vi "UHR-Fleezers Control (host) -TL FB Corrected.vi"(0 "Tab Control":T5(tab)) -> ()   [LabVIEW 2013]
uses:
  <vilib>/Utility/miscctls.llb/LVPoint32TypeDef.ctl
  <vilib>/Utility/miscctls.llb/LVMinMaxIncTypeDef.ctl
  <vilib>/userdefined/High Color/nirio_resource_hc.ctl
  <vilib>/Platform/TimedLoop/XDataNode/timing_clust.ctl
  <vilib>/Platform/TimedLoop/XDataNode/nitl_modes.ctl
  <vilib>/Platform/TimedLoop/XDataNode/wakeup.ctl
  <vilib>/Analysis/baseanly.llb/Mean (DBL).vi
  <vilib>/FPGAPlugInAG/PCIe-7852R/niLvFpga_Open_PCIe-7852R.vi
  <vilib>/FPGAPlugInAG/PCIe-7852R/niLvFpga_Reset_PCIe-7852R.vi
  <vilib>/Utility/error.llb/Error Cluster From Error Code.vi
  <vilib>/rvi/errors/niLvFpgaAdjustHostInterfaceError.vi
  <vilib>/rvi/interface/common/niFpgaWaitOnOcc.vi
  <vilib>/FPGAPlugInAG/PCIe-7852R/niLvFpga_Run_PCIe-7852R.vi
  <vilib>/express/express analysis/Spectral/Block/exnSpectralBlock spectral measurements PSD poly.vi
  <vilib>/express/express analysis/Spectral/Block/exnSpectralBlock spectral measurements PSD WFM.vi
  <vilib>/Waveform/WDTOps.llb/WDT Append Waveforms DBL.vi
  <vilib>/FPGAPlugInAG/PCIe-7852R/niLvFpga_Abort_PCIe-7852R.vi
  <vilib>/FPGAPlugInAG/PCIe-7852R/niLvFpga_Close_PCIe-7852R.vi
  openfpgaref.8.6.ctl
  <vilib>/Platform/TimedLoop/XDataNode/XDataNode.xnode
  <vilib>/rvi/interface/nirviOpenFPGA/nirviOpenFPGA.xnode
  FPGA Bitfiles/UHR-FleezersInst_FPGATarget_UHR-FleezersCont_9yP24kGuHI0.lvbitx
  UHR-Fleezers Control (fpga) FB changed - 10.3.vi
  <vilib>/rvi/interface/nirviMethod/nirviMethod.xnode
  <vilib>/rvi/interface/nirviReadWriteControl/nirviReadWriteControl.xnode
  <vilib>/express/express analysis/Spectral/XNode/ExpressSpectralMeasurementsBlockNode.xnode
  <vilib>/rvi/interface/nirviCloseFPGA/nirviCloseFPGA.xnode
  <vilib>/Analysis/NI_AALBase.lvlib
  <vilib>/Platform/TimedLoop/XDataNode/XDNodeRunTimeDep.lvlib
  <vilib>/vision/NI_Vision_Development_Module.lvlib
  <vilib>/rvi/errors/niLvFpgaMergeErrorWithErrorCode.vi
  NiFpgaLv.dll
  <vilib>/FPGAPlugInAG/PCIe-7852R/niLvFpga_ConfigureFifo_PCIe-7852R.vi
  <vilib>/FPGAPlugInAG/PCIe-7852R/niLvFpga_ReadFifo_PCIe-7852R.vi
panel:
  out "Tether Extension (nm, calculated)":dbl=nan format="%0.2f"
  in  "Set SP to Reading":bool
  out "Trap X (AI1)":T1={"Trap 1"=-1.0, "Trap 2"=0.899993896484375}
  in  "Trap Pos FB SP":fxp<+/-,16,1>=-0.092803955078125 caption="Setpoint"
  in  "Trap Pos. FB ON":bool
  out "Trap Positions":waveform(dbl)[](graph)=[{"t0"=timestamp(12.90000000000001 s since 1904-01-01), "dt"=0.15, "Y"=[-1.7479351299698465e-12, -1.7479351299698465e-12], "attributes"=variant("NI_ChannelName"=variant(string "Trap 1 Pos."))}, {"t0"=timestamp(12.90000000000001 s since 1904-01-01), "dt"=0.15, "Y"=[6.991740519879386e-12, 6.991740519879386e-12], "attributes"=variant("NI_ChannelName"=variant(string "Trap 2 Pos."))}]
  out "Action (%)":dbl(knob) scale=-100.0..100.0
  in  "Trap Pos. FB Out Scale 2^n":u8=23 caption="Action Scale"
  out "Location path":path=path "C:/Users/Fleezers/Desktop/UHR-Fleezers Instrument - Charlie/Locations.txt"
  out "Location Matrix":string[][](array[string])=[["N.D.\r\n", "N.D.\r\n", "N.D.\r\n"], ["0.19233\r\n", "0.00156\r\n", "0.20615\r\n"], ["N.D.\r\n", "N.D.\r\n", "N.D.\r\n"], ["N.D.\r\n", "N.D.\r\n", "N.D.\r\n"]]
  in  "radius":i32=10 min=1 max=20
  in  "clear markers":bool
  in  "trap\nmarkers?":bool
  in  "Pump 3 contents":string="Bottom: ADig beads" caption="contents"
  in  "Pump 1 contents":string="Top: DNA beads" caption="contents"
  in  "Scripts":T2(tab)
  in  "Take Stepping Data":bool
  in  "Got DNA bead":bool
  in  "Got ADig bead":bool
  in  "Cap 1 Flow ON":bool=TRUE
  in  "Move Cap. 1 (DNA Top)":bool
  in  "Cal/Data Acq. Spot":bool
  in  "Dump Beads":bool
  in  "Cap 1 T ON":bool=TRUE
  in  "Cap 1 Samp Flow ON":bool=TRUE
  in  "Offset 2 Set":dbl=2.0
  in  "Offset 1 Set":dbl=1.0
  in  "Cal @ (MHz)":dbl=20.0
  in  "W/ Offset 1":bool=TRUE
  in  "Offset 1 Start (MHz)":dbl=13.0
  in  "W/ Offset 2":bool
  in  "Offset 2 Start (MHz)":dbl=16.0
  in  "Pause at Closest Delta (s)":dbl
  in  "Move to Delta 2 (MHz)":dbl=41.0
  in  "Attempt Limit":dbl=30.0 caption="Limit"
  out "Attempts":dbl=1.0
  in  "Wait Before Save (s)":u32=1
  in  "Fish for Tether":bool
  in  "Closest Delta (MHz)":dbl=13.0 step=0.25
  in  "Stop F (pN)":dbl=10.0
  in  "Then...":string(combo)="2"
  in  "Move to Delta 1 (MHz)":dbl=15.0
  in  "Tether Alarm?":bool=TRUE
  out "Tether":bool
  in  "TA Cancel Save?":bool=TRUE
  in  "TA Green Off?":bool=TRUE
  in  "Raster Set Upon Tether":u32=1
  in  "Save at end (5, 6)":bool
  in  "N Steps":dbl=20.0
  in  "Step Size (nm)":dbl=0.34
  in  "Save ave factor":dbl=1.0
  in  "Dip Trap Delta 1 (MHz)":dbl=15.0
  in  "Move Trap Before?":bool
  in  "Save Data After?":bool
  in  "Green ON After?":bool
  in  "Dip Trap Delta 2 (MHz)":dbl=15.0
  in  "Move Trap After?":bool
  in  "Duration (s)":dbl=1.0
  in  "Dip for Protein":bool
  in  "APD to Watch":bool
  out "Duration (s)":dbl
  in  "Action":string(combo)="Yank"
  in  "Fl. Triggered...":bool
  in  "Fl. Delta Thresh. (kHz)":dbl=0.6
  out "Waiting":bool
  out "Fl. High":bool
  in  "N pts to average":u16=6
  in  "Yank Delay (s)":dbl=3.5
  in  "Yank to Delta Array (MHz)":dbl[](array[numeric])=[16.3, 15.85, 14.85]
  in  "N Array El":u8=3 min=1 step=1
  in  "Random Choice":bool=TRUE
  in  "Force Yank":bool
  in  "Force Reset":bool
  in  "Y change (mm)":dbl
  in  "Profile":bool
  out "Sigma/Mean 2":dbl=nan caption="Sigma/Mean" format="%#_2g"
  out "Rate sigma (Hz) 2":dbl caption="Sigma (Hz)" format="%0.2f"
  out "APD 2 Rate (Hz)":dbl format="%#_3p"
  out "Primary Video Display":T3(plugin-control)
  out "Waveform Graph":dbl[](graph) caption="APD Line Scan"
  out "Messages":string="7:59 AM\tUHR-Fleezers ready.\r"
  in  "APD Ave N":dbl=10.0
  out "Int. Time (s)":dbl=3.0
  in  "Stop All":bool=TRUE
  out "Sigma/Mean":dbl=nan format="%#_2g"
  out "Rate sigma (Hz)":dbl caption="Sigma (Hz)" format="%0.2f"
  in  "Tab Control 6":T4(tab)=enum."Imaging"
  in  "APD 2 Offset":dbl
  in  "APD 1 Offset":dbl
  out "RMS (Ang)":dbl=nan format="%_2g"
  in  "Bead Sep. Int. Time (s)":dbl=5.0 caption="Int. Time (s)"
  in  "Below (kHz)":dbl=0.5
  in  "Above (kHz)":dbl=2.0
  in  "Adjust Scale\nto Mean":bool
  in  "Rescale on Mean":bool
  in  "Offset (nm)":dbl
  out "Mean":dbl=nan caption="Mean (pN)" format="%#_3g"
  out "Force":waveform(dbl)[](graph)=[{"t0"=timestamp(12.90000000000001 s since 1904-01-01), "dt"=0.15, "Y"=[nan, nan], "attributes"=variant("NI_ChannelName"=variant(string "T1 X"))}, {"t0"=timestamp(12.90000000000001 s since 1904-01-01), "dt"=0.15, "Y"=[nan, nan], "attributes"=variant("NI_ChannelName"=variant(string "T2 X"))}]
  out "APD Chart":waveform(dbl)[](graph)=[{"t0"=timestamp(12.90000000000001 s since 1904-01-01), "dt"=0.02, "Y"=[0.0, 0.0, 0.0, 0.0, 0.0, 0.0, 0.0, 0.0, 0.0, 0.0, 0.0, 0.0, 0.0, 0.0, 0.0], "attributes"=variant("NI_ChannelName"=variant(string "APD 1"))}, {"t0"=timestamp(12.90000000000001 s since 1904-01-01), "dt"=0.02, "Y"=[0.0, 0.0, 0.0, 0.0, 0.0, 0.0, 0.0, 0.0, 0.0, 0.0, 0.0, 0.0, 0.0, 0.0, 0.0], "attributes"=variant("NI_ChannelName"=variant(string "APD 2"))}]
  in  "Calibration":u16(ring) items=["None", "Position", "Force"]
  out "T1 X":dbl=nan caption="T1 X (pN)" format="%0.2f"
  out "T2 X":dbl=nan caption="T2 X (pN)" format="%0.2f"
  out "Bead Separation":waveform(dbl)(graph)={"t0"=timestamp(12.90000000000001 s since 1904-01-01), "dt"=0.15, "Y"=[nan, nan], "attributes"=variant("NI_ChannelName"=variant(string "T1 X"))}
  in  "Amplitude (nm)":dbl=3.0
  out "Bead Mean (nm)":dbl=nan caption="Mean (nm)" format="%0.2f"
  out "Difference":dbl=nan caption="Difference (pN)" format="%.2g"
  in  "Take Detection Laser\nImage":bool
  out "APD 2":T3(plugin-control) caption="APD 2 (Cy5)"
  in  "Flip Green Filter":bool
  in  "Set X Only":bool
  in  "Set Y Only":bool
  out "APD 1":T3(plugin-control) caption="APD 1 (Cy3)"
  out "Detection Laser Y":T3(plugin-control)
  out "Pointer Y (V)":dbl format="%_3g"
  out "Pointer X (V)":dbl format="%_3g"
  in  "Set Confocal Spot (X-Y)":bool
  out "Detection Laser X":T3(plugin-control)
  out "Saved APD":dbl[][](graph) caption="Most Recent Time Trace"
  out "Trap Delta Graph":dbl[](graph) caption="Most Recent Time Trace"
  out "Save APD Deriv":dbl[][](graph) caption="Most Recent Time Trace"
  out "Delta Fl. 1":dbl
  out "Delta Fl. 2":dbl
  out "All Signals":waveform(dbl)[](graph)=[{"t0"=timestamp(12.90000000000001 s since 1904-01-01), "dt"=0.02, "Y"=[0.0, 0.0, 0.0, 0.0, 0.0, 0.0, 0.0, 0.0, 0.0, 0.0, 0.0, 0.0, 0.0, 0.0, 0.0], "attributes"=variant("NI_ChannelName"=variant(string "APD 1"))}, {"t0"=timestamp(12.90000000000001 s since 1904-01-01), "dt"=0.02, "Y"=[0.0, 0.0, 0.0, 0.0, 0.0, 0.0, 0.0, 0.0, 0.0, 0.0, 0.0, 0.0, 0.0, 0.0, 0.0], "attributes"=variant("NI_ChannelName"=variant(string "APD 2"))}, {"t0"=timestamp(12.90000000000001 s since 1904-01-01), "dt"=0.15, "Y"=[nan, nan], "attributes"=variant("NI_ChannelName"=variant(string "T1 Y"))}, {"t0"=timestamp(12.90000000000001 s since 1904-01-01), "dt"=0.15, "Y"=[nan, nan], "attributes"=variant("NI_ChannelName"=variant(string "T1 X"))}, {"t0"=timestamp(12.90000000000001 s since 1904-01-01), "dt"=0.15, "Y"=[-0.0004235663930173644, -0.0004722739341410556], "attributes"=variant("NI_ChannelName"=variant(string "T1 Sum"))}, {"t0"=timestamp(12.90000000000001 s since 1904-01-01), "dt"=0.15, "Y"=[nan, nan], "attributes"=variant("NI_ChannelName"=variant(string "T2 Y"))}, {"t0"=timestamp(12.90000000000001 s since 1904-01-01), "dt"=0.15, "Y"=[nan, nan], "attributes"=variant("NI_ChannelName"=variant(string "T2 X"))}, {"t0"=timestamp(12.90000000000001 s since 1904-01-01), "dt"=0.15, "Y"=[-0.0005883053071687949, -0.0006281319620349712], "attributes"=variant("NI_ChannelName"=variant(string "T2 Sum"))}, {"t0"=timestamp(12.90000000000001 s since 1904-01-01), "dt"=0.15, "Y"=[nan, nan], "attributes"=variant("NI_ChannelName"=variant(string "T1 FB X"))}, {"t0"=timestamp(12.90000000000001 s since 1904-01-01), "dt"=0.15, "Y"=[-0.0004680013428144157, -0.0005167699209570592], "attributes"=variant("NI_ChannelName"=variant(string "T2 FB Sum"))}, {"t0"=timestamp(12.90000000000001 s since 1904-01-01), "dt"=0.15, "Y"=[nan, nan], "attributes"=variant("NI_ChannelName"=variant(string "T2 FB X"))}, {"t0"=timestamp(12.90000000000001 s since 1904-01-01), "dt"=0.15, "Y"=[-0.0006226691488387671, -0.0006504715109714008], "attributes"=variant("NI_ChannelName"=variant(string "T2 FB Sum"))}, {"t0"=timestamp(12.90000000000001 s since 1904-01-01), "dt"=0.15, "Y"=[-0.0007901852473525123, -0.0008601641895809732], "attributes"=variant("NI_ChannelName"=variant(string "PSD Y"))}, {"t0"=timestamp(12.90000000000001 s since 1904-01-01), "dt"=0.15, "Y"=[0.00031556138798181086, 0.0002525101474044007], "attributes"=variant("NI_ChannelName"=variant(string "PSD X"))}, {"t0"=timestamp(12.90000000000001 s since 1904-01-01), "dt"=0.15, "Y"=[-0.00019678334910122974, -0.0002453993346964931], "attributes"=variant("NI_ChannelName"=variant(string "PSD Sum"))}]
  in  "Signals to Plot":i32(listbox)
  out "Trap Disp. Freq. (Hz)":dbl=6.666666666666667 caption="Freq. (Hz)" format="%#_6p"
  out "Display Period (s)":dbl=0.15 caption="Period (s)" format="%#_6p"
  in  "Trap Disp. Downsample":dbl=10000.0 caption="Downsample" max=20000.0
  in  "APD Disp. Scale":dbl=0.1 caption="Scale (Divide,\nfor above plot only)"
  in  "APD Disp. Downsample":dbl=2.0 caption="Integrate" min=1.0 max=30.0 step=1.0
  out "APD Display Freq. (Hz)":dbl=50.0 caption="Freq. (Hz)"
  out "APD Display Period (s)":dbl=0.02 caption="Period (s)"
  out "FFT 1":cluster{"f0":dbl, "df":dbl, "magnitude":dbl[]}[](graph)=[{"f0"=0.0, "df"=16.666666666666668, "magnitude"=[-331.1367572010275, -79.05506245821404, -86.61411242440559, -88.4728176091699, -90.3181253945935, -94.12566333707997, -92.52740723119955, -94.92192587982518, -99.60936585245742, -96.87568627870715, -94.02570383337763, -83.8058550151726, -97.57441397235512, -101.59968530846606, -101.523049255742, -103.35038532190343, -101.58594091014982, -102.96098031851216, -91.39759462745924, -103.75019963279499, -104.45030075054324, -103.04245334279298, -104.0720279134107, -106.06482372394834, -103.69131867828104, -104.40395035115309, -105.96420043276396, -107.6735556337804, -106.673030006608, -107.34889066208132, -108.05626565233933, -106.25659018850432, -105.29934513380842, -105.43096056709592, -108.3728498841465, -106.0555440144992, -105.78001282181421, -107.48741857324953, -108.67624970548897, -105.39976667156175, -105.91413119232612, -109.4222808198164, -107.0898971593174, -107.91164191890915, -108.26032038855709, -107.58332347164534, -108.23559688234297, -108.01271040303237, -107.66511723652701, -106.51901583170391, -109.27249501469946, -108.55647681594805, -107.93499259231463, -107.05068166453935, -109.13641475410455, -109.29679733781423, -108.19360835527803, -109.57747591546632, -109.58364591011674, -110.47061433372711, -109.8144340420426, -108.79067462293897, -107.54887553357234, -107.99559866705923, -108.85023923652685, -109.68733225238618, -108.51101278437793, -108.51620475114115, -108.22212402200637, -104.63726950302143, -110.2989919678048, -107.61796444414897, -108.68882962798736, -104.79193983043893, -103.59504263746938, -93.64633660288543, -101.9191640501395, -105.73717393151816, -108.92572458793902, -107.43962662800902, -107.79595323081325, -107.0923101993207, -108.17603277205289, -107.87074270713183, -109.20899066381877, -108.61832060412445, -109.10072003106593, -105.76480632823524, -108.60877649218978, -109.67541158970121, -110.2286232768028, -109.84952155309578, -109.33772024076384, -109.95251642394683, -110.14777282585466, -109.13825677905699, -110.05989365698167, -109.39359990189426, -110.56255614635295, -109.66477183197163, -108.9397158528824, -110.26529907650465, -109.20049464984628, -108.20183857013548, -109.09752250184418, -108.00440442238454, -108.35465963524055, -111.16774134451799, -110.34812550238405, -108.94506763426756, -108.72845542102493, -109.41512344014713, -112.44661664432377, -110.35437330889101, -111.32939440655925, -109.42989530434981, -110.98084669076195, -111.92160561143541, -108.57755551751093, -111.40042616180912, -110.15284955891853, -112.21455132279115, -111.40787773511747, -108.82949641635288, -110.13442122547907, -111.42229298204664, -112.06314940885191, -110.6015308813694, -109.51144097251623, -111.15989713761475, -110.25535755335385, -109.65868178057926, -110.51649885452997, -109.77194745285269, -108.4234206864394, -109.50892632093968, -109.46471287444389, -107.92241289271415, -109.72283805386196, -108.63426821579918, -110.37316681536255, -111.09713996884652, -110.32903619589223, -105.32012665515045, -107.36858557554393, -108.00382215905725, -110.06430686942338, -108.81666625979916, -110.01277074453823, -110.94194741225512, -109.65934609082873, -107.80979136006962, -112.81333866824724, -111.61474300955487, -109.83998277184975, -109.45953946904639, -109.79640584952526, -108.19172301667324, -109.28894656674316, -107.61471301278785, -108.83814006090513, -109.08866847726084, -108.20250571862371, -107.96222236861584, -107.03811197900873, -108.93533000393974, -107.74482548035408, -110.79811544577694, -111.1387476496877, -107.42970105883512, -109.18442281176472, -108.73546184641192, -108.71800246690864, -108.51945944378063, -108.06825856571285, -107.27210712368412, -108.12304695877637, -107.84933283677306, -109.73682373154998, -109.32284761503395, -109.31328817453769, -106.68762108642842, -109.79203616876461, -109.9020278896408, -110.27080024357275, -108.54152101558762, -111.00464391726017, -112.42244020766577, -110.82707315747889, -111.00344011890857, -109.90461839395674, -109.42877207451863, -109.73549298167016, -111.67494793393293, -108.85799077901427, -108.5348443278263, -109.803781083881, -108.30644755543659, -108.5079527456017, -111.2055351312823, -108.53089994340155, -108.01739789012176, -108.70360662855235, -107.95873456794631, -109.58297170693093, -108.9372401694271, -110.15921663527153, -109.22399119911955, -110.89883651739237, -108.92840112258382, -110.0545300523626, -109.05961065387005, -109.45831398589371, -108.61239387653227, -110.13001256174265, -108.80060224137931, -109.46327400696283, -108.0177965824709, -109.29727944627197, -110.3237255895986, -109.03258262543821, -110.97880178489321, -109.70034895077919, -111.16405638194153, -109.17324451464711, -109.65698250854277, -108.96750235822178, -112.00534231585624, -108.69274607723942, -108.98110446396657, -108.40723795464795, -111.44459094807324, -111.74799245277113, -111.1601960491512, -108.92048232753773, -110.30506377784799, -111.33145973979093, -110.91850998672503, -110.33684985776448, -108.90206518366908, -109.28458878227542, -108.98773986023751, -110.85813863075646, -109.00041591105906, -110.84543686681204, -109.84382395806176, -109.69722434763266, -108.50915601095721, -107.80829925826895, -110.59736107582401, -109.75377770317087, -109.3992084496136, -110.51151565846742, -112.49753959826434, -109.7299632589479, -109.54070743868353, -109.90314341132164, -111.05974202976806, -109.03766862152392, -109.46667095459878, -109.52800799036197, -111.3163121356807, -110.07817134522178, -108.69251657453547, -109.40472158898045, -109.71400709815576, -110.60534468715097, -109.46937396724682, -107.70342491418788, -109.86331122597839, -108.64971387994616, -110.90117371097081, -108.34928840565928, -110.04172889660904, -111.52979926554961, -110.34759300823305, -109.62712781837159, -109.24131154553284, -110.23196152450447, -108.68509612326807, -108.0246905483419, -106.61876139289784, -101.5519630114271, -80.57695480953835, -102.03744443354402, -107.1449217193017, -110.0695213407169, -106.61597783999268, -110.79221011808191, -109.58974545931426, -109.1149802216988, -109.20993813088597, -109.63768480465863, -110.10428394219181, -109.08445084271477, -108.83472375362581, -109.69508502050168, -108.05588796178941, -110.62586360101581, -109.95315261676905, -107.52208264977473, -108.80708007514875, -110.43484881098874, -110.45942171588936, -107.83804717866751, -109.98973910294193, -109.3496496054193, -108.425252911127, -110.94579264380809, -108.54181722177951, -108.67696070083541, -108.4150202151644, -109.24973583101504, -112.0454922608961, -111.29046597340738, -110.75018248960077, -109.38326363603683, -109.2033340336957, -109.45076170874889, -109.52878049853727, -109.32340869724774, -110.98123395128233, -110.75736340635505, -109.7218385823809, -107.97422606064993, -109.77313701758703, -110.95948744392717, -110.08996774172691, -108.51011830110778, -109.78063140243836, -110.65996628628228, -109.83684298615616, -110.33329049188029, -110.13755118968292, -110.3717925645783, -108.55302219178951, -106.86811628734195, -108.6302156589162, -108.75341391045045, -108.32589578384841, -108.70061474734084, -112.30742263527534, -109.16842570592085, -109.29767035534508, -108.87829025017463, -108.2255616391397, -108.4316108616088, -108.82995906929271, -110.40135575415563, -109.51623498946435, -109.79409808792403, -107.03832759632121, -108.36534528684132, -109.72010868372905, -107.90933028179892, -106.95643597294047, -111.29929166165778, -110.23001135794706, -108.98838015381585, -109.79115357104436, -108.18627479511115, -108.14988122174307, -109.12074063466532, -109.41904850488358, -111.40409873721113, -108.83156790193294, -108.77032248953847, -108.88363158686694, -108.47515048290681, -105.94172147874599, -109.38146940214403, -109.21277078848794, -108.11309390545507, -110.70840012427504, -109.5504457849329, -109.52330684534209, -110.06776026911132, -108.21949434182314, -111.21266686269992, -108.78581501170974, -108.43115799297222, -109.63260325780062, -109.84070220619535, -109.72041980780126, -110.29615941882527, -110.60316734262464, -108.79165446414692, -110.95840439895592, -109.64926233107009, -109.16526769544322, -108.65292362430982, -109.56113898129935, -109.85693046339026, -108.92316027325207, -109.79492493553914, -109.38157962945887, -110.24545136266825, -109.30031463492487, -109.0795429936869, -111.4091719525013, -108.63499083917162, -108.43863465339358, -109.23207864880891, -111.21947487191643, -109.24525201480154, -109.56842406077318, -109.46711940800672, -111.91389548262572, -108.15655736690546, -108.71882059966947, -111.26328503478568, -110.95027143873176, -108.4853106242357, -110.36902802777546, -109.9314203579182, -108.77686164101732, -108.71871020068312, -111.04829661168574, -109.95072655339462, -109.88221342875462, -109.53241732756136, -108.2625005404823, -108.00677030040697, -110.19659317581693, -108.93858924796267, -109.46817875483995, -110.78063992017232, -111.11066570318451, -110.78774336696706, -109.19199744617812, -108.54914256407436, -109.28414960420909, -110.64143585101183, -110.5855350821307, -109.47578632252726, -108.89705360836223, -109.89214013612292, -107.93271261027171, -109.32631601340563, -108.60274611341092, -109.40110159872573, -110.889237682208, -110.01391165813328, -109.99747108785071, -108.65542819213674, -110.37211847668736, -110.44656500845738, -110.8128133834973, -108.8909299260433, -110.19551227077532, -111.37647266643523, -110.83802189730321, -109.98519377913681, -110.52378970770522, -108.16970420057817, -110.70974729773344, -110.76836765494402, -110.26884275594577, -109.22041044268806, -109.87809744746195, -107.76823252107832, -109.12119474042969, -110.28066108731146, -108.55000033509207, -110.18152097767907, -110.73030521152278, -111.49470908029893, -110.2320929919509, -110.03370979233021, -109.79181668155233, -108.6673501209991, -109.86695766650877, -107.88926518046961, -110.95525003776572, -109.18130359755742, -110.42618009658618, -107.90341931158893, -111.44736855661769, -110.72634267386593, -109.29945988519303, -107.67889101961411, -108.81148059987765, -109.13375212757057, -109.8122873383549, -109.80176697684155, -109.96342275204768, -109.90406635707086, -108.75674342748256, -110.12362902701081, -109.82151095527837, -108.62543344241836, -110.09171852771195, -110.21434637862887, -109.97254504855631, -109.27043209093468, -111.35149588204125, -110.12399876776051, -111.65983675538546, -109.28788875768564, -110.86554069990251, -111.26990906470603, -108.60956517491746, -111.49613890850938, -111.79685722966795, -109.26269485364045, -110.38555615546439, -109.40641023162068, -110.966136593156, -108.78892524584494, -110.29340727375603, -111.44032043281035, -109.95212021173755, -109.79233511584334, -112.41184021118175, -109.73687851881148, -108.65493879781806, -110.76132988919045, -108.43230346094671, -110.32968175895853, -110.29890782023821, -108.77609076424456, -110.3298662333555, -109.47734504217333, -108.2677295732245, -109.21234363352882, -107.83278941978479, -108.85136784424789, -108.43241251530755, -109.76609391460555, -108.53204373005357, -110.9660641972934, -110.3152512161094, -110.72570499399905, -109.23877906286317, -111.72407743101837, -109.20311421918561, -108.06021800233717, -109.29288625761943, -108.78395253409145, -111.85250172876302, -108.78827588901797, -109.79775055719482, -109.12089297455859, -109.49896359356035, -110.34432647103819, -107.94700097960238, -109.30489238477631, -108.89170290869342, -108.82574563272509, -110.11024077194833, -107.37946433552314, -109.60167933458756, -107.80625057819019, -110.11489057210264, -107.35436859378505, -105.69819484613895, -109.11280625683739, -109.27770293057978, -107.7053735252589, -109.75022444894368, -109.3310543596577, -107.87683693707739, -108.19931495338068, -109.26462246191564, -106.71885779297867, -100.00018022217961, -92.54434511397295, -107.20472143807373, -107.39203415155283, -110.04461177268398, -108.48860496315312, -109.0057168110333, -108.37627790492552, -108.4108380728248, -109.65509454313073, -109.64243000632982, -97.04219069306761, -109.0928856629964, -107.9760697315632, -107.52611064047497, -108.87702814778996, -109.08437599027614, -110.70097118837974, -109.00969860961283, -110.38275386163214, -110.0699155421545, -106.91498895181175, -106.22178738309017, -109.36827866896039, -107.59953130968307, -109.19516217272808, -108.31502495393616, -109.384158926223, -107.11670654202719, -108.09436312738853, -110.14559230873704, -109.84997663447679, -107.83465335309926, -108.60947100624459, -108.9932479423645, -109.17174810371898, -108.79457339828916, -109.40909327982367, -109.6328723628302, -109.51081854476179, -107.63054408568418, -109.63728404010122, -108.51163794839918, -107.55002282725216, -108.97796212764939, -107.24648164623483, -112.21470452291085, -108.74294024554423, -109.62070777514892, -108.05768666239368, -109.8224946685739, -109.34575507446003, -108.53536952609525, -109.60789300457671, -107.56681538208278, -109.22777325016398, -108.79047910308894, -110.10332477250668, -108.00206387955672, -108.45604004720035, -109.00645795765472, -109.81039564269616, -108.92785144634745, -108.3978471520567, -107.94411095685999, -110.53486519304262, -108.8773780319227, -109.03345093296107, -107.30746693745031, -108.54277704832029, -108.77629108166091, -108.91111762599647, -107.74965195880401, -109.97375370738439, -109.76326492689246, -107.91717581777407, -109.0730556927617, -107.66804873204664, -110.40438871064791, -108.05794247751498, -108.80206615156494, -107.51329354700796, -108.83687012994949, -107.57713176895379, -107.94774159581414, -109.41894615439651, -107.10869425078764, -110.51480854078629, -108.92221367099775, -109.91358786461535, -110.1744263092835, -109.30795472883494, -107.91359710691006, -109.77888185049835, -109.52060975706438, -108.66686651982212, -108.71041801553639, -110.13619546359467, -108.87957097273856, -109.72150387215271, -109.00776068810654, -109.70251113927438, -110.75769213896399, -108.53234896741436, -109.69439526582246, -110.15412541604617, -108.25183374628219, -107.97402569656481, -110.34920156998648, -108.45106995186384, -108.82031145748209, -111.38690005057539, -107.01968459818563, -110.3044500039584, -110.8755481852125, -111.08915057663255, -107.94824988655199, -110.21669144934839, -109.90539774633154, -109.58985438756767, -110.12258796623348, -109.41689951612143, -109.31128210476795, -109.00258476567323, -109.11093063041056, -108.83347064311234, -108.32685287566952, -109.44770946560935, -108.40145063144861, -109.68448193892085, -108.76525439243828, -107.62837139034596, -107.39300298848994, -109.36993934990318, -109.2465218489418, -106.66307369796812, -110.15891092764934, -109.57151745419041, -108.92425698310808, -109.8036704717834, -108.79751146756549, -109.25926431818017, -108.46260574057584, -109.1967554647261, -110.63319560262356, -109.02343067385144, -111.22073171487528, -109.4731095097105, -109.69335000085164, -109.48782989577005, -107.95204227683271, -108.19468255763758, -111.36195112053247, -109.55696116543685, -110.3130767640534, -108.9621824253354, -109.99735074896789, -109.20198058456344, -108.12100614259485, -111.27227490807289, -110.09248554008288, -109.14395535060149, -110.80882692379708, -109.22632926901655, -108.64497210802793, -111.00030482190711, -111.1317849358033, -107.43140429257826, -107.9783302193555, -109.2639893652291, -108.97008485446163, -108.66556668859064, -108.12995785876932, -109.73001061107855, -108.09691302413727, -110.68391499215569, -112.78583642012705, -108.7093037763389, -110.67868795924797, -109.0190959349128, -108.36247198231372, -109.82829353258869, -108.24916379311045, -109.84154533905823, -108.55470160833775, -109.75438989348815, -108.82865632118325, -107.63622268162582, -111.00943492886312, -110.81824358463759, -109.46028423652966, -107.52479398900992, -108.99087806823736, -109.94494831750349, -110.26788355564504, -109.8954055022304, -106.9478122391182, -108.91705388158901, -107.76095584490312, -109.28456723055147, -109.7982307261767, -108.98552661346622, -109.98937979783426, -110.57907422426224, -108.68113463944836, -108.06257240208589, -110.0707224529617, -109.19515280354733, -109.35868842818849, -110.37311467065695, -109.0404734478992, -108.16686395270187, -108.61859220485148, -109.19986437876149, -108.19707189725302, -110.06564239663074, -108.87850403465154, -110.63824157544798, -107.36918104067212, -108.7008736325543, -110.9359398265406, -111.08529123080929, -108.44209934821818, -109.79529621208783, -108.38917887958179, -108.169117639508, -109.24332926356216, -110.50584058811704, -109.63592524002665, -109.32261039377495, -109.16720880524552, -109.3084314664462, -109.5812223978583, -107.70213196487856, -108.0557884982431, -110.67058020007828, -111.68459781023608, -109.66270627185824, -110.52536245663693, -109.70208409132103, -108.78645420809342, -109.23122088059863, -109.24601474121832, -111.25604763816514, -109.50225851581177, -107.32434217163818, -109.28548556764925, -107.59972621660836, -110.46928774723048, -109.25950101547609, -110.32016453935465, -107.78482761561703, -107.89462895091089, -107.51366154391481, -108.08036891159172, -109.53371809947035, -101.2452927166745, -109.32763325689056, -107.52166868423687, -109.89648659445174, -109.11350200980485, -109.81336712738089, -110.02799517445062, -108.02767143538516, -107.97850220501483, -109.50772934896838, -109.31069875721964, -108.49991657749598, -105.60880911233095, -109.79128597340213, -106.91084537903113, -107.84880087118997, -109.63628170511824, -109.03203967193224, -110.64186113413658, -110.98027990365594, -112.33841002907062, -111.01793075565425, -108.58025797022215, -110.4259296883756, -110.38643255981424, -108.93051671115133, -110.97544177116494, -108.63883100482677, -108.37581711765226, -108.90240163126536, -107.94688047875466, -109.9482937437732, -110.09097112364414, -110.09805032265376, -111.44307114024532, -109.15483789122554, -110.9713708217832, -107.8548737634672, -111.41418477109195, -109.45699779859628, -97.03595099331734, -109.16746744169623, -109.66209204485918, -112.57048704774604, -109.73989735035725, -108.16252575067017, -110.7546980664636, -108.91536673403449, -109.20509151422344, -111.0260632167785, -109.62924582406518, -110.45466277291722, -110.2973970018937, -109.67550222925419, -108.84481022020094, -107.23686414357573, -111.79004633370906, -109.85453094194085, -109.45617270081004, -110.73920606732504, -108.90879956851099, -109.67774425528265, -109.4745715721361, -110.18080454693559, -109.26079184315502, -109.41692499885505, -109.02240975088358, -107.80833423058168, -109.32657361431549, -107.87138278655101, -110.910364670719, -109.70067156846706, -108.55301754282077, -109.4243252157005, -109.77567725161107, -107.83737232063925, -110.36509412773016, -109.6371048811367, -109.49430894422814, -108.55509251499753, -108.03996302911446, -110.4385715838736, -110.08864436068788, -109.48922484379962, -109.90865554258562, -109.7491963238264, -110.04796094537969, -107.413043439116, -108.54229076126079, -108.2522516728666, -109.75464941327974, -110.26795832300996, -109.28073673851144, -108.62990200974927, -109.89408067552287, -109.09160284731726, -109.90740624925795, -109.92534708896517, -109.79578862362752, -109.97278346890566, -107.80679350393824, -112.81728446281548, -108.09689504419987, -109.89549991422173, -108.43930976031248, -109.95153099843282, -108.18277483720716, -111.89607792605433, -109.52567003805, -109.17125106979698, -109.64300739407085, -108.21045178846524, -109.64036472149706, -109.02324448538845, -109.039163008889, -110.41006510134076, -109.50289952116489, -110.4732620447796, -110.08777181504614, -110.15589511434341, -109.55705089158471, -109.2547682932589, -110.86823885471617, -109.96330502176939, -109.85995369810554, -110.63211290903473, -112.08007783432191, -110.24725218052279, -107.62861148917592, -110.08691795849435, -108.89793794632287, -111.07702220466341, -109.46946126482341, -109.19747345337464, -110.70018609416007, -109.66366205691908, -110.78032312133551, -108.05724200456513, -108.195661625627, -110.90724508408255, -110.08307674771669, -110.76863516643007, -110.46620425061583, -109.16986788877276, -109.61921294239114, -108.51159432329543, -109.96308336765689, -107.38178944242856, -111.95930944846394, -109.3329826827624, -109.59119636368249, -108.83148571828912, -110.46194288788257, -105.87694286145472, -107.985886302892, -109.2975019660806, -111.05138725716857, -109.60005889204612, -110.92871351729086, -110.73480546964537, -108.41587420326718, -109.84275465824477, -108.8249071047676, -107.65358887817105, -108.3254150042995, -111.47362100321767, -112.7287536850025, -108.8217125660507, -109.50232320231771, -110.29587061625348, -109.30644535112089, -107.69178032077258, -110.84522325672016, -109.3735891463141, -109.12506388923123, -109.65582307934665, -111.11427272192576, -112.19827973435466, -109.11306367925813, -108.19203577968261, -107.89831568266465, -108.85805249169313, -109.51100049661844, -111.71546684086955, -109.53880495724334, -107.07739286222231, -110.66836728754211, -111.5415170557177, -110.16051267940297, -110.6107546662698, -111.36389129556191, -107.77888179117923, -110.34160392509817, -109.61287125994414, -110.23791773883013, -111.00669159903549, -110.97165069538953, -109.43965413392434, -110.6813161690388, -110.31441293654314, -111.96129906273796, -108.15998218707462, -110.08095912053633, -109.41084567452768, -109.28774416263552, -110.80159950384204, -110.41956747809755, -108.85005186267244, -107.9069227847757, -108.84249369063123, -109.92569208845894, -109.34109797584448, -109.41334788055491, -108.76462023086997, -108.22069272136177, -107.0786679601274, -108.30206755098202, -108.57613406368954, -110.83330887636482, -111.93966942736989, -109.76373713473264, -108.25782074884941, -108.16490627215555, -109.93351470267982, -110.75525684428368, -108.22814762283093, -109.73442331991602, -107.53145627482685, -108.27195221226805, -110.33032779278457, -109.48951857415828, -108.12599093700939, -107.97627415508097, -108.81426859968796, -111.21764717894752, -109.80856212352333, -110.92658779118501, -109.71551885834796, -110.38682741010847, -108.87671328341361, -109.68368600774755, -108.35359806351899, -111.7519400010676, -109.89407081573103, -108.24301180922755, -110.00646944788126, -108.6685299083706, -107.52856885980722, -111.7622363038509, -111.0025144494897, -108.64719599357296, -110.62968467177518, -108.821509935539, -107.94915453463719, -111.53070432277694, -109.87282048586256, -110.71167589371663, -109.79225006081626, -109.96203471712074, -110.29921092232489, -110.10644439440416, -111.28815007382043, -111.19165661703703, -108.46024117100558, -110.22528296512183, -110.32184972386672, -110.05120383416072, -109.78792549362107, -109.00355659956696, -108.85989369286315, -113.00899556732638, -110.91756826567867, -111.25016866167897, -111.84225040552181, -110.54451635944174, -110.72722829912917, -109.60759702177283, -110.49362602516815, -108.74419542915284, -110.3379671069179, -109.66259088220754, -110.45956400953156, -109.13956157147233, -109.27130155486806, -110.83015602667983, -109.17970724944131, -109.09662765889193, -108.0447366108107, -108.9536269357457, -110.35663108940085, -108.73418835472056, -113.42965806805827, -111.81270536656905, -110.06155590173537, -108.76582224646269, -106.7488061675813, -108.5700320158723, -111.11038264410035, -110.41435767488723, -109.12763443489911, -109.30517580756394, -111.61251165371237, -109.8116632664339, -109.36845864976851, -109.00390009629231, -110.54359197165573, -109.52629258465976, -110.75932197632896, -109.50903215359567, -107.42652056246085, -107.81146496533543, -103.22224383145215, -108.53803076819163, -109.78623360072066, -109.66306634612869, -110.80245829141279, -111.87835085452016, -102.27372781471168, -111.27763038431458, -108.45838423437681, -108.79077917058028, -109.31951755762685, -110.05415097017186, -109.5535934823387, -111.62732254641111, -110.73478247119641, -109.9468722686683, -110.39698367573979, -109.30612942398305, -109.7578384694043, -109.34817295524313, -105.56944757301993, -110.1940418750125, -109.27076023513962, -111.03491935225027, -112.2980497521063, -110.65725497955563, -109.0567530102422, -110.31700596563523, -109.64508026365678, -109.6190471404421, -110.52566833759428, -109.68595899227789, -109.7431160985074, -110.4798230300751, -109.45506977604765, -110.69504157940786, -110.63067849573177, -108.06456949500138, -107.99354148885966, -108.11349194720599, -109.15944121207349, -110.61766925164031, -110.14145801314527, -110.67420842201165, -111.91532881806512, -112.15901550030345, -109.94774413630104, -109.2819568305201, -110.94623189179737, -110.17685430287735, -110.39082916961016, -109.53953238698966, -110.76940623620611, -109.89327922318515, -109.10275695043765, -110.21445972656734, -110.58968777252528, -110.57016757660259, -109.59208496373341, -109.07946946465374, -109.10762003745964, -110.36892993974607, -109.81864495218393, -112.12972189864566, -109.26185849434863, -111.56305819991357, -111.36019621828058, -110.3397604159226, -109.58675612753163, -110.58041217474447, -106.34739062044932, -108.6722699609389, -110.03906060709869, -109.16794717548382, -109.65012481802809, -109.35377624077988, -110.51889143862303, -110.03397458059777, -110.7981307056636, -110.56653507062292, -107.61367005067231, -109.99279736988825, -111.79875182878175, -108.60382315996031, -109.71381533228038, -108.60388131505613, -107.0933685540362, -107.86037690830757, -108.40980028847238, -108.83869602763895, -110.76921375395764, -109.96766364716046, -110.8256171465781, -110.13805084291067, -108.5349140035878, -110.57158437465219, -110.8920694413417, -108.71646695477324, -108.33274238445665, -108.96152108305608, -111.03750932994224, -109.48915027983756, -110.29725207211165, -110.79527247268442, -109.47969936716117, -109.79306701834035, -110.16840035577498, -110.29840230783668, -109.15306387075587, -110.72651274964761, -109.08881658764956, -110.8349724030761, -110.64653625576447, -111.40392562616867, -109.94581588927414, -108.85136340231294, -109.77228546607624, -111.48297395390018, -109.7334001251941, -109.30537415590783, -109.63937411233408, -109.69785848648013, -109.3523781030017, -112.04667421182404, -111.56311816195343, -108.18548447362308, -110.63388993686104, -111.39768634137992, -109.87157345395542, -108.6734208287271, -109.46213300216168, -111.75774769437145, -110.10245994173216, -109.52385139033495, -110.96513097775451, -111.8709319163154, -111.54948269614047, -110.29760900080463, -108.52168175904663, -111.09033925738258, -111.14752744054172, -108.83074523709202, -109.05704141259113, -111.74377805749482, -109.57200906899736, -108.84121318623825, -110.86657990204343, -109.54363603755047, -110.89448416316372, -109.58965570570145, -110.21012263847972, -110.4063470702923, -109.5021950342969, -110.33648801598177, -110.90551031296536, -109.69205870504638, -109.8648503154861, -110.28183391384131, -109.65970942950766, -108.43615680946908, -111.11790511866548, -110.89043476451553, -113.64898442872548, -113.08004494963895, -110.81525412051718, -113.91009875719509, -110.95802128672312, -110.40944585634135, -110.33464695414992, -109.98984645778987, -110.18795067005652, -110.62364351231234, -110.44029833291248, -109.01598585569788, -110.95430216511514, -109.77987141110621, -108.54452361812068, -111.41780266439777, -110.47172771858405, -109.06084635984516, -109.30794593246578, -108.8764083815745, -108.18222749506985, -110.31330487887435, -109.04176821738014, -108.8558386035048, -109.47888284507395, -110.01459604573937, -110.48596659065309, -112.6781342298378, -109.85522803775775, -109.0569534499285, -109.08991286548698, -110.89485727880403, -109.18715778948663, -111.50381433568144, -111.3545424730884, -110.07710926239977, -111.99977850157067, -109.47444853853723, -109.81605328527645, -110.74995213151195, -112.56834665925544, -108.52052472391404, -110.89121213995557, -112.02004142355113, -108.66413739656008, -111.10053848695652, -110.41241079991636, -111.80152991764473, -110.21746151515111, -110.63265128607344, -109.483042128511, -112.78639954059729, -109.47114195846122, -109.23309637902875, -108.97133643967169, -110.08909147812822, -111.01105271457081, -111.18602432128249, -110.04633990216801, -109.53453538673071, -108.81939452082017, -111.13486114285661, -111.65877073200598, -111.63763706753498, -112.14107810664572, -113.6231865196724, -109.31743865878806, -109.18551713085722, -108.74951309653638, -109.28206426212142, -112.36687029711229, -110.10933061193728, -111.29501093502684, -108.19021080564794, -109.34497312126749, -110.37228033937312, -108.63277512903049, -110.61033993911002, -111.2975761598062, -111.49780004751436, -109.91019436685814, -109.32789992989028, -111.4482538110117, -110.1538439123475, -110.66347034043578, -110.05055133068794, -108.53002033538341, -111.7522199783972, -113.49108651193104, -108.03793940563418, -110.07108694011555, -110.83958739865201, -109.62805629409038, -112.69637731014087, -109.57996950503268, -110.104850643722, -108.83376203949506, -108.69400304840181, -110.59434352922563, -110.69121011800921, -110.18694553784364, -111.90598571547098, -110.30230802494223, -109.66810649416752, -112.6017099000434, -111.00296745333219, -110.64462650261785, -111.4775358707403, -111.98753241268494, -112.26574909791167, -112.04796822399412, -110.65853064447325, -109.6623218025264, -109.40559579075378, -110.42174451813142, -109.18991987957241, -111.02050178263048, -112.77950487440032, -110.42443751566815, -111.35440372400903, -108.5263524245987, -105.07498063939795, -107.15444425741984, -110.4508720018025, -110.25163264819463, -111.1383261104107, -109.91171620173931, -110.52200560606038, -110.5299174299573, -109.34628087255733, -110.26101817411786, -109.65071853372183, -109.66953335961068, -110.83590602054682, -110.980546313788, -109.4110066989163, -111.47223607390256, -110.00281523859483, -109.4088722967626, -109.00401922839337, -109.59655302543185, -109.7359970854586, -111.46016206343049, -110.23478747568004, -109.29441275295858, -109.82941912510167, -110.43088525283673, -108.21649744751299, -108.70220592702613, -105.2334473604296, -110.60620657984927, -107.97533820921146, -110.7664079806058, -110.56406610911355, -111.76465470250328, -108.84172809688911, -111.03661078143631, -109.85351980370237, -110.70091167176791, -109.52380717508088, -108.4356492672842, -112.25498760397127, -110.69648730540193, -110.36748838594507, -109.99090797924349, -111.2678642544111, -110.42541694325627, -111.4575545259775, -109.3211175669008, -112.7465573314208, -109.56208667784249, -111.59733497772172, -109.42295730962105, -108.55804089331346, -108.71397903286748, -110.09188290952392, -108.90810063278326, -110.31333217069538, -109.69794714542728, -109.06210020835357, -112.42465112160288, -111.74630553904855, -109.99304310093493, -108.93867687355595, -113.1669287525049, -109.09193568851137, -109.27500368450697, -108.99643325722404, -110.53962759110647, -111.2052088429852, -110.05855563908841, -110.30763723153481, -110.03411001268613, -109.6161415052669, -110.6304714466923, -110.17116005754627, -109.0753171640551, -110.92564270851628, -109.60831770517053, -110.25913363817017, -107.76644895378317, -109.2619309023068, -107.64198246311884, -107.37056168314048, -107.31978563121643, -107.68171928702894, -104.57515288104209, -104.75187637758803, -105.27246893266054, -106.96524396060869, -105.93920355631757, -103.66449995825586, -104.08476660009461, -104.53081578265315, -103.0148493379086, -106.74751670818362, -104.92309629919443, -103.98320340724693, -104.81633219413234, -105.77996356028235, -107.12559309216644, -107.28196039053535, -108.84583578337953, -109.4494696919565, -109.15525441177898, -109.7634811359225, -110.79433338587495, -108.44440079452527, -108.79597700117748, -109.98590735173822, -110.72144284267539, -109.30550753718086, -109.70072152916897, -109.65801130162137, -109.65949265997646, -109.82238573025273, -110.30669821947491, -109.83394128869384, -108.90433312205332, -110.664046708231, -110.39926453734134, -110.37725911098757, -112.12508639032839, -110.26795666332589, -108.98741993218054, -107.76168841100478, -109.82334992872889, -110.83516363498563, -112.60649745671253, -111.1960726449926, -111.03919163866381, -112.05129034965563, -108.83187987662883, -109.57240688505179, -109.32857861150738, -109.54934849013647, -108.29359879300195, -111.5179112931669, -109.52702486426027, -109.95429980789645, -110.7011078611564, -109.43204524997455, -105.56031249677113, -107.70609254346495, -108.78303653454363, -108.11457060956113, -110.44215460317537, -110.78267897406572, -110.33119812901934, -109.34449539666907, -108.82636558484161, -107.1834151347969, -108.83808254322192, -108.2542825327446, -108.80298057862501, -107.59922121598055, -108.9131916496929, -109.51519107961856, -107.7704986323755, -108.79678029009878, -111.13791068210752, -110.402746275919, -111.31702623823912, -108.49812727557243, -110.63723264798182, -109.32890666586829, -110.29721723278237, -111.66560929315017, -111.04227698307153, -111.36927505376269, -112.5203298417673, -109.93967930487354, -110.14533835678606, -110.3868348991775, -110.85413569165249, -108.44519725537315, -107.93391978795047, -109.82778679299085, -109.79311153223738, -109.25261055399044, -111.47738679135526, -111.11775495397512, -108.65898844492045, -110.26505495390529, -111.02017977446526, -110.34817965403467, -107.55161094495372, -110.21667403085983, -112.43970497917284, -110.70535338255132, -110.79438078890512, -109.81809822502822, -108.99167960596515, -106.5556893069368, -97.51736665041192, -105.29926513345109, -108.72453297392224, -108.23203912463346, -109.50324111400698, -110.9939986929772, -108.05367524487318, -108.37339392211176, -109.8553291283933, -110.46179639493138, -112.48795697163695, -111.88145079973545, -110.8678969738583, -110.62677605624849, -111.83824818603244, -109.76798658735359, -109.6654742351465, -112.58543522753767, -110.3406716250781, -109.55013159400883, -108.00481229232405, -109.90793236599207, -111.28597960985334, -110.54144527494444, -110.14704702870655, -111.2652554338908, -110.97520848958668, -108.63647576273343, -110.52472680617548, -113.16137826273847, -109.62457037485827, -109.53869420402964, -110.71399284283449, -108.55435337782664, -108.09492728294455, -112.2373886856363, -110.3693019226993, -111.65116752865308, -111.3223986412311, -109.67734725401074, -111.36420709226297, -109.14293108556625, -110.5982939020188, -110.29596476096043, -112.69847120697035, -108.39052787054206, -109.06205229490357, -110.00045399262885, -110.71775009467346, -110.69530760167493, -112.54144940754935, -109.55755373438097, -107.88943697845929, -109.98578587243783, -110.14202980613851, -110.80051915904802, -109.11327182471621, -109.50637030500913, -109.77023677605327, -109.98552825925917, -110.40235854896, -109.37603004890141, -111.36989177909379, -110.8399811877331, -109.30394670937987, -112.2769814990538, -109.10893172594731, -109.17733972841754, -108.35968166480572, -112.64492569586005, -110.13779257328873, -110.64439690778532, -108.45446935516622, -108.97325006911116, -110.54637968933774, -110.66412364132371, -111.38627695224784, -109.8942998516069, -110.36392017322382, -109.92355133054227, -109.61886697310419, -109.71969465343778, -109.85627196259388, -112.1407808286419, -111.1013489416651, -110.70428953307596, -109.3454280179969, -110.22984684615578, -109.53826801613613, -107.83673208330934, -108.72742563398342, -109.5745872123195, -108.83031823548816, -110.89059911076627, -109.87842545384129, -109.21980161063786, -109.07140273870678, -109.04628915564135, -108.79255665097845, -105.20875397856382, -110.0838008881032, -109.68293832806683, -111.24644641302518, -110.01257579497496, -110.99281477454484, -108.99296184719546, -110.96495665514604, -110.70404386182749, -108.25078498739035, -100.77667501455139, -107.61479263900088, -110.06600976399395, -110.02035637581871, -111.45524052052504, -109.975541184397, -111.07333860975358, -108.4808974233161, -109.59513524582242, -110.74711589861774, -109.50005300854993, -105.23071652566294, -111.81094849223531, -109.0168079712372, -111.89029991620679, -109.90672274216391, -109.30959446424889, -108.23718655264584, -110.10868108588909, -109.21139771899594, -110.33333323577992, -110.25792318324204, -110.67825932924109, -112.33148517950511, -108.9724848367048, -110.78371843797613, -111.40913868573313, -110.2930522718577, -111.9538408094371, -108.63639312641844, -112.4462941079034, -110.40266356498321, -108.66617580940074, -109.44306834729083, -111.08962916641603, -110.52132608161017, -110.53757698855654, -111.5587344449704, -109.77722315102946, -110.40060629757771, -109.45395807961631, -108.77558572395142, -109.0151938598724, -109.80739619986889, -108.9332873172888, -112.49933978358132, -111.28667321897437, -110.40629082858706, -109.9829216820938, -108.85102919990373, -110.84179127037925, -110.27309817549309, -109.88857884367955, -112.24517967927224, -110.23377125710859, -111.26951227953063, -110.09782138347559, -109.77508406986834, -110.55359722398646, -110.09534729906368, -109.96333904888587, -110.29372855476366, -111.36651812163072, -109.97141184588116, -110.16701683369045, -112.8562627359291, -110.66651146857079, -108.78873821095968, -108.59208174618087, -110.31784275318834, -109.43177042415276, -112.80272887161644, -111.79874205007107, -111.08216899537892, -110.73699224045636, -111.04738767291953, -110.43395896705012, -111.62106163510778, -111.32599933330843, -110.29360981749807, -109.66562228449096, -109.21316193790335, -110.06363162177448, -110.54480468587292, -109.31791670875509, -112.65386492377107, -109.91857609999171, -110.57233605624137, -110.7597333064856, -111.49767138733276, -109.36548654843229, -112.34145274183716, -110.52831153822652, -111.55802243871352, -111.81399803046556, -110.17680125962372, -111.23811621944807, -110.48042049674514, -112.43786993562033, -109.56507357271987, -110.67030752598993, -110.86377249100713, -109.06001892813467, -111.37023727930494, -109.52881096984436, -112.95107295160436, -110.49467818026214, -109.29804210589607, -109.89270706931751, -109.46354468058833, -112.10350702955014, -111.06083529077077, -110.49996587015904, -111.1617248913634, -108.84725633199014, -111.42852695852422, -110.01433866707184, -109.11616968390972, -110.76961079765468, -111.80403513904453, -109.84442686379181, -109.65447921666167, -111.3378640555306, -110.8882647652338, -112.58014202075226, -109.67128881545659, -111.73429980763389, -110.82258070774773, -110.71895931098041, -112.5117489008152, -109.16182299471309, -109.71651258790612, -109.7770618808562, -111.94294809571427, -111.1629115541574, -109.57489224865171, -109.8402445779754, -111.17931450307283, -110.09045865447595, -109.23658206733491, -112.54929616847242, -110.5150381158864, -111.32296447909377, -111.64472156295191, -111.65832771066007, -111.03359562742956, -110.85303206770837, -110.80655337650862, -109.3712696310075, -110.57313454785879, -111.18525355670417, -111.67423695430561, -112.00829831274282, -111.08915434609605, -110.3298290221436, -108.68552957386795, -112.11377370993225, -110.80288297661977, -110.33640536217185, -109.5907971201988, -107.9195263775506, -108.50223113159429, -111.91191347156142, -110.29585599512956, -109.50902788911351, -110.76819145749467, -108.86899533416589, -112.09963049260891, -110.13374376572433, -110.15881393584463, -110.87392107947531, -109.18658540731009, -109.72734703956934, -110.18732487568724, -108.76554115185057, -109.94122289815374, -110.39583285609643, -111.09540935727229, -110.6618176357367, -111.6281345666718, -109.69686483639367, -110.31633402076315, -110.61246951748903, -111.73300235294965, -111.34221378834899, -109.46708370903485, -110.70412671997354, -110.7007891485379, -110.31685483435038, -111.03016917417074, -110.94517365625376, -109.46580797053619, -111.20935248224806, -109.20661126636224, -109.50147037097533, -110.14241781654353, -109.8510950344643, -111.3794198224028, -111.28966889207122, -110.43347441663424, -109.86759980279523, -111.92101892013198, -109.31594011390644, -112.92253433794441, -110.74000829597605, -110.3690783911604, -111.9386136764295, -111.04196305034188, -110.41800427558245, -110.94287511448232, -111.66035388807579, -107.53723747644062, -110.68014818358719, -111.86628806511304, -110.12097497430523, -109.69880468221378, -111.4312783987915, -109.18240866486639, -111.45649839248873, -110.1242345454651, -113.75911576151633, -112.71747598882953, -110.9614554157337, -110.92294419716129, -110.87229098694876, -111.09943759113875, -109.48107247947176, -108.62783006742795, -110.8108025857779, -111.63342408317932, -112.0221522906341, -109.96411229549527, -111.29821085030613, -110.04566676239914, -108.41674583097112, -107.50256474992416, -108.68086611003493, -110.3738906060137, -108.86763212826641, -109.81681043446049, -111.04539822346567, -111.73290882980949, -109.75238769150758, -110.55268275367449, -110.48423701377924, -112.1116140908134, -109.53952175199518, -108.538611608547, -111.3788321484912, -110.36378736224961, -110.37712171023523, -109.82150687920334, -109.17046632238393, -105.1169578108227, -110.84067642540583, -112.91626789016587, -111.32030958133453, -108.93375913686056, -112.44450956563915, -111.1596840012794, -110.17380444915341, -109.634859036508, -110.68819277718731, -110.0648098825346, -108.87385575091399, -111.99676414571755, -111.32585405719519, -110.59892045991457, -110.32589048340424, -111.1172696292077, -109.79946399891651, -110.10030723919304, -110.71841081343656, -112.23013150012054, -108.94400401141407, -109.71044551701596, -111.77560214164039, -109.68779520039777, -110.96119601299907, -113.66477058855787, -110.17794649102234, -110.30159876509862, -110.11953836266514]}, ...(2 in all)]
  out "FFT 2":cluster{"f0":dbl, "df":dbl, "magnitude":dbl[]}[](graph)=[{"f0"=0.0, "df"=16.666666666666668, "magnitude"=[-324.19011195451765, -78.1272953812706, -85.85545438627958, -89.30587144190069, -92.90590394398903, -93.63083388385274, -91.8644929119412, -95.26924857401164, -97.0710469181336, -98.01148078956652, -99.33043660296804, -95.58776817681839, -99.9570097527269, -101.45494093095093, -101.51838334751548, -101.00386616525799, -103.01963069818913, -103.20223925731209, -103.53783076500916, -103.48065647812659, -103.97797518531912, -104.58942778240602, -104.46991277190502, -104.59813972158683, -104.56685024229951, -104.69893799348945, -105.05669000016238, -106.17061117835001, -106.43303821862656, -107.39468286383597, -106.2899368267905, -105.7863846168199, -105.17170638885071, -104.53818172761852, -106.70340956723133, -106.55444321137247, -106.67654843051936, -107.79888413750199, -107.86424326005849, -106.09722609215336, -107.71648639013972, -107.79500725395155, -106.17330953637067, -105.43663624517525, -108.04970689199158, -109.92106271611999, -106.2505251183406, -110.60221373795562, -107.11377887451098, -108.4126937286195, -108.37794745021417, -113.22457316369011, -106.38281814065472, -107.55385617652075, -108.93026538982782, -106.19334142366085, -108.90462602264525, -107.63084712174981, -109.12192537022624, -107.90627042480016, -109.44472079190832, -108.91731458372392, -105.74102972706788, -105.74407510394178, -107.5989477192235, -106.2838630137392, -107.46190542725505, -107.38881299750702, -109.08024783239452, -104.97871836903269, -106.65424712290651, -107.04966019632134, -106.16202578092883, -102.98374199247179, -99.1568704142098, -87.07383781389657, -96.41471411313154, -102.65176579899618, -107.65674867775193, -102.85397890306213, -107.58658613411464, -104.79044898833125, -106.65282019869865, -108.65027966345534, -109.46169054950127, -108.69969979291741, -110.4048706652988, -108.81020193837274, -109.42808902484134, -108.85398463561398, -108.3849716744813, -109.1844457168716, -109.32787859535676, -111.01992124870878, -106.64843449415699, -108.9926343573667, -111.59837822080355, -110.57121677672183, -111.17280164669164, -110.68901970586144, -111.69013245592781, -109.90200577018311, -109.3554172126163, -110.7515368822992, -109.2863324212524, -109.66209701262974, -108.50795548698007, -110.58126481096504, -112.36093896766921, -109.78612141282203, -108.85120530917233, -109.91424431080952, -109.84698632196245, -110.93960894966105, -109.77214706089354, -110.30762971422381, -108.77791302937449, -110.79522659679036, -108.47242514643455, -111.20629758187835, -109.05996769621125, -111.13574821570619, -107.79388178889101, -111.5768481279296, -110.52058839597171, -111.58729762739313, -108.99000864386126, -111.6585121505227, -110.50715371958135, -108.87151956974363, -110.30486244367107, -108.32392040018144, -108.1769507919999, -110.43198471512189, -109.81454097966842, -110.26717009815644, -110.82924135076777, -110.34103661156989, -110.0692667126265, -109.34555682020833, -109.1694484721415, -109.9940980324044, -110.81940616215803, -108.21162003366862, -107.97087538330561, -107.55312461506225, -110.60339321606872, -110.09004629292225, -109.05860430198882, -113.1412749514818, -109.81628200948371, -108.62343219429849, -109.48172424209761, -110.85978755785311, -109.47778611557064, -108.81728552967951, -107.47864241666747, -107.61735128422292, -109.62511618983821, -110.32417726356636, -108.24287897478176, -108.60460879530194, -110.2181558494026, -107.95550802888957, -110.80234484950323, -111.09955733353904, -109.43923052503506, -108.98949130235951, -110.05778199870154, -110.36224432927585, -108.13523430027999, -110.681114579241, -110.49106131529867, -108.73493328004297, -110.07663907252234, -109.9968931372618, -112.10715231091008, -108.80994125105168, -111.63774865669372, -111.54355694032755, -111.64024217585788, -109.34986300492378, -108.88053713185408, -111.14370830146245, -111.17327416167232, -110.36311492990576, -109.99414559884396, -112.96912007380595, -111.43191437097785, -111.71327312809349, -108.77202323682606, -110.25970374932486, -112.59574277180732, -109.77247894866957, -110.09219852365874, -111.7197662726775, -109.85454092697009, -110.06789440397942, -110.38055758638309, -111.04251386932805, -111.54279434240568, -109.74385329575985, -110.98924544863415, -111.17898077762852, -110.98364252730245, -110.75024385843372, -109.24766708578407, -109.67753987004863, -110.6537235844391, -111.84436313010086, -109.12654337292446, -109.65519521121124, -111.1845162935778, -110.5009101465602, -110.22980642268818, -110.88540043278346, -110.29249073109453, -108.80459864528464, -107.49372141121728, -108.50353962704821, -110.00730069533373, -112.012876492648, -109.01283702976382, -109.07442203290057, -108.2961442983685, -111.60962842680907, -108.84312815413224, -108.6276642979969, -108.75132871638827, -109.30004903844721, -107.20359872252604, -109.12175943862074, -110.43914247337625, -109.55954680842791, -110.37116786618797, -108.55907813251434, -110.19249995041955, -106.95269845697632, -111.07027929458712, -110.1073996792702, -110.61729280468039, -109.6419175310234, -109.47995019876329, -109.66602827275211, -110.01953864498805, -108.45989120418268, -109.79778555296474, -109.94663827736616, -109.52410616839379, -110.58014441463794, -110.09182359045897, -111.0487262011397, -110.49609187214915, -110.6114701312941, -111.17752423063314, -109.74965389041003, -108.58973724447526, -108.84292130035902, -108.90689510645983, -110.69840140049361, -111.30494362640982, -111.00224390075273, -110.50848328538423, -111.59232911931113, -109.30826761863756, -108.44510893127558, -109.63744704504391, -108.95037574307332, -111.36486409910674, -112.74508631930381, -111.03952454593811, -110.57133212903979, -110.59969855145111, -108.25570461975128, -110.44617635200193, -110.32190307214704, -110.95204704643322, -112.0595421753479, -110.45342552693265, -112.50183987758867, -110.08217804938009, -108.90353583389084, -107.02032313792242, -88.3334978919524, -107.92027625495886, -109.83148570028482, -110.30427997450572, -110.92855407802753, -109.67404674397338, -111.03606345823586, -110.58277018943096, -109.77692362669393, -109.39170901729935, -110.20711662408928, -109.41601946806779, -110.34213214925832, -111.2283900972803, -111.51682597931386, -110.47069117801351, -110.93808974285523, -111.11277478000933, -112.50698886748012, -112.12918507523611, -110.46316790252011, -109.9387334819968, -109.78723249688426, -107.13037722044297, -108.16132376075751, -109.07255491017162, -108.85068428558272, -110.28038153100799, -107.77611023481016, -110.69754506886444, -110.09495581837979, -109.21214884561816, -112.62718526248648, -109.22048725312992, -109.17793923163308, -110.87372121410577, -109.71902632604333, -112.61041177225496, -109.6374750969677, -110.74738952366951, -108.93404661877067, -109.84938675700889, -112.25316361679832, -110.30788094875312, -109.26929069321925, -111.20853536783942, -110.05212566057608, -111.72448131932816, -111.55474439772887, -111.81988954424324, -108.44452452934028, -109.21897824914645, -109.55634869894358, -111.36318572800242, -110.05777399011298, -109.64458567712875, -108.73315084760529, -108.93332091319675, -108.4816455312154, -108.80120578498936, -108.1804470361839, -109.7177707524778, -109.31977709844544, -109.33603116022124, -111.46120546572519, -111.7480378245176, -109.17907150677627, -110.47970652472505, -109.73718750984082, -109.7935026884937, -110.40458408612054, -110.91781389491092, -108.39352075861481, -108.27512197925346, -109.59155075404814, -110.40183121737397, -109.25423373270381, -108.37769008625712, -107.91335995938509, -109.5576520703013, -107.27392145737491, -110.98592762117059, -108.41809950647861, -111.48163889400448, -109.70961684769624, -109.22952568656495, -109.76504719131209, -108.86928627177666, -107.97855299877004, -109.8412204399902, -109.6690048999326, -112.28329030175193, -111.54977099314607, -109.55689540119126, -107.93716711232997, -109.84247640855929, -111.5098351445789, -109.14317615215809, -110.28319116384824, -110.57901069942578, -107.2890252845352, -109.66754569546274, -110.15708115946433, -108.83782190109405, -111.60783857760667, -111.46884385151185, -109.21985333366634, -109.63605494317056, -110.87999187262697, -112.26992029775087, -111.05491095860552, -109.22795442529183, -108.99135781712076, -110.46475190704264, -109.35746113713218, -109.29125989270668, -107.40922407684049, -109.24391685563656, -110.41554602144217, -110.68952735085914, -110.62457364102458, -110.39856310555466, -108.84256124354566, -110.01614601335088, -109.8071306678428, -110.2804500736802, -108.76205061238203, -110.3962440297242, -108.98253716257014, -109.32990745926702, -111.17276766165281, -110.41113652364085, -110.36616199963426, -112.09767002991742, -108.43599666470733, -110.91876588140981, -109.05329272502944, -107.07198690769708, -108.72934463903034, -108.6666471996132, -108.97529973794413, -109.68895260146817, -109.2658844652487, -109.75690097249196, -109.38585024123027, -110.17593039468063, -107.87223111061134, -108.15261097418302, -110.09277437980633, -110.8665497655964, -108.43061614348413, -110.3052458526819, -109.22446919161898, -110.51909692711594, -110.06620699121913, -109.53439413051383, -110.31952463872884, -111.4732125902982, -110.41443606663168, -109.9579358088152, -109.930778061577, -108.5473214465574, -109.34719220288939, -109.16964653934396, -110.04824158176345, -109.42616539603762, -108.3556027482992, -110.62331917617789, -111.3652147859356, -110.12362012120938, -110.13175448595814, -111.20110099151856, -111.50643914621541, -108.11659117128028, -111.06037600347967, -109.03822892917451, -108.25678204604324, -110.82608024151122, -109.15887945314851, -109.88255674562845, -111.18322672526185, -110.95836040044516, -107.91535345885436, -110.66285812468733, -109.61906549925033, -109.58059721670746, -109.65198009505977, -109.65950565672951, -108.95264505276342, -109.23343669003113, -110.74308548011575, -106.39170014998685, -109.61471203101753, -108.24258770956924, -109.84609566640096, -107.83834185503922, -108.93052854090027, -107.55568820082641, -109.758551082242, -110.65892780872205, -111.99907420485852, -110.71043004141137, -110.62257237494617, -109.15610413532767, -106.87403836327807, -108.19175324576331, -110.27819583792918, -110.23918003777561, -108.29703377268754, -110.07182881114713, -109.60256111108491, -111.00394752430006, -110.30750337485472, -108.78309624082331, -109.24103013025798, -108.76979253891403, -109.91618737478264, -108.83915940855513, -110.92536150834754, -109.72250903746432, -108.96533939688658, -111.08949280651164, -109.20335070860871, -109.37826578362439, -109.77953166722301, -110.1867310744785, -110.07114559821346, -110.7003631567182, -107.86455899696074, -108.94113264174617, -109.35999427135138, -109.33627364788704, -108.96588828808375, -109.08716536982254, -108.73575375369026, -109.47770132070654, -109.83726171472907, -110.73516506891792, -110.56827134787686, -107.65667508354096, -109.30200115708924, -109.28406803847896, -110.55374624323233, -111.2017766725333, -108.50851279608973, -109.79494403619485, -109.08320018013063, -110.21850624918747, -108.4652936555984, -108.74837610538873, -108.81326140648238, -108.83830180036702, -108.785270477003, -110.01845876259073, -108.76030368637825, -108.57879884880157, -110.6610608456059, -108.74669367794318, -111.55956030460833, -110.22906685783455, -110.48411613865359, -109.48060880085136, -112.77556331479562, -108.2676071206087, -108.8571136162698, -108.56944905160177, -109.16406757131058, -111.42259299295839, -108.25216316582294, -110.48487127684025, -109.69532331373831, -108.13992755196784, -109.2987762526628, -109.82536192480795, -111.28650061088359, -109.12820736404241, -109.37960655471406, -108.96014976926716, -107.97535047619023, -112.31953123574708, -109.06198330523004, -107.52722515967098, -107.31555373665437, -99.89671790804692, -107.44442600896275, -110.6549218761941, -108.02265794322076, -109.63582761762919, -110.00574746987859, -109.51565124961209, -109.3550083591902, -110.4541529175301, -107.85799722437162, -105.1197113090786, -110.25038075579738, -110.39710812865657, -109.3618876098789, -107.6131301952152, -109.21529527621463, -108.7995754403799, -108.48347353145697, -106.45678488065816, -109.60427918561142, -110.81194387812535, -109.52215044127382, -109.88751598659705, -109.30205143590227, -110.74984456751768, -109.03952092986351, -110.69170786328897, -110.39236248162467, -108.65456161733339, -107.60439764386904, -109.97367926606955, -110.2754359970249, -108.81546418006434, -106.99691398176165, -108.42047325825182, -107.24499915944605, -109.28116135603187, -108.70650358781573, -108.05516916105047, -107.20893100196241, -112.07029265690055, -109.38099990478445, -111.53461820465232, -108.11312509555277, -108.76714028655223, -109.89565008459624, -107.71879172001115, -108.08434857420214, -108.79142773619792, -107.25153085963885, -110.05595039449301, -109.31604222314259, -109.94405791565286, -109.04715370361387, -108.89278831045846, -108.84682466376424, -110.0067927716526, -107.63768959294084, -108.98109382020348, -111.4720219575084, -110.76023788797733, -108.78599647633777, -106.59726674064618, -108.66715709719243, -107.99134359630926, -110.11396713841884, -107.21091759882775, -108.08576824949941, -108.80217666857972, -111.72949572713338, -107.33126296136014, -107.33731660097102, -108.04470462977443, -109.42963925921418, -111.03517778720736, -109.55293581015796, -107.99948151285162, -106.59480934999681, -107.63777243313498, -108.96490626068824, -108.8948210299064, -108.30870516747477, -109.13612869658097, -109.59971429402015, -110.2571461001396, -108.7655464686992, -109.81144209568883, -109.80796806645141, -109.20948481699544, -108.68653880881129, -109.26329796696166, -109.22428132233863, -110.12571678351438, -109.14615461144786, -107.08261621308327, -109.11338327144382, -107.75421565039201, -107.45291780756361, -109.00477000647248, -107.41031480478154, -109.98948062864928, -107.45953654921264, -106.37522884807879, -107.7786128523167, -108.03610987358499, -108.05926797128022, -108.59400205554164, -109.89620453365603, -109.03811240487515, -109.96909236705363, -109.28212981785472, -109.6772152101994, -108.26493868190678, -110.55558039199732, -106.6252818398841, -110.19075011176416, -109.56520012524705, -109.8023423576176, -111.2697570480663, -108.26752571816566, -112.00337375484828, -109.85709226796116, -109.36922081321148, -108.8424844298318, -111.2512302139209, -110.61775974680471, -110.22501328999012, -107.76874906708105, -110.71023653476604, -109.4025656165291, -107.66667684986125, -107.59759854092948, -107.94763263251238, -107.3888591871119, -108.62692803125044, -109.18012867988286, -107.78662871481455, -108.5072814073944, -109.50348958982907, -109.95177634938378, -107.78756251182895, -108.03865042797304, -110.1814993556385, -109.34937567548833, -109.52162025123161, -109.50819015441117, -108.20953105254624, -110.52154040214435, -109.3324404469266, -109.2696617050831, -109.54675609195674, -108.5940367000989, -109.40184828664549, -108.2518305610941, -108.55972691669434, -109.03647225394408, -108.48166656251695, -107.42023429066523, -109.42453054302521, -110.09532345960083, -108.78315822119662, -109.97508586102265, -108.22687406536997, -109.17110028890058, -110.15390449992647, -107.88577458651508, -108.28851074361447, -108.52030295163331, -110.03496861709483, -109.40014319167584, -107.73048113044877, -108.17571683963915, -110.34839852994926, -108.55894048192191, -108.74107339998285, -111.17734138993401, -110.22946440841412, -109.45511941802884, -108.0657300641843, -109.33797363184166, -106.95974095511333, -107.93068343723691, -109.78867669512647, -107.2087297624043, -109.542665021243, -110.05035859052961, -110.30235238883523, -109.20586170783808, -109.2796396673401, -109.14260673746566, -108.22019460542734, -109.99011886871159, -109.89103038547285, -110.36964772493243, -108.62340319923602, -109.06779821699769, -109.21830861066148, -107.7402395759509, -107.7178850938205, -113.45665085929117, -109.24039191621704, -109.30387033426037, -107.61849760982835, -109.41430582703529, -109.11482836392241, -111.89328423764577, -111.84653367963301, -109.00674896486915, -109.84488648739638, -109.41914760797953, -108.53442910169935, -109.66883322968232, -107.68762956301386, -109.82583101109167, -107.83405397804887, -108.78052031141966, -107.37842078941692, -105.40843158543845, -108.81430898189338, -109.57374640194516, -109.41111270322058, -108.82621700188898, -110.2552502368822, -110.23903890097205, -110.52171662278697, -108.21249857906324, -109.97268479379733, -108.20088823960992, -108.85682002802234, -110.11642849164285, -109.94087886999255, -111.63180946270296, -108.20899499456195, -106.73341567332112, -109.90003508676807, -110.14688274481229, -109.62259307329889, -107.57811196819495, -106.88584597822792, -109.16132624528932, -109.78677836397806, -108.59319344451784, -108.55877448618652, -109.46883711353044, -108.47309455543844, -108.09487065732198, -109.82219079158135, -109.63780237877428, -109.28348848877269, -107.62893405379826, -109.46986737961593, -108.03089712610223, -110.3931917410696, -106.06970126043262, -109.41866550703786, -105.31710372440419, -109.20218082282653, -108.28467118008108, -108.80026326744611, -107.40729224715713, -111.07322915141532, -107.1057186510818, -107.98286374205958, -108.51298722989311, -108.69632670891366, -107.96509231988331, -108.15882223414738, -106.85862416470376, -109.70705792539056, -108.64519930633055, -106.78708421443504, -109.43552377900174, -109.4474526498122, -109.10135248755788, -111.43316642580763, -109.33457343739448, -110.23547887071898, -108.95690647379442, -109.21159903769149, -108.12969562680841, -110.82751409340537, -108.55724349027832, -109.8796329603075, -108.50369978374582, -107.43145467247209, -108.60003323209516, -108.77155705999647, -109.33806063660796, -108.37500858898439, -109.65641721611547, -109.81905873737344, -108.03483220769625, -110.48028107566635, -108.60527372219985, -109.28768201151478, -99.8804125587218, -108.8913334544964, -108.23534920737794, -111.07646463287153, -108.59029790589766, -110.3405916586831, -107.66387718565608, -108.73793152614131, -110.61440166477816, -108.76211382544581, -110.23236978486065, -109.10669297094852, -109.15247609779597, -109.00539004923506, -110.14424353412238, -110.55445060661157, -109.48721312920799, -108.17040942305823, -108.77592227268228, -108.77130256578067, -107.82494496098512, -109.57266989523707, -108.75767497229612, -108.13688624150026, -107.8280716764963, -105.676279602552, -107.6370316684844, -109.73508547021689, -109.25365178573009, -108.86767843317584, -109.70969944273735, -108.91917504090888, -109.97734866522867, -112.17308993943783, -110.28356299479682, -110.7927103729386, -110.30837645846702, -107.56364161860179, -109.50188349731121, -109.36065627483853, -109.75389877587511, -109.81713476007774, -108.14524057525358, -109.43832376796216, -110.89342891210596, -108.15657882822792, -106.84106061627887, -107.83091759905821, -108.61794662682962, -109.57142366843581, -109.85402645528154, -110.12877022469837, -109.19414429724044, -110.56168468006764, -108.74720588273881, -107.90448559921305, -108.54421401507743, -105.06700039841249, -109.17937358052484, -108.94317576365822, -107.79410219455083, -109.24955437598658, -108.23334395173994, -108.98759227946937, -107.05986359444529, -107.20956512998849, -109.00295831471958, -109.43119556916457, -108.93348410522628, -108.99932477701081, -106.6448790859128, -109.06877251308666, -107.67053918439544, -109.15052780608639, -110.16878033319385, -106.55101141640301, -108.02811045752685, -111.52173447126572, -110.16854119242062, -110.93164036911654, -111.25979320890855, -108.82629030379024, -108.52004501839738, -107.09697056562636, -108.94233383169858, -107.37962568194772, -109.1239201710643, -108.93949898577122, -110.62573772949195, -110.09592372075662, -107.56136391005947, -110.45600430869621, -108.79481000016084, -109.41462449554598, -109.30248158488335, -108.70735295493108, -109.9174743694956, -109.94232543385962, -110.71725446170196, -110.0346196158573, -110.34814317845934, -110.6651078322521, -107.55409880424479, -108.71734776861287, -109.50902203986271, -110.40207542979611, -108.7847687630861, -111.10599488129682, -109.30824728923263, -108.20134064331717, -110.55959112431609, -107.77099734327174, -110.23862843385446, -108.48520797666865, -108.54205896654946, -107.79288769037599, -109.84022250170581, -108.02758364115576, -109.35132492327935, -108.87009749667932, -109.86905123364855, -109.19826752168308, -106.835240323691, -109.37910022114056, -110.80633973102931, -109.12703823829597, -111.07432699570984, -111.8064506085314, -110.09349947650527, -108.66467295777367, -108.75119108236053, -112.63983351316729, -110.90940743670113, -110.27973159222081, -109.57141664526549, -108.61645363771719, -109.31742355616147, -109.5839599160637, -110.01188998365383, -110.01923429741011, -108.94779759137936, -108.26169431000017, -109.24553201026085, -109.95709526422822, -110.68677343596859, -108.7678734483002, -110.47090469179284, -110.31604700116512, -110.10256600741997, -109.76634647265719, -110.8830805828562, -109.94609564072982, -109.20662382740542, -108.12492970530919, -110.5274435478767, -108.02351960398035, -110.6264936805739, -107.14559226383577, -109.13821777857531, -111.05324489472586, -110.15190797512811, -107.96366234783144, -110.03950681967147, -109.17476300510336, -110.41251816187909, -111.39219865477246, -111.32530426869943, -109.97369363558423, -108.98666403063845, -109.62049358645565, -109.58130494498671, -111.72738873188874, -110.39825891106616, -108.57430325757545, -111.28625510212446, -108.77421250595326, -109.75025415031793, -109.51948456745635, -108.82129398637998, -109.81362137198361, -107.86292494316123, -107.49318292857053, -109.66948564589373, -109.54288390056654, -107.99912445612077, -110.3497559614379, -108.00549349666127, -110.01361420523357, -108.4977916421456, -109.67078387286976, -109.85678367732866, -112.01237658746248, -108.4855625950998, -110.84880875737286, -110.9178674382154, -110.44187536727453, -108.75076921971127, -110.04946286646651, -109.99780941000827, -110.14242932305507, -109.56343773672316, -109.6278993388131, -108.77419573790174, -109.10543670530926, -109.7801848627463, -110.30733124104881, -113.13440550301436, -109.32709134514755, -109.74136656933283, -110.01525283266193, -109.43924662938396, -110.25325289253, -107.75460576671303, -110.60057027395933, -110.71458404922404, -110.15788509050662, -110.69167485018224, -110.96006652476157, -111.01156633983031, -111.6058448010008, -109.51364005052672, -109.76058205940885, -108.43421621088261, -109.47973949170208, -109.25533250208288, -109.47422603921065, -111.36411644613841, -107.27566171102698, -110.45098686173688, -109.93589296291184, -109.03803734663714, -110.53118128434016, -110.2408872254969, -110.0532234862915, -109.94185495614619, -110.2662004220774, -109.51094016962288, -108.5210104215432, -108.13691752270934, -110.18460088390265, -108.32609309150783, -109.89652230508281, -109.80923900768477, -109.01917388968883, -110.01248300968739, -109.43415605440147, -108.09823485138017, -107.40637725320931, -109.40632232658412, -111.97981999127656, -111.16609811629485, -111.64500793960192, -110.99793748693381, -109.55531276386903, -110.2535662621666, -108.17429802469516, -109.09425673355422, -110.23187110421917, -110.55358397926925, -109.93461124753053, -109.55604345832225, -109.44569510408274, -109.72185151080762, -109.52963702944834, -109.2303630328152, -109.74819502244243, -109.3932530349457, -109.17096788339686, -110.46153727064616, -113.1073731246639, -109.43753070459397, -108.13332547768168, -109.42294574929969, -108.45798401969856, -110.29453435046327, -112.66249403705643, -108.78314667434937, -105.9634478773668, -109.14327524669528, -108.50645190860273, -100.81571594994128, -104.4482859840643, -110.68926237051092, -109.12362553230196, -109.45234390564677, -107.91461416156068, -110.67788819353727, -110.05744935668449, -111.78333392154664, -106.83628914455993, -110.11115457346548, -109.13434608275826, -110.80006861194663, -110.35323502651462, -112.29149906501372, -109.01656376530778, -109.30871662948859, -109.79736315392456, -109.17848983603582, -108.09752397056482, -111.6039030763455, -109.27008844877828, -110.84475733314184, -109.72393917557073, -111.31060762894991, -110.78858793807466, -107.12841545099752, -109.54510865218204, -105.2805426080281, -106.28514149354733, -109.50656759582803, -110.14700878401054, -110.49737016725709, -109.19811547071924, -109.92527399676051, -110.7961615015146, -109.7447227818197, -109.49432012009893, -108.714081576733, -110.09766801550917, -109.08448507943001, -110.36154838733857, -109.86328656267403, -109.21144237434696, -112.4145136888034, -108.57567151011159, -109.66748589540896, -109.72985837578446, -109.29989238126763, -109.85868902806475, -111.01778182304162, -111.23625326328558, -110.01270868104203, -109.27067928081415, -109.71171312410247, -109.28697459293629, -110.67868067201007, -110.91353786857455, -111.21479955051575, -109.11315965407708, -109.40418681804496, -107.80511819596003, -107.37201025889816, -111.81969609169838, -109.89875624306032, -110.29328043898657, -109.74853280072202, -111.39527865400605, -109.47746221101964, -111.75141177452517, -109.31325306583483, -109.30117448911659, -109.3997781364162, -109.45356931295724, -109.60585285774386, -111.33951689512735, -107.74187210470228, -109.62706021606415, -108.72139655505221, -109.79552836110567, -110.64354037499807, -110.96138240913136, -110.02215059889615, -110.92978442698893, -110.0620778287114, -110.85019647293322, -111.77397403227091, -109.81257196800128, -109.15643451383403, -110.72777566469594, -108.7463769025616, -109.80959395914073, -111.24500986151126, -110.48863498350322, -110.30863780110901, -109.79331354195703, -110.34087081762074, -109.45183222569266, -109.6440990067103, -111.15034876658994, -112.14912485578341, -111.8886180186196, -110.57054820211916, -111.07556239924551, -110.5872832735073, -110.28912501038172, -108.91501133754849, -111.44575118962761, -109.90799859177967, -109.74421995550023, -108.70941446115883, -110.28822893097275, -109.70039554000401, -110.33701797570251, -110.79445894683306, -109.57694314608153, -108.816904416038, -109.66517126767175, -109.39501469321644, -110.85775022889956, -109.3689402795614, -112.09107318723095, -110.67985626248422, -110.32971146814747, -112.08166943494875, -109.93955548712543, -109.31722953035252, -110.2062913031861, -108.22565380081006, -110.680898028151, -111.95386604441454, -110.83354130587097, -108.5873626748948, -111.97536144124408, -109.23944159551515, -111.57859477689586, -110.80135186615524, -110.4800953731021, -110.14040729648133, -109.25873050390551, -108.87000960474569, -110.97091597211167, -110.15787270199012, -111.62434537618091, -108.5421625277294, -110.42258666403919, -110.96896115868603, -108.98253068925274, -109.54245055160168, -110.28051096122468, -109.48060498658319, -109.77618362117276, -111.64513838754992, -111.13945484239875, -110.18094280356001, -110.43757222770748, -110.81588360154201, -110.11656805555333, -108.47936291282355, -109.16476249859961, -109.3549985917136, -110.77753190334253, -111.46065694661178, -110.40387985996301, -109.95673803226478, -111.58660981285446, -108.59894875229345, -109.37333363882607, -110.26849699991793, -109.30500469266264, -109.23789020998296, -110.82000706486865, -109.25927538839868, -111.03285659417519, -111.08899832832414, -110.69361682858042, -109.45187168573815, -109.9614018482838, -109.70209527974106, -112.11903952100165, -109.59713611623246, -110.70292028698111, -110.12743849746808, -110.63315585514292, -108.60450276298175, -109.32832664986026, -109.99753023477764, -109.46644696130294, -109.1781290160558, -111.58830180575129, -111.67229040267557, -111.3750024136205, -108.33616679452298, -109.99797067800029, -110.50892429124391, -108.66074740829372, -111.17094662568759, -109.87538933985836, -109.152526628291, -110.44623159817101, -110.21603106403009, -110.64376935639365, -109.36897426842583, -108.67303022227141, -109.89327693080823, -111.50442955563923, -111.37532237834381, -109.38132821290205, -109.73509680539144, -110.53918379735906, -111.22869870340647, -109.39977573957616, -110.3674665334106, -110.5366125953241, -109.99025356764304, -109.97300035646616, -109.87631077033762, -109.64608829594286, -113.02486102973394, -108.26250283140733, -109.62234918138763, -111.18766216512655, -110.33666026406992, -110.5808115327039, -108.2971671321189, -110.10964334161903, -110.61254021379767, -109.89852549557533, -110.16562049054073, -109.41433790018287, -111.2453823439446, -110.45554802599901, -113.11454453784393, -110.7333866145056, -110.00858191882439, -108.54745315874294, -110.08430415376903, -111.9006972727596, -110.3031506154679, -110.26331790366497, -109.36797925566673, -109.04860552478912, -111.83514212681175, -111.38960737633833, -109.01429665187288, -110.96404839103826, -108.95488871107163, -109.09652004914592, -111.884304581971, -110.57566691021339, -111.95113404442795, -110.13677174050159, -108.10078686353354, -107.69442565416006, -112.42676605669463, -109.12681161784135, -109.23120766087519, -110.57649395555585, -110.22143082743162, -108.40065951773644, -109.46923168308618, -111.39095086729745, -110.46375658526013, -111.45145283328486, -112.22610823637353, -110.61090190564383, -112.22250292674809, -111.7379343196361, -110.18530386733481, -108.93867365671692, -111.89304844956082, -109.06146134986984, -110.98405731832798, -109.76366821333497, -108.08326795663608, -109.95041147835065, -112.94140614324155, -111.79814935135965, -108.07337559063119, -109.13733403265212, -111.74906646037496, -111.12228668433455, -110.02899450462209, -110.22237716929811, -109.0224776891049, -110.18135850497721, -113.32516073881047, -111.3576490243877, -110.60510094465171, -109.6935518470342, -110.36313473154901, -111.95933240129618, -109.49625308071019, -109.18827910216122, -110.54311407822692, -108.4811035913567, -112.81280225723607, -108.86530665787413, -110.85796435061886, -110.40059714639627, -108.19250716343407, -108.96956521802292, -108.61281798886506, -109.78061525370413, -111.58885511891798, -109.06279169160345, -111.43043988466789, -111.63169336321079, -109.54702536206447, -109.62860636296405, -109.47865811135546, -108.02265793654806, -109.97461304995515, -110.72549884050886, -111.57309413919933, -110.03317891949746, -110.39570411598524, -110.27606115470397, -110.63294457306095, -110.71821689302902, -110.38076268941819, -111.51223508887897, -110.40703572670697, -112.24933273737743, -109.74954300082398, -108.46020292937696, -111.05315219575881, -110.38635148390118, -109.58268303790976, -112.34211536832117, -108.45894118755307, -108.96463982695337, -110.56040438523046, -110.67803313671729, -111.07349872375121, -110.42184162876096, -111.82081126435692, -108.85923651136297, -112.57723799596502, -113.65690874668172, -112.62314325834605, -110.70357529341362, -110.959925221544, -111.26336183001875, -108.1350700630152, -107.94545932312926, -111.17610778209841, -110.20386728310686, -108.55646511121591, -109.8400922569145, -111.73466587035968, -110.47272877573613, -108.33011124048193, -107.93042857580332, -108.60928277989103, -109.25240966798974, -108.96403833602028, -106.94222615757475, -109.37086694261907, -106.72743097285155, -109.03160193412796, -107.3549903889451, -106.8543848510082, -107.83503929060929, -106.30745467433752, -108.36915807168845, -107.13065938379303, -107.84769200880969, -106.08004345082777, -108.15244601930225, -108.37254117816573, -106.57863034819223, -108.1283698227614, -108.19776505569902, -107.58283412238643, -108.17365133196301, -108.6794309781181, -107.91552140588759, -111.60122989270022, -107.04360635941174, -111.55535949001795, -109.39870426166594, -109.55937904851662, -111.81389508925734, -109.88957041098786, -110.84764586896561, -110.59130246272693, -111.15944135223884, -110.19496154041607, -111.51861903129362, -110.74798816525838, -111.37312965175558, -110.10842817220238, -110.73198099204856, -111.36708667993291, -110.30840247819665, -110.11744489669044, -110.55237850846444, -108.2073528237766, -112.70750856801911, -110.99917956040802, -109.84949484779976, -111.3403161887679, -110.08924435263565, -110.17749213365616, -112.10849123224503, -110.94270741299202, -109.29350963424746, -110.33477486966507, -112.19620157705627, -111.45484078395934, -111.86858843505124, -110.22491147345858, -108.96177661263177, -108.67862820579893, -107.55155410582937, -108.27984439169573, -108.72682528077233, -110.64231212183269, -109.32873093119183, -112.98564364754564, -110.78933114228725, -108.50921025910479, -107.91087245586935, -112.57350030929283, -111.75871577457525, -108.42095298945462, -112.31266064114303, -110.1295657579673, -109.67444664474456, -110.33749884929306, -109.16098218724147, -109.63554874360221, -109.15892392675141, -111.90580809179818, -108.81196712336858, -111.42223552606656, -109.90571484965518, -109.99739812086352, -111.64103850263211, -111.31463957090885, -110.61247447444549, -110.20960333715526, -110.1707327818923, -109.70412636554525, -110.97278093107532, -110.24386747740314, -109.81378546061525, -110.83784085086458, -109.77357954318757, -111.22663832948885, -111.14563050139252, -110.87152231402447, -110.34246044319893, -109.97174570657546, -110.23599592972218, -111.08206161770731, -110.0073315341242, -111.11748366902188, -112.04005964728601, -109.81290191679287, -109.68543639040858, -112.01143296194752, -110.13641850530031, -108.19348942447623, -109.7534468948808, -109.36697824644176, -97.56454580435337, -104.97829040517887, -108.1539132982256, -110.048991273122, -107.46172505860011, -110.49269280640675, -109.94209901400029, -109.38576869679022, -111.43699124347364, -110.89973083498887, -111.2994445418276, -109.25144782032437, -113.25676258473536, -110.82078737428088, -109.97779571182073, -113.36294799183014, -111.38584551238931, -112.17267897274873, -108.56430946159155, -112.06841286528645, -110.36822473102735, -109.54758527532016, -110.48190506674653, -110.03535695860182, -109.3951469796576, -112.41910682256774, -111.38124138857238, -109.37850389100952, -111.65544568836181, -111.55876881606889, -109.3029209617236, -109.20030046194076, -108.82610577621037, -110.53329453526098, -109.96090595542142, -109.67834229432077, -110.62303603007352, -109.8388817181171, -109.22430039793213, -108.92749786663613, -110.05794249283548, -109.58534943218437, -110.50493887507297, -109.96373022997366, -111.0645036323456, -111.28501675364454, -109.77386932343008, -108.8952247140968, -110.09242801628717, -112.90943444063141, -110.72299296247249, -109.39094335967056, -110.95165384057718, -109.59809519359453, -110.4978602309597, -109.67109981692639, -111.2489619905986, -110.0937750887109, -109.76771021128954, -108.32976315018955, -111.3058145792439, -111.09464974601362, -110.99797900696136, -109.174315000222, -109.630351559617, -110.26289147175856, -110.22688407202517, -109.96748050100612, -112.13247633583758, -110.59994952890855, -110.93023020153811, -109.22457750926695, -110.26162558926984, -110.09713110375579, -111.73858994918328, -109.78183160058515, -109.7603471824367, -110.96016892586911, -111.23309626937036, -109.83093663960678, -114.05354944347246, -111.58202863059464, -110.42281828744524, -110.9521484732059, -112.5120328206343, -111.614891937737, -109.84428787405484, -111.61119567831453, -110.43095563229411, -111.71833448430398, -110.01132196809407, -109.37558169247951, -109.14091380022785, -110.42663661754088, -110.3598013572826, -109.78207135281417, -109.94058843992468, -109.88210328447205, -108.6217811850147, -107.17834387173707, -110.6447226986756, -111.10704778101115, -111.24396771977769, -110.47849395539598, -110.75150631628034, -109.67662689396347, -109.23145032835053, -108.83780193265358, -109.43468321661163, -102.22521103859944, -106.90009867479111, -108.91580608784525, -109.58671397003187, -110.56692028436989, -108.75103142680105, -111.00795573084157, -110.75039085328763, -109.48222099288613, -111.8621134816908, -110.26507966786443, -108.885924716389, -109.30841399453053, -112.3188631425597, -111.05677697153163, -108.8268571902449, -109.63028152237679, -114.82339015806369, -107.03435216376964, -111.34847692589166, -109.61354114874855, -112.32687758049907, -109.59816404231358, -111.64248480241805, -111.84075757907273, -110.44017657636552, -110.15181635726277, -111.93813663582833, -109.11826378836209, -109.99779889778326, -109.927119030584, -109.4389650887841, -111.52448814187727, -111.38736268499642, -110.51920914917922, -108.64230614681055, -108.90307263595304, -110.57246891832371, -109.65575340646116, -109.80359672370373, -108.83368585528197, -111.09385004343437, -108.83430005497769, -112.37784208819113, -109.50005381621696, -109.67421750136593, -111.39664088797532, -109.70867599669316, -109.52498993629875, -111.12341349673187, -110.0484037026941, -109.55138667646308, -111.06614422098669, -109.4785941493091, -110.25724082617013, -110.93950616855716, -110.53487953881397, -111.45722057988401, -110.32393446412904, -110.34361936710438, -108.6610336097813, -109.53631603696368, -108.06930707969195, -107.68056561368934, -108.73860971027449, -108.87111384617579, -108.40433837098611, -110.55999576884835, -106.83832061167207, -108.28786975902513, -109.18482905697472, -107.81071696594883, -107.91047268802457, -108.79613111673706, -111.05361322310213, -109.97897453479862, -109.12920563729425, -111.20538391490288, -109.26286135293664, -111.31400407177502, -109.92167984752287, -110.70854322826071, -108.59406515713611, -109.69371333227458, -109.36664873267313, -110.35521729513704, -110.40667924006368, -112.0181844636846, -111.01529188207431, -110.59246505728431, -109.95068312717868, -110.75807466894047, -109.58596443762707, -111.12127793384956, -109.59041634463125, -111.56255571372793, -110.43405578864342, -108.39660324329928, -111.1420710307505, -113.64788483868595, -111.67645688353934, -111.36878760365944, -109.68523694561108, -110.11608766310304, -109.25670490330123, -110.73546181099229, -111.77855039399805, -107.9662794718261, -109.67483334602832, -109.891258579519, -110.24757768183042, -109.50202895993814, -110.07763831916637, -109.96891925839451, -110.97268925927641, -109.31698133827767, -112.27933593506792, -110.36206721075725, -109.47379463718867, -110.27836850941338, -110.63738280998388, -111.3611682777485, -110.72689155959884, -111.55480904927032, -111.16689658479412, -110.35555645743601, -111.56609319131051, -110.88279459952174, -114.73607246523177, -109.95813757295693, -107.64639932425493, -111.26486783320321, -112.03946356928121, -111.8915972448334, -110.35245920812773, -110.83155104803564, -110.67437747473863, -110.9959682920065, -110.7815352345103, -111.13722283763049, -112.54797265493127, -110.06894780898469, -111.65186554925783, -111.83545188116254, -110.65894756123697, -108.48458025065264, -112.43760714427981, -114.1368408201927, -110.40065777895025, -110.1066998945526, -108.60654239598591, -110.5716060205154, -110.74257357180736, -111.1136089342442, -111.53539811075092, -113.2559601458872, -109.2003227548348, -110.42285840441025, -111.4086884998834, -111.61503050693868, -110.8194303494779, -108.9701587059964, -112.58521089509063, -110.10873915265242, -112.43440038319561, -110.03468788439882, -111.57896603236308, -110.21939233582523, -109.03614470500777, -110.11738923539659, -109.55359574898291, -110.416473622654, -109.4626868574157, -111.17164025076731, -110.3579689035081, -109.04338716157822, -112.36157114517567, -109.32125615922843, -112.71105693789394, -110.11019129547768, -108.96439402555632, -111.107663418839, -111.48306369859839, -110.9317530461794, -107.98628540532181, -111.1636972328743, -110.47837837583148, -109.04649309175733, -110.27110334963734, -111.35803630614352, -110.77259078859605, -111.46352820533895, -111.16789261049541, -109.2376344776325, -111.6795794983659, -111.74292205167644, -109.40835022991612, -111.02163652600731, -108.79482078001607, -110.6718658416566, -111.08747067599332, -112.15383726791498, -109.47049126158717, -109.061574046483, -111.23993049318979, -111.02521156588335, -109.46012868444186, -110.13918914826291, -112.08180381836377, -110.61929875223015, -111.4424805369965, -111.43420275069585, -109.71347556238717, -110.24726273025648, -109.7860268673935, -109.94126895018422, -111.41948668868926, -108.90555991781676, -110.81242861886172, -109.65007052722677, -112.12672329335953, -110.01123170946096, -111.13980448279096, -113.92013682657084, -108.6000853867411, -110.66793592761913, -110.61237681642844, -110.00839105230496, -109.38083187034974, -109.46119372195675, -110.3708067287448, -108.55518656223285, -113.33935987443276, -111.92184778392033, -111.80820718236087, -107.36852757311246, -109.51077803361602, -110.066791721019, -108.756710558672, -107.91391289865918, -110.72851430959301, -111.39074956442978, -112.928843679455, -109.87348280521556, -112.21371750380071, -110.82495902297394, -109.94006136010094, -110.58757785050143, -110.2790091349881, -111.43884888223081, -108.09540986530712, -109.63783244641691, -110.19577975613292, -110.01690033746098, -112.75938920157155, -109.27158857362184, -111.19519821680541, -110.14381902425255, -110.45955291199236, -111.55660330002316, -110.75604254261134, -111.02122553784838, -111.6490091060193, -110.93362819419399, -110.49033159684308, -110.70789549836027, -110.41991882034145, -110.0264093421208, -109.18432746063652, -110.15292268755287, -112.40733942236504, -111.32869665965416, -110.95418667871114, -111.14291568823575, -111.75555369152653, -112.98146297069803, -109.73870744292117, -111.33806139459435, -110.18838799491355, -112.60408243005732, -110.26112648646833, -110.58257045107274, -109.75155437454112]}, ...(2 in all)]
  in  "FFT 1 Choice 1":u16(ring) items=["T1 Y", "T1 X", "T1 Sum", "T2 Y", "T2 X", "T2 Sum", "T1 FB X", "T1 FB Sum", "T2 FB X", "T2 FB Sum", "PSD Y", "PSD X", "PSD Y Sum", "none"]
  in  "FFT 2 Choice 1":u16(ring)=3 items=["T1 Y", "T1 X", "T1 Sum", "T2 Y", "T2 X", "T2 Sum", "T1 FB X", "T1 FB Sum", "T2 FB X", "T2 FB Sum", "PSD Y", "PSD X", "PSD Y Sum", "none"]
  in  "FFT 1 Choice 2":u16(ring)=1 items=["T1 Y", "T1 X", "T1 Sum", "T2 Y", "T2 X", "T2 Sum", "T1 FB X", "T1 FB Sum", "T2 FB X", "T2 FB Sum", "PSD Y", "PSD X", "PSD Y Sum", "none"]
  in  "FFT 2 Choice 2":u16(ring)=4 items=["T1 Y", "T1 X", "T1 Sum", "T2 Y", "T2 X", "T2 Sum", "T1 FB X", "T1 FB Sum", "T2 FB X", "T2 FB Sum", "PSD Y", "PSD X", "PSD Y Sum", "none"]
  in  "Compute FFT":bool
  in  "Reset FFT":bool
  in  "# Spectra to Ave.":dbl=25.0
  out "Ave. Time (s)":dbl=1.5
  out "1 Channel":waveform(dbl)(graph)={"t0"=timestamp(0 s since 1904-01-01), "dt"=1.4999999999999999e-05, "Y"=array[20000 elements], "attributes"=variant("NI_ChannelName"=variant(string "T1 Y"))}
  out "Slow mean":dbl=nan format="%0.2f"
  in  "Slow mean N ave.":dbl=1.0 min=1.0 step=1.0
  out "Mean Intensity":dbl=nan
  out "Sigma":dbl=nan
  out "Sigma/Mean":dbl=nan
  in  "Subtract mean":bool
  in  "High Res. Display":u16(ring) items=["T1 Y", "T1 X", "T1 Sum", "T2 Y", "T2 X", "T2 Sum", "T1 FB X", "T1 FB Sum", "T2 FB X", "T2 FB Sum", "PSD Y", "PSD X", "PSD Y Sum"]
  out "APD 1 Rate (Hz)":dbl format="%#_3p"
  out "Stage Moving":bool
  in  "Read Cal":bool
  in  "Confocal Linescan":bool
  in  "Speed (nm/s)":dbl=100.0
  in  "Furthest Withdraw (MHz)":dbl=15.0
  in  "Confocal Image":bool
  in  "Round T1 X":bool caption="Round"
  in  "T1 offset_x (mV)":dbl=nan format="%#_2g"
  in  "T1 kappa_x (pN/nm)":dbl=nan min=0.0 step=0.001 format="%#_2g"
  out "Time (s)":dbl=6.12
  out "Total Time (s)":dbl=60.0
  in  "Start Saving":bool
  in  "Cal sets to save":u32=50 min=1 step=1
  in  "Comment (data description)":string="testing confocal setup"
  out "Calibrating Trap...":bool
  in  "Trap 2 (ON/OFF)":bool=TRUE
  in  "Trap 1 (ON/OFF)":bool=TRUE
  in  "Save Calibration":bool
  in  "N sets to save":u32=200 caption="N Sets"
  in  "Save N Sets":bool
  out "Save file name":path=path "C:/Data/110526/110526_022.dat"
  in  "Save ave N":dbl=500.0 caption="Averaging Factor"
  out "Saving...":bool
  in  "Stop Saving":bool
  out "Progress":u16(slide) scale=0.0..100.0
  out "Manipulating Trap":bool
  out "Buffer Status":dbl(slide) scale=0.0..1.0
  out "Overflow (data lost)":bool
  in  "Reset":bool
  out "Data Rate (Hz)":dbl=66666.66666666667 caption="Trap Data Rate (Hz)" format="%#_3p"
  out "Data Period (s)":dbl=1.4999999999999999e-05 caption="Trap Data Period (s)" format="%#_6p"
  out "Save Data Rate (Hz)":dbl=133.33333333333334 caption="Rate (Hz)" format="%#_6p"
  out "Save Data Period (s)":dbl=0.0075 caption="Period (s)" format="%#_6p"
  in  "T1 alpha_x (nm/V)":dbl=nan step=10.0 format="%#_3g"
  in  "T2 alpha_x (nm/V)":dbl=nan step=10.0 format="%#_3g"
  in  "T2 kappa_x (pN/nm)":dbl=nan min=0.0 step=0.001 format="%#_2g"
  in  "T2 offset_x (mV)":dbl=nan format="%#_2g"
  in  "BD 1 Frequency 2 (MHz)":dbl=80.0 caption="T2 X (MHz)" min=50.0 max=100.0 step=1.0 format="%#_6p"
  in  "Green Laser ON/Interlacing":bool=TRUE
  in  "Round T2 X":bool caption="Round"
  in  "AO1":dbl(slide) caption="Confocal Y (V)" min=0.0 max=10.0 step=0.01 scale=0.0..10.0 scale format="%_1f"
  in  "AO2":dbl(slide) caption="Confocal X (V)" min=0.0 max=10.0 step=0.01 scale=0.0..10.0 scale format="%_1f"
  in  "Trap Raster Scan":bool
  out "Raster Scanning...":bool
  in  "Trap Delta (MHz)":dbl=20.0 step=1.0
  in  "Trap Intensity\nSetpoints (V)":cluster{"Set 1":dbl, "Set 2":dbl}={"Set 1"=5.2, "Set 2"=6.6}
  in  "Index":dbl=1.0 caption="Save File Index" min=1.0 step=1.0
  in  "BD 1 Frequency 1 (MHz)":dbl=65.0 caption="T1 X (MHz)" min=50.0 max=100.0 step=1.0 format="%#_6p"
  in  "Goto Top (F6)":bool
  in  "Save":bool
  in  "Capture":bool
  out "?":cluster{"x":string, "y":string, "z":string}={"x"="0.19233\r\n", "y"="0.00156\r\n", "z"="0.20615\r\n"}
  in  "Capture Locations":i32(listbox)=1
  out "X Pos":string="0.20503\r\n"
  out "Y Pos":string="0.00713\r\n"
  out "Z Pos Pos":string="0.21899\r\n"
  out "X Motion":string
  out "Y Motion":string
  out "Z motion":string
  in  "Goto Bottom (F7)":bool
  in  "Goto Exp (F8)":bool
  in  "Main:":bool caption="Inject Pump 3"
  in  "Inject Top:":bool caption="Inject Pump 1"
  in  "Shunt:":bool
  in  "Inject Bottom":bool
  out "Current Position":dbl[](array[numeric])=[4.2944, 4.91027471, 2.9278058] format="%7_7g"
  in  "Position Label 5":string="upper flow spot" caption="5"
  in  "Position 1 Label":string="Top capillary (SA beads)" caption="1"
  in  "Position 2 Label":string="Bottom capillary (AD) beads)" caption="2"
  in  "Position 3 Label":string="lower flow spot (ATP)" caption="3"
  in  "Position 4 Label":string="Dump beads" caption="4"
  out "Pump 3 cont disp":string="Left: ADig beads"
  out "Pump 1 cont disp":string="Right: DNA beads "
  in  "Ch 1 Inject Rate (ul/h)":dbl=50.0
  in  "Pump write delay (ms)":dbl=300.0
  in  "All Pump Parameters":T6={"Pump 1"={"Diameter (mm)"=4.61, "Units"=4.0, "Volume"=100.0, "Rate"=50.0}, "Pump 2"={"Diameter (mm)"=4.61, "Units"=3.0, "Volume"=0.0, "Rate"=0.0}, "Pump 3"={"Diameter (mm)"=4.61, "Units"=4.0, "Volume"=100.0, "Rate"=250.0}}
  in  "Ch 2 Inject Volume (uL)":dbl=100.0
  in  "Pump pause delay (ms)":u32
  in  "Ch 3 Inject Volume (uL)":dbl=100.0
  in  "Ch 3 Inject Rate (ul/h)":dbl=250.0
  in  "Flush Center Ch Volume (uL)":dbl=15.0
  in  "Flush Center Ch Rate (ul/m)":dbl=100.0
  in  "Inject Valve B":bool caption="Inject Pump 2\n(Flush Center)"
  in  "Total Volume\nFlushed (uL)":dbl
  in  "Tab Control 2":T7(tab)=enum."Feedback on Trap Intensity"
  in  "Restart RF":bool
  out "Total Counts (ticks)":u32=600
  in  "Trap ON/OFF X or Y Amp?":bool=TRUE
  in  "Oscillate Set 2":bool
  in  "Trap 1 ON":bool=TRUE
  in  "Number Interlace Sets":u8=3 min=1 max=3
  in  "DIO count 3 (ticks)":u32=200
  in  "DIO count 2 (ticks)":u32=200
  in  "DIO count 1 (ticks)":u32=200
  in  "BD 2 Amplitude 3 (%)":dbl min=0.0 max=75.0 step=1.0
  in  "BD 2 Amplitude 2 (%)":dbl min=0.0 max=75.0 step=1.0
  in  "BD 2 Amplitude 1 (%)":dbl min=0.0 max=75.0 step=1.0
  in  "BD 1 Amplitude 3 (%)":dbl min=0.0 max=75.0 step=1.0
  in  "BD 1 Amplitude 2 (%)":dbl=30.0 min=0.0 max=75.0 step=1.0
  in  "BD 1 Amplitude 1 (%)":dbl=30.0 min=0.0 max=75.0 step=1.0
  in  "BD 2 Frequency 3 (MHz)":dbl=26.0 min=50.0 max=100.0 step=1.0 format="%#_6p"
  in  "BD 1 Frequency 3 (MHz)":dbl=70.0 min=50.0 max=100.0 step=1.0 format="%#_6p"
  in  "BD 2 Frequency 2 (MHz)":dbl=26.0 min=50.0 max=100.0 step=1.0 format="%#_6p"
  in  "BD 2 Frequency 1 (MHz)":dbl=26.0 min=50.0 max=100.0 step=1.0 format="%#_6p"
  in  "Not-Interlacing Set":enum32{"Set 1", "Set 2", "Set 3"}(radio)
  in  "Interlace":bool=TRUE
  in  "Trap 2 ON":bool=TRUE
  in  "Trap 3 ON":bool
  in  "Scan axis 2":bool=TRUE
  in  "Osc. freq. (Hz)":dbl=0.25
  in  "Osc. amp. (MHz)":dbl=2.0 format="%1_3g"
  out "Coords":T8
  in  "Manipulation Scaling":cluster{"Horizontal":dbl, "Vertical":dbl}={"Horizontal"=0.075, "Vertical"=0.01}
  in  "Freq or Amp switch first":bool=TRUE
  in  "Swap F1 and F2":bool
  in  "Freq switch delay":u16
  in  "Amp switch delay":u16=5
  in  "Period":i64=2
  in  "MCL Step Increment (V_int)":dbl=3.0
  out "Time to Finish All (min)":dbl=0.122877 format="%#_2p"
  in  "Scan Speed (nm/s)":dbl=100.0
  in  "Scan Range (nm)":dbl=369.00000000000034
  in  "Step Size (nm)":dbl=1.0
  in  "MCL/AOM Scale Tweak":dbl=1.0
  in  "MCL Step Position Ratio":dbl=0.5
  in  "Move MCL Also?":bool=TRUE
  out "Final sep (nm)":dbl=4587.0
  out "Initial sep (nm)":dbl=4218.0
  out "Save index":dbl=22.0
  out "Final delta (MHz)":dbl=44.0
  out "Initial delta (MHz)":dbl=41.0
  out "Final freq. (MHz)":dbl=50.0
  out "Initial freq. (MHz)":dbl=53.0
  in  "Saved AOD Raster Scan Parameter Sets":T9(array[cluster])=[{"Scan Range AOD (nm) 2"=500.0, "Step Size AOD (nm) 2"=1.0, "Scan Speed AOD (nm/s) 2"=100.0, "Number of scans (AOD) 2"=1, "Label"="offset curve"}, {"Scan Range AOD (nm) 2"=420.0, "Step Size AOD (nm) 2"=1.0, "Scan Speed AOD (nm/s) 2"=100.0, "Number of scans (AOD) 2"=1, "Label"="hp raster check"}, {"Scan Range AOD (nm) 2"=6.8, "Step Size AOD (nm) 2"=0.34, "Scan Speed AOD (nm/s) 2"=0.34, "Number of scans (AOD) 2"=1, "Label"="3.4 kbp - 1 bp steps"}]
  in  "Load parameters":bool
  out "Scan Range (MHz)":dbl=-3.0000000000000027
  in  "Restart DMA? (AOD)":bool=TRUE caption="Restart DMA?"
  out "Incr. int (AOD)":i64=-7759651845
  out "Time/Scan (s) (AOD)":dbl=3.68631 format="%#_2p"
  out "Data points/scans":dbl=491508.0
  out "Data points/scan (f/b)":dbl=491508.0
  in  "Save scans":bool=TRUE
  out "AOD Scan I":u64 caption="Scan I"
  in  "Continuous AOD Scanning":bool caption="Continuous Scanning"
  in  "Abort AOD Scan":bool caption="Abort Scan"
  in  "Scan BD":bool=TRUE
  out "Cycles/step (AOD)":u64=666 format="%.3p"
  in  "Number of F/B Scans (AOD)":u16=1 min=1
  out "Scan steps (AOD)":u64=369
  out "Scan Increment (MHz)":dbl=-0.008152173913043485
  out "AOD Scanning":bool caption="Scanning"
  in  "Start AOD Scan":bool caption="Start Scan"
  out "N sets should be saved":dbl=24.5754
  out "Progress 2":u16(slide) caption="Progress" scale=0.0..100.0
  in  "Abort save 2":bool caption="Abort save"
  in  "Trap 1 Bead Size (nm)":dbl=2100.0
  in  "Trap 2 Bead Size (nm)":dbl=2100.0
  out "MCL Count":dbl=230502201.82069838
  in  "All FB On/Off":bool
  in  "AI2 to Setpoint":cluster{"Set 1":bool, "Set 2":bool}
  out "AI2 (V)":cluster{"Set 1":dbl, "Set 2":dbl}={"Set 1"=-0.0012207403790398877, "Set 2"=0.004577776421399579}
  in  "Reset Feedback":cluster{"Set 1":bool, "Set 2":bool}
  in  "PID Gains":T10={"Set 1"={"proportional gain (Kc)"=0, "integral gain (Kc*Ts/Ti)"=5, "derivative gain (Kc*Td/Ts)"=0}, "Set 2"={"proportional gain (Kc)"=0, "integral gain (Kc*Ts/Ti)"=5, "derivative gain (Kc*Td/Ts)"=0}}
  in  "Feedback On/Off":cluster{"Set 1":bool, "Set 2":bool}={"Set 1"=TRUE, "Set 2"=TRUE}
  in  "Reset Trap Pos. FB":bool
  in  "Tab Control 8":enum32{"Main Setting", "Details"}(tab)
  in  "Trap Pos FB Int Count":u16=100
  in  "Trap Pos. FB Gains":T11={"proportional gain (Kc)"=10.0, "integral gain (Kc*Ts/Ti)"=10.0, "derivative gain (Kc*Td/Ts)"=0.0} {"proportional gain (Kc)" format="%.11g"; "integral gain (Kc*Ts/Ti)" format="%.11g"; "derivative gain (Kc*Td/Ts)" format="%.11g"}
  in  "Trap Pos. FB Offset Factor":i64
  in  "Trap Pos FB Negate Action":bool
  in  "Trap Pos. FB Mult Factor":i64=33554432
  in  "Trap Pos. AI1 X Pre-scale":u16
  in  "Trap Pos. FB Range":T12={"output high"=0.999969482421875, "output low"=-1.0}
  out "Trap Pos FB Int Signal":fxp<+/-,24,9> format="%.18g"
  out "Trap Pos FB Int-Norm Signal":fxp<+/-,16,1> format="%.16g"
  in  "Set SP Using...":bool
  in  "Trap Pos FB Monitor\nT1 or T2":bool
  out "Trap X AI1 (DMA)":T13={"Set 1"=0.999969482421875, "Set 2"=0.999969482421875}
  in  "N El. to Ave.":dbl=10000.0
  out "Trap Pos FB Action":i64
  out "Mean T1 Position (nm)":dbl=-1.7479351299698465e-12 caption="Mean T1 (nm)" format="%0.2f"
  out "Trap 1 Position RMS (A)":dbl caption="RMS (Ang)"
  in  "Tab Control 3":enum32{"Timing", "MCL Scan", "Analog Out"}(tab)
  out "APD 2 Gate Late Counter":u32
  out "APD 2 Gate Relative Phase":i16
  in  "Phase Adj. (APD 2 Gate)":i16=20
  in  "Initial Phase Adjustment (APD 2 Gate)":i16=55
  out "APD 1 Gate Late Counter":u32
  in  "- phase (APD 1 Gate)":bool
  in  "+ phase (APD 1 Gate)":bool
  out "APD 1 Gate Relative Phase":i16
  in  "Phase Adj. (APD 1 Gate)":i16=20
  in  "Initial Phase Adjustment (APD 1 Gate)":i16=60
  in  "Save APD Data\nwith Trap Data":bool=TRUE
  out "APD FIFO Elements Remaining":u32
  in  "- phase (APD Acq)":bool
  in  "+ phase (APD Acq)":bool
  out "APD Acq Late Counter":u32
  out "APD Acq Relative Phase":i16
  in  "Phase Adj. (APD Acq)":i16=20
  in  "Initial Phase Adjustment (APD Acq)":i16
  in  "Invert APD Gate":bool caption="Invert Gate"
  in  "APD Gate OFF Count":u32=450 caption="Gate OFF Count"
  in  "APD Gate ON Count":u32=150 caption="Gate ON Count"
  in  "APD Gate":enum32{"ON", "OFF", "Interlace"}(radio)=enum."Interlace"
  in  "APD Integration Time (s)":dbl=0.01 caption="Integration Time (s)"
  out "APD Acq Rate (Hz)":dbl=100.0 caption="Rate (Hz)"
  out "APD Samples/FIFO Acq.":dbl=30.0
  out "APD Elements/DMA read":u32=60
  out "APD Int. Count":u32=400000 format="%.0p"
  in  "+ phase (APD 2 Gate)":bool
  in  "- phase (APD 2 Gate)":bool
  in  "Tab Control 5":enum32{"PSD X", "PSD Y", "Other Data Channel"}(tab)
  out "Data map":dbl[][](graph)
  in  "Channel":i32=4
  in  "Abort MCL Scan":bool
  out "MCL Scan I":u64
  out "MCL Scanning":bool
  in  "Start MCL Scan":bool
  out "wait to reset values":bool
  in  "Tab Control 4":enum32{"Scan Settings", "MCL FPGA Loop Timing"}(tab)
  out "Total Time (s)":dbl=48.0
  in  "Scan lines (y)":u64=20
  in  "Fast Scan Dir":bool=TRUE
  in  "2D or 1D Scan":bool=TRUE
  out "Initial X":dbl
  out "Initial Y":dbl
  out "Time/f+b scan (s) (MCL)":dbl=2.4 caption="Time/scan (s)"
  in  "Number of scans (MCL)":u64=1 caption="Scans"
  in  "Scan steps (MCL)":u64=40 caption="Scan steps (x)"
  in  "N APD Samp/step":dbl=3.0
  in  "Scan Range (V)\n(of steps)":dbl=3.5
  in  "Restart DMA? (MCL)":bool=TRUE caption="Restart DMA?"
  in  "Continuous MCL Scanning":bool caption="Cont. Scanning"
  in  "Center Scan":bool=TRUE
  in  "Save Data (MCL)":bool=TRUE caption="Save Data"
  out "Actual Incr. int (MCL)":i16=294 caption="Incr. int"
  out "Desired incr (int)":dbl=294.0628205128205
  out "Desired Scan Incr (V)":dbl=0.08974358974358974
  out "N sets should be saved (MCL)":dbl=160.0 caption="N sets should be saved"
  out "Data points/scans (MCL)":dbl=4800.0 caption="Data points/scans"
  out "Data points/scan (f+b)":dbl=240.0 caption="points/scan (f+b)"
  out "Cycles/step (MCL)":u64=2000 caption="Cycles/step" format="%.0p"
  out "Actual MCL Inc (V)":dbl=0.08972441785943175
  in  "Phase adjust (MCL)":i16 caption="Phase adjust"
  out "Relative Phase (MCL)":i16 caption="Relative Phase"
  in  "Initial Phase Adj. (MCL)":i16 caption="Initial Phase Adj."
  in  "Update Count (MCL)":u32=600
  in  "+ phase (MCL)":bool
  in  "- phase (MCL)":bool
  out "MCL Late Counter":u32
  in  "APD 1 AO Mult.":i16=1 min=1
  in  "APD 2 AO Mult.":i16=1 min=1
  in  "Tab Control 7":enum32{"Green FB Signals", "Slow MCL Scan"}(tab)
  out "Green FB Plot":dbl(graph)=10.0
  out "MCL Scan 2":cluster{"Begin (V)":dbl, dbl, dbl[]}(graph)
  out "MCL Scan":cluster{"Begin (V)":dbl, dbl, dbl[]}(graph)
  in  "Green laser mode":enum32{"Laser ON", "Laser OFF", "Interlace"}(radio)
  in  "GI Frequency, ON count":u32=150 min=1 step=1
  in  "Invert GI":bool
  out "GI Late Counter":u32
  in  "Phase adj. (GI)":i16=5
  out "GI relative phase":i16
  in  "+ phase (GI)":bool
  in  "Initial Phase Adjustment (GI)":i16=19
  in  "GI Frequency, OFF count":u32=450 min=1 step=1
  in  "- phase (GI)":bool
  out "Green FB Signals (V)":cluster{"Y":dbl, "X":dbl, "Sum":dbl}={"Y"=1.0, "X"=1.0, "Sum"=10.0}
  out "Relative phase (Green FB)":i16
  in  "+ phase (Green FB)":bool
  in  "- phase (Green FB)":bool
  in  "Green FB Count":u32=600
  in  "Phase adj. (Green FB)":i16=10
  in  "Initial Phase Adjustment (Green FB)":i16=50
  in  "Green FB On/Off":bool
  in  "Current When FB OFF (%)":dbl=10.0 min=0.0 max=100.0 step=1.0
  in  "Green int current ON count adj":u32=150
  in  "Green FB Gains":T14={"proportional gain (Kc)"=10, "integral gain (Kc*Ts/Ti)"=5, "derivative gain (Kc*Td/Ts)"=0}
  in  "Green FB Setpoint (mV)":dbl=100.0
  in  "- phase (GI) 2":bool
  in  "Initial Phase Adjustment (GI) 2":i16=-100
  in  "+ phase (GI) 2":bool
  out "GI relative phase 2":i16
  in  "Phase adj. (GI) 2":i16=20
  out "GI Late Counter 2":u32
  in  "Trap Position FIFO Depth":u32=300000 format="%.0p"
  in  "# Samples/trap":u32=20000 format="%.0p"
  out "Trap AI Elements/DMA read":u32=320000 format="%.0p"
  out "Ave. Rate (Hz)":dbl=200000.0 format="%#_6p"
  out "Trap AI FIFO El. Rem.":u32 format="%.0p"
  in  "Phase adj. (AI1)":i16
  out "Relative phase (AI1)":i16
  in  "+ phase (AI1)":bool
  in  "- phase (AI1)":bool
  out "Late Counter (AI1)":u32
  in  "Initial Phase Adjustment (AI1)":i16=180
  out "AI rate (Hz)":dbl=200000.0 format="%#_6p"
  in  "AI Count (ticks)":u32=200
  out "# Samples/channel":u32=40000 format="%.0p"
  in  "Trap AI FIFO Depth":u32=340000 format="%.0p"
  in  "Detector Type":string(combo)="UCB Fleezers 052511"
  in  "N Acq Sets (Traps + Fl.)":i16=3
  in  "Sets to FIFO (Traps)":T15={"Set 1"=TRUE, "Set 2"=TRUE, "Set 3"=FALSE}
  in  "FPGA Ave.":dbl=1.0 min=1.0 step=1.0
  out "Ave. Period (s)":dbl=5e-06 format="%#_6p"
  out "DMA Update Period (s)":dbl=0.3
  out "FPGA Averaging":bool
  out "Trap Sets":u32=2
  out "Counts/DMA":dbl=12000000.0 format="%#_6p"
  out "Trap Pos FIFO El Remaining":u32=141
  out "Trap Pos Elements/DMA read":u32=120000 format="%.0p"
  out "Trap AI FIFO Timeout":u16
  out "Trap Pos FIFO Timeout":u16
  out "Waveform Chart":i32(graph)=320000
  out "error out 2":errorcluster
  in  "Lost Tether Alarm Threshold (pN)":dbl=0.5
  in  "AOM X Cal (nm/MHz)":dbl=168.33
  in  "MCL X Cal (nm/V)":dbl=1070.0
  out "X RF Amplitude Limits (%)":T16={"Minimum"=0.0, "Maximum"=50.0, "Increment"=1.0}
  out "X RF Frequency Limits (MHz)":T16={"Minimum"=50.0, "Maximum"=100.0, "Increment"=1.0}
  out "Y RF Frequency Limits (MHz)":T16={"Minimum"=50.0, "Maximum"=100.0, "Increment"=1.0}
  out "Y RF Amplitude Limits (%)":T16={"Minimum"=0.0, "Maximum"=50.0, "Increment"=1.0}
  in  "Manip. X?":bool=TRUE
  in  "Manip. Y?":bool
  in  "Force Manip Abort":bool
  out "Read cal error":errorcluster
  in  "DAQ Delay (ms)":u32=1000
  in  "Start Scan":bool
  in  "Scan axis":bool
  in  "Osc. amp. (V)":dbl=5.0
  in  "Osc. center (V)":dbl=5.0
  in  "Osc. freq. (Hz) 2":dbl=1.0
  in  "MCL Mode":u16(ring) items=["Manual Positioning", "Sinusoidal Wave", "Linear Scan"]
  in  "Begin (V)":dbl
  in  "End (V)":dbl=10.0
  in  "N Points":dbl=20.0
  in  "Delay to Interlace (s)":dbl
  in  "Delayed Interlace Start":bool
  in  "Read Lateness and Rel Phase":bool
  out "Vec Mean of T1 T2":dbl[](array[numeric])=[nan, nan]
  in  "Cal read wait (s)":u32=5
  out "Time tether formed":timestamp=timestamp(3371146929.513132 s since 1904-01-01)
  in  "Chemyx Syringe Pump Serial Port":refnum<visa-resource-name>="ASRL3::INSTR"
  in  "Limit Min (MHz)":dbl=10.0 caption="Min (MHz)"
  in  "Limit Max (MHz)":dbl=16.0 caption="Max (MHz)"
  in  "Limits Enable":bool=TRUE caption="Enable"
  out "AI labels":string[](array[string])=["T1 Y", "T1 X", "T1 Sum", "T2 Y", "T2 X", "T2 Sum", "T1 FB X", "T2 FB Sum", "T2 FB X", "T2 FB Sum", "PSD Y", "PSD X", "PSD Sum"]
  in  "Save Trap Pos. Data":bool=TRUE
  in  "ESP Port":refnum<visa-resource-name>="COM4"
  in  "Axis 3":string="0.00500\r\n"
  in  "Axis 2":string="0.00500\r\n"
  in  "Axis 1":string="0.00500\r\n"
  in  "Axis 3":string="0.20000\r\n"
  in  "Axis 2":string="0.20000\r\n"
  in  "Axis 1":string="0.20000\r\n"
  in  "Activate Joystick":bool
  in  "ESP ZL-Limit":string="-0.09900"
  in  "ESP ZR-Limit":string="0.09900"
  in  "error in":errorcluster
  out "error out":errorcluster
  # "Save Positions of Cambers"
  # "After"
  # "During"
  # "Trap On?"
  # "BD Flow ON?"
  # "Samp Flow ON?"
  # "1"
  # "2"
  # "Trap Display:"
  # "APD Display:"
  # "originally 10k"
  # "Data Saving"
  # "Trap Manipulation"
  # "DAQ"
  # "Central frequency 80 MHz"
  # "F9"
  # "F10"
  # "Bead Calibration"
  # "Current Location"
  # "Select the chamber to go to"
  # "F4"
  # "Press F12 to move stage\nwith the mouse. F12 to cancel."
  # "F5"
  # "F6"
  # "F7"
  # "F8"
  # "Harvard Pump\n(sample channel for flow exp)"
  # "Chemyx Pump 2"
  # "Units: \n1 = ml/m\n2 = ml/h\n3 = ul/m\n4 = ul/h"
  # "Rate param is ul/h\nVolume param is ul"
  # "X"
  # "Y"
  # "Oscillate Set 2 freq. (debugging)"
  # "BD 1"
  # "BD 2"
  # "AOD Raster Scan"
  # "Approx. trap separations"
  # "X"
  # "Y"
  # "DON'T TURN ON\nUNTIL YOU CLOSE\nTHE LOOP"
  # "FPGA\nreading"
  # "DMA\ntransfer"
  # "APD Gates"
  # "APD 2"
  # "APD 1"
  # "X"
  # "2D"
  # "Y"
  # "1D"
  # "Green FB Measurement"
  # "Green Laser Interlacing"
  # "Digital Gate"
  # "Current Analog Control"
  # "was 87"
  # "originally 600k"
  # "Total AI Rates (NOT rates/trap)"
  # "originally 20k"
  # "(Samples/trap x Trap Sets)"
  # "(Samples/channel x\n8 if averaging (8 channels)\n4 if no averaging)"
  # "Trap 1"
  # "Trap 2"
  # "Flour./Trap 3"
  # "External Video Window"
  # "MCL Position Debugging"
  # "Temporary Control Storage\n(these used to be somewhere else, still want to keep them)"
  # "Y"
  # "X"
  # "Trap Position Difference Limits"
  # "Joystick Control"
  # "Setting Limit for the z-axis"
  # "Errors detected in determing Current Location"
  # "High Jog Velocity"
  # "Low Jog Velocity"
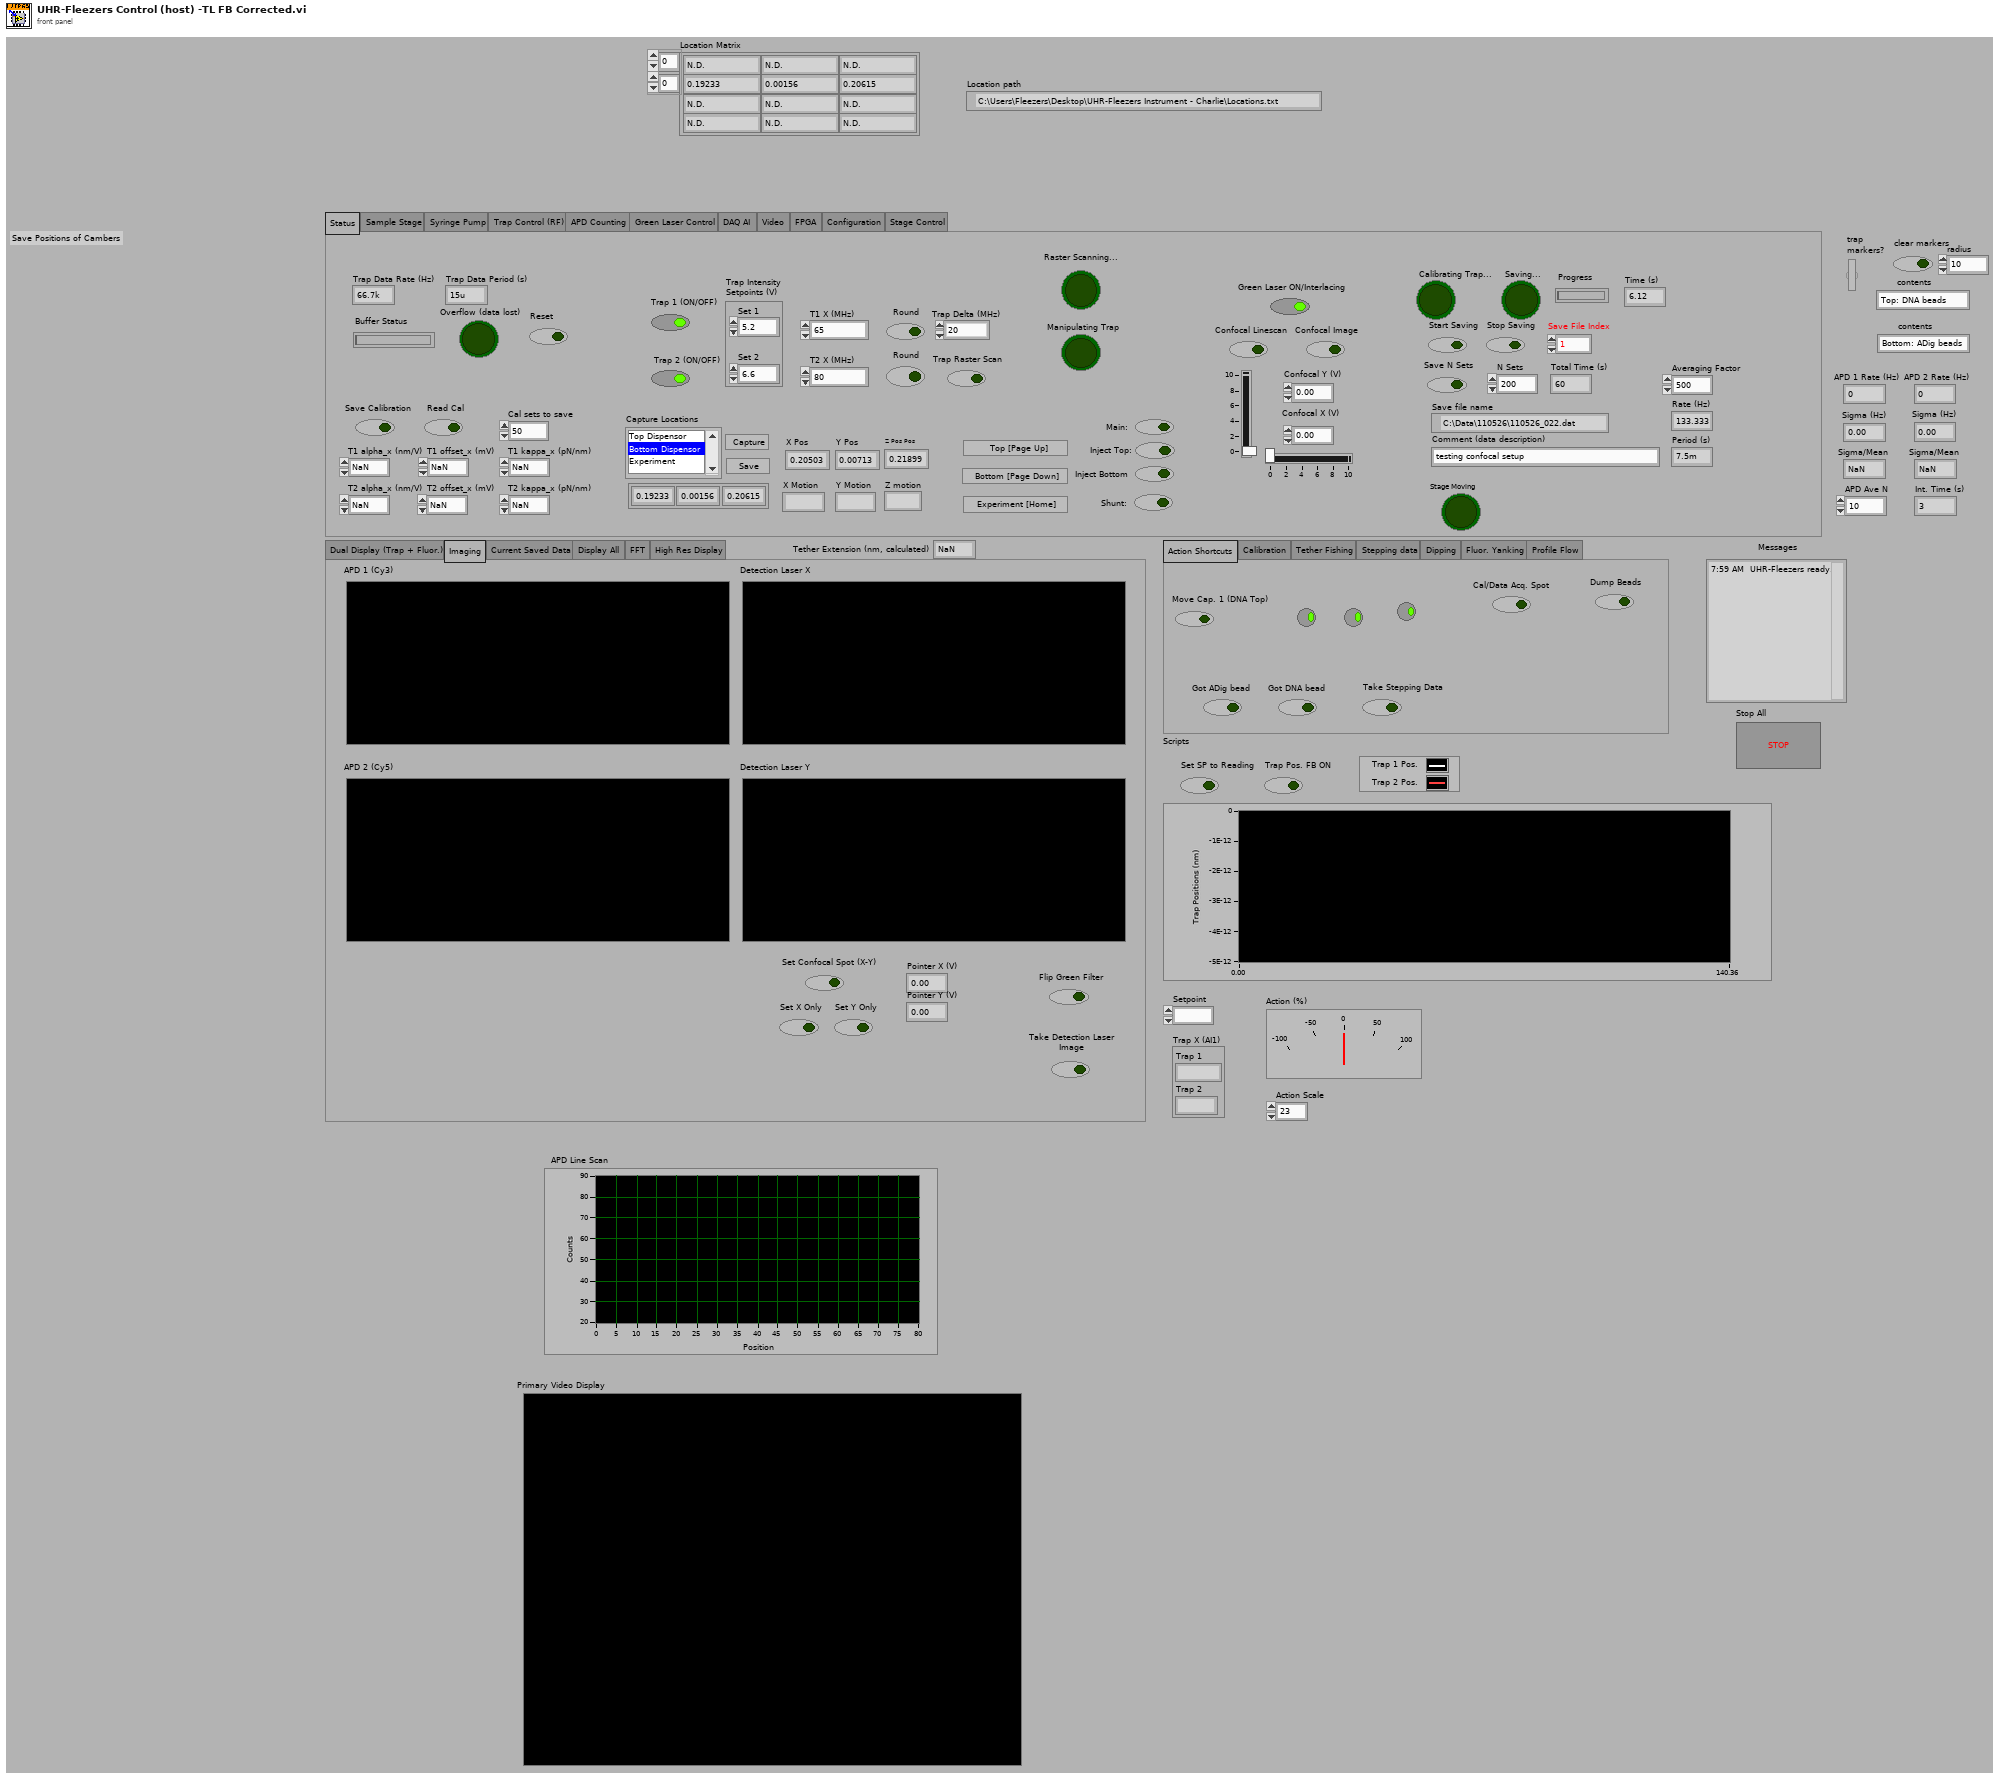
[diagram p1: front panel]
types:
  T1 = cluster{"Trap 1":fxp<+/-,16,1>, "Trap 2":fxp<+/-,16,1>}
  T2 = enum32{"Action Shortcuts", "Calibration", "Tether Fishing", "Stepping data", "Dipping", "Fluor. Yanking", "Profile Flow"}
  T3 = typedef "IMAQ Image.ctl" = refnum<image>
  T4 = enum32{"Dual Display (Trap + Fluor.)", "Imaging", "Current Saved Data", "Display All", "FFT", "High Res Display"}
  T5 = enum32{"Status", "Sample Stage", "Syringe Pump", "Trap Control (RF)", "APD Counting", "Green Laser Control", "DAQ AI", "Video", "FPGA", "Configuration", "Stage Control"}
  T6 = cluster{"Pump 1":cluster{"Diameter (mm)":dbl, "Units":dbl, "Volume":dbl, "Rate":dbl}, "Pump 2":cluster{"Diameter (mm)":dbl, "Units":dbl, "Volume":dbl, "Rate":dbl}, "Pump 3":cluster{"Diameter (mm)":dbl, "Units":dbl, "Volume":dbl, "Rate":dbl}}
  T7 = enum32{"IR Laser Interlacing (Direct RF Board Control Method)", "AOD Raster Scan", "Feedback on Trap Intensity", "Feedback on Trap Position"}
  T8 = typedef "LVPoint32TypeDef.ctl" = cluster{"Horizontal":i32, "Vertical":i32}
  T9 = cluster{"Scan Range AOD (nm) 2":dbl, "Step Size AOD (nm) 2":dbl, "Scan Speed AOD (nm/s) 2":dbl, "Number of scans (AOD) 2":u16, "Label":string}[]
  T10 = cluster{"Set 1":cluster{"proportional gain (Kc)":i16, "integral gain (Kc*Ts/Ti)":i16, "derivative gain (Kc*Td/Ts)":i16}, "Set 2":cluster{"proportional gain (Kc)":i16, "integral gain (Kc*Ts/Ti)":i16, "derivative gain (Kc*Td/Ts)":i16}}
  T11 = cluster{"proportional gain (Kc)":fxp<+/-,16,8>, "integral gain (Kc*Ts/Ti)":fxp<+/-,16,8>, "derivative gain (Kc*Td/Ts)":fxp<+/-,16,8>}
  T12 = cluster{"output high":fxp<+/-,16,1>, "output low":fxp<+/-,16,1>}
  T13 = cluster{"Set 1":fxp<+/-,16,1>, "Set 2":fxp<+/-,16,1>}
  T14 = cluster{"proportional gain (Kc)":i16, "integral gain (Kc*Ts/Ti)":i16, "derivative gain (Kc*Td/Ts)":i16}
  T15 = cluster{"Set 1":bool, "Set 2":bool, "Set 3":bool}
  T16 = typedef "LVMinMaxIncTypeDef.ctl" = cluster{"Minimum":dbl, "Maximum":dbl, "Increment":dbl}
  T17 = typedef "Image Type" = u32
  T18 = typedef "nirio_resource_hc.ctl" = tag
  T19 = typedef "openfpgaref.8.6.ctl" = refnum<k20>
  T20 = enum16{"CONNECT", "INITIALIZE VALVES", "DISCONNECT", "MOVE VALVE"}
  T21 = cluster{"New Image":T3, "New Image":T3, "New Image":T3, "New Image":T3}
  T22 = cluster{"Location Matrix[0]":string, "Location Matrix[1]":string, "Location Matrix[2]":string}
  T23 = enum16{"open", "replace", "create", "open or create", "replace or create", "replace or create with confirmation"}
  T24 = typedef "XDNodeRunTimeDep.lvlib/timing_clust.ctl" = cluster{"Expected End [f-1]":u64, "Actual End [f-1]":u64, "Finished Late? [f-1]":bool, "Expected End [i-1]":u64, "Actual End [i-1]":u64, "Finished Late? [i-1]":bool, "Expected Start [i]":u64, "Actual Start [i]":u64, "Expected Start [f]":u64, "Actual Start [f]":u64, "Source Name":string, "Structure Name":string, "Period":i64, "Deadline":i64, "Offset":i64, "Start":i64, "Priority":i32, "Timeout":i32, "Mode":T25, "Wakeup Reason":T26, "Error":errorcluster, "Source Type":string, "Secondary Source Type":string, "Global End Time":u64, "Global Start Time":u64, "Frame Duration":u64, "Iteration Duration":u64, "Assigned CPU":i32, "I/O Scan Engine Mode":u32}
  T25 = typedef "XDNodeRunTimeDep.lvlib/nitl_modes.ctl" = enum32{"No Change", "Process missed periods, maintain original phase", "Discard missed periods, maintain original phase", "Process missed periods, ignore original phase", "Discard missed periods, ignore original phase"}
  T26 = typedef "XDNodeRunTimeDep.lvlib/wakeup.ctl" = enum32{"Normal", "Aborted", "Asynchronous wakeup", "Timing source error", "Timed loop error", "Timeout"}
  T27 = cluster{"[0]":i32, "[1]":i32, "[2]":i32, "[3]":i32}
  T28 = cluster{"[0]":i32, "[1]":i32, "[2]":i32, "[3]":i32}[]
  T29 = enum16{"big-endian, network order", "native, host order", "little-endian"}
  T30 = cluster{"Scan Range AOD (nm) 2":dbl, "Step Size AOD (nm) 2":dbl, "Scan Speed AOD (nm/s) 2":dbl, "Number of scans (AOD) 2":u16, "Label":string}
  T31 = cluster{"[0]":dbl, "[1]":dbl, "[2]":dbl, "[3]":dbl, "[4]":dbl, "[5]":dbl}
  T32 = cluster{"Diameter (mm)":dbl, "Units":dbl, "Volume":dbl, "Rate":dbl}
  T33 = cluster{"Left":i32, "Top":i32, "Width":u32, "Height":u32}
  T34 = cluster{cluster{"Left":i32, "Top":i32, "Width":u32, "Height":u32}}[]
  T35 = enum32{"Normal Display", "Dual Display (APD)", "FFT", "High Res Display"}
  T36 = cluster{"Origin Pixel":cluster{"X":sgl, "Y":sgl}, "Angle Relative to Horizontal (deg)":sgl, "Axis Reference":u32}
  T37 = typedef "Simple Grid Descriptor" = cluster{"X Step":sgl, "Y Step":sgl, "Unit":T38}
  T38 = typedef "Image Unit" = enum32{"Undefined", "Angström", "Micrometer", "Millimeter", "Centimeter", "Meter", "Kilometer", "Microinch", "Inch", "Feet", "Nautical miles", "Standard miles", "Steps"}
  T39 = cluster{"averaging mode":u16, "weighting mode":u16, "number of averages":u32}
  T40 = cluster{"dB On (F)":bool, "unwrap phase (F)":bool, "convert to degree (F)":bool}
  T41 = cluster{string, string, string, string, string, string, string, string}
  T42 = cluster{string, string, string, string, string, string, string, string, string, string, string, string}
  T43 = cluster{string, string, string, string, string, string, string, string, string, string, string, string, string}
  T44 = cluster{string, string, string, string, string, string, string, string, string, string, string, string, string, string}
  T45 = cluster{"BD 1 Frequency 1 (MHz)":dbl, "BD 1 Frequency 2 (MHz)":dbl}
  T46 = cluster{"f0":dbl, "df":dbl, "magnitude":dbl[]}[][]
  T47 = cluster{"Green FB Ch 0":i16, "Green FB Ch 1":i16, "Green FB Ch 2":i16}
  T48 = cluster{"Green FB Ch 0":dbl, "Green FB Ch 1":dbl, "Green FB Ch 2":dbl}
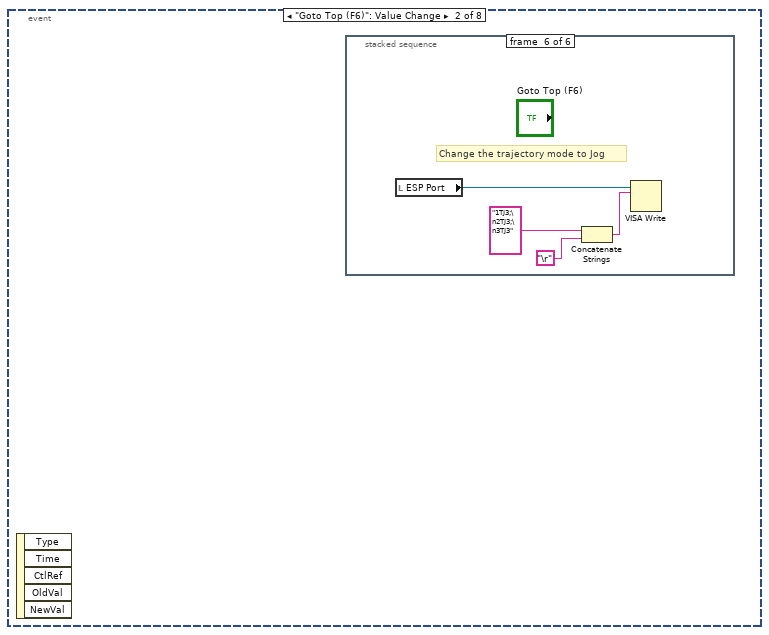
[diagram p4: hidden frame]
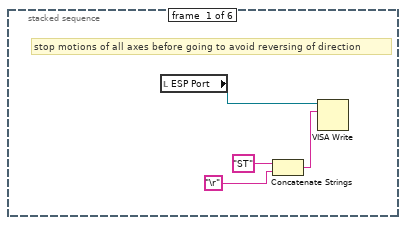
[diagram p5: hidden frame]
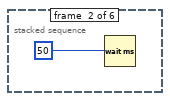
[diagram p6: hidden frame]
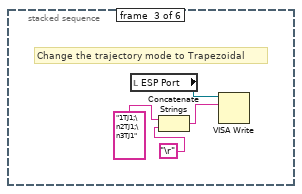
[diagram p7: hidden frame]
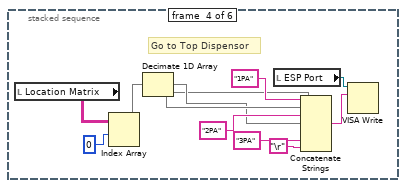
[diagram p8: hidden frame]
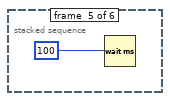
[diagram p9: hidden frame]
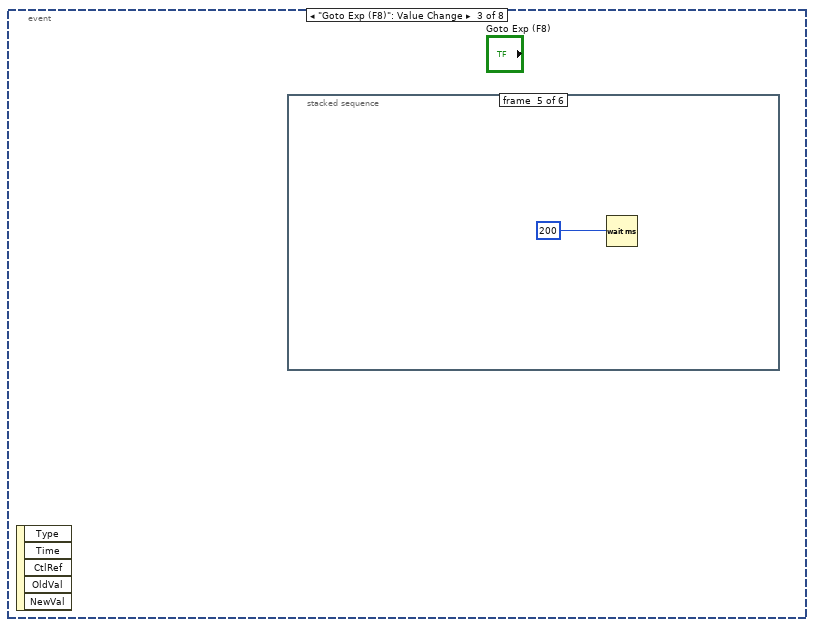
[diagram p10: hidden frame]
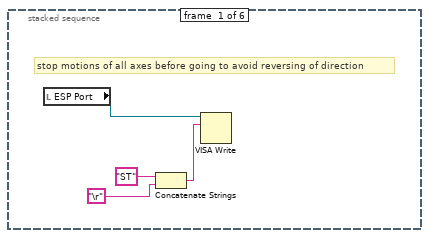
[diagram p11: hidden frame]
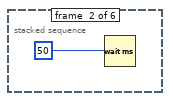
[diagram p12: hidden frame]
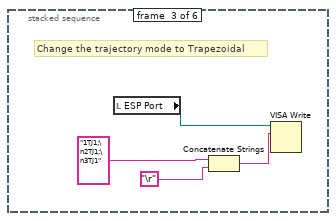
[diagram p13: hidden frame]
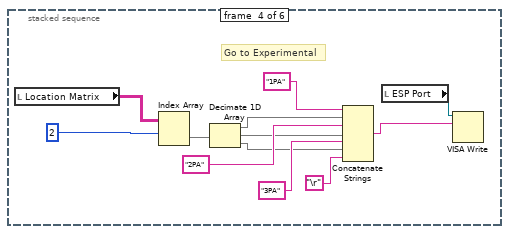
[diagram p14: hidden frame]
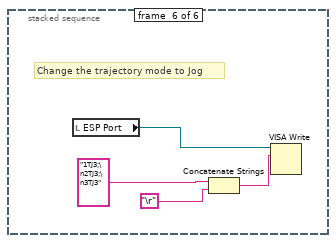
[diagram p15: hidden frame]
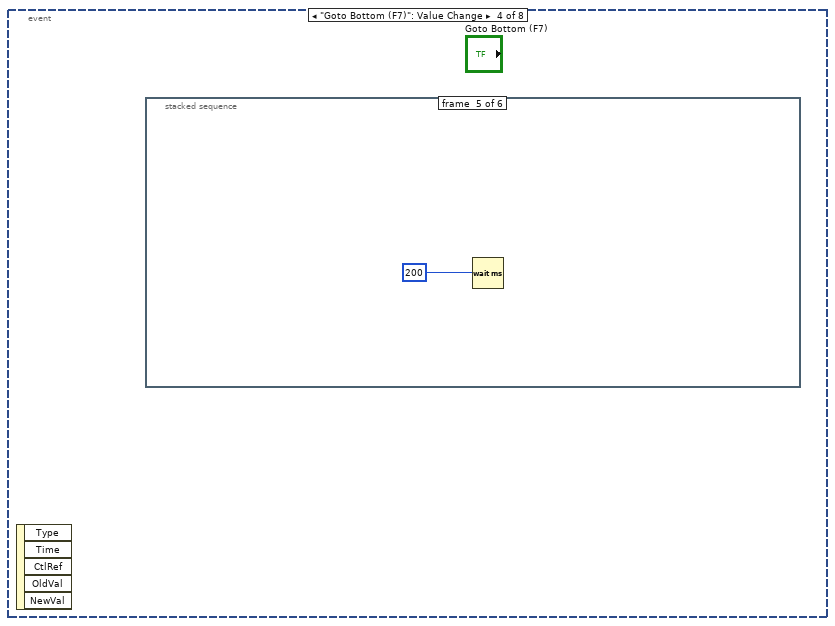
[diagram p16: hidden frame]
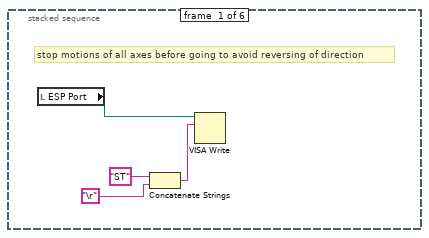
[diagram p17: hidden frame]
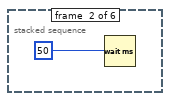
[diagram p18: hidden frame]
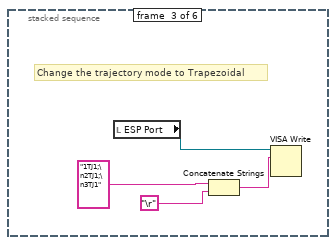
[diagram p19: hidden frame]
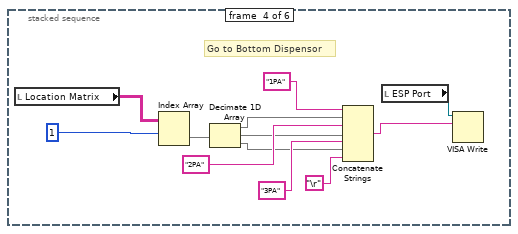
[diagram p20: hidden frame]
diagram:
  w64 = T17 2 items=["Grayscale (U8)", "Grayscale (I16)", "Grayscale (SGL)", "Complex (CSG)", "RGB (U32)", "HSL (U32)", "RGB (U64)", "Grayscale (U16)"] ("Image Type")
  w121 = cluster{"output high":i16, "output low":i16} {"output high"=3000, "output low"=0} ("FB output range 1")
  w196 = 10.0 ("y")
  w195 = 32767.0 ("y")
  w211 = 6.0  # clock mult.
  w212 = 49152000.0  # TCXO frequ.
  # "Initialize location matrix"
  n1 = Build Array("DIO count 1 (ticks)", "DIO count 2 (ticks)", "DIO count 3 (ticks)") -> (w110:u32[])
  n2 = Multiply(x="APD Integration Time (s)", y=40000000.0) -> (x*y=w128:dbl)
  n3 = Reciprocal(x="APD Integration Time (s)") -> (1/x=w125:dbl)
  n4 = local write "APD Acq Rate (Hz)"(w125) -> ()
  n5 = local read "AO1"() -> (w190:dbl)
  n6 = local read "AO2"() -> (w189:dbl)
  n7 = To Unsigned Long Integer(number=w128) -> (unsigned 32bit integer=w127:u32)
  "APD Int. Count" <- w127
  n8 = local read "Scan Increment (MHz)"() -> (w207:dbl)
  n9 = local read "Continuous MCL Scanning"() -> (w177:bool)
  n10 = local read "Fast Scan Dir"() -> (w176:bool)
  n11 = local read "Trap Intensity\nSetpoints (V)"() -> (w226:cluster{"Set 1":dbl, "Set 2":dbl})
  n12 = local read "Number of scans (MCL)"() -> (w178:u64)
  n13 = Multiply(x=w190, y=w195) -> (x*y=w192:dbl)
  n14 = Multiply(x=w189, y=w195) -> (x*y=w194:dbl)
  n15 = Divide(x=w192, y=w196) -> (x/y=w191:dbl)
  n16 = Divide(x=w194, y=w196) -> (x/y=w193:dbl)
  n17 = To Word Integer(number=w191) -> (16bit integer=w188:i16)
  n18 = To Word Integer(number=w193) -> (16bit integer=w187:i16)
  n19 = Not(x=w176) -> (.not. x?=w171:bool)
  n20 = local read "Cycles/step (MCL)"() -> (w179:u64)
  n21 = Multiply(x=w207, y=1000.0) -> (x*y=w214:dbl)
  n22 = local read "Scan steps (MCL)"() -> (w180:u64)
  n23 = local write "Trap Pos FIFO Timeout"(u16 0 ("Trap Pos FIFO Timeout")) -> ()
  n24 = local read "Desired Scan Incr (V)"() -> (w182:dbl)
  n25 = Scale By Power Of 2(n=48, x=w214) -> (x*2^n=w215:dbl)
  n26 = Multiply(x=w212, y=w211) -> (x*y=w210:dbl)
  n27 = Divide(x=w215, y=w210) -> (x/y=w209:dbl)
  n28 = local read "Number Interlace Sets"() -> (w103:u8)
  n29 = Split 1D Array(array=w110, index=w103) -> (first subarray=w112:u32[])  [unwired: 1 out]
  n30 = Add Array Elements(numeric array=w112) -> (sum=w111:u32)
  n31 = property on="AI Count (ticks)" class="DigNum (strict)"("Val(Sgnl)"="AI Count (ticks)") -> ()  [unwired: 2 in, 2 out]
  n32 = local read "# Samples/channel"() -> (w199:u32)
  n33 = local read "Number of F/B Scans (AOD)"() -> (w200:u16)
  n34 = To Quad Integer(1:w209) -> (0:w206:i64)
  n35 = local read "Not-Interlacing Set"() -> (w102:enum32{"Set 1", "Set 2", "Set 3"})
  n36 = To Unsigned Byte Integer(number=w102) -> (unsigned 8bit integer=w108:u8)
  n37 = Index Array(array=w110, index=w108) -> (element=w109:u32)
  n38 = local read "Feedback On/Off"() -> (w229:cluster{"Set 1":bool, "Set 2":bool})
  n39 = local read "PID Gains"() -> (w221:T10)
  n40 = Divide(x=40000000.0, y="AI Count (ticks)") -> (x/y=w168:dbl)
  n41 = Multiply(x=w182, y=32767.0) -> (x*y=w184:dbl)
  n42 = local read "Scan steps (AOD)"() -> (w205:u64)
  n43 = local read "All FB On/Off"() -> (w230:bool)
  n44 = local read "Cycles/step (AOD)"() -> (w204:u64)
  n45 = local write "AI rate (Hz)"(w168) -> ()
  n46 = Divide(x=w184, y=10.0) -> (x/y=w183:dbl)
  n47 = Multiply(x=w205, y=w204) -> (x*y=w203:u64)
  n48 = Multiply(x=3276.7, y=w226) -> (x*y=w225:cluster{"Set 1":dbl, "Set 2":dbl})
  n49 = To Word Integer(number=w183) -> (16bit integer=w181:i16)
  n50 = Multiply(x=w203, y=u64 2) -> (x*y=w201:u64)
  n51 = local read "Sets to FIFO (Traps)"() -> (w233:T15)
  n52 = Divide(x=w168, y="FPGA Ave.") -> (x/y=w169:dbl)
  n53 = To Word Integer(number=w225) -> (16bit integer=w224:cluster{"Set 1":i16, "Set 2":i16})
  n54 = xnode "Open FPGA VI Reference"("resource name"=T18 "RIO0") -> ("FPGA VI Reference Out"=w218:T19)  [unwired: 1 in, 1 out]
  n55 = Unbundle By Name(w221) -> ("Set 1"=w220:T14, "Set 2"=w219:T14)
  n56 = Multiply(x=w201, y=w200) -> (x*y=w198:u64)
  n57 = local write "Ave. Rate (Hz)"(w169) -> ()
  n58 = Divide(x=w198, y=w199) -> (x/y=w197:dbl)
  n59 = Unbundle By Name(w224) -> ("Set 1"=w223:i16, "Set 2"=w222:i16)
  n60 = local read "2D or 1D Scan"() -> (w122:bool)
  n61 = local write "Data points/scans"(w198) -> ()
  n62 = local read "Scan BD"() -> (w216:bool)
  n63 = And(x=w229, y=w230) -> (x .and. y?=w228:cluster{"Set 1":bool, "Set 2":bool})
  n64 = local write "Data points/scan (f/b)"(w201) -> ()
  n65 = Reciprocal(x=w169) -> (1/x=w170:dbl)
  n66 = local read "N Acq Sets (Traps + Fl.)"() -> (w161:i16)
  n67 = local write "N sets should be saved"(w197) -> ()
  n68 = Unbundle By Name(w228) -> ("Set 1"=w232:bool, "Set 2"=w231:bool)
  n69 = local read "Interlace"() -> (w104:bool)
  n70 = Select(t=w111, s=w104, f=w109) -> (s? t:f=w101:u32)
  n71 = local write "Update Count (MCL)"(w101) -> ()
  n72 = local write "Total Counts (ticks)"(w101) -> ()
  n73 = xnode "Invoke Method"("FPGA VI Reference In"=w218) -> ("FPGA VI Reference Out"=w120:T19, "error out"=w139:errorcluster)  [unwired: 1 in]
  n74 = local write "Ave. Period (s)"(w170) -> ()
  n75 = property on="2D or 1D Scan" class="Bool (strict)"("Val(Sgnl)"=w122) -> ()  [unwired: 2 in, 2 out]
  n76 = xnode "Read/Write Control"("FPGA VI Reference In"=w119, "error in"=w139, "ai count"="AI Count (ticks)", "Interlace ON/OFF"=w104, "Number Interlace Cycles"=w103, "AI1 Sets to FIFO"=w233, "FB On/Off Set 1"=w232, "FB On/Off Set 2"=w231, "Interlace Off Parameters"=w102, "FB Setpoint Set 1"=w223, "FB Setpoint Set 2"=w222, "FB Gains Set 1"=w220, "FB Gains Set 2"=w219, "FB output range 1"=w121, "FB output range 2"=w121, "Cycles per step"=w204, "Scan BD"=w216, "Number of scans"=w200, "Scan steps"=w205, "Scan freq.  increment"=w206, "AO1"=w188, "AO2"=w187, "Scan freq.  increment (MCL)"=w181, "Scan steps (MCL)"=w180, "Cycles per step (MCL)"=w179, "Number of scans (MCL)"=w178, "MCL count"=w101, "Cont. Scan (MCL)"=w177, "MCL Scan Axis"=w171, "1D or 2D Scan?"=w122, "N of AI1 Int Acq Sets"=w161, "Freq or Amp switch first"="Freq or Amp switch first", "Freq switch delay"="Freq switch delay", "Amp switch delay"="Amp switch delay", "Swap F1 and F2"="Swap F1 and F2", "APD Acq Rate Count"=w127, "APD to FIFO"=FALSE, "APD Gate Operating Mode"="APD Gate", "APD Gate ON Count"="APD Gate ON Count", "APD Gate OFF Count"="APD Gate OFF Count", "Invert APD Gate"="Invert APD Gate", "DIO count 1 (ticks)"="DIO count 1 (ticks)", "DIO count 2 (ticks)"="DIO count 2 (ticks)", "DIO count 3 (ticks)"="DIO count 3 (ticks)", "APD 1 AO scale factor"="APD 1 AO Mult.", "APD 2 AO scale factor"="APD 2 AO Mult.") -> ("FPGA VI Reference Out"=w96:T19, "error out"=w98:errorcluster)  [unwired: 1 in]
  n77 = local read "Green Laser ON/Interlacing"() -> (w99:bool)
  n78 = local read "Green laser mode"() -> (w100:enum32{"Laser ON", "Laser OFF", "Interlace"})
  n79 = local read "GI Frequency, OFF count"() -> (w92:u32)
  n80 = local read "GI Frequency, ON count"() -> (w91:u32)
  n81 = Multiply(x="Current When FB OFF (%)", y=655.35) -> (x*y=w82:dbl)
  n82 = local read "Green FB Count"() -> (w90:u32)
  n83 = Multiply(x="Green FB Setpoint (mV)", y=3.2767) -> (x*y=w79:dbl)
  n84 = To Unsigned Word Integer(number=w82) -> (unsigned 16bit integer=w80:u16)
  n85 = local read "Invert GI"() -> (w94:bool)
  n86 = To Word Integer(number=w79) -> (16bit integer=w77:i16)
  n87 = case shown="True" w99 {
    tunnel: w100 -> [_ w253]
    tunnel: [enum32{"Laser ON", "Laser OFF", "Interlace"}."Laser OFF" ("Green laser mode") w253] -> w93
    frame False {
    }
    frame True {
    }
  }
  n88 = local read "Trap Pos. AI1 X Pre-scale"() -> (w48:u16)
  n89 = local read "Trap Pos FB Monitor\nT1 or T2"() -> (w55:bool)
  n90 = local read "Trap Pos FB Int Count"() -> (w43:u16)
  n91 = local read "Trap Pos FB Negate Action"() -> (w54:bool)
  n92 = local read "Trap Pos. FB Offset Factor"() -> (w53:i64)
  n93 = local read "Trap Pos. FB Mult Factor"() -> (w52:i64)
  n94 = local read "Trap Pos. FB Gains"() -> (w50:T11)
  n95 = local read "Trap Pos. FB Range"() -> (w51:T12)
  n96 = xnode "Read/Write Control"("FPGA VI Reference In"=w96, "error in"=w98, "Green interlace ON count 2"=w91, "Green interlace OFF count 2"=w92, "Invert GI 2"=w94, "Operating Mode 2"=w93, "Green FB Gains"="Green FB Gains", "Green FB Setpoint"=w77, "Green FB On/Off"="Green FB On/Off", "Current Out"=w80, "Green int current ON count adj"="Green int current ON count adj", "Green FB Count"=w90, "Operating Mode"=w93, "Green interlace OFF count"=w92, "Green interlace ON count"=w91, "Invert GI"=w94, "Trap Pos FB Monitor T1 or T2"=w55, "Trap Pos FB Negate Action"=w54, "Trap Pos. FB Offset Factor"=w53, "Trap Pos. FB Mult Factor"=w52, "Trap Pos. FB Range"=w51, "Trap Pos. FB Gains"=w50, "Force feedback"=FALSE, "AI1 X Scale"=w48, "Trap Pos to FIFO"=TRUE, "Trap Pos FB Int Count"=w43) -> ("FPGA VI Reference Out"=w95:T19, "error out"=w97:errorcluster)
  n97 = xnode "Invoke Method"("FPGA VI Reference In"=w95, "error in"=w97, "Requested Depth"="Trap AI FIFO Depth") -> ("FPGA VI Reference Out"=w58:T19, "error out"=w57:errorcluster)  [unwired: 1 out]
  n98 = xnode "Invoke Method"("FPGA VI Reference In"=w58, "error in"=w57, "Requested Depth"="Trap Position FIFO Depth") -> ("FPGA VI Reference Out"=w45:T19, "error out"=w44:errorcluster)  [unwired: 1 out]
  n99 = flat-sequence {
    tunnel: w120 -> [w258]
    tunnel: [w258] -> w119
    tunnel: [w257] -> w118
    tunnel: [w256] -> w117
    tunnel: [w254] -> w115
    tunnel: [w255] -> w116
    frame #0 {
      w255 = T16 {"Minimum"=50.0, "Maximum"=100.0, "Increment"=1.0} ("Min Max Inc")
      w254 = T16 {"Minimum"=0.0, "Maximum"=75.0, "Increment"=1.0} ("Data Entry Limits")
      w257 = T16 {"Minimum"=50.0, "Maximum"=100.0, "Increment"=1.0} ("Min Max Inc")
      w256 = T16 {"Minimum"=0.0, "Maximum"=75.0, "Increment"=1.0} ("Data Entry Limits")
      n100 = property on="BD 2 Frequency 1 (MHz)" class="DigNum (strict)"("Data Range"=w255) -> ()  [unwired: 2 in, 2 out]
      n101 = property on="BD 2 Frequency 3 (MHz)" class="DigNum (strict)"("Data Range"=w255) -> ()  [unwired: 2 in, 2 out]
      n102 = property on="BD 2 Frequency 2 (MHz)" class="DigNum (strict)"("Data Range"=w255) -> ()  [unwired: 2 in, 2 out]
      n103 = property on="BD 1 Frequency 1 (MHz)" class="DigNum (strict)"("Data Range"=w257) -> ()  [unwired: 2 in, 2 out]
      n104 = property on="BD 1 Frequency 2 (MHz)" class="DigNum (strict)"("Data Range"=w257) -> ()  [unwired: 2 in, 2 out]
      n105 = property on="BD 1 Frequency 3 (MHz)" class="DigNum (strict)"("Data Range"=w257) -> ()  [unwired: 2 in, 2 out]
      n106 = property on="BD 2 Amplitude 1 (%)" class="DigNum (strict)"("Data Range"=w254) -> ()  [unwired: 2 in, 2 out]
      n107 = property on="BD 2 Amplitude 2 (%)" class="DigNum (strict)"("Data Range"=w254) -> ()  [unwired: 2 in, 2 out]
      n108 = property on="BD 2 Amplitude 3 (%)" class="DigNum (strict)"("Data Range"=w254) -> ()  [unwired: 2 in, 2 out]
      n109 = property on="BD 1 Amplitude 3 (%)" class="DigNum (strict)"("Data Range"=w256) -> ()  [unwired: 2 in, 2 out]
      n110 = property on="BD 1 Amplitude 2 (%)" class="DigNum (strict)"("Data Range"=w256) -> ()  [unwired: 2 in, 2 out]
      n111 = property on="BD 1 Amplitude 1 (%)" class="DigNum (strict)"("Data Range"=w256) -> ()  [unwired: 2 in, 2 out]
      "X RF Frequency Limits (MHz)" <- w257
      "X RF Amplitude Limits (%)" <- w256
      "Y RF Amplitude Limits (%)" <- w254
      "Y RF Frequency Limits (MHz)" <- w255
    }
  }
  n112 = xnode "Invoke Method"("FPGA VI Reference In"=w45, "error in"=w44) -> ("FPGA VI Reference Out"=w22:T19, "error out"=w21:errorcluster)  [unwired: 1 in]
  n113 = flat-sequence "Initial FPGA Loop Relative Phase Adjustment" {
    tunnel: "Initial Phase Adjustment (APD 2 Gate)" -> [w260]
    tunnel: "Initial Phase Adjustment (GI) 2" -> [w261]
    tunnel: "Initial Phase Adj. (MCL)" -> [w262]
    tunnel: w21 -> [w263]
    tunnel: w22 -> [w264]
    tunnel: "Initial Phase Adjustment (GI)" -> [w265]
    tunnel: "Initial Phase Adjustment (AI1)" -> [w266]
    tunnel: [w266] -> w31
    tunnel: [w265] -> w30
    tunnel: [w264] -> w29
    tunnel: [w263] -> w28
    tunnel: [w262] -> w27
    tunnel: [w261] -> w26
    tunnel: [w260] -> w25
    tunnel: [w278] -> w145
    tunnel: [w272] -> w143
    tunnel: "Initial Phase Adjustment (APD Acq)" -> [w271]
    tunnel: "Initial Phase Adjustment (APD 1 Gate)" -> [w270]
    tunnel: "Initial Phase Adjustment (Green FB)" -> [w269]
    tunnel: w31 -> [w277]
    tunnel: w30 -> [w276]
    tunnel: w29 -> [w275]
    tunnel: w28 -> [w274]
    tunnel: w27 -> [w273]
    tunnel: w26 -> [w268]
    tunnel: w25 -> [w267]
    tunnel: w145 -> [w280]
    tunnel: [w281] -> w144
    tunnel: w143 -> [w281]
    tunnel: [w280] -> w142
    tunnel: w144 -> [w284]
    tunnel: w142 -> [w283]
    tunnel: [w286] -> w141
    tunnel: [w285] -> w140
    tunnel: [w288] -> w20
    tunnel: [w289] -> w23
    tunnel: w141 -> [w289]
    tunnel: w140 -> [w288]
    frame #0 {
      n114 = Wait (ms)(milliseconds to wait=u32 1000) -> ()  [unwired: 1 out]
    }
    frame #1 {
      n115 = xnode "Read/Write Control"("FPGA VI Reference In"=w275, "error in"=w274, "Phase count adjustment"=w277, "Phase count adjustment (GI)"=w276, "Phase count adjustment (MCL)"=w273, "Phase Count Adjustment (APD Acq)"=w271, "Phase count adjustment (APD 1 Gate)"=w270, "Phase count adjustment (APD 2 Gate)"=w267, "Phase count adjustment (Green FB)"=w269, "Phase count adjustment (GI) 2"=w268) -> ("FPGA VI Reference Out"=w272:T19, "error out"=w278:errorcluster)
    }
    frame #2 {
      n116 = Wait (ms)(milliseconds to wait=u32 1000) -> ()  [unwired: 1 out]
    }
    frame #3 {
      w282 = TRUE
      n117 = xnode "Read/Write Control"("FPGA VI Reference In"=w284, "error in"=w283, "+ phase"=w282, "+ phase (GI)"=w282, "+ phase (MCL)"=w282, "+ phase (APD Acq)"=w282, "+ phase (APD 1 Gate)"=w282, "+ phase (APD 2 Gate)"=w282, "+ phase (Green FB)"=w282, "+ phase (GI) 2"=w282) -> ("FPGA VI Reference Out"=w285:T19, "error out"=w286:errorcluster)
    }
    frame #4 {
      n118 = Wait (ms)(milliseconds to wait=u32 1000) -> ()  [unwired: 1 out]
    }
  }
  n119 = local read "Phase adj. (Green FB)"() -> (w113:i16)
  n120 = local read "Phase adj. (GI) 2"() -> (w83:i16)
  n121 = local read "Phase adjust (MCL)"() -> (w172:i16)
  n122 = local read "Phase adj. (AI1)"() -> (w174:i16)
  n123 = local read "Phase adj. (GI)"() -> (w173:i16)
  n124 = xnode "Read/Write Control"("FPGA VI Reference In"=w20, "error in"=w23, "Phase count adjustment"=w174, "Phase count adjustment (GI)"=w173, "Phase count adjustment (MCL)"=w172, "Phase Count Adjustment (APD Acq)"="Phase Adj. (APD Acq)", "Phase count adjustment (APD 1 Gate)"="Phase Adj. (APD 1 Gate)", "Phase count adjustment (APD 2 Gate)"="Phase Adj. (APD 2 Gate)", "Phase count adjustment (Green FB)"=w113, "Phase count adjustment (GI) 2"=w83) -> ("FPGA VI Reference Out"=w19:T19, "error out"=w18:errorcluster)
  n125 = call "Initialize RF boards - interlace 3.vi"("error in"=w18, "FPGA VI Reference In"=w19) -> ("FPGA VI Reference Out"=w150:T19)  [unwired: 1 out]
  n126 = call "set RF board frequency - interlace.vi"("Board 2 Frequency Limits"=w116, "Board 1 Frequency Limits"=w118, "FPGA VI Reference In"=w150, "Board 2 Frequency 3 (MHz)"="BD 2 Frequency 3 (MHz)", "Board 1 Frequency 3 (MHz)"="BD 1 Frequency 3 (MHz)", "Board 2 Frequency 2 (MHz)"="BD 2 Frequency 2 (MHz)", "Board 2 Frequency 1 (MHz)"="BD 2 Frequency 1 (MHz)", "Board 1 Frequency 2 (MHz)"="BD 1 Frequency 2 (MHz)", "Board 1 Frequency 1  (MHz)"="BD 1 Frequency 1 (MHz)") -> ("error out"=w244:errorcluster, "FPGA VI Reference Out"=w245:T19)  [unwired: 1 in]
  n127 = call "set RF board amplitude - interlace.vi"("Board 2 Amplitude Limits"=w115, "Board 1 Amplitude Limits"=w117, "error in"=w244, "FPGA VI Reference In"=w245, "Board 2 Amplitude 3 (%)"="BD 2 Amplitude 3 (%)", "Board 1 Amplitude 3 (%)"="BD 1 Amplitude 3 (%)", "Board 2 Amplitude 2 (%)"="BD 2 Amplitude 2 (%)", "Board 2 Amplitude 1 (%)"="BD 2 Amplitude 1 (%)", "Board 1 Amplitude 2 (%)"="BD 1 Amplitude 2 (%)", "Board 1 Amplitude 1 (%)"="BD 1 Amplitude 1 (%)") -> ("error out"=w16:errorcluster, "FPGA VI Reference Out"=w17:T19)
  n128 = flat-sequence {
    tunnel: w17 -> [w298]
    tunnel: w16 -> [w297]
    tunnel: [w296] -> w237
    tunnel: [w295] -> w236
    tunnel: [w302] -> w235
    tunnel: w237 -> [w302]
    tunnel: [w301] -> w234
    tunnel: w236 -> [w301]
    tunnel: w235 -> [w311]
    tunnel: w234 -> [w310]
    tunnel: [w309] -> w12
    tunnel: [w304] -> w11
    tunnel: [w314] -> w40
    tunnel: [w318] -> w24
    tunnel: w12 -> [w318]
    tunnel: w11 -> [w313]
    frame #0 {
      n129 = local read "Trap 1 (ON/OFF)"() -> (w290:bool)
      n130 = xnode "Read/Write Control"("FPGA VI Reference In"=w298, "error in"=w297, "Direct RF Box  Communication"=FALSE) -> ("FPGA VI Reference Out"=w296:T19, "error out"=w295:errorcluster)
      n131 = local write "Saving..."(FALSE ("Saving Data")) -> ()
      n132 = local write "Stop All"(FALSE ("Stop All")) -> ()
      n133 = local write "Index"(1.0 ("Index")) -> ()
      n134 = property on="Trap 1 ON" class="Bool (strict)"("Value"=w290) -> ()  [unwired: 2 in, 2 out]
      "Manipulating Trap" <- FALSE ("Manipulating Trap")
    }
    frame #1 {
      n135 = local read "Trap 2 (ON/OFF)"() -> (w300:bool)
      n136 = Wait (ms)(milliseconds to wait=u32 50) -> ()  [unwired: 1 out]
      n137 = property on="Trap 2 ON" class="Bool (strict)"("Val(Sgnl)"=w300) -> ()  [unwired: 2 in, 2 out]
    }
    frame #2 {
      n138 = local read "Scan Range (nm)"() -> (w305:dbl)
      n139 = xnode "Read/Write Control"("FPGA VI Reference In"=w311, "error in"=w310, "FPGA Controls  RF Box"=TRUE ("Direct RF Box  Communication")) -> ("FPGA VI Reference Out"=w309:T19, "error out"=w304:errorcluster)
      n140 = call "Update messages.vi"("Message to add"="UHR-Fleezers ready.", "Old message string"="") -> ("New message string"=w308:string)
      n141 = local write "Messages"(w308) -> ()
      n142 = property on="Scan Range (nm)" class="DigNum (strict)"("Val(Sgnl)"=w305) -> ()  [unwired: 2 in, 2 out]
    }
    frame #3 {
      n143 = call "hamilton_controller.vi"("error in"=w313, "action"=T20."CONNECT") -> ("error out"=w315:errorcluster)  [unwired: 9 in]
      n144 = call "hamilton_controller.vi"("error in"=w315, "action"=T20."INITIALIZE VALVES") -> ("error out"=w314:errorcluster)  [unwired: 9 in]
    }
  }
  n145 = Subtract(x="BD 1 Frequency 1 (MHz)", y="BD 1 Frequency 2 (MHz)") -> (x-y=w160:dbl)
  n146 = Subtract(x="BD 2 Frequency 1 (MHz)", y="BD 2 Frequency 2 (MHz)") -> (x-y=w159:dbl)
  n147 = Square(x=w159) -> (x^2=w157:dbl)
  n148 = Square(x=w160) -> (x^2=w158:dbl)
  n149 = Add(x=w158, y=w157) -> (x+y=w156:dbl)
  n150 = Square Root(x=w156) -> (sqrt(x)=w155:dbl)
  n151 = local write "Trap Delta (MHz)"(w155) -> ()
  n152 = call "IMAQ Create"("Image Name"="APD 1 Image", "Image Type"=w64) -> ("New Image"=w63:T3)  [unwired: 3 in, 1 out]
  n153 = call "IMAQ Create"("Image Name"="APD 2 Image", "Image Type"=w64) -> ("New Image"=w62:T3)  [unwired: 3 in, 1 out]
  n154 = call "IMAQ Create"("Image Name"="Det. X Image", "Image Type"=w64) -> ("New Image"=w61:T3)  [unwired: 3 in, 1 out]
  n155 = call "IMAQ Create"("Image Name"="Det. Y Image", "Image Type"=w64) -> ("New Image"=w60:T3)  [unwired: 3 in, 1 out]
  n156 = Bundle("New Image"=w63, "New Image"=w62, "New Image"=w61, "New Image"=w60) -> (w59:T21)  [unwired: 1 in]
  n157 = Current VI's Path() -> (path=w1:path)
  n158 = Concatenate Strings("N.D.", "\r\n") -> (w5:string)
  n159 = Strip Path(path=w1) -> (stripped path=w2:path)  [unwired: 1 out]
  n160 = Initialize Array(w5, 4, 3) -> (w8:string[][])
  n161 = Build Path(base path=w2, name or relative path="Locations.txt") -> (appended path=→"Location path":path)
  n162 = local write "Location Matrix"(w8) -> ()
  n163 = while {
    stop <- w319 stop-if-true
    n164 = event shown="[0] Timeout" {
      selector: _ -> [_ _ _ _ _ _ _ _]
      dyn-events: _ -> [_ _ _ _ _ _ _ _]
      timeout: 10 -> [_ _ _ _ _ _ _ _]
      tunnel: [FALSE _ _ _ _ _ _ TRUE] -> w319
      event Timeout {
        # "Change the trajectory mode to Jog"
        # "Query and display stage positions"
        # "Setting ESP300 left and right limits for Z-axis, input in mm"
        # "Display Selected Location"
        n165 = event-data() -> ()  [unwired: 1 in, 2 out]
        n166 = local read "Capture Locations"() -> (w344:i32)
        n167 = local read "Location Matrix"() -> (w345:string[][])
        n168 = Concatenate Strings("1TP;\n2TP;\n3TP;\n1MD?;\n2MD?;\n3MD?" ("Substring"), "\r") -> (w328:string)
        n169 = local read "ESP Port"() -> (w331:refnum<visa-resource-name>)
        n170 = Index Array(array=w345, index (row)=w344) -> (element=w343:string[])  [unwired: 1 in]
        n171 = local read "ESP Port"() -> (w340:refnum<visa-resource-name>)
        n172 = VISA Write(VISA resource name=w331, write buffer=w328, error in (no error)="error in") -> (VISA resource name out=w329:refnum<visa-resource-name>, error out=w327:errorcluster)  [unwired: 1 out]
        n173 = Concatenate Strings("3SL" ("Substring"), "ESP ZL-Limit", ";3SR", "ESP ZR-Limit", "\r") -> (w339:string)
        n174 = Array To Cluster(array=w343) -> (cluster=w342:T22)
        n175 = case shown="True" TRUE ("Case Constant\n(See Context Help)") {
          tunnel: w329 -> [_ w383]
          tunnel: w327 -> [w364 w382]
          tunnel: [w364 w366] -> w333
          frame False {
          }
          frame True {
            w376 = u16 10 items=["1.0"=10, "1.5"=15, "2.0"=20] ("Serial Settings:Stop Bits")
            w377 = u16 0 items=["None", "Odd", "Even", "Mark", "Space"] ("Serial Settings:Parity")
            n176 = property class="Instr"(reference=w383, error in=w382, "Baud"=u32 921600 ("Serial Settings:Baud Rate"), "Data Bits"=u16 8 ("Serial Settings:Data Bits"), "Parity"=w377, "Stop Bits"=w376) -> (reference out=w381:refnum<visa-resource-name>, error out=w380:errorcluster, "Bytes at Port"=w365:u32)
            n177 = Wait (ms)(milliseconds to wait=u32 10) -> ()  [unwired: 1 out]
            n178 = VISA Read(VISA resource name=w381, byte count=w365, error in (no error)=w380) -> (VISA resource name out=w389:refnum<visa-resource-name>, read buffer=→"X Pos":string, error out=w390:errorcluster)  [unwired: 1 out]
            n179 = VISA Read(VISA resource name=w389, byte count=w365, error in (no error)=w390) -> (VISA resource name out=w387:refnum<visa-resource-name>, read buffer=→"Y Pos":string, error out=w388:errorcluster)  [unwired: 1 out]
            n180 = VISA Read(VISA resource name=w387, byte count=w365, error in (no error)=w388) -> (VISA resource name out=w375:refnum<visa-resource-name>, read buffer=→"Z Pos Pos":string, error out=w374:errorcluster)  [unwired: 1 out]
            n181 = VISA Read(VISA resource name=w375, byte count=w365, error in (no error)=w374) -> (VISA resource name out=w371:refnum<visa-resource-name>, read buffer=→"X Motion":string, error out=w372:errorcluster)  [unwired: 1 out]
            n182 = VISA Read(VISA resource name=w371, byte count=w365, error in (no error)=w372) -> (VISA resource name out=w370:refnum<visa-resource-name>, read buffer=→"Y Motion":string, error out=w368:errorcluster)  [unwired: 1 out]
            n183 = VISA Read(VISA resource name=w370, byte count=w365, error in (no error)=w368) -> (read buffer=→"Z motion":string, error out=w366:errorcluster)  [unwired: 2 out]
          }
        }
        "error out" <- w333
        n184 = VISA Write(VISA resource name=w340, write buffer=w339) -> ()  [unwired: 1 in, 3 out]
        n185 = local write item#485(w342) -> ()
        n186 = disable-structure shown="Disabled" {
          frame Disabled {
            # "Change Low Jog Velocity"
            # "Change High Jog Velocity"
            n187 = Concatenate Strings("1JH" ("Substring"), "Axis 1", "2JH" ("Substring"), "Axis 2", "3JH" ("Substring"), "Axis 3", "\r") -> (w363:string)
            n188 = local read "ESP Port"() -> (w362:refnum<visa-resource-name>)
            n189 = VISA Write(VISA resource name=w362, write buffer=w363) -> ()  [unwired: 1 in, 3 out]
            n190 = Concatenate Strings("1JW" ("Substring"), "Axis 1", "2JW" ("Substring"), "Axis 2", "3JW" ("Substring"), "Axis 3", "\r") -> (w354:string)
            n191 = local read "ESP Port"() -> (w353:refnum<visa-resource-name>)
            n192 = VISA Write(VISA resource name=w353, write buffer=w354) -> ()  [unwired: 1 in, 3 out]
          }
          frame Enabled {
          }
        }
        n193 = local read "ESP Port"() -> (w321:refnum<visa-resource-name>)
        n194 = Concatenate Strings("1TJ3;\n2TJ3;\n3TJ3" ("Substring"), "\r") -> (w322:string)
        n195 = VISA Write(VISA resource name=w321, write buffer=w322) -> ()  [unwired: 1 in, 3 out]
      }
      event "Goto Top (F6)": Value Change {
        n196 = event-data() -> ()  [unwired: 1 in, 5 out]
        n197 = stacked-sequence {
          frame #0 {
            # "stop motions of all axes before going to avoid reversing of direction"
            n198 = local read "ESP Port"() -> (w395:refnum<visa-resource-name>)
            n199 = Concatenate Strings("ST" ("Substring"), "\r") -> (w392:string)
            n200 = VISA Write(VISA resource name=w395, write buffer=w392) -> ()  [unwired: 1 in, 3 out]
          }
          frame #1 {
            n201 = Wait (ms)(milliseconds to wait=u32 50) -> ()  [unwired: 1 out]
          }
          frame #2 {
            # "Change the trajectory mode to Trapezoidal"
            n202 = local read "ESP Port"() -> (w400:refnum<visa-resource-name>)
            n203 = Concatenate Strings("1TJ1;\n2TJ1;\n3TJ1" ("Substring"), "\r") -> (w397:string)
            n204 = VISA Write(VISA resource name=w400, write buffer=w397) -> ()  [unwired: 1 in, 3 out]
          }
          frame #3 {
            # "Go to Top Dispensor"
            n205 = local read "Location Matrix"() -> (w412:string[][])
            n206 = Index Array(array=w412, index (row)=0) -> (element=w408:string[])  [unwired: 1 in]
            n207 = Decimate 1D Array(w408) -> (w406:string[], w404:string[], w402:string[])
            n208 = local read "ESP Port"() -> (w409:refnum<visa-resource-name>)
            n209 = Concatenate Strings("1PA" ("Substring"), w406, "2PA" ("Substring"), w404, "3PA" ("Substring"), w402, "\r") -> (w410:string)
            n210 = VISA Write(VISA resource name=w409, write buffer=w410) -> ()  [unwired: 1 in, 3 out]
          }
          frame #4 {
            n211 = Wait (ms)(milliseconds to wait=u32 100) -> ()  [unwired: 1 out]
          }
          frame #5 {
            # "Change the trajectory mode to Jog"
            n212 = local read "ESP Port"() -> (w417:refnum<visa-resource-name>)
            n213 = Concatenate Strings("1TJ3;\n2TJ3;\n3TJ3" ("Substring"), "\r") -> (w414:string)
            n214 = VISA Write(VISA resource name=w417, write buffer=w414) -> ()  [unwired: 1 in, 3 out]
          }
        }
      }
      event "Goto Exp (F8)": Value Change {
        n215 = event-data() -> ()  [unwired: 1 in, 5 out]
        n216 = stacked-sequence {
          frame #0 {
            # "stop motions of all axes before going to avoid reversing of direction"
            n217 = local read "ESP Port"() -> (w421:refnum<visa-resource-name>)
            n218 = Concatenate Strings("ST" ("Substring"), "\r") -> (w418:string)
            n219 = VISA Write(VISA resource name=w421, write buffer=w418) -> ()  [unwired: 1 in, 3 out]
          }
          frame #1 {
            n220 = Wait (ms)(milliseconds to wait=u32 50) -> ()  [unwired: 1 out]
          }
          frame #2 {
            # "Change the trajectory mode to Trapezoidal"
            n221 = local read "ESP Port"() -> (w426:refnum<visa-resource-name>)
            n222 = Concatenate Strings("1TJ1;\n2TJ1;\n3TJ1" ("Substring"), "\r") -> (w423:string)
            n223 = VISA Write(VISA resource name=w426, write buffer=w423) -> ()  [unwired: 1 in, 3 out]
          }
          frame #3 {
            # "Go to Experimental"
            n224 = local read "Location Matrix"() -> (w438:string[][])
            n225 = Index Array(array=w438, index (row)=2) -> (element=w434:string[])  [unwired: 1 in]
            n226 = Decimate 1D Array(w434) -> (w432:string[], w430:string[], w428:string[])
            n227 = Concatenate Strings("1PA" ("Substring"), w432, "2PA" ("Substring"), w430, "3PA" ("Substring"), w428, "\r") -> (w436:string)
            n228 = local read "ESP Port"() -> (w435:refnum<visa-resource-name>)
            n229 = VISA Write(VISA resource name=w435, write buffer=w436) -> ()  [unwired: 1 in, 3 out]
          }
          frame #4 {
            n230 = Wait (ms)(milliseconds to wait=u32 200) -> ()  [unwired: 1 out]
          }
          frame #5 {
            # "Change the trajectory mode to Jog"
            n231 = local read "ESP Port"() -> (w440:refnum<visa-resource-name>)
            n232 = Concatenate Strings("1TJ3;\n2TJ3;\n3TJ3" ("Substring"), "\r") -> (w443:string)
            n233 = VISA Write(VISA resource name=w440, write buffer=w443) -> ()  [unwired: 1 in, 3 out]
          }
        }
      }
      event "Goto Bottom (F7)": Value Change {
        n234 = event-data() -> ()  [unwired: 1 in, 5 out]
        n235 = stacked-sequence {
          frame #0 {
            # "stop motions of all axes before going to avoid reversing of direction"
            n236 = local read "ESP Port"() -> (w447:refnum<visa-resource-name>)
            n237 = Concatenate Strings("ST" ("Substring"), "\r") -> (w444:string)
            n238 = VISA Write(VISA resource name=w447, write buffer=w444) -> ()  [unwired: 1 in, 3 out]
          }
          frame #1 {
            n239 = Wait (ms)(milliseconds to wait=u32 50) -> ()  [unwired: 1 out]
          }
          frame #2 {
            # "Change the trajectory mode to Trapezoidal"
            n240 = local read "ESP Port"() -> (w452:refnum<visa-resource-name>)
            n241 = Concatenate Strings("1TJ1;\n2TJ1;\n3TJ1" ("Substring"), "\r") -> (w449:string)
            n242 = VISA Write(VISA resource name=w452, write buffer=w449) -> ()  [unwired: 1 in, 3 out]
          }
          frame #3 {
            # "Go to Bottom Dispensor"
            n243 = local read "Location Matrix"() -> (w464:string[][])
            n244 = Index Array(array=w464, index (row)=1) -> (element=w460:string[])  [unwired: 1 in]
            n245 = Decimate 1D Array(w460) -> (w458:string[], w456:string[], w454:string[])
            n246 = Concatenate Strings("1PA" ("Substring"), w458, "2PA" ("Substring"), w456, "3PA" ("Substring"), w454, "\r") -> (w462:string)
            n247 = local read "ESP Port"() -> (w461:refnum<visa-resource-name>)
            n248 = VISA Write(VISA resource name=w461, write buffer=w462) -> ()  [unwired: 1 in, 3 out]
          }
          frame #4 {
            n249 = Wait (ms)(milliseconds to wait=u32 200) -> ()  [unwired: 1 out]
          }
          frame #5 {
            # "Change the trajectory mode to Jog"
            n250 = local read "ESP Port"() -> (w466:refnum<visa-resource-name>)
            n251 = Concatenate Strings("1TJ3;\n2TJ3;\n3TJ3" ("Substring"), "\r") -> (w469:string)
            n252 = VISA Write(VISA resource name=w466, write buffer=w469) -> ()  [unwired: 1 in, 3 out]
          }
        }
      }
      event "Capture": Value Change {
        n253 = event-data() -> ()  [unwired: 1 in, 5 out]
        n254 = local read "Capture Locations"() -> (w470:i32)
        n255 = local read "Z Pos Pos"() -> (w471:string)
        n256 = local read "X Pos"() -> (w473:string)
        n257 = local read "Y Pos"() -> (w472:string)
        n258 = case shown="1" w470 {
          selector: w470 -> [w477 w484 w491 w498]
          tunnel: w473 -> [w480 w487 w494 w501]
          tunnel: w472 -> [w479 w486 w493 w500]
          tunnel: w471 -> [w478 w485 w492 w499]
          frame 0, Default {
            # "Capture Top Dispensor Location"
            n259 = local read "Location Matrix"() -> (w476:string[][])
            n260 = Build Array(w480, w479, w478) -> (w475:string[])
            n261 = Replace Array Subset(array=w476, new element=w475, index (row)=w477) -> (w474:string[][])  [unwired: 1 in]
            n262 = local write "Location Matrix"(w474) -> ()
          }
          frame 1 {
            # "Capture Bottom Dispensor Location"
            n263 = local read "Location Matrix"() -> (w483:string[][])
            n264 = Build Array(w487, w486, w485) -> (w482:string[])
            n265 = Replace Array Subset(array=w483, new element=w482, index (row)=w484) -> (w481:string[][])  [unwired: 1 in]
            n266 = local write "Location Matrix"(w481) -> ()
          }
          frame 2 {
            # "Capture Experimental Region Location"
            n267 = local read "Location Matrix"() -> (w490:string[][])
            n268 = Build Array(w494, w493, w492) -> (w489:string[])
            n269 = Replace Array Subset(array=w490, new element=w489, index (row)=w491) -> (w488:string[][])  [unwired: 1 in]
            n270 = local write "Location Matrix"(w488) -> ()
          }
          frame 3 {
            # "Capture Other Location"
            n271 = local read "Location Matrix"() -> (w497:string[][])
            n272 = Build Array(w501, w500, w499) -> (w496:string[])
            n273 = Replace Array Subset(array=w497, new element=w496, index (row)=w498) -> (w495:string[][])  [unwired: 1 in]
            n274 = local write "Location Matrix"(w495) -> ()
          }
        }
      }
      event "Save": Value Change {
        # "reshape Location Matrix to 1-D array to write"
        n275 = event-data() -> ()  [unwired: 1 in, 5 out]
        n276 = local read "Location Matrix"() -> (w505:string[][])
        n277 = local read "Location path"() -> (w502:path)
        n278 = Reshape Array(w505, 12) -> (w503:string[])
        n279 = Write to Text File(file (use dialog)=w502, text=w503) -> ()  [unwired: 2 in, 3 out]
      }
      event "Activate Joystick": Value Change {
        # "Change the trajectory mode to Jog"
        n280 = event-data() -> ()  [unwired: 1 in, 5 out]
        n281 = disable-structure shown="Disabled" {
          frame Disabled {
            n282 = case shown="True" "Activate Joystick" {
              frame False {
              }
              frame True {
                # "Change the trajectory mode to Jog"
                n283 = local read "ESP Port"() -> (w514:refnum<visa-resource-name>)
                n284 = Concatenate Strings("1TJ3;\n2TJ3;\n3TJ3" ("Substring"), "\r") -> (w511:string)
                n285 = VISA Write(VISA resource name=w514, write buffer=w511) -> ()  [unwired: 1 in, 3 out]
              }
            }
          }
          frame Enabled {
          }
        }
        n286 = local read "ESP Port"() -> (w506:refnum<visa-resource-name>)
        n287 = Concatenate Strings("1TJ3;\n2TJ3;\n3TJ3" ("Substring"), "\r") -> (w509:string)
        n288 = VISA Write(VISA resource name=w506, write buffer=w509) -> ()  [unwired: 1 in, 3 out]
      }
      event "Stop All": Mouse Down {
        n289 = event-data() -> ()  [unwired: 1 in, 5 out]
      }
    }
  }
  n290 = disable-structure shown="Disabled" {
    disable-tunnel: w24 -> [w544 _]
    frame Disabled {
      w539 = T17 0 items=["Grayscale (U8)", "Grayscale (I16)", "Grayscale (SGL)", "Complex (CSG)", "RGB (U32)", "HSL (U32)", "RGB (U64)", "Grayscale (U16)"] ("Image Type")
      n291 = call <vilib>:"IMAQ Init.vi"("Interface Name"="img0") -> ("error out"=w541:errorcluster, "IMAQ Session Out"=w543:refnum<k11>)  [unwired: 9 in]
      n292 = call <vilib>:"IMAQ Grab Setup.vi"("error in (no error)"=w541, "IMAQ Session In"=w543) -> ("error out"=w537:errorcluster, "IMAQ Session Out"=w538:refnum<k11>)  [unwired: 8 in]
      n293 = call "IMAQ Create"("Image Name"="untitled", "Image Type"=w539) -> ("New Image"=w536:T3)  [unwired: 3 in, 1 out]
      n294 = call <vilib>:"Application Directory.vi"() -> ("Application Directory"=w523:path)
      n295 = Build Path(base path=w523, name or relative path="_trap_screen_positions") -> (appended path=w531:path)
      n296 = Open/Create/Replace File(file path (use dialog)=w531, operation (0:open)=T23."open or create", access (0:read/write)=enum16{"read/write", "read-only", "write-only"}."read/write") -> (refnum out=w533:refnum<file>)  [unwired: 3 in, 2 out]
      n297 = local read "Trap Sets"() -> (w525:u32)
      n298 = for "Load trap positions on video screen from file." {
        N: w525 -> [_]
        tunnel: [w551] -> w526
        tunnel: w533 -> [w550]
        tunnel: [w547] -> w522 mode=indexing
        w549 = 4
        n299 = for {
          N: w549 -> [_]
          tunnel: [w555] -> w551
          tunnel: w550 -> [w554]
          tunnel: w549 -> [w553]
          tunnel: [w552] -> w548 mode=indexing
          n300 = Read from Binary File(5:w553, 11:w554) -> (2:w552:i32, 3:w555:refnum<file>)  [unwired: 4 in, 2 out]
        }
        n301 = Array To Cluster(array=w548) -> (cluster=w547:T27)
      }
      n302 = node-c288() -> (w546:T24)  [unwired: 4 in]
      n303 = timed-loop "acquire video and stage position" {
        timing: w546 -> [_]
        timing-out: [_] -> w545
        tunnel: w538 -> [w574]
        tunnel: w537 -> [w573]
        tunnel: w536 -> [w572]
        tunnel: [w571] -> w518
        tunnel: [w568] -> w519
        tunnel: [w569] -> w517
        tunnel: w544 -> [_]
        shift-right: [w565] -> w535
        shift-left: w522 -> [w566]
        tunnel: w525 -> [w563]
        stop <- w570 stop-if-true
        n304 = node-c288() -> ()  [unwired: 1 in, 1 out]
        n305 = event shown="[0] Timeout" {
          selector: _ -> [_ _ _ _]
          dyn-events: _ -> [_ _ _ _]
          timeout: 10 -> [_ _ _ _]
          tunnel: w574 -> [w585 w600 w609 w628]
          tunnel: w573 -> [w584 w602 w607 w630]
          tunnel: w572 -> [w583 w601 w608 w629]
          tunnel: [w582 w600 w609 w628] -> w571
          tunnel: [w575 w604 FALSE FALSE] -> w570
          tunnel: [w579 w602 w607 w630] -> w569
          tunnel: [w578 w601 w608 w629] -> w568
          tunnel: "radius" -> [_ _ w614 _]
          tunnel: w566 -> [w576 w603 w612 _]
          tunnel: [w576 w603 w613 cluster{i32, i32, i32, i32}[] []] -> w565
          tunnel: w563 -> [_ _ w605 _]
          event Timeout {
            n306 = event-data() -> ()  [unwired: 1 in, 2 out]
            n307 = call <vilib>:"IMAQ Grab Acquire.vi"("error in (no error)"=w584, "Image In"=w583, "IMAQ Session In"=w585) -> ("error out"=w580:errorcluster, "Image Out"=w581:T3, "IMAQ Session Out"=w582:refnum<k11>)  [unwired: 5 in, 1 out]
            n308 = case shown="True" "trap\nmarkers?" {
              tunnel: w576 -> [_ w593]
              tunnel: w581 -> [w587 w592]
              tunnel: w580 -> [w586 w591]
              tunnel: [w586 w590] -> w579
              tunnel: [w587 w588] -> w578
              frame False {
              }
              frame True {
                n309 = for {
                  tunnel: w593 -> [w599] mode=indexing
                  shift-right: [w597] -> w588
                  shift-left: w592 -> [w598]
                  tunnel: w591 -> [w596]
                  tunnel: [w595] -> w590
                  tunnel: u32 16711680 ("Color") -> [w594]
                  n310 = call "IMAQ Overlay Oval"("Color"=w594, "error in (no error)"=w596, "Bounding Rectangle"=w599, "Image"=w598) -> ("error out"=w595:errorcluster, "Image Out"=w597:T3)  [unwired: 6 in]
                }
              }
            }
            "Primary Video Display" <- w578
            n311 = Unbundle By Name(w580) -> ("status"=w575:bool)
          }
          event "Stop All": Value Change {
            n312 = event-data() -> ()  [unwired: 1 in, 5 out]
            n313 = local read "Stop All"() -> (w604:bool)
          }
          event "Primary Video Display": Mouse Down {
            n314 = event-data() -> ()  [unwired: 1 in, 7 out]
            n315 = Array Size(array=w612) -> (size(s)=w611:i32)
            n316 = Less?(x=w611, y=w605) -> (x < y?=w610:bool)
            n317 = case shown="True" w610 {
              tunnel: w614 -> [_ w624]
              tunnel: w612 -> [w615 w618]
              tunnel: [w615 w617] -> w613
              frame False {
              }
              frame True {
                n318 = property on="Primary Video Display" class="ImageControl"() -> ("Last Mouse Position"=w616:cluster{"X":i32, "Y":i32})  [unwired: 2 in, 2 out]
                n319 = Unbundle By Name(w616) -> ("X"=w626:i32, "Y"=w625:i32)
                n320 = Add(x=w625, y=w624) -> (x+y=w622:i32)
                n321 = Subtract(x=w625, y=w624) -> (x-y=w620:i32)
                n322 = Add(x=w626, y=w624) -> (x+y=w621:i32)
                n323 = Subtract(x=w626, y=w624) -> (x-y=w623:i32)
                n324 = Bundle(w623, w622, w621, w620) -> (w619:cluster{i32, i32, i32, i32})  [unwired: 1 in]
                n325 = Build Array (concatenate)(w618, w619) -> (w617:T28)
              }
            }
          }
          event "clear markers": Value Change {
            n326 = event-data() -> ()  [unwired: 1 in, 5 out]
          }
        }
        n327 = node-c288() -> ()  [unwired: 1 in, 1 out]
      }
      n328 = node-c288(w545) -> ()  [unwired: 1 out]
      n329 = Set File Position(offset (in bytes) (0)=i64 0, refnum=w526, from (0:start)=enum16{"start", "end", "current"}."start") -> (refnum out=w527:refnum<file>)  [unwired: 1 in, 1 out]
      n330 = for "Write trap positions to file so they can be remembered\nwhen program is removed from memory" {
        tunnel: w535 -> [w559] mode=indexing
        tunnel: [w557] -> w534
        tunnel: w527 -> [w556]
        n331 = Cluster To Array(cluster=w559) -> (array=w558:i32[])
        n332 = for {
          tunnel: w558 -> [w562] mode=indexing
          tunnel: [w561] -> w557
          tunnel: w556 -> [w560]
          n333 = Write to Binary File(file (use dialog)=w560, data=w562) -> (refnum out=w561:refnum<file>)  [unwired: 4 in, 2 out]
        }
      }
      n334 = Close File(refnum=w534) -> ()  [unwired: 1 in, 2 out]
      n335 = call "IMAQ Dispose"("Image"=w519, "error in (no error)"=w517) -> ("error out"=w516:errorcluster)  [unwired: 4 in]
      n336 = call <vilib>:"IMAQ Stop.vi"("error in (no error)"=w516, "IMAQ Session In"=w518) -> ("error out"=w520:errorcluster, "IMAQ Session Out"=w521:refnum<k11>)  [unwired: 8 in]
      n337 = call <vilib>:"IMAQ Close.vi"("error in (no error)"=w520, "IMAQ Session In"=w521) -> ()  [unwired: 9 in, 1 out]
    }
    frame Enabled {
    }
  }
  n338 = disable-structure shown="Enabled" {
    disable-tunnel: [w637 _] -> w35
    disable-tunnel: w24 -> [w636 _]
    frame Enabled {
      n339 = node-c288() -> (w639:T24)  [unwired: 4 out]
      n340 = timed-loop "Rough control of MCL mirror stage (debugging)" {
        tunnel: w636 -> [w642]
        tunnel: [w641] -> w637
        timing: w639 -> [_]
        timing-out: [_] -> w638
        stop <- w641 stop-if-true
        n341 = node-c288() -> ()  [unwired: 2 out]
        n342 = case shown="1" "MCL Mode" {
          tunnel: w642 -> [_ w645 w692]
          frame 0, Default {
            # "manual positioning"
          }
          frame 1 {
            # "sinusoidal wave"
            n343 = node-c288() -> (w647:T24)  [unwired: 4 out]
            n344 = timed-loop "Oscillate MCL mirror" {
              timing: w647 -> [_]
              timing-out: [_] -> w646
              tunnel: w645 -> [w686]
              i -> [w685]
              stop <- w648 stop-if-true
              n345 = node-c288() -> (w684:i64)  [unwired: 1 out]
              n346 = Multiply(x="AO1", y=32767.0) -> (x*y=w680:dbl)
              n347 = Multiply(x="AO2", y=32767.0) -> (x*y=w675:dbl)
              n348 = Divide(x=w680, y=10.0) -> (x/y=w681:dbl)
              n349 = Divide(x=w675, y=10.0) -> (x/y=w676:dbl)
              n350 = To Word Integer(number=w681) -> (16bit integer=w673:i16)
              n351 = To Word Integer(number=w676) -> (16bit integer=w672:i16)
              n352 = Divide(x=w684, y=i64 1000) -> (x/y=w655:dbl)
              n353 = Multiply(x=w655, y=w685) -> (x*y=w666:dbl)
              n354 = Multiply(x="Osc. freq. (Hz) 2", y=6.283185307179586) -> (x*y=w667:dbl)
              n355 = Multiply(x=w667, y=w666) -> (x*y=w665:dbl)
              n356 = Sine(x=w665) -> (sin(x)=w664:dbl)
              n357 = Multiply(x=w664, y="Osc. amp. (V)") -> (x*y=w662:dbl)
              n358 = Add(x=w662, y="Osc. center (V)") -> (x+y=w660:dbl)
              n359 = Divide(x=w660, y=10.0) -> (x/y=w658:dbl)
              n360 = Multiply(x=w658, y=32767.0) -> (x*y=w653:dbl)
              n361 = Select(t=w653, s="Scan axis", f=w673) -> (s? t:f=w671:dbl)
              n362 = Select(t=w672, s="Scan axis", f=w653) -> (s? t:f=w670:dbl)
              n363 = local read "MCL Mode"() -> (w652:u16)
              n364 = Not Equal?(x=w652, y=u16 1) -> (x != y?=w649:bool)
              n365 = local read "Stop All"() -> (w650:bool)
              n366 = xnode "Read/Write Control"("FPGA VI Reference In"=w686, "AO1"=w671, "AO2"=w670) -> ()  [unwired: 1 in, 2 out]
              n367 = Compound Arithmetic op=OR(w650, w649) -> (w648:bool)
              n368 = node-c288() -> ()  [unwired: 2 out]
            }
            n369 = node-c288(w646) -> ()  [unwired: 1 out]
          }
          frame 2 {
            # "linear scan"
            n370 = case shown="True" "Start Scan" {
              tunnel: w692 -> [_ w704]
              frame False {
              }
              frame True {
                n371 = Subtract(x="End (V)", y="Begin (V)") -> (x-y=w700:dbl)
                n372 = Decrement(x="N Points") -> (x-1=w699:dbl)
                n373 = Divide(x=w700, y=w699) -> (x/y=w697:dbl)
                n374 = for {
                  N: "N Points" -> [_]
                  tunnel: "Begin (V)" -> [w717]
                  tunnel: w704 -> [w709]
                  tunnel: [w708] -> w703 mode=indexing
                  tunnel: w697 -> [w707]
                  tunnel: [w705] -> w696 mode=indexing
                  i -> [w716]
                  n375 = Multiply(x=w707, y=w716) -> (x*y=w715:dbl)
                  n376 = Add(x=w717, y=w715) -> (x+y=w712:dbl)
                  n377 = local read "Scan axis"() -> (w706:bool)
                  n378 = local read "AO1"() -> (w714:dbl)
                  n379 = local read "AO2"() -> (w713:dbl)
                  n380 = Select(t=w712, s=w706, f=w714) -> (s? t:f=w711:dbl)
                  n381 = Select(t=w713, s=w706, f=w712) -> (s? t:f=w710:dbl)
                  n382 = flat-sequence {
                    tunnel: w711 -> [w721]
                    tunnel: w710 -> [w720]
                    tunnel: w709 -> [w718]
                    tunnel: [w731] -> w708
                    tunnel: [w730] -> w705
                    frame #0 {
                      w724 = 10.0 ("y")
                      w719 = 32767.0 ("y")
                      n383 = Multiply(x=w721, y=w719) -> (x*y=w727:dbl)
                      n384 = Multiply(x=w720, y=w719) -> (x*y=w725:dbl)
                      n385 = Divide(x=w727, y=w724) -> (x/y=w728:dbl)
                      n386 = Divide(x=w725, y=w724) -> (x/y=w726:dbl)
                      n387 = To Word Integer(number=w728) -> (16bit integer=w722:i16)
                      n388 = To Word Integer(number=w726) -> (16bit integer=w723:i16)
                      n389 = xnode "Read/Write Control"("FPGA VI Reference In"=w718, "AO1"=w722, "AO2"=w723) -> ()  [unwired: 1 in, 2 out]
                    }
                    frame #1 {
                      n390 = Wait (ms)(milliseconds to wait="DAQ Delay (ms)") -> ()  [unwired: 1 out]
                    }
                    frame #2 {
                      n391 = local read "Slow mean"() -> (w731:dbl)
                      n392 = local read "Sigma"() -> (w730:dbl)
                    }
                  }
                }
                n393 = Bundle("Begin (V)"="Begin (V)", w697, w703) -> (→"MCL Scan":cluster{"Begin (V)":dbl, dbl, dbl[]})  [unwired: 1 out]
                n394 = Bundle("Begin (V)"="Begin (V)", w697, w696) -> (→"MCL Scan 2":cluster{"Begin (V)":dbl, dbl, dbl[]})  [unwired: 1 out]
              }
            }
          }
        }
        n395 = local read "Stop All"() -> (w641:bool)
        n396 = node-c288() -> ()  [unwired: 2 out]
      }
      n397 = node-c288(w638) -> ()  [unwired: 1 out]
    }
    frame Disabled {
    }
  }
  n398 = node-c288(2 ("Processor")) -> (w15:T24)  [unwired: 3 in]
  n399 = node-c288() -> (w69:T24)  [unwired: 4 in]
  n400 = timed-loop "Control parameters (event loop)" {
    tunnel: w24 -> [w737]
    shift-right: [w736] -> _
    shift-left: errorcluster {"status"=FALSE, "code"=0, "source"=""} ("error out") -> [w735]
    tunnel: [w734] -> w37
    timing: w15 -> [_]
    timing-out: [_] -> w14
    stop <- w734 stop-if-true
    n401 = node-c288() -> ()  [unwired: 1 in, 1 out]
    n402 = event shown="[18] \"AI2 to Setpoint\", \"Trap Intensity Setpoints (V)\": Value Change" {
      selector: _ -> [_ _ _ _ _ _ _ _ _ _ _ _ _ _ _ _ _ _ _ _ _ _ _ _ _ _ _ _ _ _ _ _ _ _ _ _ _ _ _ _ _ _ _ _ _ _ _ _ _ _ _ _ _ _ _ _]
      dyn-events: _ -> [_ _ _ _ _ _ _ _ _ _ _ _ _ _ _ _ _ _ _ _ _ _ _ _ _ _ _ _ _ _ _ _ _ _ _ _ _ _ _ _ _ _ _ _ _ _ _ _ _ _ _ _ _ _ _ _]
      timeout: _ -> [_ _ _ _ _ _ _ _ _ _ _ _ _ _ _ _ _ _ _ _ _ _ _ _ _ _ _ _ _ _ _ _ _ _ _ _ _ _ _ _ _ _ _ _ _ _ _ _ _ _ _ _ _ _ _ _]
      tunnel: w737 -> [w775 _ _ _ w812 _ w834 _ w901 _ _ _ w944 _ _ w987 w993 w998 w1004 w1040 w1058 w1065 w1083 w1094 w1105 w1116 w1127 w1138 w1156 w1162 w1256 _ w1265 w1303 _ w1338 w1342 w1353 w1357 w1361 _ w1369 _ _ _ _ _ w1505 _ w1522 w1525 w1534 w1537 w1541 _ w1558]
      tunnel: [w774 _ _ _ w802 _ w833 _ w864 _ w909 _ w923 _ _ w986 w989 w995 w1001 w1039 w1056 w1064 w1077 w1088 w1099 w1110 w1121 w1132 w1154 w1161 w1254 _ w1263 w1301 _ w1336 w1340 w1343 w1355 w1359 _ w1367 _ _ _ _ _ w1503 _ _ _ _ _ _ _ _] -> w736
      tunnel: w735 -> [w773 _ _ _ w811 _ w832 _ w896 _ w909 _ w943 _ _ w985 w988 w994 w1000 w1038 w1057 w1063 w1082 w1093 w1104 w1115 w1126 w1137 w1155 w1160 w1255 _ w1264 w1302 _ w1337 w1341 w1352 w1356 w1360 _ w1368 _ _ _ _ _ w1504 _ w1521 w1524 w1533 w1536 w1540 _ w1557]
      tunnel: [_ _ _ _ _ _ _ _ _ _ w908 _ _ _ _ _ _ _ _ _ _ _ _ _ _ _ _ _ _ _ _ _ _ _ _ _ _ _ _ _ _ _ _ _ _ _ _ _ _ _ _ _ _ _ _ _] -> w734
      tunnel: [_ _ _ _ _ _ _ "Round T1 X" _ _ _ _ _ _ _ _ _ _ _ _ _ _ _ _ _ _ _ _ _ _ _ _ _ _ _ _ _ _ _ _ _ _ _ _ _ _ _ _ _ _ _ _ _ _ _ _] -> _
      tunnel: [_ _ _ "Adjust Scale\nto Mean" _ _ _ _ _ _ _ _ _ _ _ _ _ _ _ _ _ _ _ _ _ _ _ _ _ _ _ _ _ _ _ _ _ _ _ _ _ _ _ _ _ _ _ _ _ _ _ _ _ "Set SP to Reading" _ _] -> _
      tunnel: [_ _ _ _ _ _ _ _ _ "Round T2 X" _ "Delayed Interlace Start" _ _ _ _ _ _ _ _ _ _ _ _ _ _ _ _ _ _ _ _ _ _ _ _ _ _ _ _ _ _ _ _ _ _ _ _ _ _ _ _ _ _ _ _] -> _
      event "AI Count (ticks)", "Sets to FIFO (Traps)", "Save ave N", "FPGA Ave.", "# Samples/channel", "N sets to save": Value Change {
        # "So that if 'Save ave N' is updated, the AOD scanning code updates too."
        n403 = event-data() -> ()  [unwired: 6 out]
        n404 = local read "AI Count (ticks)"() -> (w755:u32)
        n405 = Boolean To (0,1)(Boolean="Sets to FIFO (Traps)") -> (0, 1=w765:cluster{"Set 1":i16, "Set 2":i16, "Set 3":i16})
        n406 = xnode "Read/Write Control"("FPGA VI Reference In"=w775, "error in"=w773, "ai count"=w755, "AI1 Sets to FIFO"="Sets to FIFO (Traps)", "N of AI1 Int Acq Sets"="N Acq Sets (Traps + Fl.)") -> ("error out"=w774:errorcluster)  [unwired: 1 out]
        n407 = Cluster To Array(cluster=w765) -> (array=w764:i16[])
        n408 = To Unsigned Long Integer(number=w764) -> (unsigned 32bit integer=w744:u32[])
        n409 = local read "Scan steps (AOD)"() -> (w766:u64)
        n410 = Multiply(x=w755, y="N Acq Sets (Traps + Fl.)") -> (x*y=w753:u32)
        n411 = Divide(x=40000000.0, y=w755) -> (x/y=w747:dbl)
        "AI rate (Hz)" <- w747
        "Ave. Rate (Hz)" <- w747
        n412 = Add Array Elements(numeric array=w744) -> (sum=w756:u32)
        "Trap Sets" <- w756
        n413 = Reciprocal(x=w747) -> (1/x=→"Ave. Period (s)":dbl)
        n414 = property on="Scan steps (AOD)" class="DigNum (strict)"("Val(Sgnl)"=w766) -> ()  [unwired: 2 in, 2 out]
        n415 = Divide(x=w747, y="N Acq Sets (Traps + Fl.)") -> (x/y=w770:dbl)
        "Data Rate (Hz)" <- w770
        n416 = Reciprocal(x=w770) -> (1/x=→"Data Period (s)":dbl)
        n417 = local read "Save ave N"() -> (w769:dbl)
        n418 = Divide(x=w770, y=w769) -> (x/y=w768:dbl)
        "Save Data Rate (Hz)" <- w768
        n419 = Reciprocal(x=w768) -> (1/x=→"Save Data Period (s)":dbl)
        n420 = Multiply(x=w753, y="# Samples/trap") -> (x*y=w751:u32)
        "Counts/DMA" <- w751
        n421 = property on="Trap Disp. Downsample" class="DigNum (strict)"("Maximum"="# Samples/trap") -> ()  [unwired: 2 in, 2 out]
        n422 = Multiply(x=w756, y="# Samples/trap") -> (x*y=w745:u32)
        "# Samples/channel" <- w745
        n423 = Multiply(x=w745, y=u32 8) -> (x*y=→"Trap AI Elements/DMA read":u32)
        n424 = local read "APD Int. Count"() -> (w752:u32)
        n425 = Multiply(x=w745, y=u32 3) -> (x*y=→"Trap Pos Elements/DMA read":u32)
        n426 = Divide(x=w751, y=w752) -> (x/y=w742:dbl)
        "APD Samples/FIFO Acq." <- w742
        n427 = Divide(x=w751, y=40000000.0) -> (x/y=w749:dbl)
        "DMA Update Period (s)" <- w749
        n428 = Multiply(x=2.0, y=w742) -> (x*y=→"APD Elements/DMA read":dbl)
        n429 = property on="APD Disp. Downsample" class="DigNum (strict)"("Maximum"=w742) -> ()  [unwired: 2 in, 2 out]
        n430 = local read "N sets to save"() -> (w762:u32)
        n431 = Multiply(x=w749, y=w762) -> (x*y=→"Total Time (s)":dbl)
        "FPGA Averaging" <- FALSE ("FPGA Averaging")
      }
      event "Rescale on Mean": Value Change {
        n432 = event-data() -> ()  [unwired: 7 out]
        n433 = And(x=FALSE, y="Rescale on Mean") -> (x .and. y?=w777:bool)
        n434 = local write "Rescale on Mean"(w777) -> ()
        n435 = local read "Bead Mean (nm)"() -> (w782:dbl)
        n436 = Add(x="Amplitude (nm)", y=w782) -> (x+y=w780:dbl)
        n437 = Subtract(x=w782, y="Amplitude (nm)") -> (x-y=w779:dbl)
        n438 = property on="Bead Separation" class="WFChart (strict)"("YScale.Minimum"=w779) -> ()  [unwired: 2 in, 2 out]
        n439 = property on="Bead Separation" class="WFChart (strict)"("YScale.Maximum"=w780) -> ()  [unwired: 2 in, 2 out]
      }
      event "Detector Type": Value Change {
        n440 = event-data() -> ()  [unwired: 7 out]
        n441 = local read "AI labels"() -> (w783:string[])
        n442 = property on="High Res. Display" class="Ring (strict)"("Strings []"=w783) -> ()  [unwired: 2 in, 2 out]
        n443 = Build Array (concatenate)(w783, "none") -> (w784:string[])
        n444 = property on="FFT 1 Choice 1" class="Ring (strict)"("Strings []"=w784) -> ()  [unwired: 2 in, 2 out]
        n445 = property on="FFT 1 Choice 2" class="Ring (strict)"("Strings []"=w784) -> ()  [unwired: 2 in, 2 out]
        n446 = property on="FFT 2 Choice 1" class="Ring (strict)"("Strings []"=w784) -> ()  [unwired: 2 in, 2 out]
        n447 = property on="FFT 2 Choice 2" class="Ring (strict)"("Strings []"=w784) -> ()  [unwired: 2 in, 2 out]
        n448 = Bundle("APD 1", "APD 2") -> (w787:cluster{string, string})  [unwired: 1 out]
        n449 = Cluster To Array(cluster=w787) -> (array=w785:string[])
        n450 = Build Array (concatenate)(w785, w784) -> (w789:string[])
        n451 = Array Size(array=w789) -> (size(s)=w790:i32)
        n452 = property on="Signals to Plot" class="LstBox (strict)"("Item Names"=w789) -> ()  [unwired: 2 in, 2 out]
        n453 = property on="Signals to Plot" class="LstBox (strict)"("Number of Rows"=w790) -> ()  [unwired: 2 in, 2 out]
        n454 = property on="All Signals" class="WFChart (strict)"("LegNumRows"=w790) -> ()  [unwired: 2 in, 2 out]
      }
      event "Adjust Scale\nto Mean": Value Change {
        n455 = event-data() -> ()  [unwired: 7 out]
        n456 = local read "APD 1 Rate (Hz)"() -> (w799:dbl)
        n457 = Multiply(x=1000.0, y="Above (kHz)") -> (x*y=w797:dbl)
        n458 = Multiply(x=1000.0, y="Below (kHz)") -> (x*y=w795:dbl)
        n459 = Add(x=w797, y=w799) -> (x+y=w792:dbl)
        n460 = Subtract(x=w799, y=w795) -> (x-y=w793:dbl)
        n461 = property on="APD Chart" class="WFChart (strict)"("YScale.Minimum"=w793) -> ()  [unwired: 2 in, 2 out]
        n462 = property on="APD Chart" class="WFChart (strict)"("YScale.Maximum"=w792) -> ()  [unwired: 2 in, 2 out]
      }
      event "Phase adj. (AI1)", "+ phase (AI1)", "- phase (AI1)": Value Change {
        n463 = event-data() -> ()  [unwired: 7 out]
        n464 = Negate(x="Phase adj. (AI1)") -> (-x=w809:i16)
        n465 = Select(t=w809, s="- phase (AI1)", f="Phase adj. (AI1)") -> (s? t:f=w808:i16)
        n466 = xnode "Read/Write Control"("FPGA VI Reference In"=w812, "error in"=w811, "Phase count adjustment"=w808) -> ("FPGA VI Reference Out"=w807:T19, "error out"=w806:errorcluster)
        n467 = Or(x="- phase (AI1)", y="+ phase (AI1)") -> (x .or. y?=w803:bool)
        n468 = xnode "Read/Write Control"("FPGA VI Reference In"=w807, "error in"=w806, "+ phase"=w803) -> ("error out"=w802:errorcluster)  [unwired: 1 out]
      }
      event "Signals to Plot": Double Click {
        w815 = u32 9868950 ("Color Box")
        n469 = event-data() -> ("Row"=w817:i32)  [unwired: 9 out]
        n470 = property on="All Signals" class="WFChart (strict)"("Active Plot"=w817) -> (error out=w828:errorcluster)  [unwired: 2 in, 1 out]
        n471 = property on="All Signals" class="WFChart (strict)" props=["Plot", "Visible?", "Plot", "Plot Color"](error in=w828) -> (error out=w827:errorcluster, "Plot.Visible?"=w826:bool)  [unwired: 1 in, 2 out]
        n472 = Select(t=FALSE ("Plot.Visible"), s=w826, f=TRUE ("Plot.Visible")) -> (s? t:f=w821:bool)
        n473 = property on="All Signals" class="WFChart (strict)"(error in=w827, "Plot.Visible?"=w821) -> (error out=w823:errorcluster)  [unwired: 1 in, 1 out]
        n474 = property on="All Signals" class="WFChart (strict)"(error in=w823) -> (error out=w818:errorcluster, "Plot.Plot Color"=w822:u32)  [unwired: 1 in, 1 out]
        n475 = property on="Signals to Plot" class="LstBox (strict)"(error in=w818, "Active Row"=w817) -> (error out=w816:errorcluster)  [unwired: 1 in, 1 out]
        n476 = Select(t=w822, s=w821, f=u32 0) -> (s? t:f=w819:u32)
        n477 = property on="Signals to Plot" class="LstBox (strict)"(error in=w816, "CellFontColor"=w819, "SelColor"=w815, "CellBG"=w815, "CellFontSize"=u32 20 ("Active Row:Cell Font:Size"), "CellFontBold"=TRUE ("Active Row:Cell Font:Bold")) -> ()  [unwired: 1 in, 2 out]
      }
      event "BD 1 Frequency 1 (MHz)", "BD 1 Frequency 2 (MHz)", "BD 1 Frequency 3 (MHz)", "BD 2 Frequency 1 (MHz)", "BD 2 Frequency 2 (MHz)", "BD 2 Frequency 3 (MHz)", "Trap Delta (MHz)": Value Change {
        # "anytime one of the frequencies is changed, write it to the RF board UNLESS Set 2 is being oscillated. The oscillation\nscript writes the frequencies to the RF board."
        n478 = event-data() -> ("CtlRef"=w831:refnum<vi>)  [unwired: 6 out]
        n479 = control-ref of="Trap Delta (MHz)"() -> (w830:refnum<vi>)
        n480 = Equal?(x=w830, y=w831) -> (x = y?=w829:bool)
        n481 = case shown="False" "Oscillate Set 2" {
          tunnel: w834 -> [w857 _]
          tunnel: [w856 w860] -> w833
          tunnel: w832 -> [w855 w860]
          tunnel: w829 -> [w842 _]
          frame False {
            w836 = 80
            n482 = local read "BD 1 Frequency 2 (MHz)"() -> (w844:dbl)
            n483 = Divide(x="Trap Delta (MHz)", y=2) -> (x/y=w838:dbl)
            n484 = Subtract(x=w836, y=w838) -> (x-y=w837:dbl)
            n485 = local write "BD 1 Frequency 1 (MHz)"(w837) -> ()
            n486 = Add(x=w836, y=w838) -> (x+y=w843:dbl)
            n487 = Select(t=w843, s=w842, f=w844) -> (s? t:f=w841:dbl)
            n488 = local read "Y RF Frequency Limits (MHz)"() -> (w845:T16)
            n489 = local read "X RF Frequency Limits (MHz)"() -> (w846:T16)
            n490 = local read "BD 1 Frequency 3 (MHz)"() -> (w858:dbl)
            n491 = local write "BD 1 Frequency 2 (MHz)"(w841) -> ()
            n492 = local read "BD 2 Frequency 1 (MHz)"() -> (w849:dbl)
            n493 = local read "BD 2 Frequency 2 (MHz)"() -> (w848:dbl)
            n494 = local read "BD 2 Frequency 3 (MHz)"() -> (w859:dbl)
            n495 = call "set RF board frequency - interlace.vi"("Board 2 Frequency Limits"=w845, "Board 1 Frequency Limits"=w846, "error in"=w855, "FPGA VI Reference In"=w857, "Board 2 Frequency 3 (MHz)"=w859, "Board 1 Frequency 3 (MHz)"=w858, "Board 2 Frequency 2 (MHz)"=w848, "Board 2 Frequency 1 (MHz)"=w849, "Board 1 Frequency 2 (MHz)"=w841, "Board 1 Frequency 1  (MHz)"=w837) -> ("error out"=w856:errorcluster)  [unwired: 1 out]
            n496 = Subtract(x=w849, y=w848) -> (x-y=w853:dbl)
            n497 = Subtract(x=w841, y=w837) -> (x-y=w854:dbl)
            n498 = Square(x=w853) -> (x^2=w851:dbl)
            n499 = Square(x=w854) -> (x^2=w852:dbl)
            n500 = Add(x=w852, y=w851) -> (x+y=w850:dbl)
            n501 = Square Root(x=w850) -> (sqrt(x)=w847:dbl)
            n502 = local write "Trap Delta (MHz)"(w847) -> ()
            n503 = property on="Initial delta (MHz)" class="DigNum (strict)"("Val(Sgnl)"=w847) -> ()  [unwired: 2 in, 2 out]
          }
          frame True {
          }
        }
      }
      event "Round T1 X": Value Change {
        n504 = event-data() -> ()  [unwired: 7 out]
        n505 = local read "BD 1 Frequency 1 (MHz)"() -> (w863:dbl)
        n506 = Round To Nearest(number=w863) -> (nearest integer value=w862:dbl)
        n507 = property on="BD 1 Frequency 1 (MHz)" class="DigNum (strict)"("Val(Sgnl)"=w862) -> ()  [unwired: 2 in, 2 out]
      }
      event "Restart RF": Value Change {
        n508 = event-data() -> ()  [unwired: 7 out]
        n509 = xnode "Read/Write Control"("FPGA VI Reference In"=w901, "error in"=w896, "FPGA Controls  RF Box"=FALSE) -> ("FPGA VI Reference Out"=w900:T19, "error out"=w895:errorcluster)
        n510 = local read "Y RF Amplitude Limits (%)"() -> (w876:T16)
        n511 = local read "X RF Amplitude Limits (%)"() -> (w877:T16)
        n512 = local read "X RF Frequency Limits (MHz)"() -> (w879:T16)
        n513 = local read "Y RF Frequency Limits (MHz)"() -> (w878:T16)
        n514 = xnode "Read/Write Control"("FPGA VI Reference In"=w900, "error in"=w895, "Direct RF Box  Communication"=TRUE) -> ("FPGA VI Reference Out"=w899:T19, "error out"=w894:errorcluster)
        n515 = local read "BD 2 Frequency 3 (MHz)"() -> (w886:dbl)
        n516 = local read "BD 2 Frequency 2 (MHz)"() -> (w887:dbl)
        n517 = local read "BD 1 Frequency 3 (MHz)"() -> (w890:dbl)
        n518 = local read "BD 1 Frequency 1 (MHz)"() -> (w891:dbl)
        n519 = local read "BD 2 Frequency 1 (MHz)"() -> (w888:dbl)
        n520 = local read "BD 1 Frequency 2 (MHz)"() -> (w889:dbl)
        n521 = call "Initialize RF boards - interlace 3.vi"("error in"=w894, "FPGA VI Reference In"=w899) -> ("error out"=w893:errorcluster, "FPGA VI Reference Out"=w898:T19)
        n522 = local read "BD 2 Amplitude 2 (%)"() -> (w881:dbl)
        n523 = local read "BD 2 Amplitude 1 (%)"() -> (w882:dbl)
        n524 = local read "BD 2 Amplitude 3 (%)"() -> (w880:dbl)
        n525 = local read "BD 1 Amplitude 3 (%)"() -> (w885:dbl)
        n526 = local read "BD 1 Amplitude 1 (%)"() -> (w884:dbl)
        n527 = local read "BD 1 Amplitude 2 (%)"() -> (w883:dbl)
        n528 = call "set RF board frequency - interlace.vi"("Board 2 Frequency Limits"=w878, "Board 1 Frequency Limits"=w879, "error in"=w893, "FPGA VI Reference In"=w898, "Board 2 Frequency 3 (MHz)"=w886, "Board 1 Frequency 3 (MHz)"=w890, "Board 2 Frequency 2 (MHz)"=w887, "Board 2 Frequency 1 (MHz)"=w888, "Board 1 Frequency 2 (MHz)"=w889, "Board 1 Frequency 1  (MHz)"=w891) -> ("error out"=w892:errorcluster, "FPGA VI Reference Out"=w897:T19)
        n529 = call "set RF board amplitude - interlace.vi"("Board 2 Amplitude Limits"=w876, "Board 1 Amplitude Limits"=w877, "error in"=w892, "FPGA VI Reference In"=w897, "Board 2 Amplitude 3 (%)"=w880, "Board 1 Amplitude 3 (%)"=w885, "Board 2 Amplitude 2 (%)"=w881, "Board 2 Amplitude 1 (%)"=w882, "Board 1 Amplitude 2 (%)"=w883, "Board 1 Amplitude 1 (%)"=w884) -> ("error out"=w869:errorcluster, "FPGA VI Reference Out"=w873:T19)
        n530 = xnode "Read/Write Control"("FPGA VI Reference In"=w873, "error in"=w869, "Direct RF Box  Communication"=FALSE) -> ("FPGA VI Reference Out"=w872:T19, "error out"=w871:errorcluster)
        n531 = flat-sequence {
          tunnel: w871 -> [w902]
          tunnel: [w902] -> w870
          frame #0 {
            n532 = Wait (ms)(milliseconds to wait=u32 50) -> ()  [unwired: 1 out]
          }
        }
        n533 = xnode "Read/Write Control"("FPGA VI Reference In"=w872, "error in"=w870, "FPGA Controls  RF Box"=TRUE) -> ("error out"=w865:errorcluster)  [unwired: 1 out]
        n534 = property on="Restart RF" class="Bool (strict)"(error in=w865, "Value"=FALSE ("Restart RF")) -> (error out=w864:errorcluster)  [unwired: 1 in, 1 out]
      }
      event "Round T2 X": Value Change {
        n535 = event-data() -> ()  [unwired: 7 out]
        n536 = local read "BD 1 Frequency 2 (MHz)"() -> (w905:dbl)
        n537 = Round To Nearest(number=w905) -> (nearest integer value=w904:dbl)
        n538 = property on="BD 1 Frequency 2 (MHz)" class="DigNum (strict)"("Val(Sgnl)"=w904) -> ()  [unwired: 2 in, 2 out]
      }
      event "Stop All": Value Change {
        n539 = event-data() -> ()  [unwired: 7 out]
        n540 = call "hamilton_controller.vi"("action"=T20."DISCONNECT") -> ()  [unwired: 10 in, 1 out]
        n541 = local read "Stop All"() -> (w908:bool)
      }
      event "Delayed Interlace Start": Value Change {
        n542 = event-data() -> ()  [unwired: 7 out]
        n543 = flat-sequence {
          frame #0 {
            n544 = Multiply(x="Delay to Interlace (s)", y=1000.0) -> (x*y=w911:dbl)
            n545 = Wait (ms)(milliseconds to wait=w911) -> ()  [unwired: 1 out]
          }
          frame #1 {
            n546 = property on="Green laser mode" class="RadioBtnsControl (strict)"("Val(Sgnl)"=enum32{"Laser ON", "Laser OFF", "Interlace"}."Interlace" ("Value (Signaling)")) -> ()  [unwired: 2 in, 2 out]
          }
        }
      }
      event "BD 1 Amplitude 1 (%)", "BD 1 Amplitude 2 (%)", "BD 1 Amplitude 3 (%)", "BD 2 Amplitude 1 (%)", "BD 2 Amplitude 2 (%)", "BD 2 Amplitude 3 (%)", "Trap 1 ON", "Trap 2 ON", "Trap 3 ON", "Feedback On/Off", "All FB On/Off": Value Change {
        w935 = i16 1 ("f")
        n547 = event-data() -> ()  [unwired: 7 out]
        n548 = local write "Trap 1 (ON/OFF)"("Trap 1 ON") -> ()
        n549 = local write "Trap 2 (ON/OFF)"("Trap 2 ON") -> ()
        n550 = Boolean To (0,1)(Boolean="Trap 3 ON") -> (0, 1=w936:i16)
        n551 = Boolean To (0,1)(Boolean="Trap 1 ON") -> (0, 1=w937:i16)
        n552 = Boolean To (0,1)(Boolean="Trap 2 ON") -> (0, 1=w938:i16)
        n553 = Select(t=w938, s="Trap ON/OFF X or Y Amp?", f=w935) -> (s? t:f=w933:i16)
        n554 = Select(t=w937, s="Trap ON/OFF X or Y Amp?", f=w935) -> (s? t:f=w934:i16)
        n555 = Select(t=w936, s="Trap ON/OFF X or Y Amp?", f=w935) -> (s? t:f=w932:i16)
        n556 = Select(t=w935, s="Trap ON/OFF X or Y Amp?", f=w938) -> (s? t:f=w930:i16)
        n557 = Select(t=w935, s="Trap ON/OFF X or Y Amp?", f=w937) -> (s? t:f=w931:i16)
        n558 = Select(t=w935, s="Trap ON/OFF X or Y Amp?", f=w936) -> (s? t:f=w929:i16)
        n559 = And(x="All FB On/Off", y="Feedback On/Off") -> (x .and. y?=w927:cluster{"Set 1":bool, "Set 2":bool})
        n560 = local read "BD 1 Amplitude 1 (%)"() -> (w947:dbl)
        n561 = local read "BD 1 Amplitude 2 (%)"() -> (w946:dbl)
        n562 = local read "BD 1 Amplitude 3 (%)"() -> (w945:dbl)
        n563 = Unbundle By Name(w927) -> ("Set 1"=w922:bool, "Set 2"=w919:bool)
        n564 = local read "Y RF Amplitude Limits (%)"() -> (w915:T16)
        n565 = local read "X RF Amplitude Limits (%)"() -> (w916:T16)
        n566 = local read "BD 2 Amplitude 1 (%)"() -> (w948:dbl)
        n567 = local read "BD 2 Amplitude 2 (%)"() -> (w949:dbl)
        n568 = local read "BD 2 Amplitude 3 (%)"() -> (w950:dbl)
        n569 = And(x="Trap 2 ON", y=w919) -> (x .and. y?=w917:bool)
        n570 = And(x="Trap 1 ON", y=w922) -> (x .and. y?=w920:bool)
        n571 = Multiply(x=w934, y=w947) -> (x*y=w942:dbl)
        n572 = Multiply(x=w946, y=w933) -> (x*y=w940:dbl)
        n573 = Multiply(x=w945, y=w932) -> (x*y=w941:dbl)
        n574 = Multiply(x=w948, y=w931) -> (x*y=w951:dbl)
        n575 = Multiply(x=w949, y=w930) -> (x*y=w952:dbl)
        n576 = Multiply(x=w950, y=w929) -> (x*y=w953:dbl)
        n577 = call "set RF board amplitude - interlace.vi"("Board 2 Amplitude Limits"=w915, "Board 1 Amplitude Limits"=w916, "error in"=w943, "FPGA VI Reference In"=w944, "Board 2 Amplitude 3 (%)"=w953, "Board 1 Amplitude 3 (%)"=w941, "Board 2 Amplitude 2 (%)"=w952, "Board 2 Amplitude 1 (%)"=w951, "Board 1 Amplitude 2 (%)"=w940, "Board 1 Amplitude 1 (%)"=w942) -> ("error out"=w924:errorcluster, "FPGA VI Reference Out"=w925:T19)
        n578 = xnode "Read/Write Control"("FPGA VI Reference In"=w925, "error in"=w924, "FB On/Off Set 1"=w920, "FB On/Off Set 2"=w917) -> ("error out"=w923:errorcluster)  [unwired: 1 out]
      }
      event "Load parameters": Value Change {
        n579 = event-data() -> ()  [unwired: 7 out]
        n580 = property on="Saved AOD Raster Scan Parameter Sets" class="Arr (strict)"() -> ("Index Values"=w964:u32[])  [unwired: 2 in, 2 out]
        n581 = Index Array(array=w964, index=0) -> (element=w961:u32)
        n582 = local write "Load parameters"(FALSE ("Load parameters")) -> ()
        n583 = Index Array(array="Saved AOD Raster Scan Parameter Sets", index=w961) -> (element=w960:T30)
        n584 = Unbundle By Name(w960) -> ("Scan Range AOD (nm) 2"=w959:dbl, "Step Size AOD (nm) 2"=w958:dbl, "Scan Speed AOD (nm/s) 2"=w957:dbl, "Number of scans (AOD) 2"=w956:u16)
        n585 = flat-sequence {
          tunnel: w959 -> [w967]
          tunnel: w958 -> [w966]
          tunnel: w957 -> [w965]
          tunnel: w956 -> [w968]
          frame #0 {
            n586 = local write "Scan Speed (nm/s)"(w965) -> ()
            n587 = local write "Scan Range (nm)"(w967) -> ()
            n588 = local write "Step Size (nm)"(w966) -> ()
          }
          frame #1 {
            n589 = property on="Number of F/B Scans (AOD)" class="DigNum (strict)"("Val(Sgnl)"=w968) -> ()  [unwired: 2 in, 2 out]
          }
        }
      }
      event "Trap 1 (ON/OFF)", "Trap 2 (ON/OFF)": Value Change {
        n590 = event-data() -> ()  [unwired: 7 out]
        n591 = property on="Trap 2 ON" class="Bool (strict)"("Val(Sgnl)"="Trap 2 (ON/OFF)") -> ()  [unwired: 2 in, 2 out]
        n592 = property on="Trap 1 ON" class="Bool (strict)"("Val(Sgnl)"="Trap 1 (ON/OFF)") -> ()  [unwired: 2 in, 2 out]
      }
      event "DIO count 1 (ticks)", "DIO count 2 (ticks)", "DIO count 3 (ticks)", "Interlace", "Number Interlace Sets", "Not-Interlacing Set": Value Change {
        n593 = event-data() -> ()  [unwired: 7 out]
        n594 = local read "DIO count 3 (ticks)"() -> (w981:u32)
        n595 = local read "DIO count 1 (ticks)"() -> (w983:u32)
        n596 = local read "DIO count 2 (ticks)"() -> (w982:u32)
        n597 = To Unsigned Byte Integer(number="Not-Interlacing Set") -> (unsigned 8bit integer=w972:u8)
        n598 = Add(x=w972, y=u8 1) -> (x+y=w976:u8)
        n599 = xnode "Read/Write Control"("FPGA VI Reference In"=w987, "error in"=w985, "DIO count 1 (ticks)"=w983, "DIO count 2 (ticks)"=w982, "DIO count 3 (ticks)"=w981, "Interlace ON/OFF"="Interlace", "Number Interlace Cycles"="Number Interlace Sets", "Interlace Off Parameters"=w976) -> ("error out"=w986:errorcluster)  [unwired: 1 out]
        n600 = Build Array(w983, w982, w981) -> (w974:u32[])
        n601 = Split 1D Array(array=w974, index="Number Interlace Sets") -> (first subarray=w984:u32[])  [unwired: 1 out]
        n602 = Index Array(array=w974, index=w972) -> (element=w973:u32)
        n603 = Add Array Elements(numeric array=w984) -> (sum=w978:u32)
        n604 = Select(t=w978, s="Interlace", f=w973) -> (s? t:f=→"Total Counts (ticks)":u32)
      }
      event "Reset Feedback": Value Change {
        n605 = event-data() -> ()  [unwired: 7 out]
        n606 = Unbundle By Name("Reset Feedback") -> ("Set 1"=w991:bool, "Set 2"=w990:bool)
        n607 = xnode "Read/Write Control"("FPGA VI Reference In"=w993, "error in"=w988, "FB Reset Set 1"=w991, "FB Reset Set 2"=w990) -> ("error out"=w989:errorcluster)  [unwired: 1 out]
      }
      event "PID Gains": Value Change {
        n608 = event-data() -> ()  [unwired: 7 out]
        n609 = Unbundle By Name("PID Gains") -> ("Set 1"=w997:T14, "Set 2"=w996:T14)
        n610 = xnode "Read/Write Control"("FPGA VI Reference In"=w998, "error in"=w994, "FB Gains Set 1"=w997, "FB Gains Set 2"=w996) -> ("error out"=w995:errorcluster)  [unwired: 1 out]
      }
      event "AI2 to Setpoint", "Trap Intensity\nSetpoints (V)": Value Change {
        n611 = event-data() -> ()  [unwired: 7 out]
        n612 = xnode "Read/Write Control"("FPGA VI Reference In"=w1004, "error in"=w1000) -> ("FPGA VI Reference Out"=w1003:T19, "error out"=w1002:errorcluster, "AI4 Y Sum Set 1"=w1011:i16, "AI4 Y Sum Set 2"=w1010:i16)
        n613 = Cluster To Array(cluster="AI2 to Setpoint") -> (array=w1014:bool[])
        n614 = local read "AI2 (V)"() -> (w1012:cluster{"Set 1":dbl, "Set 2":dbl})
        n615 = Or Array Elements(Boolean array=w1014) -> (logical OR=w1015:bool)
        n616 = Bundle By Name(cluster=w1012, "Set 1"=w1011, "Set 2"=w1010) -> (w1009:cluster{"Set 1":dbl, "Set 2":dbl})
        n617 = Divide(x=w1009, y=3276.7) -> (x/y=w1008:cluster{"Set 1":dbl, "Set 2":dbl})
        "AI2 (V)" <- w1008
        n618 = case shown="True" w1015 {
          tunnel: [w1018 w1035] -> w1007
          tunnel: "AI2 to Setpoint" -> [_ w1031]
          tunnel: "Trap Intensity\nSetpoints (V)" -> [w1019 w1034]
          tunnel: w1008 -> [_ w1028]
          frame False {
            n619 = Multiply(x=3276.7, y=w1019) -> (x*y=w1020:cluster{"Set 1":dbl, "Set 2":dbl})
            n620 = To Word Integer(number=w1020) -> (16bit integer=w1018:cluster{"Set 1":i16, "Set 2":i16})
          }
          frame True {
            n621 = Unbundle By Name(w1028) -> ("Set 1"=w1027:dbl, "Set 2"=w1026:dbl)
            n622 = Unbundle By Name(w1034) -> ("Set 1"=w1033:dbl, "Set 2"=w1032:dbl)
            n623 = Unbundle By Name(w1031) -> ("Set 1"=w1030:bool, "Set 2"=w1029:bool)
            n624 = Select(t=w1027, s=w1030, f=w1033) -> (s? t:f=w1025:dbl)
            n625 = Select(t=w1026, s=w1029, f=w1032) -> (s? t:f=w1024:dbl)
            n626 = Bundle By Name(cluster=w1034, "Set 1"=w1025, "Set 2"=w1024) -> (w1022:cluster{"Set 1":dbl, "Set 2":dbl})
            n627 = local write "Trap Intensity\nSetpoints (V)"(w1022) -> ()
            n628 = Multiply(x=3276.7, y=w1022) -> (x*y=w1023:cluster{"Set 1":dbl, "Set 2":dbl})
            n629 = To Word Integer(number=w1023) -> (16bit integer=w1035:cluster{"Set 1":i16, "Set 2":i16})
          }
        }
        n630 = Unbundle By Name(w1007) -> ("Set 1"=w1006:i16, "Set 2"=w1005:i16)
        n631 = xnode "Read/Write Control"("FPGA VI Reference In"=w1003, "error in"=w1002, "FB Setpoint Set 1"=w1006, "FB Setpoint Set 2"=w1005) -> ("error out"=w1001:errorcluster)  [unwired: 1 out]
      }
      event "Invert GI": Value Change {
        n632 = event-data() -> ()  [unwired: 7 out]
        n633 = xnode "Read/Write Control"("FPGA VI Reference In"=w1040, "error in"=w1038, "Invert GI"="Invert GI", "Invert GI 2"="Invert GI") -> ("error out"=w1039:errorcluster)  [unwired: 1 out]
      }
      event "Green FB Setpoint (mV)", "Green FB Gains", "Green FB On/Off", "Current When FB OFF (%)", "Green int current ON count adj": Value Change {
        n634 = event-data() -> ()  [unwired: 7 out]
        n635 = local read "Green FB Setpoint (mV)"() -> (w1047:dbl)
        n636 = local read "Current When FB OFF (%)"() -> (w1050:dbl)
        n637 = Multiply(x=w1047, y=3.2767) -> (x*y=w1046:dbl)
        n638 = Multiply(x=w1050, y=655.35) -> (x*y=w1051:dbl)
        n639 = To Unsigned Word Integer(number=w1051) -> (unsigned 16bit integer=w1049:u16)
        n640 = local read "Green int current ON count adj"() -> (w1054:u32)
        n641 = local read "Green FB Gains"() -> (w1053:T14)
        n642 = local read "Green Laser ON/Interlacing"() -> (w1044:bool)
        n643 = local read "Green laser mode"() -> (w1043:enum32{"Laser ON", "Laser OFF", "Interlace"})
        n644 = local read "Green FB On/Off"() -> (w1055:bool)
        n645 = Equal?(x=w1043, y=enum32{"Laser ON", "Laser OFF", "Interlace"}."Interlace") -> (x = y?=w1041:bool)
        n646 = Compound Arithmetic op=AND(w1041, w1055, w1044) -> (w1045:bool)
        n647 = xnode "Read/Write Control"("FPGA VI Reference In"=w1058, "error in"=w1057, "Green FB Setpoint"=w1046, "Green FB On/Off"=w1045, "Current Out"=w1049, "Green int current ON count adj"=w1054, "Green FB Gains"=w1053) -> ("error out"=w1056:errorcluster)  [unwired: 1 out]
      }
      event "Green laser mode", "Green Laser ON/Interlacing": Value Change {
        n648 = event-data() -> ()  [unwired: 7 out]
        n649 = case shown="True" "Green Laser ON/Interlacing" {
          tunnel: "Green laser mode" -> [_ w1072]
          tunnel: [enum32{"Laser ON", "Laser OFF", "Interlace"}."Laser OFF" ("Green laser mode") w1072] -> w1060
          tunnel: [FALSE w1068] -> w1059
          frame False {
          }
          frame True {
            n650 = local read "Green FB On/Off"() -> (w1069:bool)
            n651 = Equal?(x=w1072, y=enum32{"Laser ON", "Laser OFF", "Interlace"}."Interlace") -> (x = y?=w1070:bool)
            n652 = And(x=w1070, y=w1069) -> (x .and. y?=w1068:bool)
          }
        }
        n653 = xnode "Read/Write Control"("FPGA VI Reference In"=w1065, "error in"=w1063, "Operating Mode"=w1060, "Operating Mode 2"=w1060, "Green FB On/Off"=w1059) -> ("error out"=w1064:errorcluster)  [unwired: 1 out]
      }
      event "- phase (APD 1 Gate)", "+ phase (APD 1 Gate)": Value Change {
        n654 = event-data() -> ()  [unwired: 7 out]
        n655 = local read "Phase Adj. (APD 1 Gate)"() -> (w1073:i16)
        n656 = Negate(x=w1073) -> (-x=w1081:i16)
        n657 = Select(t=w1081, s="- phase (APD 1 Gate)", f=w1073) -> (s? t:f=w1080:i16)
        n658 = Or(x="- phase (APD 1 Gate)", y="+ phase (APD 1 Gate)") -> (x .or. y?=w1076:bool)
        n659 = xnode "Read/Write Control"("FPGA VI Reference In"=w1083, "error in"=w1082, "Phase count adjustment (APD 1 Gate)"=w1080) -> ("FPGA VI Reference Out"=w1078:T19, "error out"=w1079:errorcluster)
        n660 = xnode "Read/Write Control"("FPGA VI Reference In"=w1078, "error in"=w1079, "+ phase (APD 1 Gate)"=w1076) -> ("error out"=w1077:errorcluster)  [unwired: 1 out]
      }
      event "+ phase (APD 2 Gate)", "- phase (APD 2 Gate)": Value Change {
        n661 = event-data() -> ()  [unwired: 7 out]
        n662 = local read "Phase Adj. (APD 2 Gate)"() -> (w1084:i16)
        n663 = Negate(x=w1084) -> (-x=w1092:i16)
        n664 = Select(t=w1092, s="- phase (APD 2 Gate)", f=w1084) -> (s? t:f=w1091:i16)
        n665 = Or(x="- phase (APD 2 Gate)", y="+ phase (APD 2 Gate)") -> (x .or. y?=w1087:bool)
        n666 = xnode "Read/Write Control"("FPGA VI Reference In"=w1094, "error in"=w1093, "Phase count adjustment (APD 2 Gate)"=w1091) -> ("FPGA VI Reference Out"=w1089:T19, "error out"=w1090:errorcluster)
        n667 = xnode "Read/Write Control"("FPGA VI Reference In"=w1089, "error in"=w1090, "+ phase (APD 2 Gate)"=w1087) -> ("error out"=w1088:errorcluster)  [unwired: 1 out]
      }
      event "Phase Adj. (APD Acq)", "+ phase (APD Acq)", "- phase (APD Acq)": Value Change {
        n668 = event-data() -> ()  [unwired: 7 out]
        n669 = local read "Phase Adj. (APD Acq)"() -> (w1097:i16)
        n670 = Negate(x=w1097) -> (-x=w1103:i16)
        n671 = Select(t=w1103, s="+ phase (APD Acq)", f=w1097) -> (s? t:f=w1102:i16)
        n672 = Or(x="+ phase (APD Acq)", y="- phase (APD Acq)") -> (x .or. y?=w1098:bool)
        n673 = xnode "Read/Write Control"("FPGA VI Reference In"=w1105, "error in"=w1104, "Phase Count Adjustment (APD Acq)"=w1102) -> ("FPGA VI Reference Out"=w1100:T19, "error out"=w1101:errorcluster)
        n674 = xnode "Read/Write Control"("FPGA VI Reference In"=w1100, "error in"=w1101, "+ phase (APD Acq)"=w1098) -> ("error out"=w1099:errorcluster)  [unwired: 1 out]
      }
      event "Phase adj. (GI)", "+ phase (GI)", "- phase (GI)": Value Change {
        n675 = event-data() -> ()  [unwired: 7 out]
        n676 = Negate(x="Phase adj. (GI)") -> (-x=w1114:i16)
        n677 = Select(t=w1114, s="+ phase (GI)", f="Phase adj. (GI)") -> (s? t:f=w1113:i16)
        n678 = Or(x="+ phase (GI)", y="- phase (GI)") -> (x .or. y?=w1109:bool)
        n679 = xnode "Read/Write Control"("FPGA VI Reference In"=w1116, "error in"=w1115, "Phase count adjustment (GI)"=w1113) -> ("FPGA VI Reference Out"=w1111:T19, "error out"=w1112:errorcluster)
        n680 = xnode "Read/Write Control"("FPGA VI Reference In"=w1111, "error in"=w1112, "+ phase (GI)"=w1109) -> ("error out"=w1110:errorcluster)  [unwired: 1 out]
      }
      event "Phase adj. (GI) 2", "+ phase (GI) 2", "- phase (GI) 2": Value Change {
        n681 = event-data() -> ()  [unwired: 7 out]
        n682 = Negate(x="Phase adj. (GI) 2") -> (-x=w1125:i16)
        n683 = Select(t=w1125, s="+ phase (GI) 2", f="Phase adj. (GI) 2") -> (s? t:f=w1124:i16)
        n684 = Or(x="+ phase (GI) 2", y="- phase (GI) 2") -> (x .or. y?=w1120:bool)
        n685 = xnode "Read/Write Control"("FPGA VI Reference In"=w1127, "error in"=w1126, "Phase count adjustment (GI) 2"=w1124) -> ("FPGA VI Reference Out"=w1122:T19, "error out"=w1123:errorcluster)
        n686 = xnode "Read/Write Control"("FPGA VI Reference In"=w1122, "error in"=w1123, "+ phase (GI) 2"=w1120) -> ("error out"=w1121:errorcluster)  [unwired: 1 out]
      }
      event "Phase adj. (Green FB)", "- phase (Green FB)", "+ phase (Green FB)": Value Change {
        n687 = event-data() -> ()  [unwired: 7 out]
        n688 = Negate(x="Phase adj. (Green FB)") -> (-x=w1136:i16)
        n689 = Select(t=w1136, s="+ phase (Green FB)", f="Phase adj. (Green FB)") -> (s? t:f=w1135:i16)
        n690 = Or(x="+ phase (Green FB)", y="- phase (Green FB)") -> (x .or. y?=w1131:bool)
        n691 = xnode "Read/Write Control"("FPGA VI Reference In"=w1138, "error in"=w1137, "Phase count adjustment (Green FB)"=w1135) -> ("FPGA VI Reference Out"=w1133:T19, "error out"=w1134:errorcluster)
        n692 = xnode "Read/Write Control"("FPGA VI Reference In"=w1133, "error in"=w1134, "+ phase (Green FB)"=w1131) -> ("error out"=w1132:errorcluster)  [unwired: 1 out]
      }
      event "Invert APD Gate", "APD Gate ON Count", "APD Gate OFF Count", "APD Gate", "APD Integration Time (s)", "APD 1 AO Mult.", "APD 2 AO Mult.": Value Change {
        n693 = event-data() -> ()  [unwired: 7 out]
        n694 = local read "APD Integration Time (s)"() -> (w1139:dbl)
        n695 = local read "APD Gate ON Count"() -> (w1152:u32)
        n696 = local read "APD Gate OFF Count"() -> (w1151:u32)
        n697 = local read "Invert APD Gate"() -> (w1153:bool)
        n698 = local read "APD Gate"() -> (w1150:enum32{"ON", "OFF", "Interlace"})
        n699 = Multiply(x=w1139, y=40000000.0) -> (x*y=w1148:dbl)
        n700 = Reciprocal(x=w1139) -> (1/x=→"APD Acq Rate (Hz)":dbl)
        n701 = To Unsigned Long Integer(number=w1148) -> (unsigned 32bit integer=w1147:u32)
        n702 = local read "DMA Update Period (s)"() -> (w1140:dbl)
        n703 = Divide(x=w1140, y=w1139) -> (x/y=w1143:dbl)
        n704 = local read "APD 1 AO Mult."() -> (w1145:i16)
        n705 = local read "APD 2 AO Mult."() -> (w1144:i16)
        n706 = Multiply(x=2.0, y=w1143) -> (x*y=w1142:dbl)
        n707 = local write "APD Samples/FIFO Acq."(w1143) -> ()
        n708 = local write "APD Elements/DMA read"(w1142) -> ()
        n709 = xnode "Read/Write Control"("FPGA VI Reference In"=w1156, "error in"=w1155, "Invert APD Gate"=w1153, "APD Gate ON Count"=w1152, "APD Gate OFF Count"=w1151, "APD Acq Rate Count"=w1147, "APD Gate Operating Mode"=w1150, "APD 1 AO scale factor"=w1145, "APD 2 AO scale factor"=w1144) -> ("error out"=w1154:errorcluster)  [unwired: 1 out]
      }
      event "GI Frequency, ON count", "Green FB Count", "GI Frequency, OFF count": Value Change {
        n710 = event-data() -> ()  [unwired: 7 out]
        n711 = xnode "Read/Write Control"("FPGA VI Reference In"=w1162, "error in"=w1160, "Green interlace ON count"="GI Frequency, ON count", "Green interlace OFF count"="GI Frequency, OFF count", "Green interlace ON count 2"="GI Frequency, ON count", "Green interlace OFF count 2"="GI Frequency, OFF count", "Green FB Count"="Green FB Count") -> ("error out"=w1161:errorcluster)  [unwired: 1 out]
      }
      event "Number of F/B Scans (AOD)", "Scan Speed (nm/s)", "Scan BD", "Initial delta (MHz)", "Step Size (nm)", "Scan Range (nm)": Value Change {
        w1224 = 123.0  # AOM cal (nm/MHz)
        n712 = event-data() -> ()  [unwired: 7 out]
        n713 = local read "BD 1 Frequency 1 (MHz)"() -> (w1207:dbl)
        n714 = local read "AOM X Cal (nm/MHz)"() -> (w1199:dbl)
        n715 = local read "X RF Frequency Limits (MHz)"() -> (w1211:T16)
        n716 = local read "Y RF Frequency Limits (MHz)"() -> (w1208:T16)
        n717 = local read "BD 2 Frequency 1 (MHz)"() -> (w1213:dbl)
        n718 = Negate(x="Scan Range (nm)") -> (-x=w1177:dbl)
        n719 = Divide(x=w1177, y=w1199) -> (x/y=w1181:dbl)
        n720 = Select(t=w1211, s="Scan BD", f=w1208) -> (s? t:f=w1210:T16)
        n721 = Select(t=w1207, s="Scan BD", f=w1213) -> (s? t:f=w1212:dbl)
        n722 = Unbundle By Name(w1210) -> ("Maximum"=w1219:dbl, "Minimum"=w1218:dbl)
        n723 = Add(x=w1181, y=w1212) -> (x+y=w1216:dbl)
        n724 = Divide(x=w1177, y="Step Size (nm)") -> (x/y=w1196:dbl)
        n725 = Divide(x="Step Size (nm)", y=w1199) -> (x/y=w1205:dbl)
        n726 = Absolute Value(x=w1196) -> (abs(x)=w1180:dbl)
        n727 = Sign(1:w1177) -> (0:w1178:dbl)
        n728 = In Range and Coerce(upper limit=w1219, x=w1216, lower limit=w1218) -> (coerced(x)=w1215:dbl, In Range?=w1217:bool)
        n729 = To Unsigned Quad Integer(1:w1180) -> (0:w1195:u64)
        "Scan steps (AOD)" <- w1195
        n730 = call "IR AOM freq to word.vi"("Frequency In (MHz)"=w1205) -> ("Frequency Word Out (double)"=w1202:dbl)
        n731 = Multiply(x=w1178, y=w1202) -> (x*y=w1179:dbl)
        n732 = Subtract(x=w1216, y=w1215) -> (x-y=w1214:dbl)
        n733 = To Quad Integer(1:w1179) -> (0:w1201:i64)
        "Incr. int (AOD)" <- w1201
        n734 = Subtract(x=w1181, y=w1214) -> (x-y=w1200:dbl)
        "Scan Range (MHz)" <- w1200
        n735 = Select(t=w1181, s=w1217, f=w1200) -> (s? t:f=w1220:dbl)
        n736 = Multiply(x=w1200, y=w1199) -> (x*y=w1198:dbl)
        n737 = Decrement(x=w1195) -> (x-1=w1248:u64)
        n738 = Negate(x=w1198) -> (-x=w1194:dbl)
        n739 = local write "Scan Range (nm)"(w1194) -> ()
        n740 = Divide(x=w1220, y=w1248) -> (x/y=w1204:dbl)
        "Scan Increment (MHz)" <- w1204
        n741 = call "IR AOM freq to word.vi"("Frequency In (MHz)"=w1204) -> ("Frequency Word Out (double)"=w1203:dbl)
        n742 = Divide(x="Step Size (nm)", y="Scan Speed (nm/s)") -> (x/y=w1191:dbl)
        n743 = To Quad Integer(1:w1203) -> ()  [unwired: 1 out]
        n744 = local read "Number Interlace Sets"() -> (w1175:u8)
        n745 = local read "AI Count (ticks)"() -> (w1176:u32)
        n746 = local read "Total Counts (ticks)"() -> (w1174:u32)
        n747 = local read "# Samples/trap"() -> (w1206:u32)
        n748 = Multiply(x=w1176, y=w1175) -> (x*y=w1173:u32)
        n749 = Divide(x=w1174, y=w1173) -> (x/y=w1172:dbl)
        n750 = Select(t=w1207, s="Scan BD", f=w1213) -> (s? t:f=w1245:dbl)
        "Initial freq. (MHz)" <- w1245
        n751 = Add(x=w1220, y=w1245) -> (x+y=→"Final freq. (MHz)":dbl)
        n752 = Divide(x=w1174, y=40000000.0) -> (x/y=w1190:dbl)
        n753 = Divide(x=w1191, y=w1190) -> (x/y=w1189:dbl)
        n754 = To Unsigned Quad Integer(1:w1189) -> (0:w1164:u64)
        n755 = Quotient & Remainder(x=w1164, y=u64 2) -> (x-y*floor(x/y)=w1168:u64)  [unwired: 1 out]
        n756 = Equal?(x=w1168, y=u64 0) -> (x = y?=w1166:bool)
        n757 = Decrement(x=w1164) -> (x-1=w1165:u64)
        n758 = Select(t=w1164, s=w1166, f=w1165) -> (s? t:f=w1163:u64)
        "Cycles/step (AOD)" <- w1163
        n759 = xnode "Read/Write Control"("FPGA VI Reference In"=w1256, "error in"=w1255, "Scan steps"=w1195, "Number of scans"="Number of F/B Scans (AOD)", "Cycles per step"=w1163, "Scan freq.  increment"=w1201, "Scan BD"="Scan BD") -> ("error out"=w1254:errorcluster)  [unwired: 1 out]
        n760 = Multiply(x=w1195, y=w1163) -> (x*y=w1249:u64)
        n761 = Multiply(x=w1249, y=u64 2) -> (x*y=w1171:u64)
        n762 = Multiply(x=w1172, y=w1171) -> (x*y=w1170:dbl)
        "Data points/scan (f/b)" <- w1170
        n763 = Multiply(x=w1170, y="Number of F/B Scans (AOD)") -> (x*y=w1252:dbl)
        "Data points/scans" <- w1252
        n764 = Divide(x=w1252, y=w1206) -> (x/y=→"N sets should be saved":dbl)
        n765 = Multiply(x=w1249, y=w1190) -> (x*y=w1188:dbl)
        "Time/Scan (s) (AOD)" <- w1188
        n766 = Select(t=w1220, s="Scan BD", f=0.0) -> (s? t:f=w1246:dbl)
        n767 = Select(t=0.0, s="Scan BD", f=w1220) -> (s? t:f=w1242:dbl)
        n768 = local read "BD 2 Frequency 2 (MHz)"() -> (w1238:dbl)
        n769 = local read "BD 1 Frequency 2 (MHz)"() -> (w1241:dbl)
        n770 = Add(x=w1242, y=w1213) -> (x+y=w1239:dbl)
        n771 = Add(x=w1207, y=w1246) -> (x+y=w1240:dbl)
        n772 = Multiply(x=w1188, y=2.0) -> (x*y=w1187:dbl)
        n773 = Multiply(x=w1187, y="Number of F/B Scans (AOD)") -> (x*y=w1184:dbl)
        n774 = Divide(x=w1184, y=60.0) -> (x/y=→"Time to Finish All (min)":dbl)
        n775 = Add(x="Trap 2 Bead Size (nm)", y="Trap 1 Bead Size (nm)") -> (x+y=w1228:dbl)
        n776 = local read "Initial delta (MHz)"() -> (w1225:dbl)
        n777 = Divide(x=w1228, y=2.0) -> (x/y=w1222:dbl)
        n778 = Subtract(x=w1239, y=w1238) -> (x-y=w1236:dbl)
        n779 = Subtract(x=w1240, y=w1241) -> (x-y=w1237:dbl)
        n780 = Square(x=w1236) -> (x^2=w1235:dbl)
        n781 = Square(x=w1237) -> (x^2=w1234:dbl)
        n782 = Add(x=w1234, y=w1235) -> (x+y=w1233:dbl)
        n783 = Square Root(x=w1233) -> (sqrt(x)=w1232:dbl)
        "Final delta (MHz)" <- w1232
        n784 = Multiply(x=w1224, y=w1232) -> (x*y=w1231:dbl)
        n785 = Multiply(x=w1225, y=w1224) -> (x*y=w1223:dbl)
        n786 = Subtract(x=w1223, y=w1222) -> (x-y=→"Initial sep (nm)":dbl)
        n787 = Subtract(x=w1231, y=w1222) -> (x-y=→"Final sep (nm)":dbl)
      }
      event "Raster Scanning...": Value Change {
        n788 = event-data() -> ("NewVal"=w1257:bool)  [unwired: 6 out]
        n789 = case shown="True" w1257 {
          frame False {
          }
          frame True {
            n790 = property on="BD 1 Frequency 1 (MHz)" class="DigNum (strict)"("Val(Sgnl)"=65.0 ("Value (Signaling)")) -> ()  [unwired: 2 in, 2 out]
          }
        }
      }
      event "Freq or Amp switch first", "Swap F1 and F2", "Freq switch delay", "Amp switch delay": Value Change {
        n791 = event-data() -> ()  [unwired: 7 out]
        n792 = local read "Freq or Amp switch first"() -> (w1259:bool)
        n793 = local read "Amp switch delay"() -> (w1260:u16)
        n794 = local read "Freq switch delay"() -> (w1262:u16)
        n795 = local read "Swap F1 and F2"() -> (w1261:bool)
        n796 = xnode "Read/Write Control"("FPGA VI Reference In"=w1265, "error in"=w1264, "Freq switch delay"=w1262, "Swap F1 and F2"=w1261, "Amp switch delay"=w1260, "Freq or Amp switch first"=w1259) -> ("error out"=w1263:errorcluster)  [unwired: 1 out]
      }
      event "Scan steps (MCL)", "Number of scans (MCL)", "Scan Range (V)\n(of steps)", "2D or 1D Scan", "N APD Samp/step", "Fast Scan Dir", "Continuous MCL Scanning", "Scan lines (y)": Value Change {
        w1267 = 32767.0 ("y")
        n797 = event-data() -> ()  [unwired: 7 out]
        n798 = Select(t="Scan lines (y)", s="2D or 1D Scan", f="Number of scans (MCL)") -> (s? t:f=w1272:u64)
        n799 = Decrement(x="Scan steps (MCL)") -> (x-1=w1288:u64)
        n800 = Divide(x="Scan Range (V)\n(of steps)", y=w1288) -> (x/y=w1287:dbl)
        "Desired Scan Incr (V)" <- w1287
        n801 = local read "APD Integration Time (s)"() -> (w1280:dbl)
        n802 = Multiply(x=w1287, y=w1267) -> (x*y=w1296:dbl)
        n803 = Divide(x=w1296, y=10.0) -> (x/y=w1286:dbl)
        "Desired incr (int)" <- w1286
        n804 = local read "Update Count (MCL)"() -> (w1292:u32)
        n805 = Round Toward -Infinity(1:w1286) -> (0:w1295:dbl)
        n806 = To Word Integer(number=w1295) -> (16bit integer=w1270:i16)
        "Actual Incr. int (MCL)" <- w1270
        n807 = Multiply(x=w1280, y=40000000.0) -> (x*y=w1293:dbl)
        n808 = Divide(x=w1293, y=w1292) -> (x/y=w1291:dbl)
        n809 = Multiply(x=i16 10, y=w1270) -> (x*y=w1268:i16)
        n810 = Multiply(x="N APD Samp/step", y=w1291) -> (x*y=w1290:dbl)
        "Cycles/step (MCL)" <- w1290
        n811 = Divide(x=w1268, y=w1267) -> (x/y=→"Actual MCL Inc (V)":dbl)
        n812 = Multiply(x="N APD Samp/step", y="Scan steps (MCL)") -> (x*y=w1282:dbl)
        n813 = local read "APD Samples/FIFO Acq."() -> (w1279:dbl)
        n814 = Multiply(x=w1282, y=u64 2) -> (x*y=w1281:dbl)
        "Data points/scan (f+b)" <- w1281
        n815 = Multiply(x=w1281, y=w1272) -> (x*y=w1299:dbl)
        "Data points/scans (MCL)" <- w1299
        n816 = Multiply(x=w1280, y=w1281) -> (x*y=w1273:dbl)
        "Time/f+b scan (s) (MCL)" <- w1273
        n817 = Divide(x=w1299, y=w1279) -> (x/y=→"N sets should be saved (MCL)":dbl)
        n818 = Multiply(x=w1273, y=w1272) -> (x*y=→"Total Time (s)":dbl)
        n819 = Not(x="Fast Scan Dir") -> (.not. x?=w1277:bool)
        n820 = xnode "Read/Write Control"("FPGA VI Reference In"=w1303, "error in"=w1302, "Scan steps (MCL)"="Scan steps (MCL)", "Number of scans (MCL)"=w1272, "Cycles per step (MCL)"=w1290, "Scan freq.  increment (MCL)"=w1270, "1D or 2D Scan?"="2D or 1D Scan", "MCL Scan Axis"=w1277, "Cont. Scan (MCL)"="Continuous MCL Scanning") -> ("error out"=w1301:errorcluster)  [unwired: 1 out]
      }
      event "Read Cal": Value Change {
        w1305 = 1000.0 ("y")
        n821 = event-data() -> ()  [unwired: 7 out]
        n822 = local read "Save file name"() -> (w1330:path)
        n823 = local write "Read Cal"(FALSE ("Read Cal")) -> ()
        n824 = Strip Path(path=w1330) -> (stripped path=w1329:path)  [unwired: 1 out]
        n825 = Path To String(path=w1329) -> (string=w1328:string)
        n826 = Concatenate Strings(w1328, "\\current.cal" ("string")) -> (w1326:string)
        n827 = String To Path(string=w1326) -> (path=w1325:path)
        n828 = Open/Create/Replace File(file path (use dialog)=w1325, operation (0:open)=T23."open", access (0:read/write)=enum16{"read/write", "read-only", "write-only"}."read-only") -> (refnum out=w1333:refnum<file>, error out=w1319:errorcluster)  [unwired: 1 in, 3 out]
        n829 = Deny Access(4:w1319, 7:w1333) -> (0:w1318:errorcluster, 3:w1324:refnum<file>)  [unwired: 1 out]
        n830 = Read from Binary File(5:0.0, 8:w1318, 9:T29."big-endian, network order" ("byte order (0:big-endian, network order)"), 10:-1 ("count (1)"), 11:w1324) -> (0:w1317:errorcluster, 2:w1315:dbl[], 3:w1320:refnum<file>)  [unwired: 2 out]
        n831 = Array To Cluster(array=w1315) -> (cluster=w1314:T31)
        n832 = Unbundle(w1314) -> ("[0]"=w1313:dbl, "[1]"=w1312:dbl, "[2]"=w1311:dbl, "[3]"=w1310:dbl, "[4]"=w1309:dbl, "[5]"=w1308:dbl)
        n833 = Close File(refnum=w1320, error in=w1317) -> (error out=→"Read cal error":errorcluster)  [unwired: 1 out]
        n834 = Multiply(x=w1308, y=w1305) -> (x*y=w1306:dbl)
        n835 = local write "T2 kappa_x (pN/nm)"(w1310) -> ()
        n836 = local write "T1 kappa_x (pN/nm)"(w1311) -> ()
        n837 = local write "T1 alpha_x (nm/V)"(w1313) -> ()
        n838 = local write "T2 alpha_x (nm/V)"(w1312) -> ()
        n839 = Multiply(x=w1309, y=w1305) -> (x*y=w1307:dbl)
        n840 = local write "T1 offset_x (mV)"(w1307) -> ()
        n841 = local write "T2 offset_x (mV)"(w1306) -> ()
      }
      event "Abort MCL Scan": Value Change {
        n842 = event-data() -> ()  [unwired: 7 out]
        n843 = local write "MCL Scanning"(FALSE ("MCL Scanning")) -> ()
        n844 = xnode "Read/Write Control"("FPGA VI Reference In"=w1338, "error in"=w1337, "Abort scan (MCL)"="Abort MCL Scan") -> ("error out"=w1336:errorcluster)  [unwired: 1 out]
      }
      event "Update Count (MCL)": Value Change {
        n845 = event-data() -> ()  [unwired: 7 out]
        n846 = xnode "Read/Write Control"("FPGA VI Reference In"=w1342, "error in"=w1341, "MCL count"="Update Count (MCL)") -> ("error out"=w1340:errorcluster)  [unwired: 1 out]
      }
      event "Phase adjust (MCL)", "+ phase (MCL)", "- phase (MCL)": Value Change {
        n847 = event-data() -> ()  [unwired: 7 out]
        n848 = Negate(x="Phase adjust (MCL)") -> (-x=w1351:i16)
        n849 = Select(t=w1351, s="- phase (MCL)", f="Phase adjust (MCL)") -> (s? t:f=w1349:i16)
        n850 = Or(x="- phase (MCL)", y="+ phase (MCL)") -> (x .or. y?=w1344:bool)
        n851 = xnode "Read/Write Control"("FPGA VI Reference In"=w1353, "error in"=w1352, "Phase count adjustment (MCL)"=w1349) -> ("FPGA VI Reference Out"=w1345:T19, "error out"=w1346:errorcluster)
        n852 = xnode "Read/Write Control"("FPGA VI Reference In"=w1345, "error in"=w1346, "+ phase (MCL)"=w1344) -> ("error out"=w1343:errorcluster)  [unwired: 1 out]
      }
      event "Abort AOD Scan": Value Change {
        n853 = event-data() -> ()  [unwired: 7 out]
        n854 = xnode "Read/Write Control"("FPGA VI Reference In"=w1357, "error in"=w1356, "Abort scan"="Abort AOD Scan") -> ("error out"=w1355:errorcluster)  [unwired: 1 out]
      }
      event "Continuous AOD Scanning": Value Change {
        n855 = event-data() -> ()  [unwired: 7 out]
        n856 = xnode "Read/Write Control"("FPGA VI Reference In"=w1361, "error in"=w1360, "Cont. Scan"="Continuous AOD Scanning") -> ("error out"=w1359:errorcluster)  [unwired: 1 out]
      }
      event "Index": Value Change {
        n857 = event-data() -> ()  [unwired: 7 out]
        n858 = call "Create new save file.vi"("Insert"="", "Ext"=".dat" ("string"), "Index In"="Index") -> ("Path Out"=→"Save file name":path, "Index Out"=w1362:dbl)
        "Save index" <- w1362
        n859 = local write "Index"(w1362) -> ()
      }
      event "AO1", "AO2": Value Change {
        w1377 = 10.0 ("y")
        w1376 = 32767.0 ("y")
        n860 = event-data() -> ()  [unwired: 7 out]
        n861 = local read "AO2"() -> (w1375:dbl)
        n862 = local read "AO1"() -> (w1372:dbl)
        n863 = Multiply(x=w1372, y=w1376) -> (x*y=w1371:dbl)
        n864 = Multiply(x=w1375, y=w1376) -> (x*y=w1374:dbl)
        n865 = Divide(x=w1371, y=w1377) -> (x/y=w1370:dbl)
        n866 = Divide(x=w1374, y=w1377) -> (x/y=w1373:dbl)
        n867 = To Word Integer(number=w1370) -> (16bit integer=w1378:i16)
        n868 = To Word Integer(number=w1373) -> (16bit integer=w1379:i16)
        n869 = xnode "Read/Write Control"("FPGA VI Reference In"=w1369, "error in"=w1368, "AO1"=w1378, "AO2"=w1379) -> ("error out"=w1367:errorcluster)  [unwired: 1 out]
      }
      event "Inject Top:": Value Change {
        n870 = event-data() -> ()  [unwired: 7 out]
        n871 = disable-structure shown="Enabled" {
          disable-tunnel: "Inject Top:" -> [w1381 w1421]
          frame Disabled {
            n872 = local read "Chemyx Syringe Pump Serial Port"() -> (w1382:refnum<visa-resource-name>)
            n873 = local read "Pump write delay (ms)"() -> (w1383:dbl)
            n874 = case shown="True" w1381 {
              tunnel: w1383 -> [w1389 w1403]
              tunnel: w1382 -> [w1386 w1402]
              frame False {
                n875 = flat-sequence {
                  tunnel: w1386 -> [w1390]
                  tunnel: [w1390] -> w1387
                  tunnel: w1389 -> [_]
                  tunnel: [w1393] -> w1388
                  tunnel: w1387 -> [w1393]
                  tunnel: w1388 -> [w1394]
                  tunnel: [w1394] -> w1384
                  tunnel: [w1396] -> w1385
                  tunnel: w1384 -> [w1396]
                  tunnel: w1385 -> [w1398]
                  frame #0 {
                    n876 = call "Write to pump.vi"("string"="enter pump1", "VISA resource name"=w1390) -> ()  [unwired: 1 out]
                  }
                  frame #1 {
                    n877 = Wait (ms)(milliseconds to wait="Pump pause delay (ms)") -> ()  [unwired: 1 out]
                  }
                  frame #2 {
                    n878 = call "Write to pump.vi"("string"="stop", "VISA resource name"=w1394) -> ()  [unwired: 1 out]
                  }
                  frame #3 {
                    n879 = Wait (ms)(milliseconds to wait=u32 500) -> ()  [unwired: 1 out]
                  }
                  frame #4 {
                    n880 = call "Write to pump.vi"("string"="stop", "VISA resource name"=w1398) -> ()  [unwired: 1 out]
                  }
                }
              }
              frame True {
                n881 = flat-sequence {
                  tunnel: w1402 -> [w1412]
                  tunnel: w1403 -> [w1407]
                  tunnel: w1403 -> [w1414]
                  tunnel: w1402 -> [w1415]
                  tunnel: [w1415] -> w1400
                  tunnel: [w1417] -> w1401
                  tunnel: w1400 -> [w1417]
                  tunnel: w1401 -> [w1419]
                  frame #0 {
                    n882 = local read "All Pump Parameters"() -> (w1406:T6)
                    n883 = Unbundle By Name(w1406) -> ("Pump 1"=w1413:T32)
                    n884 = call "Set pump parameters.vi"("Pump write delay (ms)"=w1407, "Volume (uL)"="Ch 2 Inject Volume (uL)", "Rate (uL/h)"="Ch 1 Inject Rate (ul/h)", "Units"=4.0, "Pump #"=1.0, "Pump Parameters In"=w1413, "VISA resource name"=w1412) -> ("Pump Parameters Out"=w1405:T32)  [unwired: 3 in]
                    n885 = Bundle By Name(cluster=w1406, "Pump 1"=w1405) -> (w1404:T6)
                    n886 = local write "All Pump Parameters"(w1404) -> ()
                  }
                  frame #1 {
                    n887 = Wait (ms)(milliseconds to wait=w1414) -> ()  [unwired: 1 out]
                  }
                  frame #2 {
                    n888 = call "Write to pump.vi"("string"="start", "VISA resource name"=w1415) -> ()  [unwired: 1 out]
                  }
                  frame #3 {
                    n889 = Wait (ms)(milliseconds to wait=u32 500) -> ()  [unwired: 1 out]
                  }
                  frame #4 {
                    n890 = call "Write to pump.vi"("string"="start", "VISA resource name"=w1419) -> ()  [unwired: 1 out]
                  }
                }
              }
            }
          }
          frame Enabled {
            n891 = call "hamilton_controller.vi"("Open?"=w1421, "valve"=enum16{"A", "B", "C", "D", "ALL"}."B", "action"=T20."MOVE VALVE") -> ()  [unwired: 8 in, 1 out]
          }
        }
      }
      event "Main:": Value Change {
        n892 = event-data() -> ()  [unwired: 7 out]
        n893 = disable-structure shown="Disabled" {
          disable-tunnel: "Main:" -> [_ w1465]
          frame Disabled {
            n894 = local read "Pump write delay (ms)"() -> (w1426:dbl)
            n895 = case shown="False" w1427 {
              tunnel: w1426 -> [w1433 w1447]
              tunnel: "Chemyx Syringe Pump Serial Port" -> [w1430 w1446]
              frame False {
                n896 = flat-sequence {
                  tunnel: w1430 -> [w1434]
                  tunnel: [w1434] -> w1431
                  tunnel: w1433 -> [_]
                  tunnel: [w1437] -> w1432
                  tunnel: w1431 -> [w1437]
                  tunnel: w1432 -> [w1438]
                  tunnel: [w1438] -> w1428
                  tunnel: [w1440] -> w1429
                  tunnel: w1428 -> [w1440]
                  tunnel: w1429 -> [w1442]
                  frame #0 {
                    n897 = call "Write to pump.vi"("string"="enter pump3", "VISA resource name"=w1434) -> ()  [unwired: 1 out]
                  }
                  frame #1 {
                    n898 = local read "Pump pause delay (ms)"() -> (w1436:u32)
                    n899 = Wait (ms)(milliseconds to wait=w1436) -> ()  [unwired: 1 out]
                  }
                  frame #2 {
                    n900 = call "Write to pump.vi"("string"="stop", "VISA resource name"=w1438) -> ()  [unwired: 1 out]
                  }
                  frame #3 {
                    n901 = Wait (ms)(milliseconds to wait=u32 0) -> ()  [unwired: 1 out]
                  }
                  frame #4 {
                    n902 = call "Write to pump.vi"("string"="stop", "VISA resource name"=w1442) -> ()  [unwired: 1 out]
                  }
                }
              }
              frame True {
                n903 = flat-sequence {
                  tunnel: w1446 -> [w1456]
                  tunnel: w1447 -> [w1451]
                  tunnel: w1447 -> [w1458]
                  tunnel: w1446 -> [w1459]
                  tunnel: [w1459] -> w1444
                  tunnel: [w1462] -> w1445
                  tunnel: w1444 -> [w1462]
                  tunnel: w1445 -> [w1463]
                  frame #0 {
                    n904 = local read "All Pump Parameters"() -> (w1450:T6)
                    n905 = Unbundle By Name(w1450) -> ("Pump 3"=w1457:T32)
                    n906 = call "Set pump parameters.vi"("Pump write delay (ms)"=w1451, "Volume (uL)"="Ch 3 Inject Volume (uL)", "Rate (uL/h)"="Ch 3 Inject Rate (ul/h)", "Units"=4.0, "Pump #"=3.0, "Pump Parameters In"=w1457, "VISA resource name"=w1456) -> ("Pump Parameters Out"=w1449:T32)  [unwired: 3 in]
                    n907 = Bundle By Name(cluster=w1450, "Pump 3"=w1449) -> (w1448:T6)
                    n908 = local write "All Pump Parameters"(w1448) -> ()
                  }
                  frame #1 {
                    n909 = Wait (ms)(milliseconds to wait=w1458) -> ()  [unwired: 1 out]
                  }
                  frame #2 {
                    n910 = call "Write to pump.vi"("string"="start", "VISA resource name"=w1459) -> ()  [unwired: 1 out]
                  }
                  frame #3 {
                    n911 = Wait (ms)(milliseconds to wait=u32 500) -> ()  [unwired: 1 out]
                  }
                  frame #4 {
                    n912 = call "Write to pump.vi"("string"="start", "VISA resource name"=w1463) -> ()  [unwired: 1 out]
                  }
                }
              }
            }
          }
          frame Enabled {
            n913 = call "hamilton_controller.vi"("Open?"=w1465, "valve"=enum16{"A", "B", "C", "D", "ALL"}."A", "action"=T20."MOVE VALVE") -> ()  [unwired: 8 in, 1 out]
          }
        }
      }
      event "Inject Valve B": Value Change {
        n914 = event-data() -> ()  [unwired: 7 out]
        n915 = disable-structure shown="Enabled" {
          disable-tunnel: "Inject Valve B" -> [w1469 w1489]
          frame Disabled {
            n916 = local read "Pump write delay (ms)"() -> (w1471:dbl)
            n917 = flat-sequence {
              tunnel: w1470 -> [w1484]
              tunnel: w1471 -> [w1480]
              tunnel: w1469 -> [_]
              tunnel: w1471 -> [w1486]
              tunnel: w1470 -> [w1487]
              frame #0 {
                n918 = local read "All Pump Parameters"() -> (w1479:T6)
                n919 = Multiply(x=60.0, y="Flush Center Ch Rate (ul/m)") -> (x*y=w1476:dbl)
                n920 = Unbundle By Name(w1479) -> ("Pump 2"=w1485:T32)
                n921 = call "Set pump parameters.vi"("Pump write delay (ms)"=w1480, "Volume (uL)"="Flush Center Ch Volume (uL)", "Rate (uL/h)"=w1476, "Units"=3.0, "Pump #"=2.0, "Pump Parameters In"=w1485, "VISA resource name"=w1484) -> ("Pump Parameters Out"=w1478:T32)  [unwired: 3 in]
                n922 = Bundle By Name(cluster=w1479, "Pump 2"=w1478) -> (w1477:T6)
                n923 = local write "All Pump Parameters"(w1477) -> ()
                n924 = Add(x="Flush Center Ch Volume (uL)", y="Total Volume\nFlushed (uL)") -> (x+y=w1473:dbl)
                n925 = local write "Total Volume\nFlushed (uL)"(w1473) -> ()
              }
              frame #1 {
                n926 = Wait (ms)(milliseconds to wait=w1486) -> ()  [unwired: 1 out]
              }
              frame #2 {
                n927 = call "Write to pump.vi"("string"="start", "VISA resource name"=w1487) -> ()  [unwired: 1 out]
              }
            }
            n928 = local read "Chemyx Syringe Pump Serial Port"() -> (w1470:refnum<visa-resource-name>)
          }
          frame Enabled {
            n929 = call "hamilton_controller.vi"("Open?"=w1489, "valve"=enum16{"A", "B", "C", "D", "ALL"}."B", "action"=T20."MOVE VALVE") -> ()  [unwired: 8 in, 1 out]
          }
        }
      }
      event "Inject Bottom": Value Change {
        n930 = event-data() -> ()  [unwired: 7 out]
        n931 = call "hamilton_controller.vi"("Open?"="Inject Bottom", "valve"=enum16{"A", "B", "C", "D", "ALL"}."C", "action"=T20."MOVE VALVE") -> ()  [unwired: 8 in, 1 out]
      }
      event "Shunt:": Value Change {
        n932 = event-data() -> ()  [unwired: 7 out]
        n933 = call "hamilton_controller.vi"("Open?"="Shunt:", "valve"=enum16{"A", "B", "C", "D", "ALL"}."D", "action"=T20."MOVE VALVE") -> ()  [unwired: 8 in, 1 out]
      }
      event "Flip Green Filter": Value Change {
        n934 = event-data() -> ()  [unwired: 7 out]
        n935 = local write "Flip Green Filter"("Flip Green Filter") -> ()
        n936 = flat-sequence {
          tunnel: w1505 -> [w1510]
          tunnel: w1504 -> [w1509]
          tunnel: [w1507] -> w1502
          tunnel: [w1506] -> w1501
          tunnel: [w1512] -> w1500
          tunnel: w1502 -> [w1512]
          tunnel: [w1511] -> w1499
          tunnel: w1501 -> [w1511]
          tunnel: w1500 -> [w1516]
          tunnel: w1499 -> [w1515]
          tunnel: [w1514] -> w1503
          frame #0 {
            n937 = xnode "Read/Write Control"("FPGA VI Reference In"=w1510, "error in"=w1509, "Green Filter Flipper"=TRUE) -> ("FPGA VI Reference Out"=w1507:T19, "error out"=w1506:errorcluster)
          }
          frame #1 {
            n938 = Wait (ms)(milliseconds to wait=u32 100) -> ()  [unwired: 1 out]
          }
          frame #2 {
            n939 = xnode "Read/Write Control"("FPGA VI Reference In"=w1516, "error in"=w1515, "Green Filter Flipper"=FALSE) -> ("error out"=w1514:errorcluster)  [unwired: 1 out]
          }
        }
      }
      event "Pump 1 contents", "Pump 3 contents": Value Change {
        n940 = event-data() -> ()  [unwired: 7 out]
        n941 = local read "Pump 1 contents"() -> (→"Pump 1 cont disp":string)
        n942 = local read "Pump 3 contents"() -> (→"Pump 3 cont disp":string)
      }
      event "Reset Trap Pos. FB": Value Change {
        n943 = event-data() -> ()  [unwired: 7 out]
        n944 = xnode "Read/Write Control"("FPGA VI Reference In"=w1522, "error in"=w1521, "Trap Pos. FB Reset"="Reset Trap Pos. FB") -> ()  [unwired: 2 out]
      }
      event "Trap Pos. FB ON": Value Change {
        n945 = event-data() -> ()  [unwired: 7 out]
        n946 = xnode "Read/Write Control"("FPGA VI Reference In"=w1525, "error in"=w1524, "Force feedback"="Trap Pos. FB ON") -> ()  [unwired: 2 out]
      }
      event "Trap Pos. FB Range", "Trap Pos. FB Gains", "Trap Pos. FB Mult Factor", "Trap Pos. FB Offset Factor", "Trap Pos FB Negate Action", "Trap Pos FB Monitor\nT1 or T2": Value Change {
        n947 = event-data() -> ()  [unwired: 7 out]
        n948 = xnode "Read/Write Control"("FPGA VI Reference In"=w1534, "error in"=w1533, "Trap Pos. FB Range"="Trap Pos. FB Range", "Trap Pos. FB Gains"="Trap Pos. FB Gains", "Trap Pos. FB Mult Factor"="Trap Pos. FB Mult Factor", "Trap Pos. FB Offset Factor"="Trap Pos. FB Offset Factor", "Trap Pos FB Negate Action"="Trap Pos FB Negate Action", "Trap Pos FB Monitor T1 or T2"="Trap Pos FB Monitor\nT1 or T2", "AI1 X Scale"="Trap Pos. AI1 X Pre-scale") -> ()  [unwired: 2 out]
      }
      event "Trap Pos FB SP": Value Change {
        n949 = event-data() -> ()  [unwired: 7 out]
        n950 = xnode "Read/Write Control"("FPGA VI Reference In"=w1537, "error in"=w1536, "Trap Pos. FB SP"="Trap Pos FB SP") -> ()  [unwired: 2 out]
      }
      event "Set SP to Reading": Value Change {
        n951 = event-data() -> ()  [unwired: 7 out]
        n952 = local read "Trap Pos FB Monitor\nT1 or T2"() -> (w1545:bool)
        n953 = local read "Trap X AI1 (DMA)"() -> (w1548:T13)
        n954 = local read "Trap X (AI1)"() -> (w1551:T1)
        n955 = Unbundle By Name(w1551) -> ("Trap 1"=w1550:fxp<+/-,16,1>, "Trap 2"=w1549:fxp<+/-,16,1>)
        n956 = Unbundle By Name(w1548) -> ("Set 1"=w1547:fxp<+/-,16,1>, "Set 2"=w1546:fxp<+/-,16,1>)
        n957 = Select(t=w1550, s=w1545, f=w1549) -> (s? t:f=w1544:fxp<+/-,16,1>)
        n958 = Select(t=w1547, s=w1545, f=w1546) -> (s? t:f=w1543:fxp<+/-,16,1>)
        n959 = Not(x="Set SP Using...") -> (.not. x?=w1538:bool)
        n960 = Select(t=w1544, s=w1538, f=w1543) -> (s? t:f=w1539:fxp<+/-,16,1>)
        n961 = xnode "Read/Write Control"("FPGA VI Reference In"=w1541, "error in"=w1540, "Trap Pos. FB SP"=w1539) -> ()  [unwired: 2 out]
        n962 = local write "Trap Pos FB SP"(w1539) -> ()
      }
      event "Trap Pos. FB Out Scale 2^n": Value Change {
        n963 = event-data() -> ()  [unwired: 7 out]
        n964 = Scale By Power Of 2(n="Trap Pos. FB Out Scale 2^n", x=ext 1.0) -> (x*2^n=w1553:ext)
        n965 = property on="Trap Pos. FB Mult Factor" class="DigNum (strict)"("Val(Sgnl)"=w1553) -> ()  [unwired: 2 in, 2 out]
      }
      event "Trap Pos FB Int Count": Value Change {
        n966 = event-data() -> ()  [unwired: 7 out]
        n967 = xnode "Read/Write Control"("FPGA VI Reference In"=w1558, "error in"=w1557, "Trap Pos FB Int Count"="Trap Pos FB Int Count") -> ()  [unwired: 2 out]
      }
    }
    "error out 2" <- w736
    n968 = node-c288() -> ()  [unwired: 1 in, 1 out]
  }
  n969 = timed-loop "Run Scripts, including: stage motion" {
    timing: w69 -> [_]
    timing-out: [_] -> w68
    tunnel: w24 -> [_]
    stop <- w1560 stop-if-true
    n970 = node-c288() -> ()  [unwired: 1 in, 1 out]
    n971 = event shown="[2] \"Cal/Data Acq. Spot\": Value Change" {
      selector: _ -> [_ _ _ _ _ _ _ _ _ _ _ _]
      dyn-events: _ -> [_ _ _ _ _ _ _ _ _ _ _ _]
      timeout: 50 -> [_ _ _ _ _ _ _ _ _ _ _ _]
      tunnel: ["Move Cap. 1 (DNA Top)" _ "Cal/Data Acq. Spot" "Dump Beads" "Dip for Protein" _ "Got ADig bead" "Got DNA bead" "Take Stepping Data" _ "Take Detection Laser\nImage" _] -> _
      tunnel: [_ _ _ _ _ _ _ _ _ _ _ w1768] -> w1560
      event "Move Cap. 1 (DNA Top)": Value Change {
        n972 = event-data() -> ()  [unwired: 1 in, 5 out]
        n973 = local write "Move Cap. 1 (DNA Top)"(FALSE ("Move Cap. 1 (DNA Right)")) -> ()
        n974 = flat-sequence {
          tunnel: "Cap 1 Samp Flow ON" -> [w1566]
          frame #0 {
            n975 = local write "Stage Moving"(FALSE ("Stage Moving")) -> ()
            n976 = case "stop flow" shown="True" w1566 {
              frame False {
              }
              frame True {
                n977 = call "hamilton_controller.vi"("Open?"=FALSE, "valve"=enum16{"A", "B", "C", "D", "ALL"}."C", "action"=T20."MOVE VALVE") -> ()  [unwired: 8 in, 1 out]
              }
            }
            n978 = case shown="True" TRUE {
              tunnel: "Cap 1 T ON" -> [w1575 w1576]
              frame False {
                n979 = property on="Trap 1 (ON/OFF)" class="Bool (strict)"("Val(Sgnl)"=w1575) -> ()  [unwired: 2 in, 2 out]
              }
              frame True {
                n980 = property on="Trap 2 (ON/OFF)" class="Bool (strict)"("Val(Sgnl)"=w1576) -> ()  [unwired: 2 in, 2 out]
              }
            }
            n981 = call <vilib>:"Beep.vi"() -> ()  [unwired: 3 in, 9 out]
            n982 = case shown="True" "Cap 1 Flow ON" {
              frame False {
              }
              frame True {
                n983 = property on="Main:" class="Bool (strict)"("Val(Sgnl)"=TRUE ("Value (Signaling)")) -> ()  [unwired: 2 in, 2 out]
              }
            }
          }
        }
      }
      event Timeout {
        n984 = event-data() -> ()  [unwired: 1 in, 2 out]
      }
      event "Cal/Data Acq. Spot": Value Change {
        # "wait for calibration file\nto be written"
        # "signal save cal true\nthis tells the data \nacquisition loop to\nstart sending the data\nto a calibration file"
        # "separate traps to\nthe desired trap delta"
        # "move stage to data acquisition spot"
        # "CHANGE FISH FOR TETHER BACK\nTO TRUE VALUE HERE."
        n985 = event-data() -> ()  [unwired: 1 in, 5 out]
        n986 = local write "Cal/Data Acq. Spot"(FALSE ("Cal/Data Acq. Spot")) -> ()
        n987 = flat-sequence {
          tunnel: ["Cal @ (MHz)"] -> w1577
          tunnel: w1577 -> [w1587]
          tunnel: w1577 -> [w1608]
          frame #0 {
            n988 = property on="Trap Delta (MHz)" class="DigNum (strict)"("Val(Sgnl)"="Cal @ (MHz)") -> ()  [unwired: 2 in, 2 out]
            n989 = call <vilib>:"Beep.vi"() -> ()  [unwired: 3 in, 9 out]
          }
          frame #1 {
            n990 = Wait (ms)(milliseconds to wait=u32 100) -> ()  [unwired: 1 out]
          }
          frame #2 {
            n991 = property on="Save Calibration" class="Bool (strict)"("Val(Sgnl)"=TRUE ("Value (Signaling)")) -> ()  [unwired: 2 in, 2 out]
          }
          frame #3 {
            n992 = Wait (ms)(milliseconds to wait=u32 4000) -> ()  [unwired: 1 out]
          }
          frame #4 {
            n993 = while {
              stop <- w1584 stop-if-true
              n994 = local read "Saving..."() -> (w1585:bool)
              n995 = Wait (ms)(milliseconds to wait=u32 100) -> ()  [unwired: 1 out]
              n996 = Not(x=w1585) -> (.not. x?=w1584:bool)
            }
          }
          frame #5 {
            n997 = case shown="True" "W/ Offset 1" {
              tunnel: w1587 -> [_ w1589]
              frame False {
              }
              frame True {
                n998 = stacked-sequence {
                  tunnel: w1589 -> [_ _ _ _ _ _ _ w1606]
                  frame #0 {
                    n999 = Replace Array Subset(array=u32[] [0] ("Index Values"), new element="Offset 1 Set", index=0) -> (w1590:u32[])
                    n1000 = property on="Saved AOD Raster Scan Parameter Sets" class="Arr (strict)"("Index Values"=w1590) -> ()  [unwired: 2 in, 2 out]
                    n1001 = property on="Trap Delta (MHz)" class="DigNum (strict)"("Val(Sgnl)"="Offset 1 Start (MHz)") -> ()  [unwired: 2 in, 2 out]
                  }
                  frame #1 {
                    n1002 = Wait (ms)(milliseconds to wait=u32 200) -> ()  [unwired: 1 out]
                  }
                  frame #2 {
                    n1003 = property on="Load parameters" class="Bool (strict)"("Val(Sgnl)"=TRUE ("Value (Signaling)")) -> ()  [unwired: 2 in, 2 out]
                  }
                  frame #3 {
                    n1004 = Wait (ms)(milliseconds to wait=u32 200) -> ()  [unwired: 1 out]
                  }
                  frame #4 {
                    n1005 = property on="Trap Raster Scan" class="Bool (strict)"("Val(Sgnl)"=TRUE ("Value (Signaling)")) -> ()  [unwired: 2 in, 2 out]
                  }
                  frame #5 {
                    n1006 = Wait (ms)(milliseconds to wait=u32 2000) -> ()  [unwired: 1 out]
                  }
                  frame #6 {
                    n1007 = while {
                      stop <- w1603 stop-if-true
                      n1008 = local read "Raster Scanning..."() -> (w1605:bool)
                      n1009 = local read "Saving..."() -> (w1601:bool)
                      n1010 = Wait (ms)(milliseconds to wait=u32 100) -> ()  [unwired: 1 out]
                      n1011 = Not(x=w1601) -> (.not. x?=w1600:bool)
                      n1012 = Not(x=w1605) -> (.not. x?=w1602:bool)
                      n1013 = And(x=w1602, y=w1600) -> (x .and. y?=w1603:bool)
                    }
                  }
                  frame #7 {
                    n1014 = property on="Trap Delta (MHz)" class="DigNum (strict)"("Val(Sgnl)"=w1606) -> ()  [unwired: 2 in, 2 out]
                  }
                }
              }
            }
          }
          frame #6 {
            n1015 = local read "Save ave N"() -> (w1607:dbl)
            n1016 = case shown="True" "W/ Offset 2" {
              tunnel: w1608 -> [_ w1614]
              tunnel: w1607 -> [_ w1613]
              frame False {
                n1017 = Multiply(x="Cal read wait (s)", y=u32 1000 ("milliseconds to wait")) -> (x*y=w1611:u32)
                n1018 = Wait (ms)(milliseconds to wait=w1611) -> ()  [unwired: 1 out]
              }
              frame True {
                n1019 = stacked-sequence {
                  tunnel: w1614 -> [_ _ _ _ _ _ _ _ _ w1635 _ _]
                  tunnel: w1613 -> [_ _ _ _ _ _ _ _ _ w1633 _ _]
                  frame #0 {
                    n1020 = property on="Save ave N" class="DigNum (strict)"("Val(Sgnl)"=1.0 ("Value (Signaling)")) -> ()  [unwired: 2 in, 2 out]
                  }
                  frame #1 {
                    n1021 = Wait (ms)(milliseconds to wait=u32 500) -> ()  [unwired: 1 out]
                  }
                  frame #2 {
                    n1022 = property on="Trap Delta (MHz)" class="DigNum (strict)"("Val(Sgnl)"="Offset 2 Start (MHz)") -> ()  [unwired: 2 in, 2 out]
                    n1023 = Replace Array Subset(array=u32[] [0] ("Index Values"), new element="Offset 2 Set", index=0) -> (w1619:u32[])
                    n1024 = property on="Saved AOD Raster Scan Parameter Sets" class="Arr (strict)"("Index Values"=w1619) -> ()  [unwired: 2 in, 2 out]
                  }
                  frame #3 {
                    n1025 = Wait (ms)(milliseconds to wait=u32 500) -> ()  [unwired: 1 out]
                  }
                  frame #4 {
                    n1026 = property on="Load parameters" class="Bool (strict)"("Val(Sgnl)"=TRUE ("Value (Signaling)")) -> ()  [unwired: 2 in, 2 out]
                  }
                  frame #5 {
                    n1027 = Wait (ms)(milliseconds to wait=u32 500) -> ()  [unwired: 1 out]
                  }
                  frame #6 {
                    n1028 = property on="Trap Raster Scan" class="Bool (strict)"("Val(Sgnl)"=TRUE ("Value (Signaling)")) -> ()  [unwired: 2 in, 2 out]
                  }
                  frame #7 {
                    n1029 = Wait (ms)(milliseconds to wait=u32 2000) -> ()  [unwired: 1 out]
                  }
                  frame #8 {
                    n1030 = while {
                      stop <- w1628 stop-if-true
                      n1031 = local read "Raster Scanning..."() -> (w1631:bool)
                      n1032 = local read "Saving..."() -> (w1629:bool)
                      n1033 = Wait (ms)(milliseconds to wait=u32 100) -> ()  [unwired: 1 out]
                      n1034 = Not(x=w1629) -> (.not. x?=w1627:bool)
                      n1035 = Not(x=w1631) -> (.not. x?=w1630:bool)
                      n1036 = And(x=w1630, y=w1627) -> (x .and. y?=w1628:bool)
                    }
                  }
                  frame #9 {
                    n1037 = property on="Trap Delta (MHz)" class="DigNum (strict)"("Val(Sgnl)"=w1635) -> ()  [unwired: 2 in, 2 out]
                    n1038 = property on="Saved AOD Raster Scan Parameter Sets" class="Arr (strict)"("Index Values"=u32[] [0]) -> ()  [unwired: 2 in, 2 out]
                    n1039 = property on="Save ave N" class="DigNum (strict)"("Val(Sgnl)"=w1633) -> ()  [unwired: 2 in, 2 out]
                  }
                  frame #10 {
                    n1040 = Wait (ms)(milliseconds to wait=u32 500) -> ()  [unwired: 1 out]
                  }
                  frame #11 {
                    n1041 = property on="Load parameters" class="Bool (strict)"("Val(Sgnl)"=TRUE ("Value (Signaling)")) -> ()  [unwired: 2 in, 2 out]
                  }
                }
              }
            }
          }
          frame #7 {
            n1042 = property on="Read Cal" class="Bool (strict)"("Val(Sgnl)"=TRUE ("Value (Signaling)")) -> ()  [unwired: 2 in, 2 out]
          }
          frame #8 {
            n1043 = Wait (ms)(milliseconds to wait=u32 500) -> ()  [unwired: 1 out]
          }
          frame #9 {
            n1044 = property on="Fish for Tether" class="Bool (strict)"("Val(Sgnl)"=FALSE ("Value (Signaling)")) -> ()  [unwired: 2 in, 2 out]
          }
        }
      }
      event "Dump Beads": Value Change {
        # "SCRIPT TO REMOVE BOTH BEADS FROM THE TRAPS. TURNS ON LIGHT WHICH INDICATES THAT STAGE IS MOVING. THEN STOPS SAVING DATA. \nSETS Sample Channel Flow TO TRUE. STOPS INTERLACING GREEN FLUORESCENCE. TURNS OFF Tether INDICATOR BECAUSE WE ARE THROWING IT\nAWAY. SHUTS OFF TRAP POSITION FEEDBACK."
        n1045 = event-data() -> ()  [unwired: 1 in, 5 out]
        n1046 = flat-sequence {
          frame #0 {
            w1642 = FALSE ("Fl. Triggered...")
            w1643 = TRUE ("Stage Moving")
            n1047 = local read "Saving..."() -> (w1644:bool)
            n1048 = local write "Fl. Triggered..."(w1642) -> ()
            n1049 = local write "Stage Moving"(w1643) -> ()
            n1050 = local write "Tether"(w1642) -> ()
            n1051 = property on="Green Laser ON/Interlacing" class="Bool (strict)"("Val(Sgnl)"=w1642) -> ()  [unwired: 2 in, 2 out]
            n1052 = property on="Trap Pos. FB ON" class="Bool (strict)"("Val(Sgnl)"=w1642) -> ()  [unwired: 2 in, 2 out]
            n1053 = property on="Inject Bottom" class="Bool (strict)"("Val(Sgnl)"=w1643) -> ()  [unwired: 2 in, 2 out]
            n1054 = local write "Stop Saving"(w1644) -> ()
          }
          frame #1 {
            w1645 = FALSE ("Value (Signaling)")
            # "TURNS TRAPS OFF SO THAT\nBEADS REMAIN AT DUMP \nBEADS POSITION"
            n1055 = property on="Trap 1 (ON/OFF)" class="Bool (strict)"("Val(Sgnl)"=w1645) -> ()  [unwired: 2 in, 2 out]
            n1056 = property on="Trap 2 (ON/OFF)" class="Bool (strict)"("Val(Sgnl)"=w1645) -> ()  [unwired: 2 in, 2 out]
            n1057 = call <vilib>:"Beep.vi"() -> ()  [unwired: 3 in, 9 out]
          }
          frame #2 {
            n1058 = property on="Goto Bottom (F7)" class="Bool (strict)"("Val(Sgnl)"=TRUE ("Value (Signaling)")) -> ()  [unwired: 2 in, 2 out]
          }
          frame #3 {
            n1059 = Wait (ms)(milliseconds to wait=u32 8000) -> ()  [unwired: 1 out]
          }
          frame #4 {
            n1060 = property on="Trap Delta (MHz)" class="DigNum (strict)"("Val(Sgnl)"=20.0 ("Value (Signaling)")) -> ()  [unwired: 2 in, 2 out]
          }
          frame #5 {
            n1061 = property on="Trap 2 (ON/OFF)" class="Bool (strict)"("Val(Sgnl)"=TRUE ("Value (Signaling)")) -> ()  [unwired: 2 in, 2 out]
          }
          frame #6 {
            n1062 = property on="Inject Bottom" class="Bool (strict)"("Val(Sgnl)"=FALSE ("Value (Signaling)")) -> ()  [unwired: 2 in, 2 out]
          }
        }
      }
      event "Dip for Protein": Value Change {
        n1063 = event-data() -> ()  [unwired: 1 in, 5 out]
        n1064 = flat-sequence {
          frame #0 {
            n1065 = case shown="True" "Move Trap Before?" {
              frame False {
              }
              frame True {
                n1066 = property on="Trap Delta (MHz)" class="DigNum (strict)"("Val(Sgnl)"="Dip Trap Delta 1 (MHz)") -> ()  [unwired: 2 in, 2 out]
              }
            }
          }
          frame #1 {
            n1067 = Multiply(x="Duration (s)", y=1000.0) -> (x*y=w1654:dbl)
            n1068 = Wait (ms)(milliseconds to wait=w1654) -> ()  [unwired: 1 out]
          }
          frame #2 {
            n1069 = case shown="True" "Move Trap After?" {
              frame False {
              }
              frame True {
                n1070 = property on="Trap Delta (MHz)" class="DigNum (strict)"("Val(Sgnl)"="Dip Trap Delta 2 (MHz)") -> ()  [unwired: 2 in, 2 out]
              }
            }
          }
          frame #3 {
            n1071 = case shown="True" "Green ON After?" {
              frame False {
              }
              frame True {
                n1072 = property on="Green Laser ON/Interlacing" class="Bool (strict)"("Val(Sgnl)"=TRUE ("Value (Signaling)")) -> ()  [unwired: 2 in, 2 out]
              }
            }
          }
          frame #4 {
            n1073 = Wait (ms)(milliseconds to wait=u32 500) -> ()  [unwired: 1 out]
          }
          frame #5 {
            n1074 = case shown="True" "Save Data After?" {
              frame False {
              }
              frame True {
                n1075 = property on="Start Saving" class="Bool (strict)"("Val(Sgnl)"=TRUE ("Value (Signaling)")) -> ()  [unwired: 2 in, 2 out]
              }
            }
          }
        }
      }
      event "Profile": Value Change {
        n1076 = event-data() -> ()  [unwired: 1 in, 5 out]
        n1077 = flat-sequence {
          frame #0 {
            w1664 = 0.0 ("element")
            n1078 = Build Array(w1664, "Y change (mm)", w1664) -> ()  [unwired: 1 out]
          }
          frame #1 {
            # "stop saving"
            n1079 = local write "Stop Saving"(TRUE ("Stop Saving")) -> ()
            n1080 = local write "Stage Moving"(FALSE ("Stage Moving")) -> ()
          }
        }
      }
      event "Got ADig bead": Value Change {
        n1081 = event-data() -> ()  [unwired: 1 in, 5 out]
        n1082 = property on="Move Cap. 1 (DNA Top)" class="Bool (strict)"("Val(Sgnl)"=TRUE ("Value (Signaling)")) -> ()  [unwired: 2 in, 2 out]
        n1083 = property on="Inject Top:" class="Bool (strict)"("Val(Sgnl)"=FALSE ("Value (Signaling)")) -> ()  [unwired: 2 in, 2 out]
      }
      event "Got DNA bead": Value Change {
        n1084 = event-data() -> ()  [unwired: 1 in, 5 out]
        n1085 = property on="Cal/Data Acq. Spot" class="Bool (strict)"("Val(Sgnl)"=TRUE ("Value (Signaling)")) -> ()  [unwired: 2 in, 2 out]
        n1086 = property on="Main:" class="Bool (strict)"("Val(Sgnl)"=FALSE ("Value (Signaling)")) -> ()  [unwired: 2 in, 2 out]
      }
      event "Take Stepping Data": Value Change {
        n1087 = event-data() -> ()  [unwired: 1 in, 5 out]
        n1088 = local read "Save ave N"() -> (w1682:dbl)
        n1089 = flat-sequence {
          tunnel: w1682 -> [w1684]
          tunnel: [w1684] -> w1677
          tunnel: [w1686] -> w1678
          tunnel: w1677 -> [w1686]
          tunnel: [w1688] -> w1679
          tunnel: w1678 -> [w1688]
          tunnel: [w1691] -> w1680
          tunnel: w1679 -> [w1691]
          tunnel: [w1693] -> w1681
          tunnel: w1680 -> [w1693]
          tunnel: [w1695] -> w1675
          tunnel: w1681 -> [w1695]
          tunnel: w1675 -> [w1698]
          tunnel: [w1698] -> w1674
          tunnel: w1674 -> [w1699]
          tunnel: [w1699] -> w1676
          tunnel: w1676 -> [w1705]
          frame #0 {
            n1090 = property on="Save ave N" class="DigNum (strict)"("Val(Sgnl)"="Save ave factor") -> ()  [unwired: 2 in, 2 out]
          }
          frame #1 {
            n1091 = Wait (ms)(milliseconds to wait=u32 100) -> ()  [unwired: 1 out]
          }
          frame #2 {
            n1092 = local read "Offset 2 Start (MHz)"() -> (w1690:dbl)
            n1093 = property on="Saved AOD Raster Scan Parameter Sets" class="Arr (strict)"("Index Values"=u32[] [2]) -> ()  [unwired: 2 in, 2 out]
            n1094 = property on="Trap Delta (MHz)" class="DigNum (strict)"("Val(Sgnl)"=w1690) -> ()  [unwired: 2 in, 2 out]
          }
          frame #3 {
            n1095 = property on="Load parameters" class="Bool (strict)"("Val(Sgnl)"=TRUE ("Value (Signaling)")) -> ()  [unwired: 2 in, 2 out]
          }
          frame #4 {
            n1096 = Wait (ms)(milliseconds to wait=u32 100) -> ()  [unwired: 1 out]
          }
          frame #5 {
            n1097 = property on="Trap Raster Scan" class="Bool (strict)"("Val(Sgnl)"=TRUE ("Value (Signaling)")) -> ()  [unwired: 2 in, 2 out]
          }
          frame #6 {
            n1098 = Wait (ms)(milliseconds to wait=u32 1000) -> ()  [unwired: 1 out]
          }
          frame #7 {
            n1099 = while {
              stop <- w1702 stop-if-true
              n1100 = local read "Raster Scanning..."() -> (w1704:bool)
              n1101 = local read "Saving..."() -> (w1703:bool)
              n1102 = Not(x=w1703) -> (.not. x?=w1700:bool)
              n1103 = Not(x=w1704) -> (.not. x?=w1701:bool)
              n1104 = And(x=w1701, y=w1700) -> (x .and. y?=w1702:bool)
            }
          }
          frame #8 {
            n1105 = property on="Save ave N" class="DigNum (strict)"("Val(Sgnl)"=w1705) -> ()  [unwired: 2 in, 2 out]
          }
        }
      }
      event "Step Size (nm)": Value Change {
        n1106 = event-data() -> ()  [unwired: 1 in, 5 out]
        n1107 = flat-sequence {
          frame #0 {
            n1108 = property on="Saved AOD Raster Scan Parameter Sets" class="Arr (strict)"("Index Values"=u32[] [1]) -> ()  [unwired: 2 in, 2 out]
          }
          frame #1 {
            n1109 = Multiply(x="N Steps", y="Step Size (nm)") -> (x*y=w1707:dbl)
            n1110 = property on="Scan Speed AOD (nm/s) 2" class="DigNum (strict)"("Value"="Step Size (nm)") -> ()  [unwired: 2 in, 2 out]
            n1111 = property on="Step Size AOD (nm) 2" class="DigNum (strict)"("Value"="Step Size (nm)") -> ()  [unwired: 2 in, 2 out]
            n1112 = property on="Scan Range AOD (nm) 2" class="DigNum (strict)"("Value"=w1707) -> ()  [unwired: 2 in, 2 out]
          }
        }
      }
      event "Take Detection Laser\nImage": Value Change {
        n1113 = event-data() -> ()  [unwired: 1 in, 5 out]
        n1114 = flat-sequence {
          tunnel: [w1735] -> w1725
          tunnel: [w1734] -> w1718
          tunnel: [w1733] -> w1710
          tunnel: [w1738] -> w1726
          tunnel: w1725 -> [w1738]
          tunnel: [w1737] -> w1719
          tunnel: w1718 -> [w1737]
          tunnel: [w1736] -> w1711
          tunnel: w1710 -> [w1736]
          tunnel: [w1742] -> w1727
          tunnel: w1726 -> [w1742]
          tunnel: [w1741] -> w1720
          tunnel: w1719 -> [w1741]
          tunnel: [w1740] -> w1712
          tunnel: w1711 -> [w1740]
          tunnel: [w1748] -> w1728
          tunnel: w1727 -> [w1748]
          tunnel: [w1747] -> w1721
          tunnel: w1720 -> [w1747]
          tunnel: [w1746] -> w1713
          tunnel: w1712 -> [w1746]
          tunnel: [w1752] -> w1729
          tunnel: w1728 -> [w1752]
          tunnel: [w1751] -> w1722
          tunnel: w1721 -> [w1751]
          tunnel: [w1750] -> w1714
          tunnel: w1713 -> [w1750]
          tunnel: [w1756] -> w1730
          tunnel: w1729 -> [w1756]
          tunnel: [w1755] -> w1723
          tunnel: w1722 -> [w1755]
          tunnel: [w1754] -> w1715
          tunnel: w1714 -> [w1754]
          tunnel: [w1760] -> w1731
          tunnel: w1730 -> [w1760]
          tunnel: [w1759] -> w1724
          tunnel: w1723 -> [w1759]
          tunnel: [w1758] -> w1716
          tunnel: w1715 -> [w1758]
          tunnel: w1731 -> [w1766]
          tunnel: w1724 -> [w1765]
          tunnel: [w1763] -> w1717
          tunnel: w1716 -> [w1763]
          tunnel: w1717 -> [w1767]
          frame #0 {
            n1115 = local read "Green Laser ON/Interlacing"() -> (w1735:bool)
            n1116 = local read "Green laser mode"() -> (w1734:enum32{"Laser ON", "Laser OFF", "Interlace"})
            n1117 = local read "Green FB On/Off"() -> (w1733:bool)
          }
          frame #1 {
            n1118 = property on="Green FB On/Off" class="Bool (strict)"("Val(Sgnl)"=FALSE ("Value (Signaling)")) -> ()  [unwired: 2 in, 2 out]
          }
          frame #2 {
            n1119 = property on="Green Laser ON/Interlacing" class="Bool (strict)"("Val(Sgnl)"=TRUE ("Value (Signaling)")) -> ()  [unwired: 2 in, 2 out]
            n1120 = property on="Flip Green Filter" class="Bool (strict)"("Val(Sgnl)"=TRUE ("Value (Signaling)")) -> ()  [unwired: 2 in, 2 out]
            n1121 = property on="Green laser mode" class="RadioBtnsControl (strict)"("Val(Sgnl)"=enum32{"Laser ON", "Laser OFF", "Interlace"}."Laser ON" ("Value (Signaling)")) -> ()  [unwired: 2 in, 2 out]
          }
          frame #3 {
            n1122 = Wait (ms)(milliseconds to wait=u32 500) -> ()  [unwired: 1 out]
          }
          frame #4 {
            n1123 = property on="Confocal Image" class="Bool (strict)"("Val(Sgnl)"=TRUE ("Value (Signaling)")) -> ()  [unwired: 2 in, 2 out]
          }
          frame #5 {
            n1124 = Wait (ms)(milliseconds to wait=u32 2000) -> ()  [unwired: 1 out]
          }
          frame #6 {
            n1125 = while {
              stop <- w1761 stop-if-true
              n1126 = local read "Saving..."() -> (w1762:bool)
              n1127 = Not(x=w1762) -> (.not. x?=w1761:bool)
            }
          }
          frame #7 {
            n1128 = property on="Flip Green Filter" class="Bool (strict)"("Val(Sgnl)"=TRUE ("Value (Signaling)")) -> ()  [unwired: 2 in, 2 out]
            n1129 = property on="Green Laser ON/Interlacing" class="Bool (strict)"("Val(Sgnl)"=w1766) -> ()  [unwired: 2 in, 2 out]
            n1130 = property on="Green laser mode" class="RadioBtnsControl (strict)"("Val(Sgnl)"=w1765) -> ()  [unwired: 2 in, 2 out]
          }
          frame #8 {
            n1131 = property on="Green FB On/Off" class="Bool (strict)"("Val(Sgnl)"=w1767) -> ()  [unwired: 2 in, 2 out]
          }
        }
      }
      event "Stop All": Value Change {
        n1132 = event-data() -> ()  [unwired: 1 in, 5 out]
        n1133 = local read "Stop All"() -> (w1768:bool)
      }
    }
    n1134 = node-c288() -> ()  [unwired: 1 in, 1 out]
  }
  n1135 = node-c288() -> (w76:T24)  [unwired: 4 out]
  n1136 = timed-loop "Mouse control: trap position (AOM deflection), set confocal spot from image" {
    tunnel: [w1770] -> w34
    tunnel: w24 -> [w1769]
    timing: w76 -> [_]
    timing-out: [_] -> w75
    stop <- w1770 stop-if-true
    n1137 = node-c288() -> ()  [unwired: 2 out]
    n1138 = event shown="[0] \"Pane\": Mouse Down" {
      selector: _ -> [_ _]
      dyn-events: _ -> [_ _]
      timeout: _ -> [_ _]
      tunnel: w1769 -> [w1773 _]
      event Mouse Down {
        n1139 = event-data() -> ("Time"=w1775:u32, "Coords"=w1774:T8, "Button"=w1776:u16)  [unwired: 6 out]
        n1140 = case shown="1" w1776 {
          tunnel: w1775 -> [_ _ w1879]
          tunnel: w1774 -> [_ w1813 w1877]
          tunnel: w1773 -> [_ _ w1875]
          frame 0, Default {
          }
          frame 1 {
            n1141 = property on="APD 2" class="ImageControl"() -> ("Displayed Image Position"=w1783:cluster{"Left":i32, "Top":i32})  [unwired: 2 in, 2 out]
            n1142 = property on="APD 1" class="ImageControl"() -> ("Displayed Image Position"=w1812:cluster{"Left":i32, "Top":i32})  [unwired: 2 in, 2 out]
            n1143 = property on="Detection Laser X" class="ImageControl"() -> ("Displayed Image Position"=w1809:cluster{"Left":i32, "Top":i32})  [unwired: 2 in, 2 out]
            n1144 = property on="Detection Laser Y" class="ImageControl"() -> ("Displayed Image Position"=w1808:cluster{"Left":i32, "Top":i32})  [unwired: 2 in, 2 out]
            n1145 = property on="APD 2" class="ImageControl"() -> ("Displayed Image Size"=w1782:cluster{"Width":u32, "Height":u32})  [unwired: 2 in, 2 out]
            n1146 = property on="APD 1" class="ImageControl"() -> ("Displayed Image Size"=w1810:cluster{"Width":u32, "Height":u32})  [unwired: 2 in, 2 out]
            n1147 = property on="Detection Laser X" class="ImageControl"() -> ("Displayed Image Size"=w1811:cluster{"Width":u32, "Height":u32})  [unwired: 2 in, 2 out]
            n1148 = property on="Detection Laser Y" class="ImageControl"() -> ("Displayed Image Size"=w1807:cluster{"Width":u32, "Height":u32})  [unwired: 2 in, 2 out]
            n1149 = Unbundle By Name(w1782) -> ("Width"=w1779:u32, "Height"=w1778:u32)
            n1150 = Unbundle By Name(w1783) -> ("Left"=w1781:i32, "Top"=w1780:i32)
            n1151 = Unbundle By Name(w1810) -> ("Width"=w1804:u32, "Height"=w1803:u32)
            n1152 = Unbundle By Name(w1811) -> ("Width"=w1800:u32, "Height"=w1799:u32)
            n1153 = Unbundle By Name(w1807) -> ("Width"=w1796:u32, "Height"=w1795:u32)
            n1154 = Unbundle By Name(w1812) -> ("Left"=w1806:i32, "Top"=w1805:i32)
            n1155 = Unbundle By Name(w1809) -> ("Left"=w1802:i32, "Top"=w1801:i32)
            n1156 = Unbundle By Name(w1808) -> ("Left"=w1798:i32, "Top"=w1797:i32)
            n1157 = Bundle("Left"=w1781, "Top"=w1780, "Width"=w1779, "Height"=w1778) -> (w1777:T33)  [unwired: 1 in]
            n1158 = Bundle("Left"=w1806, "Top"=w1805, "Width"=w1804, "Height"=w1803) -> (w1794:T33)  [unwired: 1 in]
            n1159 = Bundle("Left"=w1802, "Top"=w1801, "Width"=w1800, "Height"=w1799) -> (w1793:T33)  [unwired: 1 in]
            n1160 = Bundle("Left"=w1798, "Top"=w1797, "Width"=w1796, "Height"=w1795) -> (w1792:T33)  [unwired: 1 in]
            n1161 = Build Cluster Array(w1777, w1794, w1793, w1792) -> (w1791:T34)
            n1162 = for {
              tunnel: w1813 -> [w1824]
              tunnel: w1791 -> [w1825] mode=indexing
              shift-right: [w1822] -> w1789
              shift-left: TRUE -> [w1823]
              shift-right: [w1821] -> w1787
              shift-left: _ -> [w1817]
              shift-right: [w1820] -> w1786
              shift-left: _ -> [w1816]
              shift-right: [w1819] -> w1785
              shift-left: _ -> [w1815]
              shift-right: [w1818] -> w1784
              shift-left: _ -> [w1814]
              n1163 = case shown="True" w1823 {
                selector: w1823 -> [w1830 _]
                tunnel: w1825 -> [_ w1839]
                tunnel: w1824 -> [_ w1837]
                tunnel: [w1830 w1835] -> w1822
                tunnel: [w1829 w1834] -> w1821
                tunnel: [w1828 w1833] -> w1820
                tunnel: [w1827 w1832] -> w1819
                tunnel: [w1826 w1831] -> w1818
                tunnel: w1817 -> [w1829 _]
                tunnel: w1816 -> [w1828 _]
                tunnel: w1815 -> [w1827 _]
                tunnel: w1814 -> [w1826 _]
                frame False {
                }
                frame True {
                  n1164 = Unbundle(w1839) -> (w1838:T33)
                  n1165 = call "isclickinwindow.vi"("Image Param"=w1838, "Point32"=w1837) -> ("4 Y"=w1831:i32, "3 Height"=w1832:i32, "2 X"=w1833:i32, "1 Width"=w1834:i32, "In image?"=w1836:bool)  [unwired: 1 in]
                  n1166 = Not(x=w1836) -> (.not. x?=w1835:bool)
                }
              }
            }
            n1167 = Not(x=w1789) -> (.not. x?=w1788:bool)
            n1168 = case shown="True" w1788 {
              tunnel: w1786 -> [_ w1852]
              tunnel: w1784 -> [_ w1851]
              tunnel: w1787 -> [_ w1850]
              tunnel: w1785 -> [_ w1849]
              frame False {
              }
              frame True {
                w1845 = FALSE ("Get Point")
                n1169 = local read "Scan lines (y)"() -> (w1854:u64)
                n1170 = local read "Actual MCL Inc (V)"() -> (w1846:dbl)
                n1171 = local read "Scan steps (MCL)"() -> (w1853:u64)
                n1172 = Divide "Y Pix/step"(x=w1849, y=w1854) -> (x/y=w1861:dbl)
                n1173 = Divide "Y V/pix"(x=w1846, y=w1861) -> (x/y=w1860:dbl)
                n1174 = Divide "Y half step offset"(x=w1846, y=2.0) -> (x/y=w1862:dbl)
                n1175 = Divide "X pix/step"(x=w1850, y=w1853) -> (x/y=w1859:dbl)
                n1176 = Negate(x=w1862) -> (-x=w1863:dbl)
                n1177 = local read "Initial Y"() -> (w1869:dbl)
                n1178 = Multiply(x=w1851, y=w1860) -> (x*y=w1870:dbl)
                n1179 = Divide "X half step offset"(x=w1846, y=2.0) -> (x/y=w1856:dbl)
                n1180 = Divide "X V/pix"(x=w1846, y=w1859) -> (x/y=w1858:dbl)
                n1181 = Multiply(x=w1846, y=w1853) -> (x*y=w1865:dbl)
                n1182 = Compound Arithmetic op=ADD(w1863, w1870, w1869) -> (w1847:dbl)
                "Pointer Y (V)" <- w1847
                n1183 = Multiply(x=w1858, y=w1852) -> (x*y=w1867:dbl)
                n1184 = Negate(x=w1856) -> (-x=w1855:dbl)
                n1185 = local read "Initial X"() -> (w1868:dbl)
                n1186 = Negate(x=w1867) -> (-x=w1866:dbl)
                n1187 = Compound Arithmetic op=ADD(w1855, w1865, w1868, w1866) -> (w1848:dbl)
                "Pointer X (V)" <- w1848
                n1188 = Or(x="Set X Only", y="Set Confocal Spot (X-Y)") -> (x .or. y?=w1841:bool)
                n1189 = Or(x="Set Confocal Spot (X-Y)", y="Set Y Only") -> (x .or. y?=w1840:bool)
                n1190 = case shown="True" w1841 {
                  tunnel: w1848 -> [_ w1871]
                  frame False {
                  }
                  frame True {
                    n1191 = property on="AO2" class="Slide (strict)"("Val(Sgnl)"=w1871) -> ()  [unwired: 2 in, 2 out]
                  }
                }
                n1192 = case shown="True" w1840 {
                  tunnel: w1847 -> [_ w1872]
                  frame False {
                  }
                  frame True {
                    n1193 = property on="AO1" class="Slide (strict)"("Val(Sgnl)"=w1872) -> ()  [unwired: 2 in, 2 out]
                  }
                }
                n1194 = local write "Set Confocal Spot (X-Y)"(w1845) -> ()
                n1195 = local write "Set X Only"(w1845) -> ()
                n1196 = local write "Set Y Only"(w1845) -> ()
              }
            }
          }
          frame 3 {
            n1197 = local read "BD 2 Frequency 1 (MHz)"() -> (w1873:dbl)
            n1198 = local read "BD 1 Frequency 1 (MHz)"() -> (w1874:dbl)
            n1199 = local write "Manipulating Trap"(TRUE ("Manipulating Trap")) -> ()
            n1200 = local write "Coords"(T8 {"Horizontal"=0, "Vertical"=0} ("Coords")) -> ()
            n1201 = while {
              tunnel: w1879 -> [w1884]
              tunnel: w1877 -> [w1883]
              tunnel: w1875 -> [w1882]
              tunnel: w1874 -> [w1881]
              tunnel: w1873 -> [w1880]
              stop <- w1885 stop-if-true
              n1202 = event shown="[0] \"Pane\": Mouse Move" {
                selector: _ -> [_ _]
                dyn-events: _ -> [_ _]
                timeout: _ -> [_ _]
                tunnel: ["Force Manip Abort" w1949] -> w1885
                tunnel: w1884 -> [w1892 _]
                tunnel: w1883 -> [w1890 _]
                tunnel: w1882 -> [w1889 _]
                tunnel: w1881 -> [w1888 _]
                tunnel: w1880 -> [w1887 _]
                event Mouse Move {
                  n1203 = event-data() -> ("Time"=w1893:u32, "Coords"=w1894:T8)  [unwired: 3 out]
                  n1204 = Less?(x=w1893, y=w1892) -> (x < y?=w1891:bool)
                  n1205 = case "Makes sure old motion events prior to mouse click aren't used" shown="False" w1891 {
                    tunnel: w1894 -> [w1936 _]
                    tunnel: w1890 -> [w1937 _]
                    tunnel: w1889 -> [w1914 _]
                    tunnel: w1888 -> [w1910 _]
                    tunnel: w1887 -> [w1909 _]
                    frame False {
                      n1206 = Subtract(x=w1936, y=w1937) -> (x-y=w1935:T8)
                      "Coords" <- w1935
                      n1207 = local read "Y RF Frequency Limits (MHz)"() -> (w1895:T16)
                      n1208 = To Double Precision Float(number=w1935) -> (double precision float=w1934:cluster{"Horizontal":dbl, "Vertical":dbl})
                      n1209 = Multiply(x=cluster{"Horizontal":dbl, "Vertical":dbl} {"Horizontal"=-1.0, "Vertical"=1.0}, y="Manipulation Scaling") -> (x*y=w1930:cluster{"Horizontal":dbl, "Vertical":dbl})
                      n1210 = local read "X RF Frequency Limits (MHz)"() -> (w1896:T16)
                      n1211 = Multiply(x=w1934, y=w1930) -> (x*y=w1932:cluster{"Horizontal":dbl, "Vertical":dbl})
                      n1212 = Unbundle By Name(w1932) -> ("Horizontal"=w1927:dbl, "Vertical"=w1931:dbl)
                      n1213 = Unbundle By Name(w1895) -> ("Maximum"=w1898:dbl, "Minimum"=w1897:dbl)
                      n1214 = Boolean To (0,1)(Boolean="Manip. X?") -> (0, 1=w1925:i16)
                      n1215 = Boolean To (0,1)(Boolean="Manip. Y?") -> (0, 1=w1922:i16)
                      n1216 = local read "BD 1 Frequency 2 (MHz)"() -> (w1912:dbl)
                      n1217 = Multiply(x=w1931, y=w1922) -> (x*y=w1924:dbl)
                      n1218 = Multiply(x=w1925, y=w1927) -> (x*y=w1928:dbl)
                      n1219 = local read "BD 2 Frequency 2 (MHz)"() -> (w1911:dbl)
                      n1220 = Unbundle By Name(w1896) -> ("Maximum"=w1900:dbl, "Minimum"=w1899:dbl)
                      n1221 = Add(x=w1909, y=w1924) -> (x+y=w1902:dbl)
                      n1222 = Add(x=w1910, y=w1928) -> (x+y=w1904:dbl)
                      n1223 = In Range and Coerce(upper limit=w1900, x=w1904, lower limit=w1899) -> (coerced(x)=w1903:dbl)  [unwired: 1 out]
                      n1224 = In Range and Coerce(upper limit=w1898, x=w1902, lower limit=w1897) -> (coerced(x)=w1901:dbl)  [unwired: 1 out]
                      n1225 = Subtract(x=w1903, y=w1912) -> (x-y=w1921:dbl)
                      n1226 = Subtract(x=w1901, y=w1911) -> (x-y=w1920:dbl)
                      n1227 = Square(x=w1921) -> (x^2=w1919:dbl)
                      n1228 = Square(x=w1920) -> (x^2=w1918:dbl)
                      n1229 = Add(x=w1919, y=w1918) -> (x+y=w1917:dbl)
                      n1230 = Square Root(x=w1917) -> (sqrt(x)=w1913:dbl)
                      n1231 = In Range and Coerce(upper limit="Limit Max (MHz)", x=w1913, lower limit="Limit Min (MHz)") -> (In Range?=w1906:bool)  [unwired: 1 out]
                      n1232 = Not(x="Limits Enable") -> (.not. x?=w1905:bool)
                      n1233 = Or(x=w1906, y=w1905) -> (x .or. y?=w1907:bool)
                      n1234 = case shown="True" w1907 {
                        tunnel: w1914 -> [_ w1947]
                        tunnel: w1913 -> [_ w1938]
                        tunnel: w1903 -> [_ w1945]
                        tunnel: w1912 -> [_ w1944]
                        tunnel: w1901 -> [_ w1943]
                        tunnel: w1911 -> [_ w1942]
                        tunnel: w1896 -> [_ w1940]
                        tunnel: w1895 -> [_ w1939]
                        frame False {
                        }
                        frame True {
                          n1235 = local read "BD 1 Frequency 3 (MHz)"() -> (w1946:dbl)
                          n1236 = local read "BD 2 Frequency 3 (MHz)"() -> (w1941:dbl)
                          n1237 = local write "Trap Delta (MHz)"(w1938) -> ()
                          n1238 = property on="Initial delta (MHz)" class="DigNum (strict)"("Val(Sgnl)"=w1938) -> ()  [unwired: 2 in, 2 out]
                          n1239 = call "set RF board frequency - interlace.vi"("Board 2 Frequency Limits"=w1939, "Board 1 Frequency Limits"=w1940, "FPGA VI Reference In"=w1947, "Board 2 Frequency 3 (MHz)"=w1941, "Board 1 Frequency 3 (MHz)"=w1946, "Board 2 Frequency 2 (MHz)"=w1942, "Board 2 Frequency 1 (MHz)"=w1943, "Board 1 Frequency 2 (MHz)"=w1944, "Board 1 Frequency 1  (MHz)"=w1945) -> ()  [unwired: 1 in, 2 out]
                          n1240 = local write "BD 2 Frequency 1 (MHz)"(w1943) -> ()
                          n1241 = local write "BD 1 Frequency 1 (MHz)"(w1945) -> ()
                        }
                      }
                    }
                    frame True {
                    }
                  }
                }
                event Mouse Up {
                  n1242 = event-data() -> ("Button"=w1948:u16)  [unwired: 8 out]
                  n1243 = case shown="3" w1948 {
                    tunnel: [FALSE TRUE] -> w1949
                    frame 0, Default {
                    }
                    frame 3 {
                      n1244 = local write "Manipulating Trap"(FALSE ("Manipulating Trap")) -> ()
                    }
                  }
                }
              }
            }
          }
        }
      }
      event Mouse Move {
        n1245 = event-data() -> ()  [unwired: 6 out]
      }
    }
    n1246 = local read "Stop All"() -> (w1770:bool)
    n1247 = node-c288() -> ()  [unwired: 2 out]
  }
  n1248 = node-c288(w14) -> ()  [unwired: 1 out]
  n1249 = node-c288(w68) -> ()  [unwired: 1 out]
  n1250 = node-c288(w75) -> ()  [unwired: 1 out]
  n1251 = node-c288(i64 1 ("Period"), 1 ("Processor")) -> (w164:T24)  [unwired: 2 out]
  n1252 = timed-loop "Acquire Data" {
    tunnel: w24 -> [w2218]
    tunnel: w40 -> [w2217]
    tunnel: [w2248] -> w33
    tunnel: [w2242] -> w32
    timing: w164 -> [_]
    timing-out: [_] -> w163
    tunnel: w59 -> [w2047]
    stop <- "Stop All" stop-if-true
    (unwired) u32 0 ("Number of Elements")
    w2034 = "NI_ChannelName" ("name")
    n1253 = node-c288() -> ()  [unwired: 2 out]
    n1254 = First Call?() -> (First Call?: T/F=w2000:bool)
    n1255 = Or(x="Reset", y=w2000) -> (x .or. y?=w2001:bool)
    n1256 = case "Reset data stream" shown="True" w2001 {
      tunnel: w2218 -> [w2264 w2272]
      tunnel: w2217 -> [w2263 w2271]
      tunnel: [w2264 w2266] -> w2213
      tunnel: [w2263 w2265] -> w2212
      frame False {
      }
      frame True {
        w2269 = TRUE ("AI to FIFO")
        n1257 = local write "Overflow (data lost)"(FALSE ("Overflow (data lost)")) -> ()
        n1258 = call "reset FPGA DMA.vi"("error in"=w2271, "FPGA VI Reference In"=w2272) -> ("error out"=w2267:errorcluster, "FPGA VI Reference Out"=w2268:T19)
        n1259 = xnode "Read/Write Control"("FPGA VI Reference In"=w2268, "error in"=w2267, "AI to FIFO"=w2269, "APD to FIFO"=w2269) -> ("FPGA VI Reference Out"=w2266:T19, "error out"=w2265:errorcluster)
      }
    }
    n1260 = Or(x="Start AOD Scan", y="Trap Raster Scan") -> (x .or. y?=w2163:bool)
    n1261 = case "Start AOM raster scan" shown="True" w2163 {
      tunnel: w2213 -> [w3001 w3011]
      tunnel: w2212 -> [w3000 w3010]
      tunnel: [w3001 w3004] -> w2211
      tunnel: [w3000 w3003] -> w2210
      frame False {
      }
      frame True {
        n1262 = case shown="True" "Restart DMA? (AOD)" {
          tunnel: [w3049 w3051] -> w3005
          tunnel: [w3048 w3050] -> w3006
          tunnel: w3011 -> [w3049 w3053]
          tunnel: w3010 -> [w3048 w3052]
          frame False {
          }
          frame True {
            n1263 = local write "Overflow (data lost)"(FALSE ("Overflow (data lost)")) -> ()
            n1264 = call "reset FPGA DMA.vi"("error in"=w3052, "FPGA VI Reference In"=w3053) -> ("error out"=w3050:errorcluster, "FPGA VI Reference Out"=w3051:T19)
          }
        }
        n1265 = local write "Trap Raster Scan"(FALSE ("Trap Raster Scan")) -> ()
        n1266 = case shown="True" "Move MCL Also?" {
          tunnel: w3006 -> [w3014 w3043]
          tunnel: w3005 -> [w3015 w3044]
          tunnel: [w3013 w3047] -> w3004
          tunnel: [w3012 w3046] -> w3003
          frame False {
            w3016 = TRUE ("AI to FIFO")
            n1267 = xnode "Read/Write Control"("FPGA VI Reference In"=w3015, "error in"=w3014, "AI to FIFO"=w3016, "APD to FIFO"=w3016, "Start scan"=w3016) -> ("FPGA VI Reference Out"=w3013:T19, "error out"=w3012:errorcluster)
          }
          frame True {
            w3040 = FALSE ("1D or 2D Scan?")
            w3045 = TRUE ("AI to FIFO")
            # "Count for MCL loop"
            # "N total cycles"
            # "N steps"
            # "V_int"
            n1268 = local read "Scan Range (nm)"() -> (w3022:dbl)
            n1269 = local read "Number of F/B Scans (AOD)"() -> (w3039:u16)
            n1270 = Sign(1:w3022) -> (0:w3021:dbl)
            n1271 = Compound Arithmetic op=MULTIPLY(w3022, "MCL Step Position Ratio", "MCL/AOM Scale Tweak") -> (w3026:dbl)
            n1272 = Negate(x=w3021) -> (-x=w3018:dbl)
            n1273 = Multiply(x=w3018, y="MCL Step Increment (V_int)") -> (x*y=w3020:dbl)
            n1274 = Divide(x=w3026, y="MCL X Cal (nm/V)") -> (x/y=w3032:dbl)
            n1275 = Multiply(x=32767.0 ("y"), y=w3032) -> (x*y=w3038:dbl)
            n1276 = local read "Total Counts (ticks)"() -> (w3023:u32)
            n1277 = local read "Cycles/step (AOD)"() -> (w3034:u64)
            n1278 = local read "Scan steps (AOD)"() -> (w3035:u64)
            n1279 = Divide(x=w3038, y=10.0) -> (x/y=w3031:dbl)
            n1280 = Divide(x=w3031, y="MCL Step Increment (V_int)") -> (x/y=w3029:dbl)
            n1281 = Absolute Value(x=w3029) -> (abs(x)=w3017:dbl)
            n1282 = Compound Arithmetic op=MULTIPLY(w3035, w3034, w3023) -> (w3030:u64)
            n1283 = local write "wait to reset values"(w3045) -> ()
            n1284 = local write "MCL Scanning"(w3045) -> ()
            n1285 = Divide(x=w3030, y=w3017) -> (x/y=w3027:dbl)
            "MCL Count" <- w3027
            n1286 = xnode "Read/Write Control"("FPGA VI Reference In"=w3044, "error in"=w3043, "Scan steps (MCL)"=w3017, "Number of scans (MCL)"=w3039, "Cycles per step (MCL)"=u64 1, "Scan freq.  increment (MCL)"=w3020, "1D or 2D Scan?"=w3040, "MCL Scan Axis"=w3040, "Cont. Scan (MCL)"=w3040, "MCL count"=w3027) -> ("FPGA VI Reference Out"=w3042:T19, "error out"=w3041:errorcluster)
            n1287 = xnode "Read/Write Control"("FPGA VI Reference In"=w3042, "error in"=w3041, "AI to FIFO"=w3045, "APD to FIFO"=w3045, "Start scan"=w3045, "Start scan (MCL)"=w3045) -> ("FPGA VI Reference Out"=w3047:T19, "error out"=w3046:errorcluster)
          }
        }
        "Raster Scanning..." <- TRUE ("Scanning...")
      }
    }
    n1288 = And(x="Save scans", y=w2163) -> (x .and. y?=w2209:bool)
    n1289 = Compound Arithmetic op=OR("Start MCL Scan", "Confocal Image", "Confocal Linescan") -> (w2161:bool)
    n1290 = And(x="Save Data (MCL)", y=w2161) -> (x .and. y?=w2208:bool)
    n1291 = case "Start MCL raster scan" shown="True" w2161 {
      tunnel: w2211 -> [w2555 w2570]
      tunnel: w2210 -> [w2554 w2569]
      tunnel: [w2555 w2565] -> w1969
      tunnel: [w2554 w2564] -> w1968
      tunnel: [FALSE w2563] -> w2194
      tunnel: "Start MCL Scan" -> [_ w2558]
      tunnel: "Confocal Image" -> [_ w2557]
      tunnel: "Confocal Linescan" -> [_ _]
      frame False {
      }
      frame True {
        w2563 = TRUE
        n1292 = case shown="True" "Restart DMA? (MCL)" {
          tunnel: [w2615 w2617] -> w2568
          tunnel: [w2614 w2616] -> w2567
          tunnel: w2570 -> [w2615 w2620]
          tunnel: w2569 -> [w2614 w2619]
          frame False {
          }
          frame True {
            n1293 = call "reset FPGA DMA.vi"("error in"=w2619, "FPGA VI Reference In"=w2620) -> ("error out"=w2616:errorcluster, "FPGA VI Reference Out"=w2617:T19)
            n1294 = local write "Overflow (data lost)"(FALSE ("Overflow (data lost)")) -> ()
          }
        }
        n1295 = case shown="False" w2558 {
          selector: w2558 -> [_ w2574]
          tunnel: w2557 -> [w2573 _]
          tunnel: [w2573 w2574] -> w2556
          frame False {
            n1296 = property on="2D or 1D Scan" class="Bool (strict)"("Val(Sgnl)"=w2573) -> ()  [unwired: 2 in, 2 out]
            n1297 = property on="Confocal Image" class="Bool (strict)"("Value"=FALSE ("Start Confocal Map")) -> ()  [unwired: 2 in, 2 out]
          }
          frame True {
          }
        }
        n1298 = local write "MCL Scanning"(w2563) -> ()
        n1299 = local read "AO1"() -> (w2560:dbl)
        n1300 = local read "AO2"() -> (w2559:dbl)
        n1301 = case shown="True" "Center Scan" {
          tunnel: w2568 -> [w2581 w2613]
          tunnel: w2567 -> [w2580 w2612]
          tunnel: [w2579 w2611] -> w2565
          tunnel: [w2578 w2610] -> w2564
          tunnel: [w2576 w2597] -> w2562
          tunnel: [w2575 w2596] -> w2561
          tunnel: w2560 -> [w2576 w2602]
          tunnel: w2559 -> [w2575 w2605]
          tunnel: w2556 -> [_ _]
          frame False {
            w2577 = TRUE ("AI to FIFO")
            n1302 = xnode "Read/Write Control"("FPGA VI Reference In"=w2581, "error in"=w2580, "AI to FIFO"=w2577, "APD to FIFO"=w2577, "Start scan (MCL)"=w2577) -> ("FPGA VI Reference Out"=w2579:T19, "error out"=w2578:errorcluster)
          }
          frame True {
            w2609 = TRUE ("AI to FIFO")
            n1303 = local read "Scan steps (MCL)"() -> (w2588:u64)
            n1304 = local read "Scan lines (y)"() -> (w2584:u64)
            n1305 = local read "Fast Scan Dir"() -> (w2595:bool)
            n1306 = local read "Actual MCL Inc (V)"() -> (w2585:dbl)
            n1307 = Decrement(x=w2584) -> (x-1=w2583:u64)
            n1308 = Decrement(x=w2588) -> (x-1=w2587:u64)
            n1309 = Multiply(x=w2585, y=w2583) -> (x*y=w2582:dbl)
            n1310 = Divide(x=w2582, y=2.0) -> (x/y=w2592:dbl)
            n1311 = Multiply(x=w2585, y=w2587) -> (x*y=w2586:dbl)
            n1312 = Divide(x=w2586, y=2.0) -> (x/y=w2591:dbl)
            n1313 = Select(t=w2591, s=w2595, f=w2592) -> (s? t:f=w2590:dbl)
            n1314 = Select(t=w2592, s=w2595, f=w2591) -> (s? t:f=w2594:dbl)
            n1315 = Subtract(x=w2602, y=w2594) -> (x-y=w2593:dbl)
            n1316 = Subtract(x=w2605, y=w2590) -> (x-y=w2589:dbl)
            n1317 = local read "2D or 1D Scan"() -> (w2607:bool)
            n1318 = Not(x=w2595) -> (.not. x?=w2601:bool)
            n1319 = Not(x=w2607) -> (.not. x?=w2603:bool)
            n1320 = And(x=w2595, y=w2603) -> (x .and. y?=w2604:bool)
            n1321 = And(x=w2603, y=w2601) -> (x .and. y?=w2606:bool)
            n1322 = Select(t=w2605, s=w2606, f=w2589) -> (s? t:f=w2596:dbl)
            n1323 = Select(t=w2602, s=w2604, f=w2593) -> (s? t:f=w2597:dbl)
            n1324 = call "Volt to I16.vi"("Voltage In"=w2597) -> ("I16 Voltage Out"=w2600:i16)
            n1325 = call "Volt to I16.vi"("Voltage In"=w2596) -> ("I16 Voltage Out"=w2599:i16)
            n1326 = xnode "Read/Write Control"("FPGA VI Reference In"=w2613, "error in"=w2612, "AI to FIFO"=w2609, "APD to FIFO"=w2609, "Start scan (MCL)"=w2609, "AO1"=w2600, "AO2"=w2599) -> ("FPGA VI Reference Out"=w2611:T19, "error out"=w2610:errorcluster)
          }
        }
        "Initial Y" <- w2562
        "Initial X" <- w2561
        "wait to reset values" <- w2563
      }
    }
    n1327 = local read "Trap Pos Elements/DMA read"() -> (w2043:u32)
    n1328 = local read "Trap AI Elements/DMA read"() -> (w1967:u32)
    n1329 = local read "APD Elements/DMA read"() -> (w2086:u32)
    n1330 = local read "Trap AI FIFO Depth"() -> (w2258:u32)
    n1331 = xnode "Invoke Method"("FPGA VI Reference In"=w1969, "error in"=w1968, "Number of Elements"=w2043, "Timeout (ms)"=-1) -> ("Data"=w2007:u16[], "Elements Remaining"=→"Trap Pos FIFO El Remaining":u32)  [unwired: 2 out]
    n1332 = xnode "Invoke Method"("FPGA VI Reference In"=w1969, "error in"=w1968, "Number of Elements"=w1967, "Timeout (ms)"=-1 ("Timeout")) -> ("FPGA VI Reference Out"=w1971:T19, "error out"=w1970:errorcluster, "Data"=w1966:i16[], "Elements Remaining"=w1972:u32)
    "Trap AI FIFO El. Rem." <- w1972
    n1333 = xnode "Get APD Data"("FPGA VI Reference In"=w1969, "error in"=w1968, "Number of Elements"=w2086, "Timeout (ms)"=-1) -> ("Data"=w2085:u32[], "Elements Remaining"=→"APD FIFO Elements Remaining":u32)  [unwired: 2 out]
    n1334 = Subtract(x=w2258, y=w1967) -> (x-y=w2257:u32)
    n1335 = Decimate 1D Array(w2007) -> (w2004:u16[], w2006:u16[], w2005:u16[])
    n1336 = Divide(x=w1972, y=w2257) -> (x/y=w2256:dbl)
    "Buffer Status" <- w2256
    n1337 = To Unsigned Long Integer(number=w2004) -> (unsigned 32bit integer=w2003:u32[])
    n1338 = Join Numbers(hi=w2006, lo=w2005) -> ((hi.lo)=w2002:u32[])
    n1339 = Equal?(x=w2256, y=1.0) -> (x = y?=w2254:bool)
    n1340 = Join Numbers(hi=w2003, lo=w2002) -> ((hi.lo)=w1996:u64[])
    n1341 = call "IR AOM word to freq - vec.vi"("Frequency Word In (double vec)"=w1996) -> ("Frequency Out"=w2042:dbl[])
    n1342 = case "Alert buffer overflow" shown="True" w2254 {
      frame False {
      }
      frame True {
        n1343 = call <vilib>:"Beep.vi"() -> ()  [unwired: 3 in, 9 out]
        "Overflow (data lost)" <- TRUE ("Overflow (data lost)")
      }
    }
    n1344 = Decimate 1D Array(w2042) -> (w2041:dbl[], w2040:dbl[])
    n1345 = Array Size(array=w1966) -> (size(s)=→"Waveform Chart":i32)
    n1346 = Build Array(w2041, w2040) -> (w2039:dbl[][])
    n1347 = local read "Trap Sets"() -> (w2123:u32)
    n1348 = case "Deinterlace trap data, average down PSD" shown="2" w2123 {
      tunnel: w1966 -> [w2650 w2715]
      tunnel: [w2647 w2712] -> w2116
      tunnel: [w2650 w2714] -> w1999
      tunnel: "Detector Type" -> [w2649 w2710]
      tunnel: [w2648 w2713] -> w2115
      tunnel: [w2646 w2711] -> w2229
      frame 1, Default {
        n1349 = Divide(x=w2650, y=3276.7) -> (x/y=w2651:dbl[])
        n1350 = Decimate 1D Array(w2651) -> (w2660:dbl[], w2659:dbl[], w2658:dbl[], w2657:dbl[], w2656:dbl[], w2655:dbl[], w2654:dbl[], w2653:dbl[])
        n1351 = case shown="\"IR-QPD + PSD + FB-QPD position\"" w2649 {
          tunnel: w2660 -> [w2684 w2709]
          tunnel: w2659 -> [w2683 w2708]
          tunnel: w2658 -> [w2668 w2686]
          tunnel: w2657 -> [w2669 w2696]
          tunnel: w2656 -> [w2682 w2707]
          tunnel: w2655 -> [w2681 w2706]
          tunnel: w2654 -> [w2665 w2687]
          tunnel: w2653 -> [w2664 w2685]
          tunnel: [w2663 w2693] -> w2648
          tunnel: [w2662 w2692] -> w2647
          tunnel: [w2661 w2691] -> w2646
          frame "IR-QPD + PSD + FB-QPD", Default {
            w2661 = 0  # Channel pattern
            n1352 = Divide(x=w2684, y=w2669) -> (x/y=w2671:dbl[])
            n1353 = Divide(x=w2683, y=w2669) -> (x/y=w2670:dbl[])
            n1354 = Divide(x=w2682, y=w2665) -> (x/y=w2667:dbl[])
            n1355 = Divide(x=w2681, y=w2664) -> (x/y=w2666:dbl[])
            n1356 = Build Array(w2671, w2670, w2669, w2668, w2667, w2666, w2665, w2664) -> (w2662:dbl[][])
            n1357 = Bundle("T1 Y", "T1 X", "T1 Sum", "FB Sum", "PSD Y", "PSD X", "PSD Y Sum", "PSD X Sum") -> (w2680:T41)  [unwired: 1 out]
            n1358 = Cluster To Array(cluster=w2680) -> (array=w2663:string[])
          }
          frame "IR-QPD + PSD + FB-QPD position" {
            w2691 = 3  # Channel pattern
            n1359 = Negate(x=w2687) -> (-x=w2688:dbl[])
            n1360 = Divide(x=w2709, y=w2696) -> (x/y=w2698:dbl[])
            n1361 = Divide(x=w2708, y=w2696) -> (x/y=w2697:dbl[])
            n1362 = Divide(x=w2707, y=w2687) -> (x/y=w2695:dbl[])
            n1363 = Divide(x=w2706, y=w2688) -> (x/y=w2694:dbl[])
            n1364 = Build Array(w2698, w2697, w2696, w2685, w2686, w2695, w2694, w2687) -> (w2692:dbl[][])
            n1365 = Bundle("T1 Y", "T1 X", "T1 Sum", "FB X", "FB Sum", "PSD Y", "PSD X", "PSD Y Sum") -> (w2705:T41)  [unwired: 1 out]
            n1366 = Cluster To Array(cluster=w2705) -> (array=w2693:string[])
          }
        }
      }
      frame 2 {
        n1367 = case shown="\"UCB Fleezers 052511\"" w2710 {
          tunnel: w2715 -> [w2777 w2844 w2872 w2979]
          tunnel: [w2716 w2836 w2867 w2910] -> w2714
          tunnel: [w2743 w2827 w2869 w2957] -> w2713
          tunnel: [w2742 w2791 w2846 w2924] -> w2712
          tunnel: [w2736 w2826 w2909 w2955] -> w2711
          frame "IR-QPD + PSD + FB-QPD", Default {
            w2736 = 1  # Channel pattern
            # "time average x2 the 4th signal and the 4 psd signals (detection laser)"
            # "deinterlace 3 signals from qpd"
            n1368 = Decimate 1D Array(w2777) -> (w2776:i16[], w2775:i16[], w2741:i16[], w2774:i16[], w2764:i16[], w2762:i16[], w2761:i16[], w2759:i16[])
            n1369 = call "downsample 1D array - double.vi"("Ave N"=2.0, "Array In"=w2764) -> ("Array Out"=w2763:dbl[])  [unwired: 1 out]
            n1370 = call "downsample 1D array - double.vi"("Ave N"=2.0, "Array In"=w2759) -> ("Array Out"=w2758:dbl[])  [unwired: 1 out]
            n1371 = call "downsample 1D array - double.vi"("Ave N"=2.0, "Array In"=w2761) -> ("Array Out"=w2760:dbl[])  [unwired: 1 out]
            n1372 = call "downsample 1D array - double.vi"("Ave N"=2.0, "Array In"=w2762) -> ("Array Out"=w2744:dbl[])  [unwired: 1 out]
            n1373 = Decimate 1D Array(w2776) -> (w2773:i16[], w2745:i16[])
            n1374 = Decimate 1D Array(w2775) -> (w2772:i16[], w2770:i16[])
            n1375 = Decimate 1D Array(w2774) -> (w2771:i16[], w2769:i16[])
            n1376 = Decimate 1D Array(w2741) -> (w2740:i16[], w2739:i16[])
            n1377 = Interleave 1D Arrays(w2773, w2772, w2771, w2745, w2770, w2769, w2740, w2739, w2763, w2744, w2760, w2758) -> (w2757:dbl[])
            n1378 = To Word Integer(number=w2757) -> (16bit integer=w2716:i16[])
            n1379 = Divide(x=w2757, y=3276.7) -> (x/y=w2756:dbl[])
            n1380 = Decimate 1D Array(w2756) -> (w2755:dbl[], w2754:dbl[], w2753:dbl[], w2752:dbl[], w2751:dbl[], w2750:dbl[], w2738:dbl[], w2737:dbl[], w2749:dbl[], w2748:dbl[], w2747:dbl[], w2746:dbl[])
            n1381 = Divide(x=w2755, y=w2753) -> (x/y=w2723:dbl[])
            n1382 = Divide(x=w2754, y=w2753) -> (x/y=w2722:dbl[])
            n1383 = Divide(x=w2752, y=w2750) -> (x/y=w2721:dbl[])
            n1384 = Divide(x=w2751, y=w2750) -> (x/y=w2720:dbl[])
            n1385 = Divide(x=w2749, y=w2747) -> (x/y=w2719:dbl[])
            n1386 = Divide(x=w2748, y=w2746) -> (x/y=w2718:dbl[])
            n1387 = Bundle("T1 Y", "T1 X", "T1 Sum", "T2 Y", "T2 X", "T2 Sum", "T1 FB Sum", "T2 FB Sum", "PSD Y", "PSD X", "PSD Y Sum", "PSD X Sum") -> (w2724:T42)  [unwired: 1 out]
            n1388 = Build Array(w2723, w2722, w2753, w2721, w2720, w2750, w2738, w2737, w2719, w2718, w2747, w2746) -> (w2742:dbl[][])
            n1389 = Cluster To Array(cluster=w2724) -> (array=w2743:string[])
          }
          frame "IR-QPD + PSD + FB-QPD X position" {
            w2826 = 2  # Channel pattern
            # "convert\nADC numbers\nto volts"
            # "time average x2 the 3 psd signals (detection laser)"
            # "deinterlace 3 signals from qpds"
            n1390 = Decimate 1D Array(w2844) -> (w2843:i16[], w2842:i16[], w2779:i16[], w2780:i16[], w2789:i16[], w2786:i16[], w2783:i16[], w2814:i16[])
            n1391 = Decimate 1D Array(w2843) -> (w2841:i16[], w2828:i16[])
            n1392 = call "downsample 1D array - I16.vi"("Ave N"=2.0, "Array In"=w2789) -> ("Array Out"=w2787:i16[])  [unwired: 1 in]
            n1393 = call "downsample 1D array - I16.vi"("Ave N"=2.0, "Array In"=w2786) -> ("Array Out"=w2784:i16[])  [unwired: 1 in]
            n1394 = Decimate 1D Array(w2842) -> (w2840:i16[], w2838:i16[])
            n1395 = Decimate 1D Array(w2780) -> (w2839:i16[], w2837:i16[])
            n1396 = Decimate 1D Array(w2814) -> (w2813:i16[], w2811:i16[])
            n1397 = Decimate 1D Array(w2779) -> (w2812:i16[], w2810:i16[])
            n1398 = call "downsample 1D array - I16.vi"("Ave N"=2.0, "Array In"=w2783) -> ("Array Out"=w2781:i16[])  [unwired: 1 in]
            n1399 = Interleave 1D Arrays(w2841, w2840, w2839, w2828, w2838, w2837, w2813, w2812, w2811, w2810, w2787, w2784, w2781) -> (w2836:i16[])
            n1400 = Divide(x=w2836, y=3276.7) -> (x/y=w2835:dbl[])
            n1401 = Decimate 1D Array(w2835) -> (w2834:dbl[], w2833:dbl[], w2832:dbl[], w2831:dbl[], w2830:dbl[], w2829:dbl[], w2802:dbl[], w2800:dbl[], w2799:dbl[], w2797:dbl[], w2796:dbl[], w2795:dbl[], w2792:dbl[])
            n1402 = Divide(x=w2834, y=w2832) -> (x/y=w2818:dbl[])
            n1403 = Divide(x=w2833, y=w2832) -> (x/y=w2817:dbl[])
            n1404 = Divide(x=w2831, y=w2829) -> (x/y=w2816:dbl[])
            n1405 = Divide(x=w2830, y=w2829) -> (x/y=w2815:dbl[])
            n1406 = Divide(x=w2802, y=w2800) -> (x/y=w2801:dbl[])
            n1407 = Divide(x=w2799, y=w2797) -> (x/y=w2798:dbl[])
            n1408 = Divide(x=w2796, y=w2792) -> (x/y=w2794:dbl[])
            n1409 = Negate(x=w2792) -> (-x=w2790:dbl[])
            n1410 = Divide(x=w2795, y=w2790) -> (x/y=w2793:dbl[])
            n1411 = Bundle("T1 Y", "T1 X", "T1 Sum", "T2 Y", "T2 X", "T2 Sum", "T1 FB X", "T1 FB Sum", "T2 FB X", "T2 FB Sum", "PSD Y", "PSD X", "PSD Y Sum") -> (w2819:T43)  [unwired: 1 out]
            n1412 = Build Array(w2818, w2817, w2832, w2816, w2815, w2829, w2801, w2800, w2798, w2797, w2794, w2793, w2792) -> (w2791:dbl[][])
            n1413 = Cluster To Array(cluster=w2819) -> (array=w2827:string[])
          }
          frame "UCB Fleezers 052511" {
            w2909 = 2  # Channel pattern
            n1414 = Decimate 1D Array(w2872) -> (w2907:i16[], w2906:i16[], w2871:i16[], w2870:i16[], w2864:i16[], w2861:i16[], w2860:i16[], w2859:i16[])
            n1415 = Decimate 1D Array(w2907) -> (w2905:i16[], w2890:i16[])
            n1416 = Decimate 1D Array(w2906) -> (w2904:i16[], w2902:i16[])
            n1417 = Decimate 1D Array(w2871) -> (w2903:i16[], w2901:i16[])
            n1418 = Decimate 1D Array(w2870) -> (w2866:i16[], w2865:i16[])
            n1419 = Decimate 1D Array(w2864) -> (w2863:i16[], w2862:i16[])
            n1420 = call "downsample 1D array - I16.vi"("Ave N"=2.0, "Array In"=w2861) -> ("Array Out"=w2858:i16[])  [unwired: 1 in]
            n1421 = call "downsample 1D array - I16.vi"("Ave N"=2.0, "Array In"=w2860) -> ("Array Out"=w2857:i16[])  [unwired: 1 in]
            n1422 = call "downsample 1D array - I16.vi"("Ave N"=2.0, "Array In"=w2859) -> ("Array Out"=w2856:i16[])  [unwired: 1 in]
            n1423 = Interleave 1D Arrays(w2905, w2904, w2903, w2890, w2902, w2901, w2866, w2863, w2865, w2862, w2858, w2857, w2856) -> (w2867:i16[])
            n1424 = Divide(x=w2867, y=3276.7) -> (x/y=w2897:dbl[])
            n1425 = Decimate 1D Array(w2897) -> (w2896:dbl[], w2895:dbl[], w2894:dbl[], w2893:dbl[], w2892:dbl[], w2891:dbl[], w2855:dbl[], w2853:dbl[], w2852:dbl[], w2850:dbl[], w2849:dbl[], w2848:dbl[], w2847:dbl[])
            n1426 = Divide(x=w2896, y=w2894) -> (x/y=w2877:dbl[])
            n1427 = Divide(x=w2895, y=w2894) -> (x/y=w2876:dbl[])
            n1428 = Divide(x=w2893, y=w2891) -> (x/y=w2875:dbl[])
            n1429 = Divide(x=w2892, y=w2891) -> (x/y=w2874:dbl[])
            n1430 = Divide(x=w2855, y=w2853) -> (x/y=w2854:dbl[])
            n1431 = Divide(x=w2852, y=w2850) -> (x/y=w2851:dbl[])
            n1432 = Bundle("T1 Y", "T1 X", "T1 Sum", "T2 Y", "T2 X", "T2 Sum", "T1 FB X", "T2 FB Sum", "T2 FB X", "T2 FB Sum", "PSD Y", "PSD X", "PSD Sum") -> (w2878:T43)  [unwired: 1 out]
            n1433 = Build Array(w2877, w2876, w2894, w2875, w2874, w2891, w2854, w2853, w2851, w2850, w2849, w2848, w2847) -> (w2846:dbl[][])
            n1434 = Cluster To Array(cluster=w2878) -> (array=w2869:string[])
          }
          frame "IR-QPD + PSD + FB-QPD XY positions" {
            w2955 = 4  # Channel pattern
            # "time average x2 the 3 psd signals (detection laser)"
            # "deinterlace 3 signals from qpds"
            n1435 = Decimate 1D Array(w2979) -> (w2978:i16[], w2977:i16[], w2956:i16[], w2976:i16[], w2922:i16[], w2968:i16[], w2967:i16[], w2944:i16[])
            n1436 = Decimate 1D Array "QPD Y"(w2978) -> (w2975:i16[], w2958:i16[])
            n1437 = call "downsample 1D array - double.vi"("Ave N"=2.0, "Array In"=w2968) -> ("Array Out"=w2943:dbl[])  [unwired: 1 out]
            n1438 = call "downsample 1D array - double.vi"("Ave N"=2.0, "Array In"=w2967) -> ("Array Out"=w2942:dbl[])  [unwired: 1 out]
            n1439 = Decimate 1D Array "Feedback Sum"(w2956) -> (w2940:i16[], w2938:i16[])
            n1440 = Decimate 1D Array "Feedback Y"(w2922) -> (w2921:i16[], w2920:i16[])
            n1441 = Decimate 1D Array "Feedback X"(w2944) -> (w2941:i16[], w2939:i16[])
            n1442 = Decimate 1D Array "QPD Sum"(w2976) -> (w2973:i16[], w2971:i16[])
            n1443 = Decimate 1D Array "QPD X"(w2977) -> (w2974:i16[], w2972:i16[])
            n1444 = Interleave 1D Arrays(w2975, w2974, w2973, w2958, w2972, w2971, w2921, w2941, w2940, w2920, w2939, w2938, w2943, w2942) -> (w2966:dbl[])
            n1445 = To Word Integer(number=w2966) -> (16bit integer=w2910:i16[])
            n1446 = Divide(x=w2966, y=3276.7) -> (x/y=w2965:dbl[])
            n1447 = Decimate 1D Array(w2965) -> (w2964:dbl[], w2963:dbl[], w2962:dbl[], w2961:dbl[], w2960:dbl[], w2959:dbl[], w2917:dbl[], w2931:dbl[], w2915:dbl[], w2916:dbl[], w2929:dbl[], w2913:dbl[], w2927:dbl[], w2925:dbl[])
            n1448 = Divide(x=w2964, y=w2962) -> (x/y=w2948:dbl[])
            n1449 = Divide(x=w2963, y=w2962) -> (x/y=w2947:dbl[])
            n1450 = Divide(x=w2961, y=w2959) -> (x/y=w2946:dbl[])
            n1451 = Divide(x=w2960, y=w2959) -> (x/y=w2945:dbl[])
            n1452 = Divide(x=w2917, y=w2915) -> (x/y=w2914:dbl[])
            n1453 = Divide(x=w2931, y=w2915) -> (x/y=w2930:dbl[])
            n1454 = Divide(x=w2916, y=w2913) -> (x/y=w2912:dbl[])
            n1455 = Divide(x=w2929, y=w2913) -> (x/y=w2928:dbl[])
            n1456 = Negate(x=w2925) -> (-x=w2923:dbl[])
            n1457 = Divide(x=w2927, y=w2923) -> (x/y=w2926:dbl[])
            n1458 = Bundle("T1 Y", "T1 X", "T1 Sum", "T2 Y", "T2 X", "T2 Sum", "T1 FB Y", "T1 FB X", "T1 FB Sum", "T2 FB Y", "T2 FB X", "T2 FB Sum", "PSD X", "PSD Y Sum") -> (w2911:T44)  [unwired: 1 out]
            n1459 = Build Array(w2948, w2947, w2962, w2946, w2945, w2959, w2914, w2930, w2915, w2912, w2928, w2913, w2926, w2925) -> (w2924:dbl[][])
            n1460 = Cluster To Array(cluster=w2911) -> (array=w2957:string[])
          }
        }
      }
    }
    "AI labels" <- w2115
    n1461 = Decimate 1D Array(w2085) -> (w2113:u32[], w2049:u32[])
    n1462 = local read "DMA Update Period (s)"() -> (w2124:dbl)
    n1463 = local read "BD 1 Frequency 2 (MHz)"() -> (w1991:dbl)
    n1464 = local read "BD 1 Frequency 1 (MHz)"() -> (w1992:dbl)
    n1465 = Build Array(w2113, w2049) -> (w2191:u32[][])
    n1466 = local read "Data Period (s)"() -> (w2098:dbl)
    n1467 = Decimate 1D Array(w1999) -> (w2022:i16[], w2021:i16[], w2019:i16[], w2018:i16[])  [unwired: 9 out]
    n1468 = To Double Precision Float(number=w2191) -> (double precision float=w2192:dbl[][])
    n1469 = local read "APD Integration Time (s)"() -> (w2062:dbl)
    n1470 = Divide(x=w2022, y=w2021) -> (x/y=w2023:dbl[])
    n1471 = Divide(x=w2019, y=w2018) -> (x/y=w2020:dbl[])
    n1472 = feedback #1(0.0) -> (w2036:dbl)
    n1473 = Add(x=w2124, y=w2036) -> (x+y=w2231:dbl)
    n1474 = feedback-in #1(w2231) -> ()
    n1475 = local read "AOM X Cal (nm/MHz)"() -> (w1989:dbl)
    n1476 = To Time Stamp(1:w2036) -> (0:w2035:timestamp)
    n1477 = Split 1D Array(array=w2023, index="N El. to Ave.") -> (second subarray=w2026:dbl[])  [unwired: 1 out]
    n1478 = Split 1D Array(array=w2020, index="N El. to Ave.") -> (second subarray=w2025:dbl[])  [unwired: 1 out]
    n1479 = local read "Trap X AI1 (DMA)"() -> (w2024:T13)
    n1480 = Multiply(x=w2098, y="Trap Disp. Downsample") -> (x*y=w2037:dbl)
    "Display Period (s)" <- w2037
    n1481 = Bundle("BD 1 Frequency 1 (MHz)"=w1992, "BD 1 Frequency 2 (MHz)"=w1991) -> (w1993:T45)  [unwired: 1 out]
    n1482 = for "Trap AI" {
      tunnel: [w2645] -> w2225 mode=indexing
      tunnel: w2035 -> [w2635]
      tunnel: "Trap Disp. Downsample" -> [w2643]
      tunnel: w2116 -> [w2641] mode=indexing
      tunnel: w2098 -> [w2640]
      tunnel: w2115 -> [w2639] mode=indexing
      tunnel: w2034 -> [w2638]
      tunnel: [w2637] -> w2073 mode=indexing
      tunnel: w2037 -> [w2636]
      n1483 = Bundle By Name("Y"=w2641, "dt"=w2640) -> (w2642:waveform(dbl))  [unwired: 1 out]
      n1484 = Set Waveform Attribute(5:w2639, 6:w2638, 7:w2642) -> (3:w2637:waveform(dbl))  [unwired: 1 in, 2 out]
      n1485 = call "downsample 1D array - double.vi"("Ave N"=w2643, "Array In"=w2641) -> ("Array Out"=w2644:dbl[])  [unwired: 1 out]
      n1486 = Bundle By Name(cluster=w2637, "t0"=w2635, "Y"=w2644, "dt"=w2636) -> (w2645:waveform(dbl))
    }
    n1487 = call-poly <vilib>:"Mean.vi"("X"=w2025) -> ("mean"=w2013:dbl)  [unwired: 1 out]
    n1488 = call-poly <vilib>:"Mean.vi"("X"=w2026) -> ("mean"=w2014:dbl)  [unwired: 1 out]
    n1489 = Cluster To Array(cluster=w1993) -> (array=w1990:dbl[])
    n1490 = Reciprocal(x=w2037) -> (1/x=→"Trap Disp. Freq. (Hz)":dbl)
    n1491 = local read "Data points/scans (MCL)"() -> (w2203:dbl)
    n1492 = To Fixed-Point(number=w2013) -> (fixed-point=w2011:fxp<+/-,16,1>)  [unwired: 1 in]
    n1493 = To Fixed-Point(number=w2014) -> (fixed-point=w2012:fxp<+/-,16,1>)  [unwired: 1 in]
    n1494 = Bundle("Trap 1 Pos.", "Trap 2 Pos.") -> (w2033:cluster{string, string})  [unwired: 1 out]
    n1495 = Bundle By Name(cluster=w2024, "Set 1"=w2012, "Set 2"=w2011) -> (→"Trap X AI1 (DMA)":T13)
    n1496 = Cluster To Array(cluster=w2033) -> (array=w2030:string[])
    n1497 = for "Trap Position" {
      tunnel: w2039 -> [w2285] mode=indexing
      tunnel: "Trap Disp. Downsample" -> [w2284]
      tunnel: w2037 -> [w2282]
      tunnel: w2035 -> [w2281]
      tunnel: w2034 -> [w2279]
      tunnel: w2030 -> [w2278] mode=indexing
      tunnel: [w2277] -> w1988 mode=indexing
      tunnel: w1990 -> [w2275] mode=indexing
      tunnel: w1989 -> [w2273]
      n1498 = call "downsample 1D array - double.vi"("Ave N"=w2284, "Array In"=w2285) -> ("Array Out"=w2283:dbl[])  [unwired: 1 out]
      n1499 = Subtract(x=w2283, y=w2275) -> (x-y=w2276:dbl[])
      n1500 = Multiply(x=w2273, y=w2276) -> (x*y=w2274:dbl[])
      n1501 = Bundle By Name("Y"=w2274, "dt"=w2282, "t0"=w2281) -> (w2280:waveform(dbl))  [unwired: 1 out]
      n1502 = Set Waveform Attribute(5:w2278, 6:w2279, 7:w2280) -> (3:w2277:waveform(dbl))  [unwired: 1 in, 2 out]
    }
    "Trap Positions" <- w1988
    n1503 = Bundle("APD 1", "APD 2") -> (w2224:cluster{string, string})  [unwired: 1 out]
    n1504 = Cluster To Array(cluster=w2224) -> (array=w2221:string[])
    n1505 = for "APD" {
      tunnel: w2192 -> [w2624] mode=indexing
      tunnel: w2062 -> [w2632]
      tunnel: [w2628] -> w2069 mode=indexing
      tunnel: "APD Disp. Scale" -> [w2629]
      tunnel: w2034 -> [w2627]
      tunnel: w2221 -> [w2626] mode=indexing
      tunnel: "APD Disp. Downsample" -> [w2622]
      tunnel: [w2625] -> w2220
      tunnel: w2035 -> [w2621]
      n1506 = call "integrate 1D array interval - double.vi"("Ave N"=w2622, "Array In"=w2624) -> ("Array Out"=w2623:dbl[])  [unwired: 1 out]
      n1507 = Multiply(x=w2632, y=w2622) -> (x*y=w2625:dbl)
      n1508 = Divide(x=w2623, y=w2629) -> (x/y=w2630:dbl[])
      n1509 = Bundle By Name("t0"=w2621, "Y"=w2630, "dt"=w2625) -> (w2631:waveform(dbl))  [unwired: 1 out]
      n1510 = Set Waveform Attribute(5:w2626, 6:w2627, 7:w2631) -> (3:w2628:waveform(dbl))  [unwired: 1 in, 2 out]
    }
    "APD Display Period (s)" <- w2220
    n1511 = Reciprocal(x=w2220) -> (1/x=→"APD Display Freq. (Hz)":dbl)
    n1512 = local read "Display Period (s)"() -> (w2097:dbl)
    n1513 = Increment(x=w2203) -> (x+1=w2204:dbl)
    n1514 = Index Array(array=w1988, index=0) -> (element=w1986:waveform(dbl))
    n1515 = To Double Precision Float(number=w2113) -> (double precision float=w2112:dbl[])
    n1516 = feedback #2(w2204) -> (w2207:dbl)
    n1517 = Select(t=0, s=w2194, f=w2207) -> (s? t:f=w2200:dbl)
    n1518 = Array Size(array=w2112) -> (size(s)=w2206:i32)
    n1519 = Add(x=w2206, y=w2200) -> (x+y=w2201:dbl)
    n1520 = Unbundle By Name(w1986) -> ("Y"=w1984:dbl[])
    n1521 = feedback #3(w2113) -> (w2190:u32[])
    n1522 = Build Array (concatenate)(w2190, w2113) -> (w2187:u32[])
    n1523 = feedback #4(w2049) -> (w2068:u32[])
    n1524 = Divide(x="Bead Sep. Int. Time (s)", y=w2097) -> (x/y=w1982:dbl)
    n1525 = Build Array (concatenate)(w2068, w2049) -> (w2067:u32[])
    n1526 = Greater?(x=w2201, y=w2203) -> (0:w2202:bool)
    n1527 = feedback #5(w1984) -> (w1985:dbl[])
    n1528 = Build Array (concatenate)(w1984, w1985) -> (w1983:dbl[])
    n1529 = Select(t=w2200, s=w2202, f=w2201) -> (s? t:f=w2199:dbl)
    n1530 = feedback-in #2(w2199) -> ()
    n1531 = Array Size(array=w2187) -> (size(s)=w2184:i32)
    n1532 = Array Size(array=w2113) -> (size(s)=w2186:i32)
    n1533 = local read "MCL Scanning"() -> (w2197:bool)
    n1534 = local read "APD Integration Time (s)"() -> (w2076:dbl)
    n1535 = Build Array (concatenate)(w2069, w2225) -> (w2071:waveform(dbl)[])
    "All Signals" <- w2071
    n1536 = Split 1D Array(array=w1983, index=w1982) -> (first subarray=w1976:dbl[])  [unwired: 1 out]
    n1537 = feedback-in #5(w1976) -> ()
    n1538 = Multiply(x=w2186, y="APD Ave N") -> (x*y=w2185:dbl)
    n1539 = Greater?(x=w2184, y=w2185) -> (0:w2188:bool)
    n1540 = Not(x=w2202) -> (.not. x?=w2196:bool)
    n1541 = To Double Precision Float(number=w2049) -> (double precision float=w2048:dbl[])
    n1542 = call-poly <vilib>:"Mean.vi"("X"=w1976) -> ("mean"=w1975:dbl)  [unwired: 1 out]
    "Mean T1 Position (nm)" <- w1975
    n1543 = Subtract(x=w1976, y=w1975) -> (x-y=w1981:dbl[])
    n1544 = Square(x=w1981) -> (x^2=w1980:dbl[])
    n1545 = And(x=w2196, y=w2197) -> (x .and. y?=w2198:bool)
    n1546 = call-poly <vilib>:"Mean.vi"("X"=w1980) -> ("mean"=w1979:dbl)  [unwired: 1 out]
    n1547 = case shown="True" w2188 {
      tunnel: w2187 -> [w2405 w2412]
      tunnel: [w2405 w2410] -> w2129
      tunnel: w2185 -> [_ w2407]
      tunnel: w2184 -> [_ w2411]
      tunnel: w2067 -> [w2404 w2409]
      tunnel: [w2404 w2406] -> w2064
      frame False {
      }
      frame True {
        n1548 = Subtract(x=w2411, y=w2407) -> (x-y=w2408:dbl)
        n1549 = Array Subset(array=w2412, index=w2408, length=w2407) -> (w2410:u32[])
        n1550 = Array Subset(array=w2409, index=w2408, length=w2407) -> (w2406:u32[])
      }
    }
    n1551 = feedback-in #3(w2129) -> ()
    n1552 = feedback-in #4(w2064) -> ()
    n1553 = Or(x=w2198, y=w2194) -> (x .or. y?=w2195:bool)
    n1554 = Square Root(x=w1979) -> (sqrt(x)=w1978:dbl)
    n1555 = Equal?(x="Tab Control 6", y=T35."High Res Display") -> (x = y?=w2119:bool)
    n1556 = Multiply(x="APD Disp. Scale", y=w2069) -> (x*y=w2078:waveform(dbl)[])
    n1557 = Multiply(x="APD Disp. Downsample", y=w2076) -> (x*y=w2074:dbl)
    n1558 = Multiply(x=10.0, y=w1978) -> (x*y=→"Trap 1 Position RMS (A)":dbl)
    n1559 = Divide(x=w2078, y=w2074) -> (x/y=w2046:waveform(dbl)[])
    n1560 = Index Array(array=w2046, index=0) -> (element=w2056:waveform(dbl))
    n1561 = case "For computing FFTs for display" shown="True" "Compute FFT" {
      tunnel: w2073 -> [_ w3082]
      frame False {
      }
      frame True {
        n1562 = Build Array("FFT 1 Choice 1", "FFT 1 Choice 2", "FFT 2 Choice 1", "FFT 2 Choice 2") -> (w3075:u16[])
        n1563 = Array Size(array=w3082) -> (size(s)=w3081:i32)
        n1564 = feedback-in #6(w3075) -> ()
        n1565 = feedback #6(u16[] [100, 100, 100, 100]) -> (w3076:u16[])
        n1566 = feedback-in #7("# Spectra to Ave.") -> ()
        n1567 = feedback #7("# Spectra to Ave.") -> (w3073:dbl)
        n1568 = Not Equal?(x="# Spectra to Ave.", y=w3073) -> (x != y?=w3072:bool)
        n1569 = Not Equal?(x=w3075, y=w3076) -> (x != y?=w3074:bool)
        n1570 = feedback #8(1.0) -> (w3059:dbl)
        n1571 = Compound Arithmetic op=OR("Reset FFT", w3074, w3072) -> (w3057:bool)
        n1572 = Select(t=1.0, s=w3057, f=w3059) -> (s? t:f=w3061:dbl)
        n1573 = Greater?(x=w3061, y="# Spectra to Ave.") -> (0:w3080:bool)
        n1574 = Increment(x=w3061) -> (x+1=w3060:dbl)
        n1575 = feedback-in #8(w3060) -> ()
        n1576 = local read "DMA Update Period (s)"() -> (w3055:dbl)
        n1577 = Multiply(x="# Spectra to Ave.", y=w3055) -> (x*y=→"Ave. Time (s)":dbl)
        n1578 = Build Array(cluster{"f0":dbl, "df":dbl, "magnitude":dbl[]} {"f0"=0.0, "df"=0.0, "magnitude"=[]} ("PSD")) -> (w3064:cluster{"f0":dbl, "df":dbl, "magnitude":dbl[]}[])
        n1579 = Build Array(w3064, w3064, w3064, w3064) -> (w3066:T46)
        n1580 = feedback #9(w3066) -> (w3071:T46)
        n1581 = for {
          N: 4 -> [_]
          tunnel: w3075 -> [w3104] mode=indexing
          tunnel: w3082 -> [w3105]
          tunnel: w3081 -> [w3107]
          tunnel: w3057 -> [w3100]
          tunnel: w3080 -> [w3099]
          tunnel: "# Spectra to Ave." -> [w3098]
          tunnel: [w3097] -> w3070 mode=indexing
          tunnel: w3071 -> [w3102] mode=indexing
          tunnel: [w3101] -> w3058 mode=indexing
          tunnel: w3061 -> [w3096]
          n1582 = Less?(x=w3104, y=w3107) -> (x < y?=w3106:bool)
          n1583 = Index Array(array=w3105, index=w3104) -> (element=w3103:waveform(dbl))
          n1584 = case shown="True" w3106 {
            tunnel: w3103 -> [_ w3124]
            tunnel: w3102 -> [w3109 w3122]
            tunnel: [w3109 w3110] -> w3101
            tunnel: w3100 -> [_ w3121]
            tunnel: w3099 -> [_ w3114]
            tunnel: w3098 -> [_ w3113]
            tunnel: [cluster{"f0":dbl, "df":dbl, "magnitude":dbl[]} {"f0"=0.0, "df"=0.0, "magnitude"=[]} ("PSD") w3115] -> w3097
            tunnel: w3096 -> [_ w3112]
            frame False {
            }
            frame True {
              n1585 = call <vilib>:"Std Deviation and Variance.vi"("X"=w3124) -> ("mean"=w3125:dbl)  [unwired: 1 in, 2 out]
              n1586 = Subtract(x=w3124, y=w3125) -> (x-y=w3123:waveform(dbl))
              n1587 = xnode "Spectral Measurements"("Signals"=w3123) -> ("PSD"=w3117:cluster{"f0":dbl, "df":dbl, "magnitude":dbl[]})  [unwired: 1 in, 1 out]
              n1588 = case shown="False" w3121 {
                tunnel: w3122 -> [w3134 _]
                tunnel: [w3130 w3139] -> w3110
                tunnel: w3117 -> [w3133 w3140]
                tunnel: w3114 -> [w3132 _]
                frame False {
                  n1589 = Build Array (concatenate)(w3134, w3133) -> (w3131:cluster{"f0":dbl, "df":dbl, "magnitude":dbl[]}[])
                  n1590 = case shown="True" w3132 {
                    tunnel: w3131 -> [w3135 w3138]
                    tunnel: [w3135 w3136] -> w3130
                    frame False {
                    }
                    frame True {
                      n1591 = Delete From Array(array=w3138, index=0) -> (array with subset deleted=w3136:cluster{"f0":dbl, "df":dbl, "magnitude":dbl[]}[])  [unwired: 1 in, 1 out]
                    }
                  }
                }
                frame True {
                  n1592 = Build Array(w3140) -> (w3139:cluster{"f0":dbl, "df":dbl, "magnitude":dbl[]}[])
                }
              }
              n1593 = for {
                tunnel: w3110 -> [w3129] mode=indexing
                tunnel: [w3128] -> w3120 mode=indexing
                workers-P: _ -> [_]
                n1594 = Unbundle By Name(w3129) -> ("magnitude"=w3128:dbl[])
              }
              n1595 = Transpose 2D Array(2D array=w3120) -> (transposed array=w3119:dbl[][])
              n1596 = for {
                tunnel: w3119 -> [w3127] mode=indexing
                tunnel: [w3126] -> w3118 mode=indexing
                workers-P: _ -> [_]
                n1597 = Add Array Elements(numeric array=w3127) -> (sum=w3126:dbl)
              }
              n1598 = Select(t=w3113, s=w3114, f=w3112) -> (s? t:f=w3111:dbl)
              n1599 = Divide(x=w3118, y=w3111) -> (x/y=w3116:dbl[])
              n1600 = Bundle By Name(cluster=w3117, "magnitude"=w3116) -> (w3115:cluster{"f0":dbl, "df":dbl, "magnitude":dbl[]})
            }
          }
        }
        n1601 = case shown="True" w3057 {
          tunnel: w3058 -> [w3089 w3095]
          tunnel: [w3089 w3090] -> w3056
          frame False {
          }
          frame True {
            n1602 = Array Subset(array=w3095, index (row)=0 ("index"), length (row)=4 ("length"), index (col)=0 ("index"), length (col)=1 ("length")) -> (w3090:T46)
          }
        }
        n1603 = feedback-in #9(w3056) -> ()
        n1604 = Split 1D Array(array=w3070, index=2) -> (first subarray=→"FFT 1":cluster{"f0":dbl, "df":dbl, "magnitude":dbl[]}[], second subarray=→"FFT 2":cluster{"f0":dbl, "df":dbl, "magnitude":dbl[]}[])
      }
    }
    n1605 = Index Array(array=w2046, index=1) -> (element=w2054:waveform(dbl))
    n1606 = case "For displaying the high resolution display (no downsampling)" shown="True" w2119 {
      tunnel: w2073 -> [_ w2305]
      frame False {
      }
      frame True {
        n1607 = Index Array(array=w2305, index="High Res. Display") -> (element=w2306:waveform(dbl))
        n1608 = call <vilib>:"Std Deviation and Variance.vi"("X"=w2306) -> ("mean"=w2313:dbl, "standard deviation"=w2318:dbl)  [unwired: 1 in, 1 out]
        "Mean Intensity" <- w2313
        "Sigma" <- w2318
        n1609 = Subtract(x=w2306, y=w2313) -> (x-y=w2312:waveform(dbl))
        n1610 = Select(t=w2312, s="Subtract mean", f=w2306) -> (s? t:f=→"1 Channel":waveform(dbl))
        n1611 = Divide(x=w2318, y=w2313) -> (x/y=→"Sigma/Mean":dbl)
        n1612 = feedback #10(1) -> (w2307:i32)
        n1613 = Greater Or Equal?(x=w2307, y="Slow mean N ave.") -> (x >= y?=w2320:bool)
        n1614 = Increment(x=w2307) -> (x+1=w2322:i32)
        n1615 = Select(t=1, s=w2320, f=w2322) -> (s? t:f=w2309:i32)
        n1616 = feedback-in #10(w2309) -> ()
        n1617 = feedback #11() -> (w2310:waveform(dbl))  [unwired: 1 out]
        n1618 = case shown="Default" w2307 {
          tunnel: [w2325 w2328] -> w2311
          tunnel: w2310 -> [w2327 _]
          tunnel: w2306 -> [w2326 w2328]
          frame Default {
            n1619 = call-poly <vilib>:"Append Waveforms.vi"("waveform B"=w2326, "waveform A"=w2327) -> ("waveform out"=w2325:waveform(dbl))  [unwired: 1 in, 8 out]
          }
          frame 1 {
          }
        }
        n1620 = feedback-in #11(w2311) -> ()
        n1621 = case shown="True" w2320 {
          tunnel: w2311 -> [_ w2324]
          frame False {
          }
          frame True {
            n1622 = call-poly <vilib>:"Mean.vi"("X"=w2324) -> ("mean"=→"Slow mean":dbl)  [unwired: 1 out]
          }
        }
      }
    }
    n1623 = case "For plotting results of scanning MCL" shown="True" w2195 {
      tunnel: w2194 -> [_ w2445]
      tunnel: w2112 -> [_ w2541]
      tunnel: w2203 -> [_ _]
      tunnel: w2073 -> [_ w2515]
      tunnel: w2048 -> [_ w2446]
      tunnel: w2047 -> [_ w2419]
      frame False {
      }
      frame True {
        w2426 = u32 0 items=["Horizontal", "Vertical", "Central", "1st Diagonal", "2nd Diagonal"] ("Type of Symmetry")
        w2454 = u32 0 items=["Horizontal", "Vertical", "Central", "1st Diagonal", "2nd Diagonal"] ("Type of Symmetry")
        w2457 = u32 0 items=["Horizontal", "Vertical", "Central", "1st Diagonal", "2nd Diagonal"] ("Type of Symmetry")
        w2486 = u32 0 items=["Horizontal", "Vertical", "Central", "1st Diagonal", "2nd Diagonal"] ("Type of Symmetry")
        n1624 = Index Array(array=w2515, index=10) -> (element=w2521:waveform(dbl))
        n1625 = Index Array(array=w2515, index=11) -> (element=w2518:waveform(dbl))
        n1626 = local read "Cycles/step (MCL)"() -> (w2471:u64)
        n1627 = Index Array(array=w2515, index="Channel") -> (element=w2517:waveform(dbl))
        n1628 = Unbundle(w2419) -> ("New Image"=w2418:T3, "New Image"=w2417:T3, "New Image"=w2416:T3, "New Image"=w2415:T3)
        n1629 = Unbundle By Name(w2521) -> ("Y"=w2473:dbl[])
        n1630 = Unbundle By Name(w2518) -> ("Y"=w2475:dbl[])
        n1631 = Unbundle By Name(w2517) -> ("Y"=w2480:dbl[])
        n1632 = call "downsample 1D array - double.vi"("Ave N"=w2471, "Array In"=w2473) -> ("Array Out"=w2472:dbl[])  [unwired: 1 out]
        n1633 = call "downsample 1D array - double.vi"("Ave N"=w2471, "Array In"=w2475) -> ("Array Out"=w2474:dbl[])  [unwired: 1 out]
        n1634 = call "downsample 1D array - double.vi"("Ave N"=w2471, "Array In"=w2480) -> ("Array Out"=w2479:dbl[])  [unwired: 1 out]
        n1635 = feedback #12(w2541) -> (w2542:dbl[])
        n1636 = Build Array (concatenate)(w2542, w2541) -> (w2523:dbl[])
        n1637 = feedback #13(w2446) -> (w2448:dbl[])
        n1638 = Build Array (concatenate)(w2448, w2446) -> (w2447:dbl[])
        n1639 = local read "Scan steps (MCL)"() -> (w2428:u64)
        n1640 = Select(t=w2541, s=w2445, f=w2523) -> (s? t:f=w2527:dbl[])
        n1641 = feedback-in #12(w2527) -> ()
        n1642 = Select(t=w2446, s=w2445, f=w2447) -> (s? t:f=w2429:dbl[])
        n1643 = feedback-in #13(w2429) -> ()
        n1644 = local read "Scan lines (y)"() -> (w2414:u64)
        n1645 = local read "N APD Samp/step"() -> (w2430:dbl)
        n1646 = feedback #14(w2472) -> (w2529:dbl[])
        n1647 = Build Array (concatenate)(w2529, w2472) -> (w2520:dbl[])
        n1648 = feedback #15(w2479) -> (w2539:dbl[])
        n1649 = Build Array (concatenate)(w2539, w2479) -> (w2538:dbl[])
        n1650 = feedback #16(w2474) -> (w2531:dbl[])
        n1651 = Build Array (concatenate)(w2531, w2474) -> (w2532:dbl[])
        n1652 = Select(t=w2472, s=w2445, f=w2520) -> (s? t:f=w2476:dbl[])
        n1653 = feedback-in #14(w2476) -> ()
        n1654 = Select(t=w2479, s=w2445, f=w2538) -> (s? t:f=w2478:dbl[])
        n1655 = feedback-in #15(w2478) -> ()
        n1656 = Select(t=w2474, s=w2445, f=w2532) -> (s? t:f=w2477:dbl[])
        n1657 = feedback-in #16(w2477) -> ()
        n1658 = Multiply(x=w2428, y=u64 2) -> (x*y=w2413:u64)
        n1659 = call "integrate 1D array interval - double.vi"("Ave N"=w2430, "Array In"=w2429) -> ("Array Out"=w2441:dbl[])  [unwired: 1 out]
        n1660 = call "integrate 1D array interval - double.vi"("Ave N"=w2430, "Array In"=w2527) -> ("Array Out"=w2526:dbl[])  [unwired: 1 out]
        n1661 = Array Size(array=w2441) -> (size(s)=w2442:i32)
        n1662 = Array Size(array=w2526) -> (size(s)=w2528:i32)
        n1663 = Multiply(x=w2414, y=w2413) -> (x*y=w2444:u64)
        n1664 = Multiply(x=w2414, y=w2413) -> (x*y=w2536:u64)
        n1665 = call-poly <vilib>:"Mean.vi"("X"=w2476) -> ("mean"=w2460:dbl)  [unwired: 1 out]
        n1666 = Subtract(x=w2444, y=w2442) -> (x-y=w2435:u64)
        n1667 = call-poly <vilib>:"Mean.vi"("X"=w2478) -> ("mean"=w2465:dbl)  [unwired: 1 out]
        n1668 = call-poly <vilib>:"Mean.vi"("X"=w2477) -> ("mean"=w2463:dbl)  [unwired: 1 out]
        n1669 = call-poly <vilib>:"Mean.vi"("X"=w2441) -> ("mean"=w2432:dbl)  [unwired: 1 out]
        n1670 = Subtract(x=w2536, y=w2528) -> (x-y=w2470:u64)
        n1671 = call-poly <vilib>:"Mean.vi"("X"=w2526) -> ("mean"=w2467:dbl)  [unwired: 1 out]
        n1672 = Initialize Array(1.0 ("element"), w2435) -> (w2431:dbl[])
        n1673 = Initialize Array(1.0 ("element"), w2470) -> (w2461:dbl[])
        n1674 = Multiply(x=w2431, y=w2432) -> (x*y=w2433:dbl[])
        n1675 = Multiply(x=w2461, y=w2463) -> (x*y=w2464:dbl[])
        n1676 = Multiply(x=w2461, y=w2465) -> (x*y=w2466:dbl[])
        n1677 = Multiply(x=w2461, y=w2460) -> (x*y=w2462:dbl[])
        n1678 = Multiply(x=w2461, y=w2467) -> (x*y=w2468:dbl[])
        n1679 = Build Array (concatenate)(w2476, w2462) -> (w2530:dbl[])
        n1680 = Build Array (concatenate)(w2478, w2466) -> (w2534:dbl[])
        n1681 = Build Array (concatenate)(w2477, w2464) -> (w2533:dbl[])
        n1682 = Build Array (concatenate)(w2441, w2433) -> (w2443:dbl[])
        n1683 = Build Array (concatenate)(w2526, w2468) -> (w2535:dbl[])
        n1684 = Reshape Array(w2530, w2414, w2413) -> (w2496:dbl[][])
        n1685 = Reshape Array(w2443, w2414, w2413) -> (w2439:dbl[][])
        n1686 = Reshape Array(w2534, w2414, w2413) -> (w2488:dbl[][])
        n1687 = Reshape Array(w2533, w2414, w2413) -> (w2503:dbl[][])
        n1688 = Reshape Array(w2535, w2414, w2413) -> (w2513:dbl[][])
        n1689 = Array Subset(array=w2503, index (col)=0 ("index"), length (col)=w2428) -> (w2508:dbl[][])  [unwired: 2 in]
        n1690 = Array Subset(array=w2503, index (col)=w2428) -> (w2506:dbl[][])  [unwired: 3 in]
        n1691 = Array Subset(array=w2488, index (col)=0 ("index"), length (col)=w2428) -> (w2494:dbl[][])  [unwired: 2 in]
        n1692 = Array Subset(array=w2488, index (col)=w2428) -> (w2492:dbl[][])  [unwired: 3 in]
        n1693 = Array Subset(array=w2439, index (col)=0 ("index"), length (col)=w2428) -> (w2438:dbl[][])  [unwired: 2 in]
        n1694 = Array Subset(array=w2439, index (col)=w2428) -> (w2436:dbl[][])  [unwired: 3 in]
        n1695 = Array Subset(array=w2513, index (col)=0 ("index"), length (col)=w2428) -> (w2512:dbl[][])  [unwired: 2 in]
        n1696 = Array Subset(array=w2513, index (col)=w2428) -> (w2510:dbl[][])  [unwired: 3 in]
        n1697 = Array Subset(array=w2496, index (col)=0 ("index"), length (col)=w2428) -> (w2501:dbl[][])  [unwired: 2 in]
        n1698 = Array Subset(array=w2496, index (col)=w2428) -> (w2499:dbl[][])  [unwired: 3 in]
        n1699 = for {
          tunnel: w2508 -> [w2550] mode=indexing
          tunnel: [w2549] -> w2507 mode=indexing
          workers-P: _ -> [_]
          n1700 = Reverse 1D Array(array=w2550) -> (reversed array=w2549:dbl[])
        }
        n1701 = for {
          tunnel: w2494 -> [w2546] mode=indexing
          tunnel: [w2545] -> w2493 mode=indexing
          workers-P: _ -> [_]
          n1702 = Reverse 1D Array(array=w2546) -> (reversed array=w2545:dbl[])
        }
        n1703 = for {
          tunnel: w2438 -> [w2544] mode=indexing
          tunnel: [w2543] -> w2437 mode=indexing
          workers-P: _ -> [_]
          n1704 = Reverse 1D Array(array=w2544) -> (reversed array=w2543:dbl[])
        }
        n1705 = for {
          tunnel: w2512 -> [w2552] mode=indexing
          tunnel: [w2551] -> w2511 mode=indexing
          workers-P: _ -> [_]
          n1706 = Reverse 1D Array(array=w2552) -> (reversed array=w2551:dbl[])
        }
        n1707 = for {
          tunnel: w2501 -> [w2548] mode=indexing
          tunnel: [w2547] -> w2500 mode=indexing
          workers-P: _ -> [_]
          n1708 = Reverse 1D Array(array=w2548) -> (reversed array=w2547:dbl[])
        }
        n1709 = Index Array(array=w2513, index (row)=0) -> (element=→"Waveform Graph":dbl[])  [unwired: 1 in]
        n1710 = Add(x=w2507, y=w2506) -> (x+y=w2505:dbl[][])
        n1711 = Add(x=w2493, y=w2492) -> (x+y=w2491:dbl[][])
        n1712 = Add(x=w2437, y=w2436) -> (x+y=w2421:dbl[][])
        n1713 = Add(x=w2511, y=w2510) -> (x+y=w2485:dbl[][])
        n1714 = Add(x=w2500, y=w2499) -> (x+y=w2498:dbl[][])
        n1715 = Divide(x=w2491, y=2) -> (x/y=w2489:dbl[][])
        n1716 = Divide(x=w2505, y=2) -> (x/y=w2450:dbl[][])
        n1717 = Divide(x=w2498, y=2) -> (x/y=w2452:dbl[][])
        n1718 = To Single Precision Float(number=w2485) -> (single precision float=w2484:sgl[][])
        n1719 = Transpose 2D Array(2D array=w2489) -> (transposed array=→"Data map":dbl[][])
        n1720 = To Single Precision Float(number=w2421) -> (single precision float=w2425:sgl[][])
        n1721 = To Single Precision Float(number=w2450) -> (single precision float=w2456:sgl[][])
        n1722 = To Single Precision Float(number=w2452) -> (single precision float=w2453:sgl[][])
        n1723 = call "IMAQ ArrayToImage"("Image Pixels (Float)"=w2484, "Image"=w2418) -> ("Image Out"=w2487:T3)  [unwired: 8 in, 1 out]
        n1724 = call "IMAQ ArrayToImage"("Image Pixels (Float)"=w2425, "Image"=w2417) -> ("Image Out"=w2427:T3)  [unwired: 8 in, 1 out]
        n1725 = call "IMAQ ArrayToImage"("Image Pixels (Float)"=w2456, "Image"=w2416) -> ("Image Out"=w2458:T3)  [unwired: 8 in, 1 out]
        n1726 = call "IMAQ ArrayToImage"("Image Pixels (Float)"=w2453, "Image"=w2415) -> ("Image Out"=w2455:T3)  [unwired: 8 in, 1 out]
        n1727 = call "IMAQ Symmetry"("Type of Symmetry"=w2486, "Image Src"=w2487) -> ("Image Dst Out"=w2482:T3)  [unwired: 3 in, 1 out]
        n1728 = call "IMAQ Symmetry"("Type of Symmetry"=w2426, "Image Src"=w2427) -> ("Image Dst Out"=w2423:T3)  [unwired: 3 in, 1 out]
        n1729 = call "IMAQ Symmetry"("Type of Symmetry"=w2457, "Image Src"=w2458) -> ("Image Dst Out"=→"Detection Laser X":T3)  [unwired: 3 in, 1 out]
        n1730 = call "IMAQ Symmetry"("Type of Symmetry"=w2454, "Image Src"=w2455) -> ("Image Dst Out"=→"Detection Laser Y":T3)  [unwired: 3 in, 1 out]
        n1731 = call "IMAQ Set Simple Calibration"("Calibration Axis Info"=T36 {"Origin Pixel"={"X"=0.0, "Y"=0.0}, "Angle Relative to Horizontal (deg)"=0.0, "Axis Reference"=0}, "Grid Descriptor"=T37 {"X Step"=0.3, "Y Step"=0.3, "Unit"=enum."Undefined"}, "Image"=w2482) -> ("Calibrated Image"=→"APD 1":T3)  [unwired: 7 in, 1 out]
        n1732 = call "IMAQ Set Simple Calibration"("Calibration Axis Info"=T36 {"Origin Pixel"={"X"=0.0, "Y"=0.0}, "Angle Relative to Horizontal (deg)"=0.0, "Axis Reference"=0}, "Grid Descriptor"=T37 {"X Step"=0.3, "Y Step"=0.3, "Unit"=enum."Undefined"}, "Image"=w2423) -> ("Calibrated Image"=→"APD 2":T3)  [unwired: 7 in, 1 out]
      }
    }
    n1733 = Subtract(x=w2054, y="APD 2 Offset") -> (x-y=w2051:waveform(dbl))
    n1734 = Subtract(x=w2056, y="APD 1 Offset") -> (x-y=w2052:waveform(dbl))
    n1735 = Index Array(array=w2071, index=3) -> (element=w2139:waveform(dbl))
    n1736 = Index Array(array=w2071, index=6) -> (element=w2136:waveform(dbl))
    n1737 = Build Array(w2052, w2051) -> (→"APD Chart":waveform(dbl)[])
    n1738 = Array Size(array=w2129) -> (size(s)=w2183:i32)
    n1739 = call <vilib>:"Std Deviation and Variance.vi"("X"=w2064) -> ("standard deviation"=w2063:dbl)  [unwired: 1 in, 2 out]
    n1740 = Add Array Elements(numeric array=w2064) -> (sum=w2066:u32)
    n1741 = Add Array Elements(numeric array=w2129) -> (sum=w2193:u32)
    n1742 = call <vilib>:"Std Deviation and Variance.vi"("X"=w2129) -> ("standard deviation"=w2128:dbl)  [unwired: 1 in, 2 out]
    n1743 = Divide(x="T1 offset_x (mV)", y=1000.0) -> (x/y=w2140:dbl)
    n1744 = Divide(x=w2063, y=w2062) -> (x/y=w2059:dbl)
    "Rate sigma (Hz) 2" <- w2059
    n1745 = Multiply(x=w2062, y=w2183) -> (x*y=w2065:dbl)
    "Int. Time (s)" <- w2065
    n1746 = Divide(x=w2066, y=w2065) -> (x/y=w2060:dbl)
    "APD 2 Rate (Hz)" <- w2060
    n1747 = Divide(x=w2193, y=w2065) -> (x/y=w2126:dbl)
    "APD 1 Rate (Hz)" <- w2126
    n1748 = Divide(x=w2128, y=w2062) -> (x/y=w2127:dbl)
    "Rate sigma (Hz)" <- w2127
    n1749 = Divide(x=w2059, y=w2060) -> (x/y=→"Sigma/Mean 2":dbl)
    n1750 = Divide(x=w2127, y=w2126) -> (x/y=→"Sigma/Mean":dbl)
    n1751 = Divide(x="T2 offset_x (mV)", y=1000.0) -> (x/y=w2138:dbl)
    n1752 = case shown="1" "Calibration" {
      tunnel: "T1 alpha_x (nm/V)" -> [_ w2381 w2402]
      tunnel: "T1 kappa_x (pN/nm)" -> [_ _ w2392]
      tunnel: "T2 alpha_x (nm/V)" -> [_ w2380 w2400]
      tunnel: "T2 kappa_x (pN/nm)" -> [_ _ w2393]
      tunnel: w2139 -> [w2363 w2378 w2398]
      tunnel: w2136 -> [w2362 w2376 w2396]
      tunnel: [w2363 w2375 w2395] -> w2169
      tunnel: [w2362 w2374 w2394] -> w2168
      tunnel: ["T1 X (V)" ("Label.Text") "T1 X (nm)" ("Label.Text") "T1 X (pN)" ("Label.Text")] -> w2157
      tunnel: ["T2 X (V)" ("Label.Text") "T2 X (nm)" ("Label.Text") "T2 X (pN)" ("Label.Text")] -> w2156
      tunnel: ["Position (V)" ("Label.Text") "Position (nm)" ("Label.Text") "Force (pN)" ("Label.Text")] -> w2158
      tunnel: w2138 -> [_ w2366 w2385]
      tunnel: w2140 -> [_ w2369 w2387]
      tunnel: ["Mean (V)" ("Label.Text") "Mean (nm)" ("Label.Text") "Mean (pN)" ("Label.Text")] -> w2153
      tunnel: ["Difference (V)" ("Label.Text") "Difference (nm)" ("Label.Text") "Difference (pN)" ("Label.Text")] -> w2079
      frame 0, Default {
      }
      frame 1 {
        # "position"
        n1753 = Unbundle By Name(w2378) -> ("Y"=w2382:dbl[])
        n1754 = Unbundle By Name(w2376) -> ("Y"=w2367:dbl[])
        n1755 = Subtract(x=w2382, y=w2369) -> (x-y=w2370:dbl[])
        n1756 = Subtract(x=w2367, y=w2366) -> (x-y=w2368:dbl[])
        n1757 = Multiply(x=w2368, y=w2380) -> (x*y=w2377:dbl[])
        n1758 = Multiply(x=w2381, y=w2370) -> (x*y=w2379:dbl[])
        n1759 = Bundle By Name(cluster=w2376, "Y"=w2377) -> (w2374:waveform(dbl))
        n1760 = Bundle By Name(cluster=w2378, "Y"=w2379) -> (w2375:waveform(dbl))
      }
      frame 2 {
        # "force"
        n1761 = Unbundle By Name(w2398) -> ("Y"=w2403:dbl[])
        n1762 = Unbundle By Name(w2396) -> ("Y"=w2401:dbl[])
        n1763 = Subtract(x=w2401, y=w2385) -> (x-y=w2386:dbl[])
        n1764 = Subtract(x=w2403, y=w2387) -> (x-y=w2388:dbl[])
        n1765 = Compound Arithmetic op=MULTIPLY(w2386, w2400, w2393) -> (w2397:dbl[])
        n1766 = Compound Arithmetic op=MULTIPLY(w2392, w2402, w2388) -> (w2399:dbl[])
        n1767 = Bundle By Name(cluster=w2396, "Y"=w2397) -> (w2394:waveform(dbl))
        n1768 = Bundle By Name(cluster=w2398, "Y"=w2399) -> (w2395:waveform(dbl))
      }
    }
    n1769 = feedback-in #17("Calibration") -> ()
    n1770 = feedback #17(u16 1 ("Calibration")) -> (w2160:u16)
    n1771 = local read "Trap 2 Bead Size (nm)"() -> (w1958:dbl)
    n1772 = local read "Trap 1 Bead Size (nm)"() -> (w1957:dbl)
    n1773 = local read "AOM X Cal (nm/MHz)"() -> (w1955:dbl)
    n1774 = local read "Trap Delta (MHz)"() -> (w1954:dbl)
    n1775 = Not Equal?(x=w2160, y="Calibration") -> (x != y?=w2117:bool)
    n1776 = Multiply(x=w1955, y=w1954) -> (x*y=w1959:dbl)
    n1777 = Add(x=w1958, y=w1957) -> (x+y=w1961:dbl)
    n1778 = Unbundle By Name(w2139) -> ("Y"=w2142:dbl[])
    n1779 = Unbundle By Name(w2136) -> ("Y"=w2145:dbl[])
    n1780 = Divide(x=w1961, y=2.0) -> (x/y=w1956:dbl)
    n1781 = Subtract(x=w2142, y=w2140) -> (x-y=w2143:dbl[])
    n1782 = Subtract(x=w2145, y=w2138) -> (x-y=w2144:dbl[])
    n1783 = disable-structure shown="Enabled" {
      disable-tunnel: [-1.0 ("y") 1.0] -> w2146
      frame Disabled {
      }
      frame Enabled {
      }
    }
    n1784 = Multiply(x=w2144, y="T2 alpha_x (nm/V)") -> (x*y=w2135:dbl[])
    n1785 = Multiply(x="T1 alpha_x (nm/V)", y=w2143) -> (x*y=w2134:dbl[])
    n1786 = Multiply(x=w2168, y=w2146) -> (x*y=w2147:waveform(dbl))
    n1787 = case shown="False" "Read Lateness and Rel Phase" {
      tunnel: w1971 -> [w2329 w2351]
      tunnel: w1970 -> [w2330 w2350]
      tunnel: [w2329 w2349] -> w2132
      tunnel: [w2330 w2348] -> w2131
      frame False {
      }
      frame True {
        n1788 = xnode "Read/Write Control"("FPGA VI Reference In"=w2351, "error in"=w2350) -> ("FPGA VI Reference Out"=w2349:T19, "error out"=w2348:errorcluster, "GI Relative phase"=→"GI relative phase":i16, "Relative phase"=→"Relative phase (AI1)":i16, "AI Late Counter"=→"Late Counter (AI1)":u16, "GI Late Counter"=→"GI Late Counter":u16, "MCL Late Counter"=→"MCL Late Counter":u16, "MCL Relative Phase"=→"Relative Phase (MCL)":i16, "APD Acq Relative Phase"=→"APD Acq Relative Phase":i16, "APD 1 Gate Relative Phase"=→"APD 1 Gate Relative Phase":i16, "APD 2 Gate Relative Phase"=→"APD 2 Gate Relative Phase":i16, "APD Acq Late Counter"=→"APD Acq Late Counter":u16, "APD 1 Gate Late Counter"=→"APD 1 Gate Late Counter":u16, "APD 2 Gate Late Counter"=→"APD 2 Gate Late Counter":u16, "Green FB Relative Phase"=→"Relative phase (Green FB)":i16, "GI Relative phase 2"=→"GI relative phase 2":i16, "GI Late Counter 2"=→"GI Late Counter 2":u16, "Trap Pos FIFO Timeout"=→"Trap Pos FIFO Timeout":u16, "Trap AI FIFO Timeout"=→"Trap AI FIFO Timeout":u16)
      }
    }
    n1789 = Subtract(x=w2135, y=w2134) -> (x-y=w1953:dbl[])
    n1790 = call-poly <vilib>:"Mean.vi"("X"=w1953) -> ("mean"=w1960:dbl)  [unwired: 1 out]
    n1791 = Add(x=w1959, y=w1960) -> (x+y=w1963:dbl)
    n1792 = Subtract(x=w1963, y=w1956) -> (x-y=→"Tether Extension (nm, calculated)":dbl)
    n1793 = Unbundle By Name(w2168) -> ("Y"=w2104:dbl[])
    n1794 = Unbundle By Name(w2169) -> ("Y"=w2105:dbl[])
    n1795 = Build Array(w2169, w2147) -> (→"Force":waveform(dbl)[])
    n1796 = Subtract(x=w1953, y="Offset (nm)") -> (x-y=w2102:dbl[])
    n1797 = call-poly <vilib>:"Mean.vi"("X"=w2104) -> ("mean"=w2083:dbl)  [unwired: 1 out]
    "T2 X" <- w2083
    n1798 = Absolute Value(x=w2105) -> (abs(x)=w2106:dbl[])
    n1799 = Absolute Value(x=w2104) -> (abs(x)=w2107:dbl[])
    n1800 = call-poly <vilib>:"Mean.vi"("X"=w2105) -> ("mean"=w2084:dbl)  [unwired: 1 out]
    "T1 X" <- w2084
    n1801 = Add(x=w2106, y=w2107) -> (x+y=w2108:dbl[])
    n1802 = Bundle By Name(cluster=w2139, "Y"=w2102) -> (w2070:waveform(dbl))
    "Bead Separation" <- w2070
    n1803 = Divide(x=w2108, y=2.0) -> (x/y=→"Vec Mean of T1 T2":dbl[])
    n1804 = case shown="True" w2117 {
      tunnel: w2158 -> [_ w2356]
      tunnel: w2157 -> [_ w2355]
      tunnel: w2156 -> [_ w2354]
      tunnel: w2153 -> [_ w2353]
      tunnel: w2079 -> [_ w2352]
      frame False {
      }
      frame True {
        n1805 = property on="Force" class="WFChart (strict)"("YScale.NameLbl.Text"=w2356) -> ()  [unwired: 2 in, 2 out]
        n1806 = property on="T2 X" class="DigNum (strict)"("Caption.Text"=w2354) -> ()  [unwired: 2 in, 2 out]
        n1807 = property on="T1 X" class="DigNum (strict)"("Caption.Text"=w2355) -> ()  [unwired: 2 in, 2 out]
        n1808 = property on="Mean" class="DigNum (strict)"("Caption.Text"=w2353) -> ()  [unwired: 2 in, 2 out]
        n1809 = property on="Difference" class="DigNum (strict)"("Caption.Text"=w2352) -> ()  [unwired: 2 in, 2 out]
      }
    }
    n1810 = local read "Tether"() -> (w2111:bool)
    n1811 = Absolute Value(x=w2084) -> (abs(x)=w2081:dbl)
    n1812 = Absolute Value(x=w2083) -> (abs(x)=w2080:dbl)
    n1813 = Add(x=w2081, y=w2080) -> (x+y=w2155:dbl)
    n1814 = Subtract(x=w2081, y=w2080) -> (x-y=→"Difference":dbl)
    n1815 = feedback #18(w2102) -> (w2101:dbl[])
    n1816 = Divide(x=w2155, y=2.0) -> (x/y=w2110:dbl)
    "Mean" <- w2110
    n1817 = case shown="True" w2111 {
      tunnel: w2110 -> [_ w2288]
      frame False {
      }
      frame True {
        n1818 = Greater?(x="Lost Tether Alarm Threshold (pN)", y=w2288) -> (0:w2286:bool)
        n1819 = case shown="True" w2286 {
          frame False {
          }
          frame True {
            n1820 = flat-sequence {
              frame #0 {
                # "stop only if saving"
                n1821 = local read "Saving..."() -> (w2301:bool)
                n1822 = And(x=w2301, y="TA Cancel Save?") -> (x .and. y?=w2300:bool)
                n1823 = local write "Stop Saving"(w2300) -> ()
              }
              frame #1 {
                n1824 = case shown="True" "TA Green Off?" {
                  frame False {
                  }
                  frame True {
                    w2304 = FALSE ("Fl. Triggered...")
                    n1825 = local write "Fl. Triggered..."(w2304) -> ()
                    n1826 = property on="Green Laser ON/Interlacing" class="Bool (strict)"("Val(Sgnl)"=w2304) -> ()  [unwired: 2 in, 2 out]
                  }
                }
              }
            }
            n1827 = local read "Time tether formed"() -> (w2295:timestamp)
            n1828 = Get Date/Time In Seconds() -> (seconds since 1Jan1904=w2296:timestamp)
            n1829 = Subtract(x=w2296, y=w2295) -> (x-y=w2294:dbl)
            n1830 = Number To Decimal String(number=w2294) -> (decimal integer string=w2291:string)  [unwired: 1 out]
            n1831 = local read "Messages"() -> (w2298:string)
            n1832 = call <vilib>:"Beep.vi"() -> ()  [unwired: 3 in, 9 out]
            n1833 = Concatenate Strings("Lost tether (" ("Message to add"), w2291, " s)." ("string")) -> (w2293:string)
            n1834 = local write "Tether"(FALSE ("Tether")) -> ()
            n1835 = call "Update messages.vi"("Message to add"=w2293, "Old message string"=w2298) -> ("New message string"=w2297:string)
            n1836 = local write "Messages"(w2297) -> ()
            n1837 = property on="Trap Pos. FB ON" class="Bool (strict)"("Val(Sgnl)"=FALSE ("Value (Signaling)")) -> ()  [unwired: 2 in, 2 out]
          }
        }
      }
    }
    n1838 = Build Array (concatenate)(w2102, w2101) -> (w2100:dbl[])
    n1839 = Split 1D Array(array=w2100, index=w1982) -> (first subarray=w2096:dbl[])  [unwired: 1 out]
    n1840 = feedback-in #18(w2096) -> ()
    n1841 = call-poly <vilib>:"Mean.vi"("X"=w2096) -> ("mean"=w2095:dbl)  [unwired: 1 out]
    "Bead Mean (nm)" <- w2095
    n1842 = Subtract(x=w2096, y=w2095) -> (x-y=w2094:dbl[])
    n1843 = Square(x=w2094) -> (x^2=w2093:dbl[])
    n1844 = call-poly <vilib>:"Mean.vi"("X"=w2093) -> ("mean"=w2092:dbl)  [unwired: 1 out]
    n1845 = Square Root(x=w2092) -> (sqrt(x)=w2091:dbl)
    n1846 = Multiply(x=10.0, y=w2091) -> (x*y=→"RMS (Ang)":dbl)
    n1847 = xnode "Read/Write Control"("FPGA VI Reference In"=w2132, "error in"=w2131) -> ("FPGA VI Reference Out"=w2249:T19, "error out"=w2243:errorcluster, "AI4 Y Sum Set 1"=w2239:i16, "AI4 Y Sum Set 2"=w2238:i16, "AI1 X Set 1"=w2016:fxp<+/-,16,1>, "AI1 X Set 2"=w2015:fxp<+/-,16,1>, "Trap Pos FB Int Signal"=→"Trap Pos FB Int Signal":fxp<+/-,24,9>, "Trap Pos FB Int-Norm Signal"=→"Trap Pos FB Int-Norm Signal":fxp<+/-,16,1>, "Trap Pos FB Action"=w2009:i64, "Scanning"=→"AOD Scanning":bool, "Scan I"=→"AOD Scan I":u64, "Scanning MCL"=w2241:bool, "Scan I (MCL)"=→"MCL Scan I":u64, "Green FB Signals"=w2178:T47)  [unwired: 1 out]
    "MCL Scanning" <- w2241
    "Trap Pos FB Action" <- w2009
    n1848 = local read "AI2 (V)"() -> (w2240:cluster{"Set 1":dbl, "Set 2":dbl})
    n1849 = Bundle By Name(cluster=w2240, "Set 1"=w2239, "Set 2"=w2238) -> (w2236:cluster{"Set 1":dbl, "Set 2":dbl})
    n1850 = Divide(x=w2009, y=327.67) -> (x/y=→"Action (%)":dbl)
    n1851 = local read "Trap X (AI1)"() -> (w2029:T1)
    n1852 = Divide(x=w2236, y=3276.7) -> (x/y=w2235:cluster{"Set 1":dbl, "Set 2":dbl})
    n1853 = local write "AI2 (V)"(w2235) -> ()
    n1854 = Bundle(cluster=w2029, "Trap 1"=w2016, "Trap 2"=w2015) -> (→"Trap X (AI1)":T1)
    n1855 = Divide(x=w2178, y=3276.7) -> (x/y=w2174:T48)
    n1856 = Unbundle By Name(w2174) -> ("Green FB Ch 0"=w2177:dbl, "Green FB Ch 1"=w2176:dbl, "Green FB Ch 2"=w2175:dbl)
    n1857 = Divide(x=w2177, y=w2175) -> (x/y=w2173:dbl)
    n1858 = Divide(x=w2176, y=w2175) -> (x/y=w2172:dbl)
    n1859 = flat-sequence "To save data" {
      tunnel: [w3178] -> w2260
      tunnel: [w3179] -> w2259
      tunnel: w2209 -> [w3172]
      tunnel: w2098 -> [w3176]
      tunnel: ["Save Calibration"] -> w2232
      tunnel: w2229 -> [w3175]
      tunnel: [w3168] -> w2228
      tunnel: [w3165] -> w2227
      tunnel: [w3162] -> w2226
      tunnel: w2208 -> [w3164]
      tunnel: w2115 -> [w3158]
      tunnel: [w3158] -> w2114
      tunnel: ["Start Saving"] -> w2072
      tunnel: [w3152] -> w1998
      tunnel: [w3151] -> w1997
      tunnel: w2260 -> [w3413]
      tunnel: w2259 -> [w3412]
      tunnel: w1999 -> [w3411]
      tunnel: w2232 -> [w3410]
      tunnel: w2228 -> [w3408]
      tunnel: w2227 -> [w3407]
      tunnel: w2226 -> [w3406]
      tunnel: w2085 -> [w3405]
      tunnel: w2124 -> [w3404]
      tunnel: w2114 -> [w3403]
      tunnel: w2072 -> [w3402]
      tunnel: w2070 -> [w3401]
      tunnel: w2046 -> [w3400]
      tunnel: w1998 -> [w3399]
      tunnel: w1997 -> [w3398]
      tunnel: w1996 -> [w3397]
      frame #0 {
        n1860 = Or(x="Save N Sets", y="Start Saving") -> (x .or. y?=w3159:bool)
        n1861 = To Double Precision Float(number=w3175) -> (double precision float=w3169:dbl)
        n1862 = Build Array(w3159, "Save Calibration", w3172, w3164) -> (w3174:bool[])
        n1863 = Compound Arithmetic op=OR("Save Calibration", w3172, w3159, w3164) -> (w3177:bool)
        n1864 = Boolean Array To Number(Boolean array=w3174) -> (number=w3171:u32)
        n1865 = feedback #19(FALSE ("Save APD Data\nwith Trap Data")) -> (w3153:bool)
        n1866 = feedback #20(refnum<k0> refnum) -> (w3180:refnum<file>)
        n1867 = feedback #21(refnum<k0> refnum) -> (w3155:refnum<file>)
        n1868 = feedback #22(FALSE ("Save APD Data\nwith Trap Data")) -> (w3163:bool)
        n1869 = feedback #23(refnum<k0> refnum) -> (w3166:refnum<file>)
        n1870 = feedback #24(0) -> (w3182:i32)
        n1871 = feedback #25() -> (w3170:u32)  [unwired: 1 out]
        n1872 = case shown="True" w3177 {
          tunnel: [w3189 1] -> w3178
          tunnel: w3182 -> [w3191 _]
          tunnel: [w3190 w3209] -> w3179
          tunnel: w3180 -> [w3190 _]
          tunnel: w3176 -> [_ w3229]
          tunnel: w3169 -> [_ w3227]
          tunnel: w3171 -> [_ w3230]
          tunnel: [w3188 w3208] -> w3168
          tunnel: w3170 -> [w3188 _]
          tunnel: [w3187 w3206] -> w3165
          tunnel: w3166 -> [w3187 _]
          tunnel: [w3186 w3205] -> w3162
          tunnel: w3163 -> [w3186 _]
          tunnel: "Start Saving" -> [_ w3203]
          tunnel: w3158 -> [_ w3202]
          tunnel: [w3185 w3193] -> w3151
          tunnel: w3155 -> [w3185 _]
          tunnel: [w3184 w3192] -> w3152
          tunnel: w3153 -> [w3184 _]
          frame False {
            n1873 = Increment(x=w3191) -> (x+1=w3189:i32)
          }
          frame True {
            w3199 = FALSE ("Start Saving")
            w3204 = 9.0  # File Version
            w3212 = FALSE ("prepend array or string size? (T)")
            w3210 = T29."big-endian, network order" ("byte order (0:big-endian, network order)")
            # "write file headers"
            n1874 = local read "BD 1 Frequency 1 (MHz)"() -> (w3226:dbl)
            n1875 = local read "BD 2 Frequency 1 (MHz)"() -> (w3225:dbl)
            n1876 = local read "BD 1 Frequency 2 (MHz)"() -> (w3224:dbl)
            n1877 = local read "BD 2 Frequency 2 (MHz)"() -> (w3223:dbl)
            n1878 = local read "BD 1 Frequency 3 (MHz)"() -> (w3222:dbl)
            n1879 = local read "BD 2 Frequency 3 (MHz)"() -> (w3221:dbl)
            n1880 = Array Size(array=w3202) -> (size(s)=w3201:i32)
            n1881 = To Double Precision Float(number=w3201) -> (double precision float=w3200:dbl)
            n1882 = local write "Save Calibration"(w3199) -> ()
            n1883 = local write "Start Saving"(w3199) -> ()
            n1884 = Build Array("Save APD Data\nwith Trap Data", "Save Trap Pos. Data") -> (w3196:bool[])
            n1885 = Boolean Array To Number(Boolean array=w3196) -> (number=w3195:u32)
            n1886 = Build Array(w3226, w3225, w3224, w3223, w3222, w3221) -> (w3220:dbl[])
            n1887 = case shown="4" w3230 {
              tunnel: w3229 -> [w3301 w3321 w3337 w3375]
              tunnel: w3200 -> [w3306 w3328 w3357 w3394]
              tunnel: w3227 -> [w3305 w3327 w3356 w3393]
              tunnel: [w3302 w3323 w3348 w3385] -> w3218
              tunnel: [w3293 "Cal sets to save" w3338 w3376] -> w3208
              tunnel: w3220 -> [w3303 w3324 w3350 w3387]
              tunnel: "Save APD Data\nwith Trap Data" -> [w3300 _ w3334 w3373]
              tunnel: [w3300 w3315 w3334 w3373] -> w3205
              tunnel: w3204 -> [w3296 w3316 w3332 w3371]
              tunnel: w3203 -> [w3295 _ _ _]
              tunnel: [w3286 w3315 w3331 w3361] -> w3192
              tunnel: "Save Trap Pos. Data" -> [w3286 _ w3331 w3361]
              tunnel: w3195 -> [w3285 _ w3330 w3360]
              frame 1, Default {
                # "timeseries"
                n1888 = case shown="True" "Profile" {
                  tunnel: [w3309 w3312] -> w3290
                  tunnel: [w3309 w3311] -> w3289
                  tunnel: [w3309 w3310] -> w3288
                  tunnel: [w3309 w3314] -> w3287
                  frame False {
                    w3309 = 0.0 ("f")
                  }
                  frame True {
                    n1889 = local read "Current Position"() -> (w3313:dbl[])
                    n1890 = local read "Y change (mm)"() -> (w3314:dbl)
                    n1891 = call "subVI_explode3array.vi"("Array"=w3313) -> ("x"=w3312:dbl, "y"=w3311:dbl, "z"=w3310:dbl)  [unwired: 12 in]
                  }
                }
                n1892 = local read "Save ave N"() -> (w3308:dbl)
                n1893 = Multiply(x=w3308, y=w3301) -> (x*y=w3307:dbl)
                n1894 = To Double Precision Float(number=w3285) -> (double precision float=w3299:dbl)
                n1895 = Build Array(w3296, w3301, w3307, w3306, w3305, 0.0 ("f")) -> (w3304:dbl[])
                n1896 = Build Array(w3299, w3290, w3289, w3288, w3287) -> (w3297:dbl[])
                n1897 = Select(t=u32 4000000000, s=w3295, f="N sets to save") -> (s? t:f=w3293:u32)
                n1898 = Build Array (concatenate)(w3304, w3303, w3297) -> (w3302:dbl[])
              }
              frame 2 {
                w3318 = 0.0 ("f")
                w3315 = FALSE ("Save APD Data\nwith Trap Data")
                # "calibration"
                n1899 = Boolean To (0,1)(Boolean=w3315) -> (0, 1=w3320:i16)
                n1900 = To Double Precision Float(number=w3320) -> (double precision float=w3319:dbl)
                n1901 = Build Array(w3319, w3318, w3318, w3318, w3318) -> (w3317:dbl[])
                n1902 = Build Array(w3316, w3321, w3321, w3328, w3327, 1.0 ("t")) -> (w3325:dbl[])
                n1903 = Build Array (concatenate)(w3325, w3324, w3317) -> (w3323:dbl[])
                "Calibrating Trap..." <- TRUE ("Calibrating...")
              }
              frame 4 {
                w3335 = 0.0 ("f")
                # "write file header for a trap \nraster scan"
                # "scan dir (x/y = 0/1)"
                # "cycles/step"
                # "n scans (f/b)"
                # "steps"
                # "freq. range"
                # "AOD raster scan"
                n1904 = local read "Number of F/B Scans (AOD)"() -> (w3342:u16)
                n1905 = local read "Cycles/step (AOD)"() -> (w3344:u64)
                n1906 = local read "Scan Range (MHz)"() -> (w3347:dbl)
                n1907 = local read "Scan steps (AOD)"() -> (w3346:u64)
                n1908 = local read "Scan BD"() -> (w3354:bool)
                n1909 = local read "Save ave N"() -> (w3359:dbl)
                n1910 = Boolean To (0,1)(Boolean=w3354) -> (0, 1=w3353:i16)
                n1911 = To Double Precision Float(number=w3342) -> (double precision float=w3341:dbl)
                n1912 = To Double Precision Float(number=w3346) -> (double precision float=w3345:dbl)
                n1913 = To Double Precision Float(number=w3344) -> (double precision float=w3343:dbl)
                n1914 = To Double Precision Float(number=w3353) -> (double precision float=w3352:dbl)
                n1915 = Multiply(x=w3359, y=w3337) -> (x*y=w3358:dbl)
                n1916 = To Double Precision Float(number=w3330) -> (double precision float=w3336:dbl)
                n1917 = Build Array(w3336, w3335, w3335, w3335, w3335) -> (w3333:dbl[])
                n1918 = local read "N sets should be saved"() -> (w3339:dbl)
                n1919 = Build Array(w3352, w3347, w3345, w3343, w3341) -> (w3349:dbl[])
                n1920 = Build Array(w3332, w3337, w3358, w3357, w3356, 2.0 ("t")) -> (w3351:dbl[])
                n1921 = Round Toward +Infinity(x=w3339) -> (ceil(x): smallest int >= x=w3340:dbl)
                n1922 = Build Array (concatenate)(w3351, w3350, w3333, w3349) -> (w3348:dbl[])
                n1923 = To Unsigned Long Integer(number=w3340) -> (unsigned 32bit integer=w3338:u32)
              }
              frame 8 {
                w3368 = 0.0 ("f")
                # "MCL raster scan"
                n1924 = local read "Number of scans (MCL)"() -> (w3363:u64)
                n1925 = local read "Scan lines (y)"() -> (w3362:u64)
                n1926 = local read "2D or 1D Scan"() -> (w3365:bool)
                n1927 = local read "Scan Range (V)\n(of steps)"() -> (w3384:dbl)
                n1928 = local read "Fast Scan Dir"() -> (w3391:bool)
                n1929 = local read "Cycles/step (MCL)"() -> (w3381:u64)
                n1930 = local read "Scan steps (MCL)"() -> (w3383:u64)
                n1931 = Select(t=w3362, s=w3365, f=w3363) -> (s? t:f=w3364:u64)
                n1932 = Boolean To (0,1)(Boolean=w3365) -> (0, 1=w3367:i16)
                n1933 = local read "Save ave N"() -> (w3396:dbl)
                n1934 = local read "Initial X"() -> (w3370:dbl)
                n1935 = local read "Initial Y"() -> (w3369:dbl)
                n1936 = To Double Precision Float(number=w3367) -> (double precision float=w3366:dbl)
                n1937 = Boolean To (0,1)(Boolean=w3391) -> (0, 1=w3390:i16)
                n1938 = To Double Precision Float(number=w3364) -> (double precision float=w3379:dbl)
                n1939 = To Double Precision Float(number=w3383) -> (double precision float=w3382:dbl)
                n1940 = To Double Precision Float(number=w3381) -> (double precision float=w3380:dbl)
                n1941 = To Double Precision Float(number=w3390) -> (double precision float=w3389:dbl)
                n1942 = Multiply(x=w3396, y=w3375) -> (x*y=w3395:dbl)
                n1943 = To Double Precision Float(number=w3360) -> (double precision float=w3374:dbl)
                n1944 = local read "N sets should be saved (MCL)"() -> (w3377:dbl)
                n1945 = Build Array(w3374, w3366, w3368, w3368, w3368) -> (w3372:dbl[])
                n1946 = Build Array(w3389, w3384, w3382, w3380, w3379, w3370, w3369) -> (w3386:dbl[])
                n1947 = Build Array(w3371, w3375, w3395, w3394, w3393, 3.0 ("t")) -> (w3388:dbl[])
                n1948 = Round Toward +Infinity(x=w3377) -> (ceil(x): smallest int >= x=w3378:dbl)
                n1949 = Build Array (concatenate)(w3388, w3387, w3372, w3386) -> (w3385:dbl[])
                n1950 = To Unsigned Long Integer(number=w3378) -> (unsigned 32bit integer=w3376:u32)
              }
            }
            n1951 = local read "Index"() -> (w3235:dbl)
            n1952 = call "Create new save file.vi"("Insert"="", "Ext"=".dat", "Index In"=w3235) -> ("Path Out"=w3194:path, "Index Out"=w3207:dbl)
            n1953 = local write "Save file name"(w3194) -> ()
            n1954 = local write "Index"(w3207) -> ()
            n1955 = local write "Save index"(w3207) -> ()
            n1956 = Array Size(array=w3218) -> (size(s)=w3219:i32)
            n1957 = Open/Create/Replace File(file path (use dialog)=w3194, operation (0:open)=T23."create", access (0:read/write)=enum16{"read/write", "read-only", "write-only"}."write-only") -> (refnum out=w3232:refnum<file>)  [unwired: 1 in, 4 out]
            n1958 = local write "Saving..."(TRUE ("Saving...")) -> ()
            n1959 = To Double Precision Float(number=w3219) -> (double precision float=w3217:dbl)
            n1960 = String Length(string="Comment (data description)") -> (length=w3215:i32)
            n1961 = To Double Precision Float(number=w3215) -> (double precision float=w3214:dbl)
            n1962 = Deny Access(7:w3232) -> (3:w3231:refnum<file>)  [unwired: 1 in, 2 out]
            n1963 = Build Array (concatenate)(w3217, w3218, w3214) -> (w3216:dbl[])
            n1964 = case "If fluorescence data to be saved" shown="True" w3205 {
              tunnel: w3194 -> [_ w3284]
              tunnel: [refnum<k0> refnum w3264] -> w3206
              frame False {
              }
              frame True {
                w3263 = 0.0
                n1965 = local read "APD Integration Time (s)"() -> (w3269:dbl)
                n1966 = local read "N APD Samp/step"() -> (w3262:dbl)
                n1967 = Path To String(path=w3284) -> (string=w3283:string)
                n1968 = String Length(string=w3283) -> (length=w3282:i32)
                n1969 = Subtract(x=w3282, y=4) -> (x-y=w3280:i32)
                n1970 = String Subset(string=w3283, length (rest)=w3280) -> (substring=w3279:string)  [unwired: 1 out]
                n1971 = Build Array(w3269, w3262, w3263, w3263, w3263, w3263, w3263, w3263) -> (w3266:dbl[])
                n1972 = Concatenate Strings(w3279, "_fl.dat" ("string")) -> (w3277:string)
                n1973 = Array Size(array=w3266) -> (size(s)=w3268:i32)
                n1974 = String To Path(string=w3277) -> (path=w3273:path)
                n1975 = Open/Create/Replace File(file path (use dialog)=w3273, operation (0:open)=T23."create", access (0:read/write)=enum16{"read/write", "read-only", "write-only"}."write-only") -> (refnum out=w3274:refnum<file>)  [unwired: 1 in, 4 out]
                n1976 = Deny Access(7:w3274) -> (3:w3270:refnum<file>)  [unwired: 1 in, 2 out]
                n1977 = To Double Precision Float(number=w3268) -> (double precision float=w3267:dbl)
                n1978 = Build Array (concatenate)(w3267, w3266) -> (w3265:dbl[])
                n1979 = Write to Binary File(file (use dialog)=w3270, data=w3265, 5:FALSE ("prepend array or string size? (T)"), 9:T29."big-endian, network order" ("byte order (0:big-endian, network order)")) -> (refnum out=w3264:refnum<file>)  [unwired: 1 in, 3 out]
              }
            }
            n1980 = case shown="True" w3192 {
              tunnel: w3194 -> [_ w3246]
              tunnel: [refnum<k0> refnum w3245] -> w3193
              frame False {
              }
              frame True {
                w3241 = 0.0 ("element")
                n1981 = Path To String(path=w3246) -> (string=w3260:string)
                n1982 = Build Array(w3241, w3241, w3241, w3241, w3241, w3241, w3241, w3241) -> (w3242:dbl[])
                n1983 = String Length(string=w3260) -> (length=w3259:i32)
                n1984 = Subtract(x=w3259, y=4) -> (x-y=w3257:i32)
                n1985 = Array Size(array=w3242) -> (size(s)=w3244:i32)
                n1986 = String Subset(string=w3260, length (rest)=w3257) -> (substring=w3256:string)  [unwired: 1 out]
                n1987 = To Double Precision Float(number=w3244) -> (double precision float=w3243:dbl)
                n1988 = Concatenate Strings(w3256, "_pos.dat" ("string")) -> (w3254:string)
                n1989 = Build Array (concatenate)(w3243, w3242) -> (w3240:dbl[])
                n1990 = String To Path(string=w3254) -> (path=w3250:path)
                n1991 = Open/Create/Replace File(file path (use dialog)=w3250, operation (0:open)=T23."create", access (0:read/write)=enum16{"read/write", "read-only", "write-only"}."write-only") -> (refnum out=w3251:refnum<file>)  [unwired: 1 in, 4 out]
                n1992 = Deny Access(7:w3251) -> (3:w3247:refnum<file>)  [unwired: 1 in, 2 out]
                n1993 = Write to Binary File(file (use dialog)=w3247, data=w3240, 5:FALSE ("prepend array or string size? (T)"), 9:T29."big-endian, network order" ("byte order (0:big-endian, network order)")) -> (refnum out=w3245:refnum<file>)  [unwired: 1 in, 3 out]
              }
            }
            n1994 = Write to Binary File(file (use dialog)=w3231, data=w3216, 5:w3212, 9:w3210) -> (refnum out=w3213:refnum<file>)  [unwired: 1 in, 3 out]
            n1995 = Write to Binary File(file (use dialog)=w3213, data="Comment (data description)", 5:w3212, 9:w3210) -> (refnum out=w3209:refnum<file>)  [unwired: 1 in, 3 out]
          }
        }
        n1996 = feedback-in #19(w3152) -> ()
        n1997 = feedback-in #20(w3179) -> ()
        n1998 = feedback-in #21(w3151) -> ()
        n1999 = feedback-in #22(w3162) -> ()
        n2000 = feedback-in #23(w3165) -> ()
        n2001 = feedback-in #24(w3178) -> ()
        n2002 = feedback-in #25(w3168) -> ()
      }
      frame #1 {
        n2003 = local read "Saving..."() -> (w3409:bool)
        n2004 = case shown="True" w3409 {
          tunnel: w3413 -> [_ w3423]
          tunnel: w3412 -> [_ w3437]
          tunnel: w3411 -> [_ w3433]
          tunnel: w3410 -> [_ w3432]
          tunnel: w3408 -> [_ w3431]
          tunnel: w3407 -> [_ w3426]
          tunnel: w3406 -> [_ w3425]
          tunnel: w3405 -> [_ w3424]
          tunnel: w3404 -> [_ w3422]
          tunnel: w3403 -> [_ w3420]
          tunnel: w3402 -> [_ w3419]
          tunnel: w3401 -> [_ w3418]
          tunnel: w3400 -> [_ w3417]
          tunnel: w3399 -> [_ w3416]
          tunnel: w3398 -> [_ w3415]
          tunnel: w3397 -> [_ w3414]
          frame False {
          }
          frame True {
            n2005 = Multiply(x=w3423, y=w3422) -> (x*y=→"Time (s)":dbl)
            n2006 = Less Or Equal?(x=w3423, y=w3431) -> (x <= y?=w3435:bool)
            n2007 = Or(x="Stop Saving", y="Abort save 2") -> (x .or. y?=w3427:bool)
            n2008 = Not(x=w3427) -> (.not. x?=w3436:bool)
            n2009 = And(x=w3435, y=w3436) -> (x .and. y?=w3434:bool)
            n2010 = case shown="True" w3434 {
              tunnel: w3437 -> [w3444 w3512]
              tunnel: [0.0 w3515] -> w3430
              tunnel: w3423 -> [_ w3513]
              tunnel: w3431 -> [_ w3514]
              tunnel: w3433 -> [_ w3509]
              tunnel: w3432 -> [_ _]
              tunnel: w3426 -> [w3442 w3502]
              tunnel: w3425 -> [w3441 w3503]
              tunnel: w3424 -> [_ w3501]
              tunnel: w3420 -> [_ w3500]
              tunnel: w3419 -> [_ w3454]
              tunnel: w3418 -> [_ w3493]
              tunnel: w3417 -> [_ w3471]
              tunnel: w3416 -> [w3439 w3452]
              tunnel: w3415 -> [w3440 w3451]
              tunnel: w3414 -> [_ w3448]
              frame False {
                w3438 = FALSE
                n2011 = Close File(refnum=w3444) -> ()  [unwired: 1 in, 2 out]
                n2012 = case shown="True" w3441 {
                  tunnel: w3442 -> [_ w3446]
                  frame False {
                  }
                  frame True {
                    n2013 = Close File(refnum=w3446) -> ()  [unwired: 1 in, 2 out]
                  }
                }
                n2014 = case shown="True" w3439 {
                  tunnel: w3440 -> [_ w3445]
                  frame False {
                  }
                  frame True {
                    n2015 = Close File(refnum=w3445) -> ()  [unwired: 1 in, 2 out]
                  }
                }
                n2016 = local write "Calibrating Trap..."(w3438) -> ()
                n2017 = call <vilib>:"Beep.vi"() -> ()  [unwired: 3 in, 9 out]
                n2018 = local write "Stop Saving"(w3438) -> ()
                n2019 = property on="Raster Scanning..." class="Bool (strict)"("Val(Sgnl)"=w3438) -> ()  [unwired: 2 in, 2 out]
                "Saving..." <- w3438
              }
              frame True {
                n2020 = local read "Calibrating Trap..."() -> (w3504:bool)
                n2021 = case "Write fl. data" shown="True" w3503 {
                  tunnel: w3502 -> [_ w3538]
                  tunnel: w3501 -> [_ w3537]
                  frame False {
                  }
                  frame True {
                    n2022 = Write to Binary File(file (use dialog)=w3538, data=w3537, 5:FALSE ("prepend array or string size? (T)"), 9:T29."big-endian, network order" ("byte order (0:big-endian, network order)")) -> ()  [unwired: 1 in, 4 out]
                  }
                }
                n2023 = Greater?(x="Save ave N", y=1.0) -> (0:w3507:bool)
                n2024 = Not(x=w3504) -> (.not. x?=w3506:bool)
                n2025 = And(x=w3506, y=w3507) -> (x .and. y?=w3449:bool)
                n2026 = case shown="True" w3449 {
                  tunnel: w3448 -> [w3518 w3529]
                  tunnel: [w3518 w3521] -> w3447
                  tunnel: "Save ave N" -> [_ w3522]
                  frame False {
                  }
                  frame True {
                    w3519 = 2 ("dimension size")
                    n2027 = Array Size(array=w3529) -> (size(s)=w3523:i32)
                    n2028 = Divide(x=w3523, y=w3519) -> (x/y=w3527:dbl)
                    n2029 = Reshape Array(w3529, w3527, w3519) -> (w3528:u64[][])
                    n2030 = Transpose 2D Array(2D array=w3528) -> (transposed array=w3526:u64[][])
                    n2031 = for {
                      tunnel: w3526 -> [w3531] mode=indexing
                      tunnel: [w3530] -> w3520 mode=indexing
                      tunnel: w3522 -> [w3532]
                      workers-P: _ -> [_]
                      n2032 = call "downsample 1D array - U64.vi"("Ave N"=w3532, "Array In"=w3531) -> ("Array Out"=w3530:u64[])  [unwired: 1 in]
                    }
                    n2033 = Transpose 2D Array(2D array=w3520) -> (transposed array=w3525:u64[][])
                    n2034 = Divide(x=w3523, y=w3522) -> (x/y=w3524:dbl)
                    n2035 = Reshape Array(w3525, w3524) -> (w3521:u64[])
                  }
                }
                n2036 = case shown="True" w3449 {
                  tunnel: w3509 -> [w3541 w3553]
                  tunnel: [w3541 w3545] -> w3505
                  tunnel: "Save ave N" -> [_ w3546]
                  tunnel: w3500 -> [_ w3544]
                  frame False {
                    # "don't downsample data for trap calibration"
                  }
                  frame True {
                    n2037 = Array Size(array=w3553) -> (size(s)=w3547:i32)
                    n2038 = Array Size(array=w3544) -> (size(s)=w3543:i32)
                    n2039 = Divide(x=w3547, y=w3543) -> (x/y=w3551:dbl)
                    n2040 = Reshape Array(w3553, w3551, w3543) -> (w3552:i16[][])
                    n2041 = Transpose 2D Array(2D array=w3552) -> (transposed array=w3550:i16[][])
                    n2042 = for {
                      tunnel: w3550 -> [w3556] mode=indexing
                      tunnel: [w3555] -> w3542 mode=indexing
                      tunnel: w3546 -> [w3554]
                      workers-P: _ -> [_]
                      n2043 = call "downsample 1D array - I16.vi"("Ave N"=w3554, "Array In"=w3556) -> ("Array Out"=w3555:i16[])  [unwired: 1 out]
                    }
                    n2044 = Transpose 2D Array(2D array=w3542) -> (transposed array=w3549:i16[][])
                    n2045 = Divide(x=w3547, y=w3546) -> (x/y=w3548:dbl)
                    n2046 = Reshape Array(w3549, w3548) -> (w3545:i16[])
                  }
                }
                n2047 = Index Array(array=w3471, index=1) -> (element=w3474:waveform(dbl))
                n2048 = Index Array(array=w3471, index=0) -> (element=w3476:waveform(dbl))
                n2049 = Unbundle By Name(w3474) -> ("Y"=w3478:dbl[])
                n2050 = Unbundle By Name(w3476) -> ("Y"=w3486:dbl[])
                n2051 = case "Write trap pos. data" shown="True" w3452 {
                  tunnel: w3451 -> [_ w3534]
                  tunnel: w3447 -> [_ w3533]
                  frame False {
                  }
                  frame True {
                    n2052 = Write to Binary File(file (use dialog)=w3534, data=w3533, 5:FALSE ("prepend array or string size? (T)"), 9:T29."big-endian, network order" ("byte order (0:big-endian, network order)")) -> ()  [unwired: 1 in, 4 out]
                  }
                }
                n2053 = Write to Binary File(file (use dialog)=w3512, data=w3505, 5:FALSE ("prepend array or string size? (T)"), 9:T29."big-endian, network order" ("byte order (0:big-endian, network order)")) -> ()  [unwired: 1 in, 4 out]
                n2054 = feedback #26(w3478) -> (w3480:dbl[])
                n2055 = Build Array (concatenate)(w3480, w3478) -> (w3479:dbl[])
                n2056 = Select(t=w3478, s=w3454, f=w3479) -> (s? t:f=w3464:dbl[])
                n2057 = feedback-in #26(w3464) -> ()
                n2058 = feedback #27(w3486) -> (w3499:dbl[])
                n2059 = Build Array (concatenate)(w3499, w3486) -> (w3498:dbl[])
                n2060 = Select(t=w3486, s=w3454, f=w3498) -> (s? t:f=w3473:dbl[])
                n2061 = feedback-in #27(w3473) -> ()
                n2062 = Divide(x=w3513, y=w3514) -> (x/y=w3516:dbl)
                n2063 = Multiply(x=w3516, y=100.0) -> (x*y=w3515:dbl)
                n2064 = Build Array(w3473, w3464) -> (→"Saved APD":dbl[][])
                n2065 = Array Size(array=w3473) -> (size(s)=w3491:i32)
                n2066 = Unbundle By Name(w3493) -> ("Y"=w3497:dbl[])
                n2067 = Subtract(x=w3491, y="N pts to average") -> (x-y=w3467:i32)
                n2068 = Multiply(x="N pts to average", y=u16 2) -> (x*y=w3468:u16)
                n2069 = Subtract(x=w3491, y=w3468) -> (x-y=w3466:i32)
                n2070 = feedback #28(w3497) -> (w3496:dbl[])
                n2071 = Build Array (concatenate)(w3496, w3497) -> (w3495:dbl[])
                n2072 = Select(t=w3497, s=w3454, f=w3495) -> (s? t:f=w3494:dbl[])
                "Trap Delta Graph" <- w3494
                n2073 = feedback-in #28(w3494) -> ()
                n2074 = Array Subset(array=w3473, index=w3467, length="N pts to average") -> (w3490:dbl[])
                n2075 = Array Subset(array=w3473, index=w3466, length="N pts to average") -> (w3489:dbl[])
                n2076 = Array Subset(array=w3464, index=w3467, length="N pts to average") -> (w3470:dbl[])
                n2077 = Array Subset(array=w3464, index=w3466, length="N pts to average") -> (w3469:dbl[])
                n2078 = call-poly <vilib>:"Mean.vi"("X"=w3490) -> ("mean"=w3488:dbl)  [unwired: 1 out]
                n2079 = call-poly <vilib>:"Mean.vi"("X"=w3470) -> ("mean"=w3463:dbl)  [unwired: 1 out]
                n2080 = call-poly <vilib>:"Mean.vi"("X"=w3489) -> ("mean"=w3487:dbl)  [unwired: 1 out]
                n2081 = call-poly <vilib>:"Mean.vi"("X"=w3469) -> ("mean"=w3462:dbl)  [unwired: 1 out]
                n2082 = Subtract(x=w3463, y=w3462) -> (x-y=w3453:dbl)
                "Delta Fl. 2" <- w3453
                n2083 = Subtract(x=w3488, y=w3487) -> (x-y=w3485:dbl)
                "Delta Fl. 1" <- w3485
                n2084 = Initialize Array(w3485, 1 ("dimension size")) -> (w3482:dbl[])
                n2085 = Initialize Array(w3453, 1 ("dimension size")) -> (w3459:dbl[])
                n2086 = feedback #29(w3482) -> (w3483:dbl[])
                n2087 = Build Array (concatenate)(w3483, w3482) -> (w3481:dbl[])
                n2088 = feedback #30(w3459) -> (w3460:dbl[])
                n2089 = Build Array (concatenate)(w3460, w3459) -> (w3458:dbl[])
                n2090 = Select(t=w3482, s=w3454, f=w3481) -> (s? t:f=w3457:dbl[])
                n2091 = feedback-in #29(w3457) -> ()
                n2092 = Select(t=w3459, s=w3454, f=w3458) -> (s? t:f=w3456:dbl[])
                n2093 = feedback-in #30(w3456) -> ()
                n2094 = Build Array(w3457, w3456) -> (→"Save APD Deriv":dbl[][])
              }
            }
            "Progress" <- w3430
            "Progress 2" <- w3430
          }
        }
      }
    }
    n2095 = Bundle By Name(cluster=w2174, "Green FB Ch 0"=w2173, "Green FB Ch 1"=w2172) -> (w2152:T48)
    "Green FB Signals (V)" <- w2152
    n2096 = Unbundle By Name(w2152) -> ("Green FB Ch 2"=→"Green FB Plot":dbl)
    n2097 = local read "wait to reset values"() -> (w2244:bool)
    n2098 = Not(x=w2241) -> (.not. x?=w2245:bool)
    n2099 = And(x=w2245, y=w2244) -> (x .and. y?=w2246:bool)
    n2100 = case "Part of MCL raster scanning: returns to initial positions after scan done" shown="False" w2246 {
      tunnel: w2249 -> [w2982 w2989]
      tunnel: [w2982 w2988] -> w2248
      tunnel: w2243 -> [w2981 w2987]
      tunnel: [w2981 w2986] -> w2242
      frame False {
      }
      frame True {
        w2997 = 10.0 ("y")
        w2996 = 32767.0 ("y")
        # "to return scan values\nafter a synchronous \nAOM scan"
        n2101 = local read "AO2"() -> (w2990:dbl)
        n2102 = local read "AO1"() -> (w2991:dbl)
        n2103 = local write "wait to reset values"(FALSE ("wait to reset values")) -> ()
        n2104 = Multiply(x=w2991, y=w2996) -> (x*y=w2993:dbl)
        n2105 = Multiply(x=w2990, y=w2996) -> (x*y=w2995:dbl)
        n2106 = Divide(x=w2993, y=w2997) -> (x/y=w2992:dbl)
        n2107 = Divide(x=w2995, y=w2997) -> (x/y=w2994:dbl)
        n2108 = To Word Integer(number=w2992) -> (16bit integer=w2998:i16)
        n2109 = To Word Integer(number=w2994) -> (16bit integer=w2999:i16)
        n2110 = local read "Total Counts (ticks)"() -> (w2983:u32)
        n2111 = xnode "Read/Write Control"("FPGA VI Reference In"=w2989, "error in"=w2987, "AO1"=w2998, "AO2"=w2999, "MCL count"=w2983) -> ("FPGA VI Reference Out"=w2988:T19, "error out"=w2986:errorcluster)
        n2112 = local read "Scan Range (V)\n(of steps)"() -> (w2984:dbl)
        n2113 = property on="Scan Range (V)\n(of steps)" class="DigNum (strict)"("Val(Sgnl)"=w2984) -> ()  [unwired: 2 in, 2 out]
      }
    }
    n2114 = node-c288() -> ()  [unwired: 2 out]
  }
  n2115 = node-c288(3 ("Processor")) -> (w74:T24)  [unwired: 3 out]
  n2116 = timed-loop "Oscillate AOD (debugging)" {
    tunnel: w24 -> [w3558]
    tunnel: [w3557] -> w36
    timing: w74 -> [_]
    timing-out: [_] -> w73
    stop <- w3557 stop-if-true
    n2117 = node-c288() -> ()  [unwired: 2 out]
    n2118 = event shown="[0] \"Oscillate Set 2\", \"Fish for Tether\": Value Change" {
      selector: _ -> [_ _ _]
      dyn-events: _ -> [_ _ _]
      timeout: _ -> [_ _ _]
      tunnel: w3558 -> [w3565 _ _]
      tunnel: [FALSE ("Stop All") _ w3833] -> w3557
      event "Oscillate Set 2", "Fish for Tether": Value Change {
        n2119 = event-data() -> ()  [unwired: 6 out]
        n2120 = local read "Oscillate Set 2"() -> (w3564:bool)
        n2121 = Or(x=w3564, y="Fish for Tether") -> (x .or. y?=w3562:bool)
        n2122 = case shown="True" w3562 {
          tunnel: w3565 -> [_ w3568]
          tunnel: "Fish for Tether" -> [_ w3567]
          frame False {
          }
          frame True {
            n2123 = case shown="True" w3567 {
              frame False {
              }
              frame True {
                n2124 = local write "Scan axis 2"(TRUE) -> ()
                n2125 = local write "Tether"(FALSE ("Tether")) -> ()
              }
            }
            n2126 = node-c288("Period") -> (w3570:T24)  [unwired: 3 out]
            n2127 = timed-loop "Oscillate AOD" {
              timing: w3570 -> [_]
              timing-out: [_] -> w3569
              tunnel: w3568 -> [w3580]
              tunnel: w3567 -> [w3579]
              i -> [w3582]
              stop <- w3578 stop-if-true
              n2128 = node-c288() -> (w3581:i64)  [unwired: 1 out]
              n2129 = flat-sequence {
                tunnel: w3582 -> [w3608]
                tunnel: w3581 -> [w3607]
                tunnel: w3580 -> [w3591]
                tunnel: w3579 -> [w3593]
                tunnel: [w3593] -> w3577
                tunnel: [w3592] -> w3576
                tunnel: [w3590] -> w3575
                tunnel: [w3587] -> w3573
                tunnel: w3577 -> [w3644]
                tunnel: w3576 -> [w3642]
                tunnel: w3575 -> [w3641]
                tunnel: [w3640] -> w3574
                tunnel: w3573 -> [w3639]
                tunnel: [w3708] -> w3578
                tunnel: w3574 -> [w3706]
                frame #0 {
                  n2130 = Divide(x=w3607, y=i64 1000) -> (x/y=w3602:dbl)
                  n2131 = Multiply(x=w3602, y=w3608) -> (x*y=w3604:dbl)
                  n2132 = Multiply(x="Osc. freq. (Hz)", y=6.283185307179586) -> (x*y=w3605:dbl)
                  n2133 = Multiply(x=w3605, y=w3604) -> (x*y=w3589:dbl)
                  n2134 = local read "BD 1 Frequency 2 (MHz)"() -> (w3586:dbl)
                  n2135 = local read "BD 1 Frequency 1 (MHz)"() -> (w3583:dbl)
                  n2136 = case shown="True" w3593 {
                    tunnel: w3589 -> [w3614 w3621]
                    tunnel: w3586 -> [_ w3631]
                    tunnel: [w3611 w3615] -> w3594
                    tunnel: [FALSE w3624] -> w3590
                    tunnel: [0.0 w3617] -> w3587
                    tunnel: w3583 -> [_ w3616]
                    frame False {
                      n2137 = Sine(x=w3614) -> (sin(x)=w3612:dbl)
                      n2138 = Multiply(x=w3612, y="Osc. amp. (MHz)") -> (x*y=w3611:dbl)
                    }
                    frame True {
                      n2139 = Cosine(x=w3621) -> (cos(x)=w3634:dbl)
                      n2140 = Subtract(x=w3631, y=w3616) -> (x-y=w3630:dbl)
                      n2141 = Decrement(x=w3634) -> (x-1=w3633:dbl)
                      n2142 = Subtract(x=w3630, y="Closest Delta (MHz)") -> (x-y=w3627:dbl)
                      n2143 = Divide(x=w3633, y=2.0) -> (x/y=w3628:dbl)
                      n2144 = Multiply(x=w3628, y=w3627) -> (x*y=w3615:dbl)
                      n2145 = local read "Vec Mean of T1 T2"() -> (w3623:dbl[])
                      n2146 = Greater?(x=w3623, y="Stop F (pN)") -> (0:w3625:bool[])
                      n2147 = Or Array Elements(Boolean array=w3625) -> (logical OR=w3624:bool)
                      n2148 = Divide(x=w3621, y=6.283185307179586) -> (x/y=w3620:dbl)
                      n2149 = Round Toward +Infinity(x=w3620) -> (ceil(x): smallest int >= x=w3617:dbl)
                      "Attempts" <- w3617
                      n2150 = Greater?(x=w3617, y="Attempt Limit") -> (0:w3619:bool)
                      n2151 = case shown="True" w3619 {
                        frame False {
                        }
                        frame True {
                          n2152 = local write "Fish for Tether"(FALSE ("Fish for Tether")) -> ()
                          n2153 = call <vilib>:"Beep.vi"() -> ()  [unwired: 3 in, 9 out]
                          n2154 = local read "Messages"() -> (w3636:string)
                          n2155 = call "Update messages.vi"("Message to add"="Tether fishing timeout." ("Messages"), "Old message string"=w3636) -> ("New message string"=→"Messages":string)
                        }
                      }
                    }
                  }
                  n2156 = local read "Y RF Frequency Limits (MHz)"() -> (w3595:T16)
                  n2157 = local read "X RF Frequency Limits (MHz)"() -> (w3596:T16)
                  n2158 = local read "BD 1 Frequency 3 (MHz)"() -> (w3601:dbl)
                  n2159 = local read "BD 2 Frequency 2 (MHz)"() -> (w3585:dbl)
                  n2160 = Select(t=w3586, s="Scan axis 2", f=w3585) -> (s? t:f=w3597:dbl)
                  n2161 = Add(x=w3594, y=w3597) -> (x+y=w3592:dbl)
                  n2162 = Select(t=w3592, s="Scan axis 2", f=w3586) -> (s? t:f=w3584:dbl)
                  n2163 = Select(t=w3585, s="Scan axis 2", f=w3592) -> (s? t:f=w3599:dbl)
                  n2164 = local read "BD 2 Frequency 3 (MHz)"() -> (w3600:dbl)
                  n2165 = call "set RF board frequency - interlace.vi"("Board 2 Frequency Limits"=w3595, "Board 1 Frequency Limits"=w3596, "FPGA VI Reference In"=w3591, "Board 2 Frequency 3 (MHz)"=w3600, "Board 1 Frequency 3 (MHz)"=w3601, "Board 2 Frequency 2 (MHz)"=w3585, "Board 2 Frequency 1 (MHz)"=w3599, "Board 1 Frequency 2 (MHz)"=w3584, "Board 1 Frequency 1  (MHz)"=w3583) -> ()  [unwired: 1 in, 2 out]
                }
                frame #1 {
                  n2166 = And(x=w3644, y=w3641) -> (x .and. y?=w3643:bool)
                  n2167 = case "Only if were fishing and now formed tether" shown="True" w3643 {
                    tunnel: w3642 -> [w3646 w3658]
                    tunnel: [w3645 w3657] -> w3640
                    tunnel: w3639 -> [_ w3653]
                    frame False {
                      n2168 = local read "Fish for Tether"() -> (w3645:bool)
                      n2169 = case shown="True" w3645 {
                        tunnel: w3646 -> [_ _]
                        frame False {
                        }
                        frame True {
                        }
                      }
                    }
                    frame True {
                      w3657 = FALSE ("Fish for Tether")
                      n2170 = call <vilib>:"Beep.vi"() -> ()  [unwired: 3 in, 9 out]
                      n2171 = Number To Decimal String(number=w3653, width (-)=i16 1) -> (decimal integer string=w3651:string)
                      n2172 = case shown="\"2\", \"3\", \"4\", \"5\", \"6\"" "Then..." {
                        selector: "Then..." -> [_ w3661]
                        tunnel: w3658 -> [w3660 _]
                        frame "1", Default {
                          # "do nothing"
                          n2173 = property on="BD 1 Frequency 1 (MHz)" class="DigNum (strict)"("Val(Sgnl)"=w3660) -> ()  [unwired: 2 in, 2 out]
                        }
                        frame "2", "3", "4", "5", "6" {
                          n2174 = flat-sequence {
                            tunnel: w3661 -> [w3663]
                            frame #0 {
                              n2175 = property on="Trap Delta (MHz)" class="DigNum (strict)"("Val(Sgnl)"="Move to Delta 1 (MHz)") -> ()  [unwired: 2 in, 2 out]
                            }
                            frame #1 {
                              n2176 = case shown="\"5\", \"6\"" w3663 {
                                selector: w3663 -> [w3666 w3676 _]
                                frame "3", "4" {
                                n2177 = flat-sequence {
                                tunnel: w3666 -> [w3667]
                                tunnel: [w3667] -> w3664
                                tunnel: [w3669] -> w3665
                                tunnel: w3664 -> [w3669]
                                tunnel: w3665 -> [w3673]
                                frame #0 {
                                n2178 = property on="Green Laser ON/Interlacing" class="Bool (strict)"("Val(Sgnl)"=TRUE ("Value (Signaling)")) -> ()  [unwired: 2 in, 2 out]
                                }
                                frame #1 {
                                n2179 = Multiply(x="Wait Before Save (s)", y=u32 1000 ("x")) -> (x*y=w3671:u32)
                                n2180 = Wait (ms)(milliseconds to wait=w3671) -> ()  [unwired: 1 out]
                                }
                                frame #2 {
                                n2181 = property on="Start Saving" class="Bool (strict)"("Value"=TRUE ("Start Saving")) -> ()  [unwired: 2 in, 2 out]
                                n2182 = case shown="Default" w3673 {
                                frame Default {
                                }
                                frame "4" {
                                n2183 = property on="Fl. Triggered..." class="Bool (strict)"("Val(Sgnl)"=TRUE ("Value (Signaling)")) -> ()  [unwired: 2 in, 2 out]
                                }
                                }
                                }
                                }
                                }
                                frame "5", "6" {
                                n2184 = stacked-sequence {
                                tunnel: w3676 -> [_ _ _ _ _ _ _ _ w3693 _ _]
                                frame #0 {
                                n2185 = Replace Array Subset(array=u32[] [0] ("Index Values"), new element="Raster Set Upon Tether", index=0) -> (w3677:u32[])
                                n2186 = property on="Saved AOD Raster Scan Parameter Sets" class="Arr (strict)"("Index Values"=w3677) -> ()  [unwired: 2 in, 2 out]
                                }
                                frame #1 {
                                n2187 = Wait (ms)(milliseconds to wait=u32 500) -> ()  [unwired: 1 out]
                                }
                                frame #2 {
                                n2188 = property on="Load parameters" class="Bool (strict)"("Val(Sgnl)"=TRUE ("Value (Signaling)")) -> ()  [unwired: 2 in, 2 out]
                                }
                                frame #3 {
                                n2189 = Wait (ms)(milliseconds to wait=u32 500) -> ()  [unwired: 1 out]
                                }
                                frame #4 {
                                n2190 = property on="Trap Raster Scan" class="Bool (strict)"("Val(Sgnl)"=TRUE ("Value (Signaling)")) -> ()  [unwired: 2 in, 2 out]
                                }
                                frame #5 {
                                n2191 = Wait (ms)(milliseconds to wait=u32 2000) -> ()  [unwired: 1 out]
                                }
                                frame #6 {
                                n2192 = while {
                                stop <- w3688 stop-if-true
                                n2193 = local read "Raster Scanning..."() -> (w3687:bool)
                                n2194 = local read "Saving..."() -> (w3690:bool)
                                n2195 = Wait (ms)(milliseconds to wait=u32 100) -> ()  [unwired: 1 out]
                                n2196 = Not(x=w3690) -> (.not. x?=w3689:bool)
                                n2197 = Not(x=w3687) -> (.not. x?=w3686:bool)
                                n2198 = And(x=w3689, y=w3686) -> (x .and. y?=w3688:bool)
                                }
                                }
                                frame #7 {
                                n2199 = property on="Trap Delta (MHz)" class="DigNum (strict)"("Val(Sgnl)"="Move to Delta 2 (MHz)") -> ()  [unwired: 2 in, 2 out]
                                }
                                frame #8 {
                                n2200 = local read "Tether"() -> (w3694:bool)
                                n2201 = case shown="True" w3694 {
                                tunnel: w3693 -> [_ w3695]
                                frame False {
                                }
                                frame True {
                                n2202 = flat-sequence {
                                tunnel: w3695 -> [w3697]
                                frame #0 {
                                n2203 = Wait (ms)(milliseconds to wait=u32 500) -> ()  [unwired: 1 out]
                                }
                                frame #1 {
                                n2204 = case shown="\"6\"" w3697 {
                                frame Default {
                                }
                                frame "6" {
                                n2205 = property on="Green Laser ON/Interlacing" class="Bool (strict)"("Val(Sgnl)"=TRUE ("Green Laser ON/Interlacing")) -> ()  [unwired: 2 in, 2 out]
                                }
                                }
                                }
                                frame #2 {
                                n2206 = Wait (ms)(milliseconds to wait=u32 500) -> ()  [unwired: 1 out]
                                }
                                frame #3 {
                                n2207 = local write "Start Saving"("Save at end (5, 6)") -> ()
                                }
                                }
                                }
                                }
                                }
                                frame #9 {
                                n2208 = local read "Bead Sep. Int. Time (s)"() -> (w3703:dbl)
                                n2209 = Multiply(x=w3703, y=1000.0) -> (x*y=w3702:dbl)
                                n2210 = Wait (ms)(milliseconds to wait=w3702) -> ()  [unwired: 1 out]
                                }
                                frame #10 {
                                n2211 = property on="Rescale on Mean" class="Bool (strict)"("Val(Sgnl)"=TRUE ("Value (Signaling)")) -> ()  [unwired: 2 in, 2 out]
                                }
                                }
                                }
                                frame "2", Default {
                                }
                              }
                            }
                          }
                        }
                      }
                      n2212 = Concatenate Strings("Formed tether in ", w3651, " attempt(s)." ("string")) -> (w3648:string)
                      n2213 = local read "Messages"() -> (w3655:string)
                      n2214 = local write "Fish for Tether"(w3657) -> ()
                      n2215 = call "Update messages.vi"("Message to add"=w3648, "Old message string"=w3655) -> ("New message string"=w3654:string)
                      n2216 = local write "Messages"(w3654) -> ()
                      n2217 = Get Date/Time In Seconds() -> (seconds since 1Jan1904=→"Time tether formed":timestamp)
                      "Tether" <- "Tether Alarm?"
                    }
                  }
                }
                frame #2 {
                  n2218 = local read "Oscillate Set 2"() -> (w3707:bool)
                  n2219 = local read "Stop All"() -> (w3709:bool)
                  n2220 = Not Or(1:w3706, 2:w3707) -> (0:w3705:bool)
                  n2221 = Compound Arithmetic op=OR(w3709, w3705) -> (w3708:bool)
                }
              }
              n2222 = node-c288() -> ()  [unwired: 2 out]
            }
            n2223 = node-c288(w3569) -> ()  [unwired: 1 out]
          }
        }
      }
      event "Fl. Triggered...": Value Change {
        n2224 = event-data() -> ()  [unwired: 7 out]
        n2225 = case shown="True" "Fl. Triggered..." {
          frame False {
          }
          frame True {
            n2226 = node-c288() -> (w3721:T24)  [unwired: 4 out]
            n2227 = timed-loop {
              timing: w3721 -> [_]
              timing-out: [_] -> w3720
              tunnel: "Action" -> [w3725]
              shift-right: [w3722] -> _
              shift-left: u8 255 -> [w3724]
              stop <- w3726 stop-if-true
              n2228 = node-c288() -> ()  [unwired: 2 out]
              n2229 = flat-sequence {
                tunnel: w3725 -> [w3738]
                tunnel: w3724 -> [w3735]
                tunnel: [w3734] -> w3723
                tunnel: [w3824] -> w3726
                tunnel: w3723 -> [w3823]
                tunnel: [w3823] -> w3722
                frame #0 {
                  n2230 = local read "Delta Fl. 2"() -> (w3729:dbl)
                  n2231 = local read "Delta Fl. 1"() -> (w3730:dbl)
                  n2232 = Select(t=w3730, s="APD to Watch", f=w3729) -> (s? t:f=w3728:dbl)
                  n2233 = Multiply(x="Fl. Delta Thresh. (kHz)", y=1000.0) -> (x*y=w3737:dbl)
                  n2234 = Greater?(x=w3728, y=w3737) -> (0:w3732:bool)
                  n2235 = Or(x="Force Yank", y=w3732) -> (x .or. y?=w3733:bool)
                  n2236 = case shown="True" w3733 {
                    tunnel: w3738 -> [_ w3748]
                    tunnel: w3735 -> [w3740 w3744]
                    tunnel: [w3740 w3741] -> w3734
                    frame False {
                    }
                    frame True {
                      n2237 = flat-sequence {
                        tunnel: w3745 -> [w3754]
                        tunnel: [w3754] -> w3749
                        tunnel: w3748 -> [w3753]
                        tunnel: [w3753] -> w3747
                        tunnel: [w3752] -> w3746
                        tunnel: w3744 -> [w3751]
                        tunnel: [w3750] -> w3743
                        tunnel: w3749 -> [w3779]
                        tunnel: w3747 -> [w3778]
                        tunnel: w3746 -> [w3777]
                        tunnel: w3743 -> [w3776]
                        tunnel: [w3776] -> w3742
                        tunnel: w3742 -> [w3821]
                        tunnel: [w3821] -> w3741
                        frame #0 {
                          n2238 = call <vilib>:"Beep.vi"() -> ()  [unwired: 3 in, 9 out]
                          n2239 = local write "Waiting"(FALSE ("Waiting")) -> ()
                          n2240 = Increment(x=w3751) -> (x+1=w3750:u8)
                          n2241 = case shown="\"Yank\"" w3753 {
                            tunnel: w3750 -> [_ _ w3760]
                            frame "Image" {
                              n2242 = property on="Confocal Image" class="Bool (strict)"("Val(Sgnl)"=TRUE ("Value (Signaling)")) -> ()  [unwired: 2 in, 2 out]
                            }
                            frame "Alarm", Default {
                            }
                            frame "Yank" {
                              n2243 = flat-sequence {
                                tunnel: w3760 -> [w3763]
                                tunnel: [w3762] -> w3759
                                tunnel: ["N Array El"] -> w3758
                                tunnel: w3759 -> [w3773]
                                tunnel: w3758 -> [w3769]
                                frame #0 {
                                n2244 = Multiply(x="Yank Delay (s)", y=1000.0) -> (x*y=w3766:dbl)
                                n2245 = Quotient & Remainder(x=w3763, y="N Array El") -> (x-y*floor(x/y)=w3762:u8)  [unwired: 1 out]
                                n2246 = Wait (ms)(milliseconds to wait=w3766) -> ()  [unwired: 1 out]
                                }
                                frame #1 {
                                n2247 = Random Number (0-1)() -> (number: 0 to 1=w3770:dbl)
                                n2248 = Multiply(x=w3769, y=w3770) -> (x*y=w3768:dbl)
                                n2249 = Round Toward -Infinity(1:w3768) -> (0:w3767:dbl)
                                n2250 = Select(t=w3767, s="Random Choice", f=w3773) -> (s? t:f=w3771:dbl)
                                n2251 = Index Array(array="Yank to Delta Array (MHz)", index=w3771) -> (element=w3774:dbl)
                                n2252 = property on="Trap Delta (MHz)" class="DigNum (strict)"("Val(Sgnl)"=w3774) -> ()  [unwired: 2 in, 2 out]
                                }
                              }
                            }
                          }
                          n2253 = local read "Time (s)"() -> (w3752:dbl)
                          "Fl. High" <- TRUE ("Yanking")
                        }
                        frame #1 {
                          n2254 = node-c288() -> (w3781:T24)  [unwired: 4 out]
                          n2255 = timed-loop {
                            timing: w3781 -> [_]
                            timing-out: [_] -> w3780
                            tunnel: w3779 -> [w3797]
                            tunnel: w3778 -> [w3795]
                            tunnel: w3777 -> [w3794]
                            stop <- w3796 stop-if-true
                            n2256 = node-c288() -> ()  [unwired: 2 out]
                            n2257 = local read "Fl. Delta Thresh. (kHz)"() -> (w3789:dbl)
                            n2258 = local read "Fl. Triggered..."() -> (w3798:bool)
                            n2259 = local read "Delta Fl. 1"() -> (w3785:dbl)
                            n2260 = local read "Delta Fl. 2"() -> (w3783:dbl)
                            n2261 = local read "Stop All"() -> (w3792:bool)
                            n2262 = local read "APD to Watch"() -> (w3784:bool)
                            n2263 = Select(t=w3785, s=w3784, f=w3783) -> (s? t:f=w3782:dbl)
                            n2264 = Not(x=w3798) -> (.not. x?=w3793:bool)
                            n2265 = Multiply(x=w3789, y=1000.0) -> (x*y=w3788:dbl)
                            n2266 = Negate(x=w3788) -> (-x=w3787:dbl)
                            n2267 = Less?(x=w3782, y=w3787) -> (x < y?=w3791:bool)
                            n2268 = Compound Arithmetic op=OR(w3791, w3792, w3793, "Force Reset") -> (w3796:bool)
                            n2269 = case shown="True" w3796 {
                              tunnel: w3797 -> [_ w3809]
                              tunnel: w3795 -> [_ w3808]
                              tunnel: w3794 -> [_ w3806]
                              frame False {
                              }
                              frame True {
                                n2270 = case shown="\"Yank\"" w3808 {
                                tunnel: w3809 -> [_ w3810]
                                frame "Image", Default {
                                }
                                frame "Yank" {
                                n2271 = flat-sequence {
                                tunnel: [w3815] -> w3811
                                tunnel: w3810 -> [w3815]
                                tunnel: w3811 -> [w3816]
                                frame #0 {
                                n2272 = local read "Yank Delay (s)"() -> (w3814:dbl)
                                n2273 = Multiply(x=w3814, y=1000.0) -> (x*y=w3812:dbl)
                                n2274 = Wait (ms)(milliseconds to wait=w3812) -> ()  [unwired: 1 out]
                                }
                                frame #1 {
                                n2275 = property on="Trap Delta (MHz)" class="DigNum (strict)"("Val(Sgnl)"=w3816) -> ()  [unwired: 2 in, 2 out]
                                }
                                }
                                }
                                }
                                n2276 = local read "Time (s)"() -> (w3807:dbl)
                                n2277 = Subtract(x=w3807, y=w3806) -> (x-y=w3803:dbl)
                                "Duration (s)" <- w3803
                                n2278 = Number To Decimal String(number=w3803, width (-)=i16 0) -> (decimal integer string=w3801:string)
                                n2279 = Concatenate Strings(w3801, " s fluorescence event." ("string")) -> (w3799:string)
                                n2280 = local read "Messages"() -> (w3805:string)
                                n2281 = call "Update messages.vi"("Message to add"=w3799, "Old message string"=w3805) -> ("New message string"=w3804:string)
                                n2282 = call <vilib>:"Beep.vi"() -> ()  [unwired: 3 in, 9 out]
                                n2283 = local write "Messages"(w3804) -> ()
                              }
                            }
                            n2284 = node-c288() -> ()  [unwired: 2 out]
                          }
                          n2285 = node-c288(w3780) -> ()  [unwired: 1 out]
                        }
                        frame #2 {
                          n2286 = local write "Fl. High"(FALSE ("Yanking")) -> ()
                        }
                      }
                      n2287 = local read "Trap Delta (MHz)"() -> (w3745:dbl)
                    }
                  }
                }
                frame #1 {
                  n2288 = local read "Stop All"() -> (w3827:bool)
                  n2289 = local read "Fl. Triggered..."() -> (w3825:bool)
                  n2290 = Not(x=w3825) -> (.not. x?=w3826:bool)
                  n2291 = Or(x=w3826, y=w3827) -> (x .or. y?=w3824:bool)
                  n2292 = Not(x=w3824) -> (.not. x?=→"Waiting":bool)
                }
              }
              n2293 = node-c288() -> ()  [unwired: 2 out]
            }
            n2294 = node-c288(w3720) -> ()  [unwired: 1 out]
          }
        }
      }
      event "Stop All": Value Change {
        n2295 = event-data() -> ()  [unwired: 7 out]
        n2296 = local read "Stop All"() -> (w3833:bool)
      }
    }
    n2297 = node-c288() -> ()  [unwired: 2 out]
  }
  n2298 = node-c288(w73) -> ()  [unwired: 1 out]
  n2299 = node-c288(w163) -> ()  [unwired: 1 out]
  n2300 = flat-sequence {
    tunnel: w33 -> [w3838]
    tunnel: [w3837] -> w39
    tunnel: [w3834] -> w38
    tunnel: w37 -> [_]
    tunnel: w36 -> [_]
    tunnel: w35 -> [_]
    tunnel: w34 -> [_]
    tunnel: w32 -> [w3835]
    tunnel: w39 -> [w3841]
    tunnel: w38 -> [w3840]
    frame #0 {
      w3836 = FALSE ("APD to FIFO")
      n2301 = xnode "Read/Write Control"("FPGA VI Reference In"=w3838, "error in"=w3835, "APD to FIFO"=w3836, "AI to FIFO"=w3836) -> ("FPGA VI Reference Out"=w3837:T19, "error out"=w3834:errorcluster)
    }
    frame #1 {
      n2302 = xnode "Invoke Method"("FPGA VI Reference In"=w3841, "error in"=w3840) -> ("FPGA VI Reference Out"=w3839:T19)  [unwired: 1 out]
      n2303 = xnode "Close FPGA VI Reference"("FPGA VI Reference In"=w3839) -> ()  [unwired: 1 in, 1 out]
    }
  }
